vi "main4ChProspectiveStudyBK20251125.vi"() -> ()   [LabVIEW 2024]
doc: "Main VI for FLS imaging system."
uses:
  SubVI/DigitizerConfiguration/FLImDAQ.ctl
  <instrlib>/niScope/Controls/niScope trigger source.ctl
  SubVI/LabJack/LJ Pin Setting.ctl
  ConfigFiles/AimingBeamVideoConfig.ctl
  LaguerreDeconLib/DeconEngineClass/LaguerreDeconEngineClass.lvclass/LaguerreDeconEngineClass.ctl
  <vilib>/Utility/error.llb/DialogType.ctl
  LaguerreDeconLib/DeconEngineClass/LaguerreDeconEngineClass.lvclass
  <vilib>/event_ctls.llb/usereventprio.ctl
  <vilib>/Utility/miscctls.llb/LVMinMaxIncTypeDef.ctl
  SubVI/APD/APDClass.lvclass
  <vilib>/Analysis/baseanly.llb/Mean (DBL).vi
  SubVI/GlobalVariables.vi
  <vilib>/addons/control/pid/pid.llb/PID (DBL).vi
  <instrlib>/niScope/Acquire/Fetch/niScope Multi Fetch Binary 16.vi
  <vilib>/Instr/_visa.llb/VISA Configure Serial Port (Instr).vi
  <vilib>/Python/Open Anaconda Python Session.vi
  C:/Users/MarcuLab/Documents/GitHub/NetDeconForLV/Source/DotNETAssembly/output/build/LaguerreDeConNative.dll
  Documents/GitHub/NetDeconForLV/Source/DotNETAssembly/output/build/LaguerreDeConNative.dll
  <userlib>/_OpenG.lib/file/file.llb/openg_file.lvlib
  <userlib>/_OpenG.lib/time/time.llb/openg_time.lvlib
  <vilib>/Analysis/NI_AALBase.lvlib
  <vilib>/Utility/miscctls.llb/LVPointTypeDef.ctl
  <vilib>/addons/control/pid/NI_PID_pid.lvlib
panel:
  in  "488nm Power":u16(ring)=32 items=["3.30mW"=60, "2.35mW"=50, "2.00mW"=47, "1.75mW"=44, "1.48mW"=41, "1.16mW"=38, "0.87mW"=35, "0.57mW"=32, "0.28mW"=29]
  in  "CancerThreshold":dbl=0.15
  out "Decon Loop timing (ms)":dbl
  out "Ch3 Lifetime (ns)":dbl caption="Lifetime (ns)"
  out "Ch2 Lifetime (ns)":dbl caption="Lifetime (ns)"
  out "Ch1 Lifetime (ns)":dbl caption="Lifetime (ns)"
  out "Cancer Prob":dbl
  in  "Overlay selection":u16(ring)=2 items=["Gain", "Lifetime", "CancerProbability"]
  out "Record Backlog 2":i32
  in  "Auto gain ch4":bool=TRUE caption="Auto gain ch3"
  in  "V 4":dbl caption="Gain 3" min=0.0 max=4.67 step=0.1
  out "Gain4":dbl
  out "IntR4":dbl format="%#_2g"
  out "SNR4":dbl format="%#_3g"
  out "Channel 4":dbl[][](graph) caption="Channel 3"
  out "RunStartTime":u32
  out "Dig1 Temp":dbl
  out "Dig2 Temp":dbl
  out "Visualization PC video source":T1
  in  "V target(1.0)":dbl=1.0 caption="V target(1.5)" min=0.3 max=1.5 step=0.1 format="%#_4g"
  out "SNR3":dbl format="%#_3g"
  out "SNR2":dbl format="%#_3g"
  out "SNR1":dbl format="%#_3g"
  in  "Show BG removed?":bool=TRUE
  out "IntR3":dbl format="%#_2g"
  out "IntR2":dbl format="%#_2g"
  out "IntR1":dbl format="%#_2g"
  in  "Video Display":bool
  out "Gain3":dbl
  out "Gain2":dbl
  out "Gain1":dbl
  in  "Skip Data Save?":bool
  out "Aq Loop?":bool
  out "ML?":bool
  out "aquisition loop Error Out":errorcluster
  out "Laser f (Hz)":dbl
  out "Record Backlog":i32
  out "Fetch Record #":i32
  out "Sync Success?":bool
  out "Disclamer":picture
  out "Calibration #":i8
  out "BG #":i8
  in  "TCP Connect":bool
  out "Help":string
  in  "355nm Laser toggle":bool caption="355nm 460Hz"
  in  "Cali&iRF alignment":bool
  in  "Background":bool
  in  "Aiming beam toggle":bool caption="488nm 15Hz"
  in  "Auto gain ch3":bool=TRUE
  in  "Auto gain ch2":bool=TRUE
  in  "Auto gain ch1":bool=TRUE
  out "Run #":i8
  in  "StopButton":bool caption="Stop"
  out "Aquisition Status:":bool
  in  "StartButton":bool caption="Start"
  in  "V 3":dbl caption="Gain 3" min=0.0 max=4.65 step=0.1
  in  "V 2":dbl caption="Gain 2" min=0.0 max=4.59 step=0.1
  in  "V 1":dbl caption="Gain 1" min=0.0 max=4.63 step=0.1 format="%#_4g"
  in  "Video Source":enum32{"Camera", "FrameGrabber"}(radio)
  out "Case #":string
  out "System Hardware Connection Status":T2
  out "Channel 3":dbl[][](graph)
  out "Channel 2":dbl[][](graph)
  out "Channel 1":dbl[][](graph)
  in  "Tab Control":T3(tab)
  out "display loop timing(ms)":u32
  out "Aquisition loop timing(ms)":u32 format="%.2f"
  out "DisplayLoop":i32
  out "PID loop":i32 caption="processing loop"
  out "PID loop timing(ms)":u32 caption="processing loop timing(ms)"
  out "Communication loop(ms)":u32
  out "laser EM lamp V":dbl format="%0.6f"
  out "Auisition Loop idx":i32
  out "LJ process (ms)":u32
  out "LJ time(ms)":u32[](array[numeric])
  out "output variable":i32
  out "BG Graph":dbl[][](graph)
  out "Lifetime (ns)":cluster{dbl, dbl, dbl}(graph)
  out "DeCon Speed(ms)":dbl(graph)
  out "iRF Graph":dbl[][](graph)
  in  "Show BG":bool
  out "iRF length":i32
  out "BG length":i32
  out "data length":i32
  out "WarmupTime(ms)":u32
  out "BGAll":dbl[][](array[numeric])
  out "DeConOut":dbl[](array[numeric])
  in  "Ch1GainLim":dbl=350.0 format="%#_13g"
  in  "Ch2&3GainLim":dbl=1750.0 format="%#_13g"
  out "LJ Pinout":T4={"Ch1 Bias"="DAC0", "Ch2 Bias"="DAC1", "Ch3 Bias"="DAC2", "Ch4 Bias"="DAC0", "355 PWM"="FIO0", "AimingBeam PWM"="FIO2", "Laser Ready"="FIO3", "Interlock"="FIO1", "Laser Start/Stop"="FIO1", "Red LED"="FIO1", "Green LED"="DIO3", "Foot Pedal"="DIO15"}
  out "FLImDAQ":T5={"Digitizer 1"="", "Digitizer 2"="", "Channel"=enum."Channel 0", "trigger source"="VAL_EXTERNAL", "trigger level"=0.5, "trigger delay"=1.35e-07, "min sample rate"=12500000000.0, "min record length"=2500, "vertical range"=1.0, "vertical offset"=-0.25, "Waveform to Avg"=2000} caption="FLIm DAQ Configuration" {"trigger delay" format="%^#.4e"; "trigger level" min=0.0 max=3.5 step=0.5 format="%.2f"; "vertical offset" format="%.4f"; "vertical range" format="%.2f"; "min sample rate" format="%#.2p"}
  in  "Sys Reconfig":bool
  out "data out(communcation loop)":string
  out "PID loop error out":errorcluster caption="processing Error Out"
  out "decon error out":errorcluster
  out "Laser Rep Rate":dbl
  out "V4 Size":i32 caption="V3 Size"
  in  "Data Class":enum16{"Data", "BG", "Cali"}(ring)=enum."BG"
  out "V1 Size":i32
  out "V2 Size":i32
  out "V3 Size":i32
  out "data Size":i32[](array[numeric])
  out "State log":string
  out "SysConfigCluster":T7
  in  "Ch4 PID gains":T8={"proportional gain (Kc)"=30.0, "integral time (Ti, min)"=0.0003, "derivative time (Td, min)"=1e-05}
  in  "Ch3 PID gains":T8={"proportional gain (Kc)"=30.0, "integral time (Ti, min)"=0.0003, "derivative time (Td, min)"=1e-05}
  in  "Ch2 PID gains":T8={"proportional gain (Kc)"=30.0, "integral time (Ti, min)"=0.0003, "derivative time (Td, min)"=1e-05}
  in  "Ch1 PID gains":T8={"proportional gain (Kc)"=30.0, "integral time (Ti, min)"=0.0003, "derivative time (Td, min)"=1e-05}
  in  "module path":path=path "C:/Users/MarcuLab/Documents/GitHub/NetDeconForLV/Classifier/HNClassifier.py"
  in  "model path":path=path "C:/Users/MarcuLab/Documents/GitHub/NetDeconForLV/Classifier/20241127_dc/200.pkl"
  in  "Env name":string="HNClassifier"
  in  "Python version":string="3.10"
  out "Python session":refnum<k35>
  in  "Quit":bool
  in  "Radio Buttons":T9(radio)=enum."Ch2" caption="DeCon Chan"
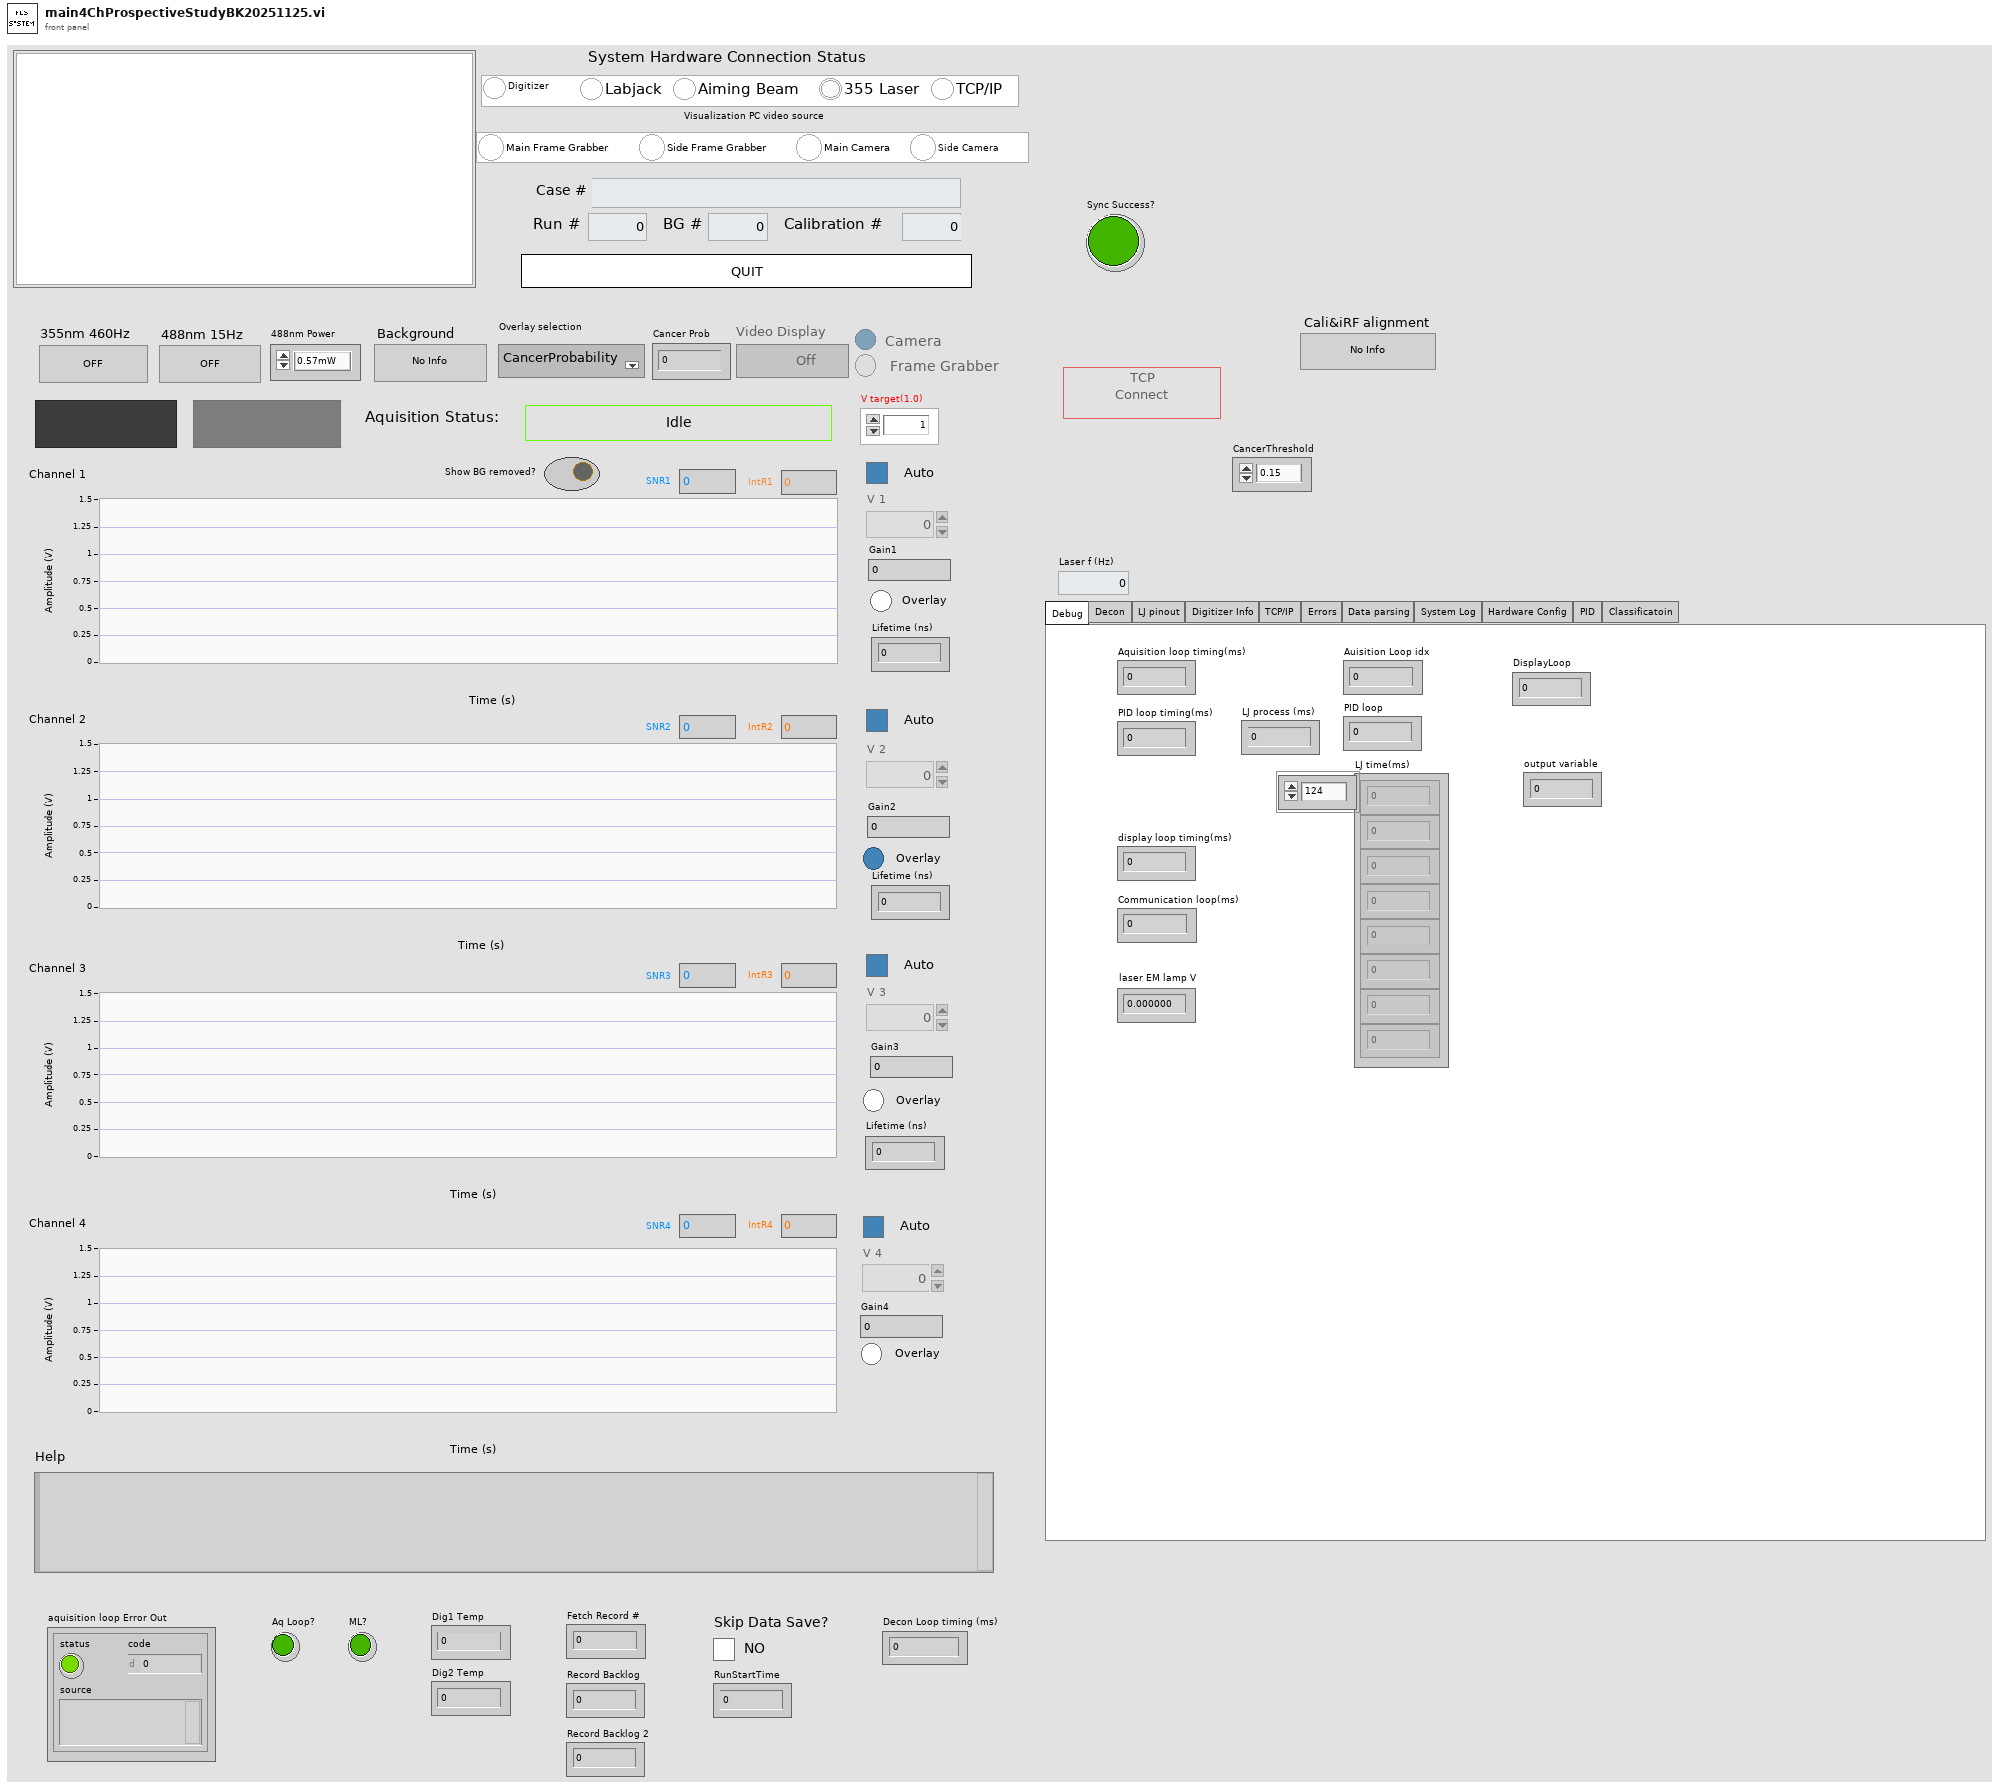
[diagram p1: front panel]
types:
  T1 = cluster{"Main Frame Grabber":bool, "Side Frame Grabber":bool, "Main Camera":bool, "Side Camera":bool}
  T2 = cluster{"Digitizer":bool, "Labjack":bool, "Aiming Beam":bool, "355 Laser":bool, "TCP/IP":bool}
  T3 = enum32{"Debug", "Decon", "LJ pinout", "Digitizer Info", "TCP/IP", "Errors", "Data parsing", "System Log", "Hardware Config", "PID", "Classificatoin"}
  T4 = typedef "LJ Pin Setting.ctl" = cluster{"Ch1 Bias":string, "Ch2 Bias":string, "Ch3 Bias":string, "Ch4 Bias":string, "355 PWM":string, "AimingBeam PWM":string, "Laser Ready":string, "Interlock":string, "Laser Start/Stop":string, "Red LED":string, "Green LED":string, "Foot Pedal":string}
  T5 = typedef "FLImDAQ.ctl" = cluster{"Digitizer 1":refnum<k15>, "Digitizer 2":refnum<k15>, "Channel":enum16{"Channel 0", "Channel 1", "Channel 0&1"}, "trigger source":T6, "trigger level":dbl, "trigger delay":dbl, "min sample rate":dbl, "min record length":i32, "vertical range":dbl, "vertical offset":dbl, "Waveform to Avg":i16}
  T6 = typedef "niScope trigger source.ctl" = string
  T7 = cluster{"Ch1Enable?":bool, "Ch2Enable?":bool, "Ch3Enable?":bool, "Ch1AutoGain?":bool, "Ch2AutoGain?":bool, "Ch3AutoGain?":bool, "AimingBeamEnable?":bool}
  T8 = cluster{"proportional gain (Kc)":dbl, "integral time (Ti, min)":dbl, "derivative time (Td, min)":dbl}
  T9 = enum32{"No Selection", "Ch1", "Ch2", "Ch3", "Ch4"}
  T10 = cluster{"remote start event":refnum<user-event>, "remote stop  event":refnum<user-event>}
  T11 = enum8{"Enabled", "Disabled", "Disabled and Grayed Out"}
  T12 = enum16{"open", "replace", "create", "open or create", "replace or create", "replace or create with confirmation"}
  T13 = cluster{"CH1":dbl[][], "CH2":dbl[][], "CH3":dbl[][], "CH4":dbl[][], "Gain cluster":cluster{"V1":dbl, "V2":dbl, "V3":dbl, "V4":dbl}}
  T14 = cluster{"idx":i32, "CH1&2":dbl[][], "CH3&4":dbl[][], "V cluster":cluster{"V1":dbl, "V2":dbl, "V3":dbl, "V4":dbl}}
  T15 = cluster{"Ch1 iRF":dbl[], "Ch2 iRF":dbl[], "Ch3 iRF":dbl[], "Ch4 iRF":dbl[]}
  T16 = enum16{"open", "open or create", "create or replace", "create", "open (read-only)"}
  T17 = enum32{"Invalid", "Standard", "Closed", "Hidden", "Minimized", "Maximized"}
  T18 = enum32{"invalid app kind", "Development System", "Run Time System", "Student Edition", "Embedded LabVIEW", "Evaluation", "Custom"}
  T19 = typedef "usereventprio.ctl" = enum32{"high priority", "normal priority"}
  T20 = enum32{"Bad", "Idle", "Run top level", "Running"}
  T21 = enum16{"Standard", "Buffered", "CRLF", "Immediate"}
  T22 = typedef "AimingBeamVideoConfig.ctl" = cluster{"DeCon Channel":enum16{"1", "2", "3"}, "Scale Bar":bool, "Scale Low":dbl, "Scale High":dbl, "ANSI":dbl, "Radius":dbl, "3D?":bool, "Firefly?":bool, "Pentero?":bool}
  T23 = cluster{"Core":cluster{"Current VI Reference":refnum<vi>, "Close Panel on Exit?":bool}, "SysConfigCluster":cluster{"Ch1Enable?":bool, "Ch2Enable?":bool, "Ch3Enable?":bool, "Ch1AutoGain?":bool, "Ch2AutoGain?":bool, "Ch3AutoGain?":bool, "AimingBeamEnable?":bool}, "System Status":cluster{"Digitizer":bool, "Labjack":bool, "Aiming Beam":bool, "355 Laser":bool, "TCP/IP":bool}, "IDs":cluster{"RunID":i8, "BG ID":i8, "Cali ID":i8}, "CaseID":string, "DefaultPath":path, "Pathes":cluster{"DataPath":path, "BG Path":path, "iRFPath":path, "CaliPath":path}, "FLImDAQ":cluster{"resource name":refnum<k15>, "resource name 2":refnum<k15>, "Channel":enum16{"Channel 0", "Channel 1", "Channel 0&1"}, "trigger source":T6, "trigger level":dbl, "trigger delay":dbl, "min sample rate":dbl, "min record length":i32, "vertical range":dbl, "vertical offset":dbl, "Waveform to Avg":i32}, "SysRunning?":bool, "AB Cluster":cluster{"Aiming Beam COM Port":refnum<visa-resource-name>, "Min Current":dbl, "Max Current":dbl, "Default Current":dbl, "Freq":i32}, "LJ Pinout":T4, "355 PWM setting":cluster{"DIO_EF_CLOCK1_DIVISOR":i16, "DIO_EF_CLOCK1_ROLL_VALUE":i32, "DIO#_EF_INDEX":i16, "DIO#_EF_OPTIONS":i16, "DIO#_EF_CONFIG_A":i32}, "AB PWM setting":cluster{"DIO_EF_CLOCK1_DIVISOR":i16, "DIO_EF_CLOCK1_ROLL_VALUE":i32, "DIO#_EF_INDEX":i16, "DIO#_EF_OPTIONS":i16, "DIO#_EF_CONFIG_A":i32}, "Last Trigger":u32, "niTClk sessions":refnum<k20>[], "Laser start tic":u32, "TCP attempt count":i32, "Ch1Data":dbl[][], "Ch2Data":dbl[][], "Ch3Data":dbl[][], "Ch4Data":dbl[][], "V1":dbl[], "V2":dbl[], "V3":dbl[], "V4":dbl[], "SlowTimer":u32, "FastTimer":u32, "listener ID":refnum<k5>, "TempPath":path, "CaliPath":path, "LED vi reference":refnum<vi>, "Aquisition Timer":u32, "APDSerialNum":cluster{"Ch1APDSerial#":string, "Ch2APDSerial#":string, "Ch3APDSerial#":string, "Ch4APDSerial#":string}, "VideoConfig":T22, "LED vi ref open?":bool, "video source":cluster{"Main Frame Grabber":bool, "Side Frame Grabber":bool, "Main Camera":bool, "Side Camera":bool}, "bothVidSourceAvail":bool}
  T24 = typedef "LVCursorListTypeDef.ctl" = cluster{"Name":string, "Color":u32, "Style":u8, "Point Style":u8, "Name Visible":bool, "Allow Drag":bool, "Cursor Mode":u32, "Plot":i32, "Index":i32, "Position":cluster{"X":dbl, "Y":dbl}, "X Scale":u32, "Y Scale":u32, "Watch Plots":i32[], "Watch All Plots":bool, "Plot Area":i32, "Label Offset":cluster{"X":dbl, "Y":dbl}}[]
  T25 = cluster{"Name":string, "Color":u32, "Style":u8, "Point Style":u8, "Name Visible":bool, "Allow Drag":bool, "Cursor Mode":u32, "Plot":i32, "Index":i32, "Position":cluster{"X":dbl, "Y":dbl}, "X Scale":u32, "Y Scale":u32, "Watch Plots":i32[], "Watch All Plots":bool, "Plot Area":i32, "Label Offset":cluster{"X":dbl, "Y":dbl}}
  T26 = cluster{"Ch1APDSerial#":string, "Ch2APDSerial#":string, "Ch3APDSerial#":string, "Ch4APDSerial#":string}
  T27 = cluster{"DataPath":path, "BG Path":path, "iRFPath":path, "CaliPath":path}
  T28 = cluster{"DIO_EF_CLOCK1_DIVISOR":i16, "DIO_EF_CLOCK1_ROLL_VALUE":i32, "DIO#_EF_INDEX":i16, "DIO#_EF_OPTIONS":i16, "DIO#_EF_CONFIG_A":i32}
  T29 = cluster{"Aiming Beam COM Port":refnum<visa-resource-name>, "Min Current":dbl, "Max Current":dbl, "Default Current":dbl, "Freq":i32}
  T30 = cluster{"resource name":refnum<k15>, "resource name 2":refnum<k15>, "Channel":enum16{"Channel 0", "Channel 1", "Channel 0&1"}, "trigger source":T6, "trigger level":dbl, "trigger delay":dbl, "min sample rate":dbl, "min record length":i32, "vertical range":dbl, "vertical offset":dbl, "Waveform to Avg":i32}
  T31 = cluster{"Current VI Reference":refnum<vi>, "Close Panel on Exit?":bool}
  T32 = cluster{"Channel 1":dbl[], "Channel 2":dbl[], "Channel 3":dbl[], "Channel 4":dbl[]}
  T33 = cluster{"V 1":dbl[], "V 2":dbl[], "V 3":dbl[], "V 4":dbl[]}
  T34 = cluster{"Ch1 WF":dbl[], "Ch2 WF":dbl[], "Ch3 WF":dbl[], "Ch4 WF":dbl[], "V1":dbl, "V2":dbl, "V3":dbl, "V4":dbl}
  T35 = typedef "iRFData.ctl" = cluster{"dt":dbl, "NumOfWFs":i32, "WFLength":i32, "iRFCtrlV":dbl[], "iRFWFsAvg":dbl[][], "iRFRaw":dbl[][]}
  T36 = cluster{"mean":dbl, "mean":dbl, "mean":dbl, "mean":dbl}
  T37 = cluster{"V1":dbl, "V2":dbl, "V3":dbl, "V4":dbl}[]
  T38 = cluster{"DataPath":path, "CaseID":string, "RunID":i16, "Ch1Data":dbl[][], "Ch2Data":dbl[][], "Ch3Data":dbl[][], "Ch4Data":dbl[][], "V1":dbl[], "V2":dbl[], "V3":dbl[], "V4":dbl[], "LaserRepRate":u16, "WFAverage":i16, "RunStartTime":u64}
  T39 = typedef "DialogType.ctl" = u16
  T40 = typedef "APD.ctl" = cluster{"gainV":dbl[], "gain":dbl[], "irfV":dbl[], "irfTNorm":dbl[][]}
  T41 = typedef "LJ PWM Setting.ctl" = cluster{"DIO_EF_CLOCK1_DIVISOR":i16, "DIO_EF_CLOCK1_ROLL_VALUE":i32, "DIO#_EF_INDEX":i16, "DIO#_EF_OPTIONS":i16, "DIO#_EF_CONFIG_A":i32}
  T42 = typedef "AimingBeam.ctl" = cluster{"Aiming Beam COM Port":refnum<visa-resource-name>, "Min Current":dbl, "Max Current":dbl, "Default Current":dbl, "Frequency(Hz)":u32}
  T43 = cluster{"DC1":i32, "DC2":i32, "BG1":i32, "BG2":i32}
  T44 = typedef "LVMinMaxIncTypeDef.ctl" = cluster{"Minimum":dbl, "Maximum":dbl, "Increment":dbl}
  T45 = typedef "LVBoundsTypeDef.ctl" = cluster{"Width":u32, "Height":u32}
  T46 = typedef "imagedata.ctl" = cluster{"image type":i32, "image depth":i32, "image":u8[], "mask":u8[], "colors":u32[], "Rectangle":cluster{"left":i16, "top":i16, "right":i16, "bottom":i16}}
  T47 = cluster{"DC Idx1":i32, "DC Idx2":i32, "BG Idx1":i32, "BG Idx2":i32}
  T48 = cluster{dbl[][], dbl[][], dbl[][], dbl[][], "V cluster":cluster{"V1":dbl, "V2":dbl, "V3":dbl, "V4":dbl}}
  T49 = cluster{"actualSamples":i32, "absoluteInitialX":dbl, "relativeInitialX":dbl, "xIncrement":dbl, "offset":dbl, "gain":dbl, "reserved1":dbl, "reserved2":dbl}[]
  T50 = cluster{"V1 out":dbl, "V2 out":dbl, "V3 out":dbl, "V3 out":dbl}
  T51 = cluster{i32, dbl[][], dbl[][], cluster{"V1 out":dbl, "V2 out":dbl, "V3 out":dbl, "V3 out":dbl}}
  T52 = typedef "LVPointTypeDef.ctl" = cluster{"Horizontal":i16, "Vertical":i16}
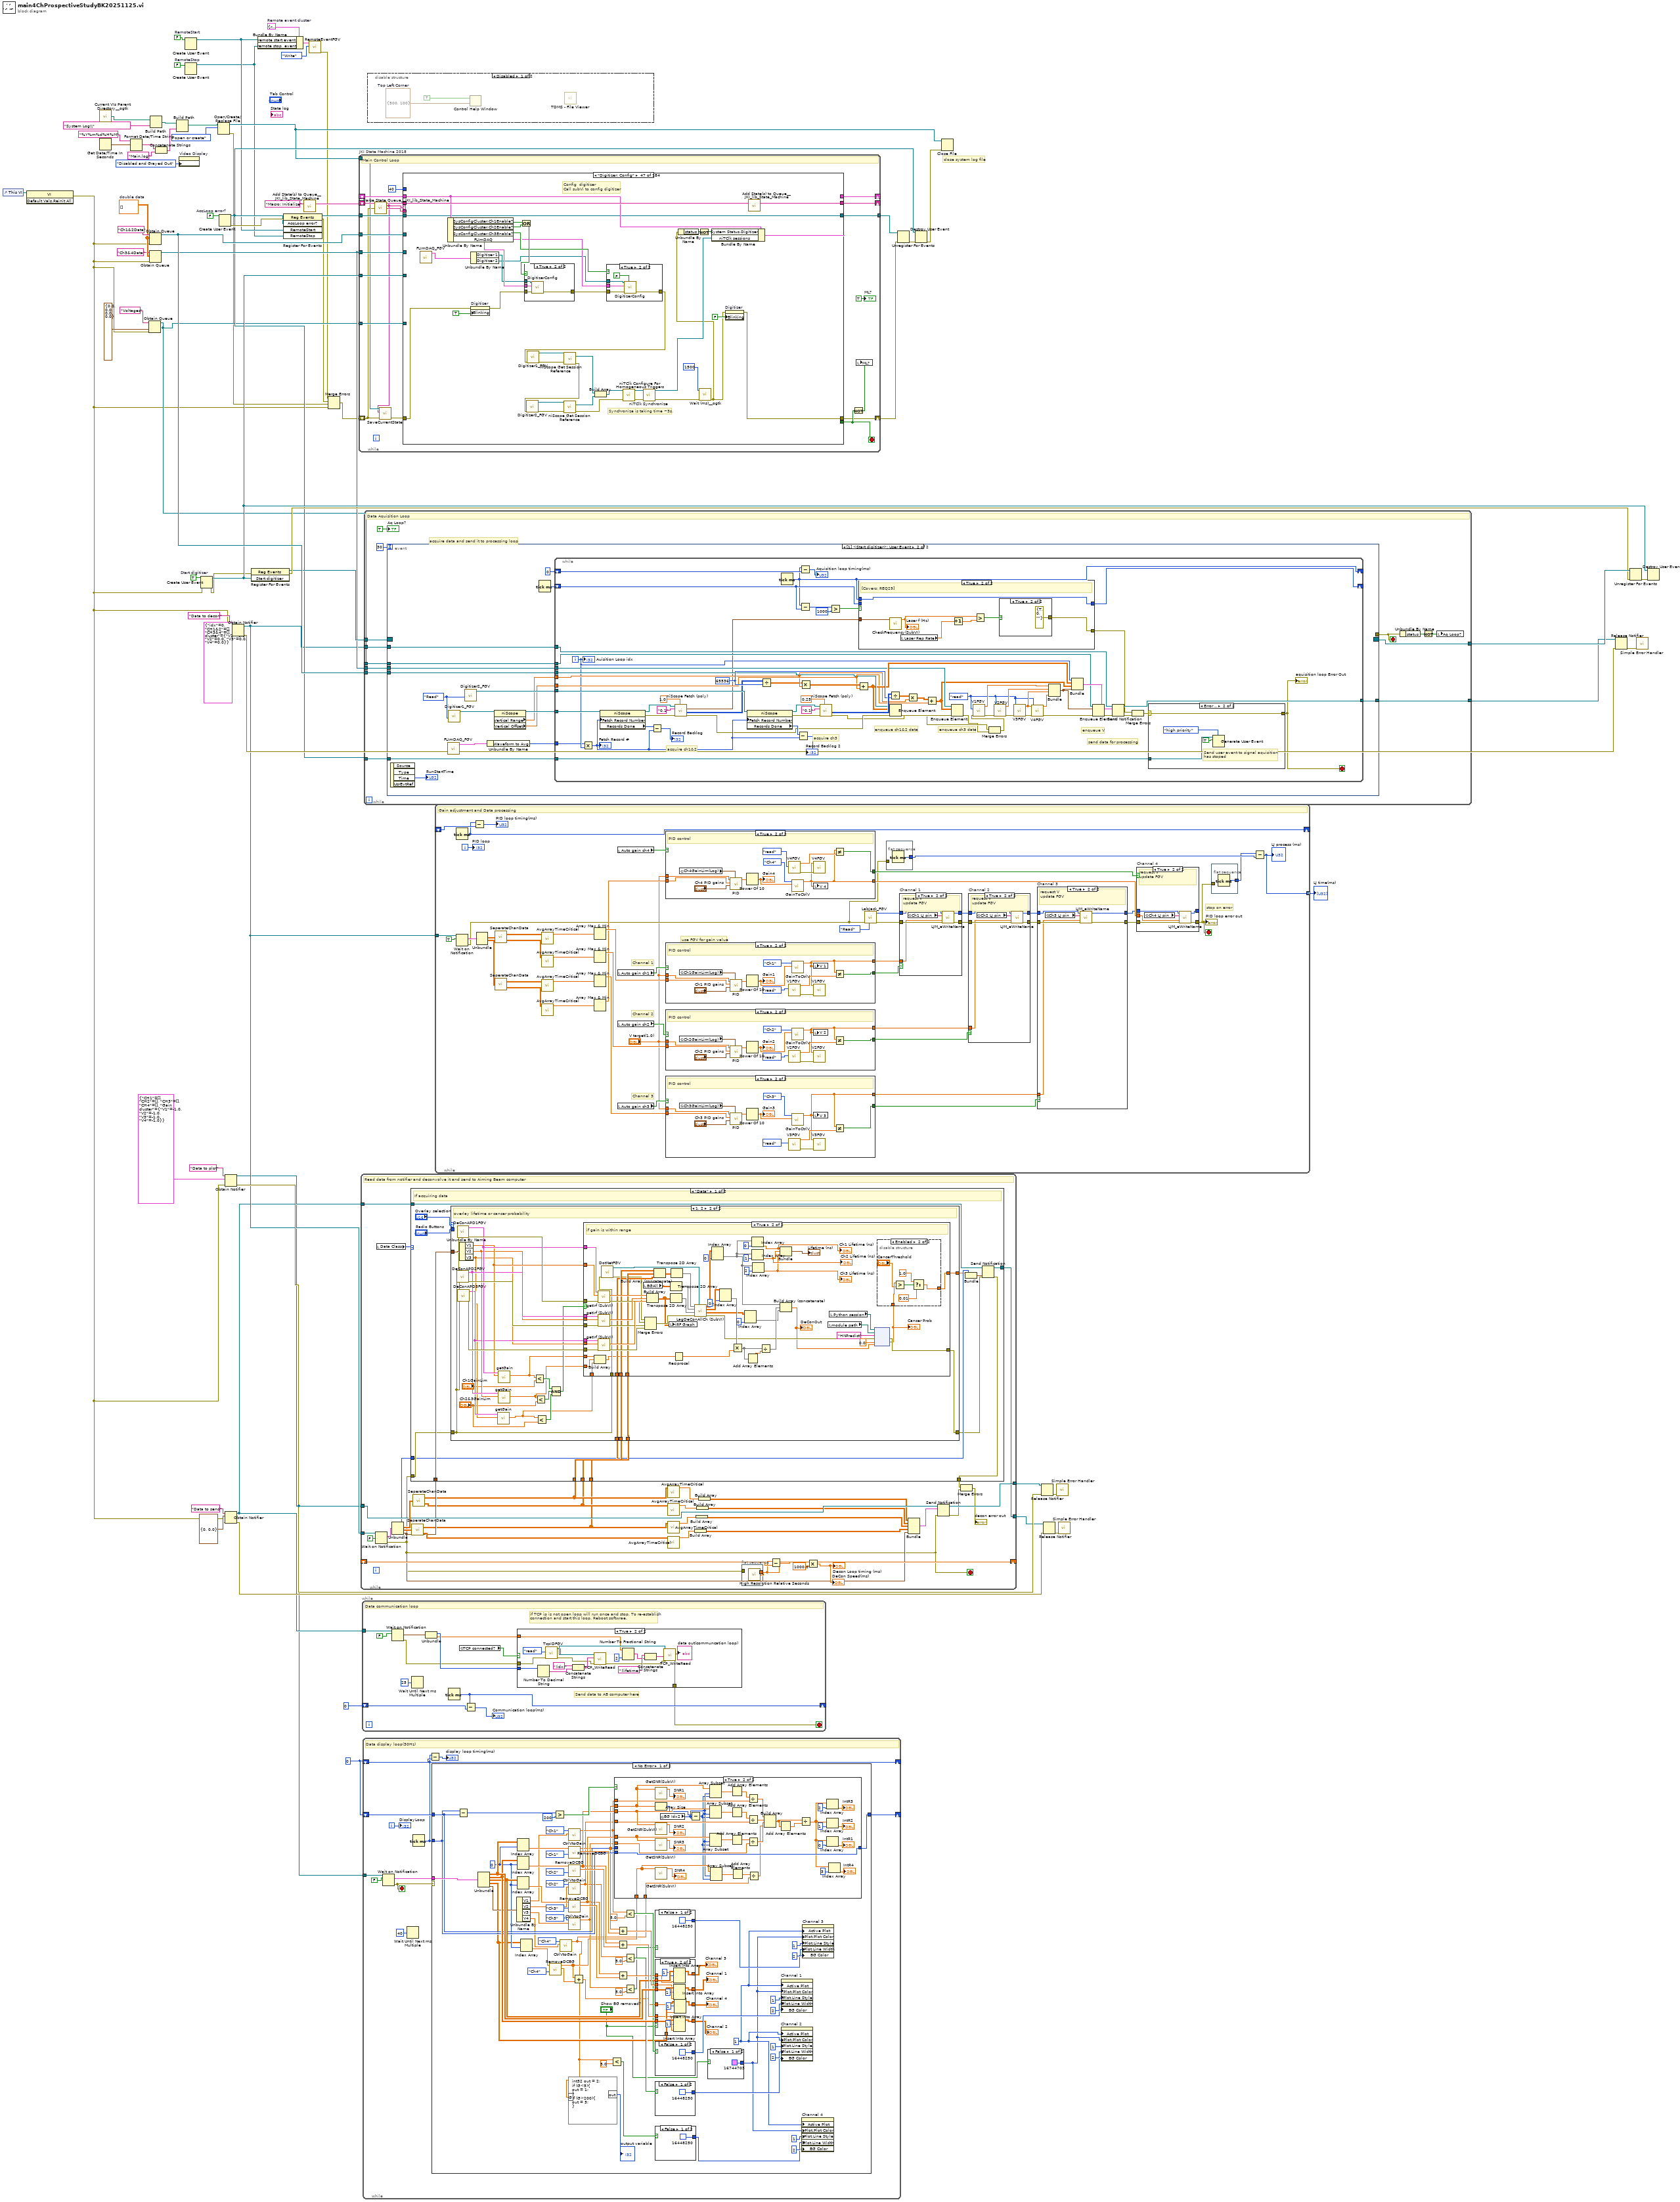
[diagram p0: block diagram]
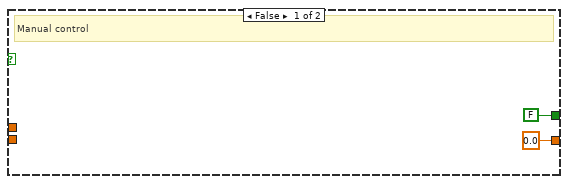
[diagram p6: hidden frame]
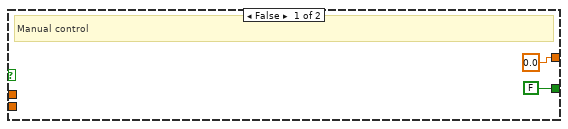
[diagram p7: hidden frame]
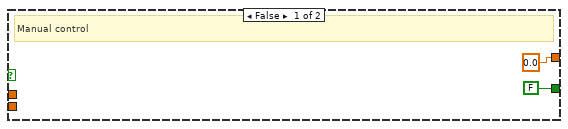
[diagram p8: hidden frame]
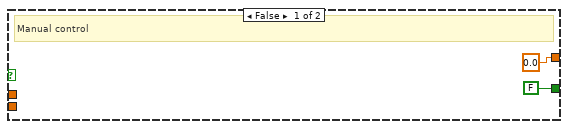
[diagram p9: hidden frame]
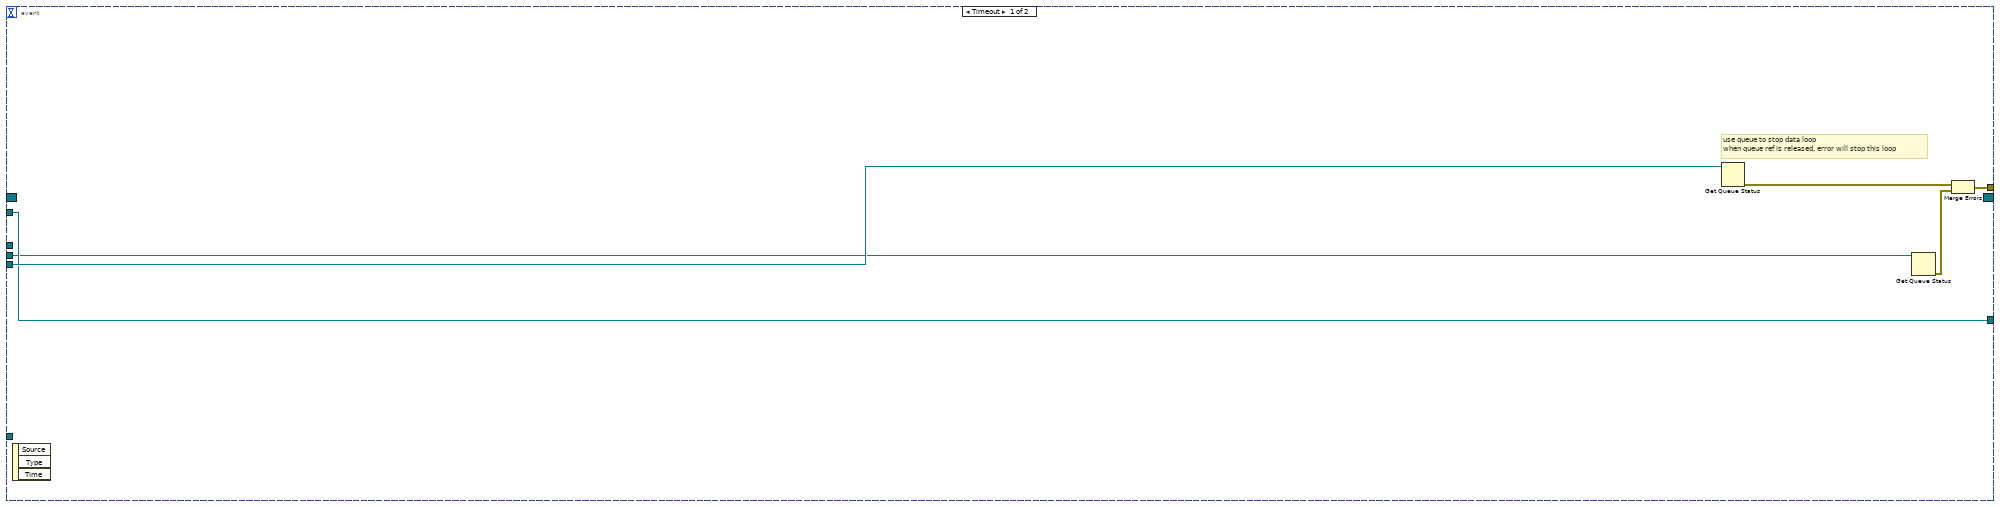
[diagram p10: hidden frame]
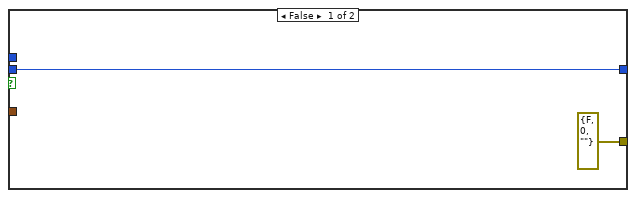
[diagram p11: hidden frame]
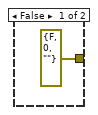
[diagram p12: hidden frame]
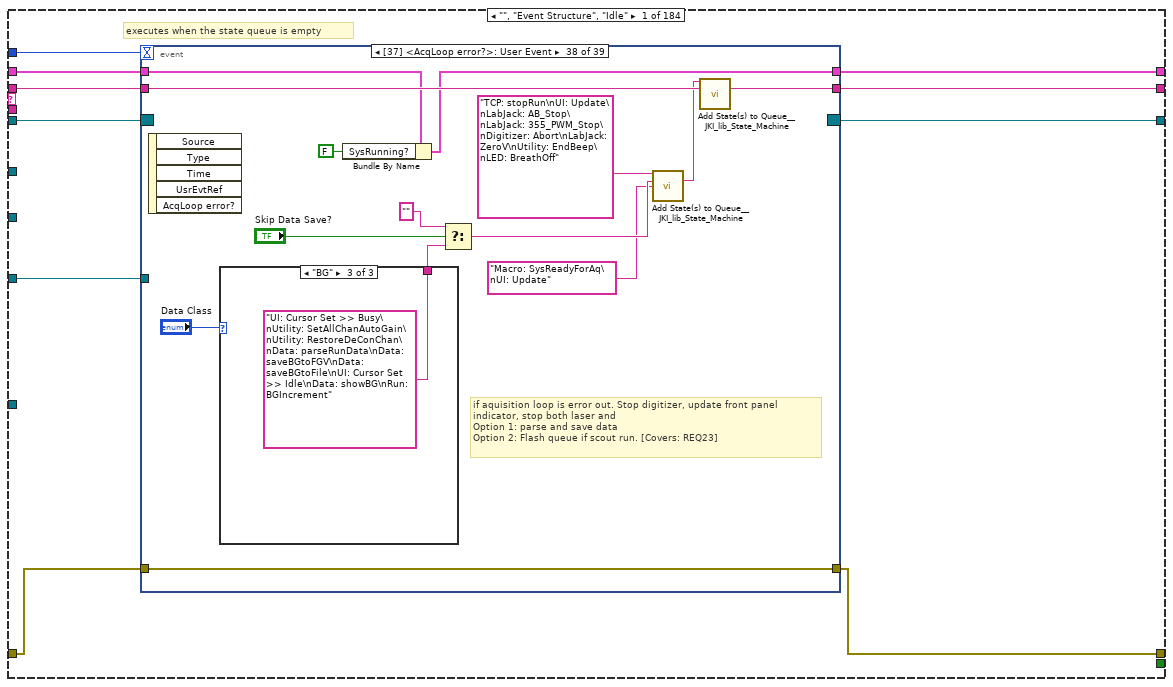
[diagram p14: hidden frame]
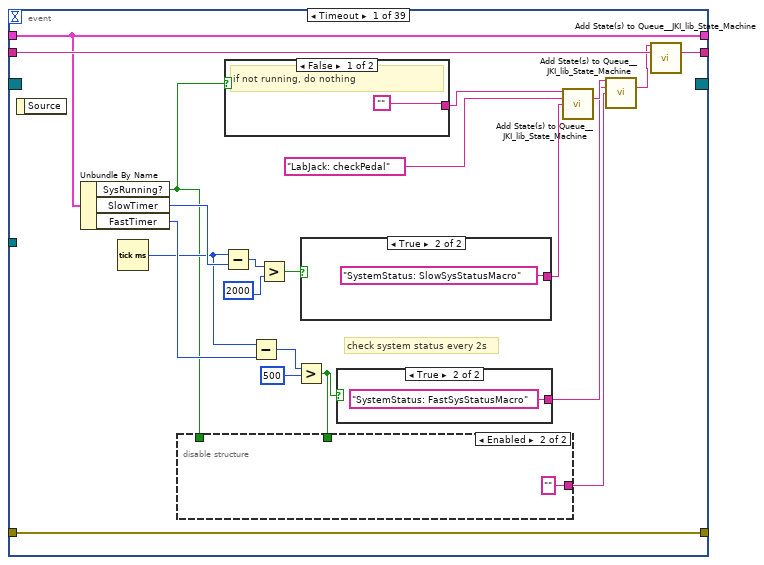
[diagram p15: hidden frame]
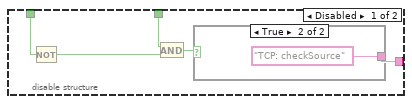
[diagram p16: hidden frame]
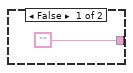
[diagram p17: hidden frame]
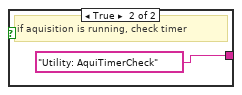
[diagram p18: hidden frame]
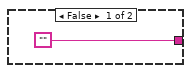
[diagram p19: hidden frame]
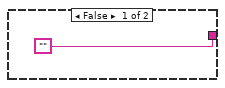
[diagram p20: hidden frame]
diagram:
  w8 = T10 {"remote start event"=refnum, "remote stop  event"=refnum}  # Remote event cluster
  w11 = FALSE  # RemoteStop
  w12 = FALSE  # RemoteStart
  w15 = u32 0 ("millisecond timer value")
  w54 = FALSE  # AcqLoop error?
  w64 = TRUE  # Start digitizer
  w67 = dbl[][] []  # double data
  # "close system log file"
  n1 = control-ref of="This VI"() -> (w69:refnum<vi>)
  n2 = invoke on="Invoke Node" class="VI" method="Default Vals.Reinit All"(reference=w69) -> (error out=w23:errorcluster)  [unwired: 2 in, 2 out]
  n3 = call <userlib>:"Current VIs Parent Directory__ogtk.vi"() -> ("Parent Directory (+ Relative)"=w34:path)  [unwired: 5 in]
  n4 = Get Date/Time In Seconds() -> (seconds since 1Jan1904=w32:timestamp)
  n5 = Format Date/Time String(time format string (%c)="%Y%m%d%H%M", seconds (now)=w32) -> (date/time string=w29:string)  [unwired: 1 in]
  n6 = Obtain Queue(name (unnamed)="Voltages", element data type=cluster{"V1":dbl, "V2":dbl, "V3":dbl, "V4":dbl} {"V1"=0.0, "V2"=0.0, "V3"=0.0, "V4"=0.0}, error in (no error)=w23) -> (queue out=w35:refnum<queue>)  [unwired: 2 in, 2 out]
  n7 = Obtain Queue(name (unnamed)="Ch3&4Data", element data type=w67, error in (no error)=w23) -> (queue out=w48:refnum<queue>)  [unwired: 2 in, 2 out]
  n8 = Obtain Queue(name (unnamed)="Ch1&2Data", element data type=w67, error in (no error)=w23) -> (queue out=w65:refnum<queue>)  [unwired: 2 in, 2 out]
  n9 = Build Path(base path=w34, name or relative path="System Log\\") -> (appended path=w25:path)
  n10 = Concatenate Strings(w29, "Main.log" ("string")) -> (w27:string)
  n11 = Build Path(base path=w25, name or relative path=w27) -> (appended path=w30:path)
  n12 = property on="Video Display" class="Bool (strict)"("DisabledEnum"=T11."Disabled and Grayed Out" ("Disabled")) -> ()  [unwired: 2 in, 2 out]
  n13 = Create User Event(user event datatype=w12) -> (user event=w10:refnum<user-event>)  [unwired: 1 in, 1 out]
  n14 = Create User Event(user event datatype=w11) -> (user event=w9:refnum<user-event>)  [unwired: 1 in, 1 out]
  n15 = Create User Event(user event datatype=w64, error in=w23) -> (user event=w53:refnum<user-event>, error out=w40:errorcluster)
  n16 = Open/Create/Replace File(file path (use dialog)=w30, operation (0:open)=T12."open or create") -> (refnum out=w21:refnum<file>, error out=w22:errorcluster)  [unwired: 4 in, 1 out]
  n17 = Create User Event(user event datatype=w54) -> (user event=w39:refnum<user-event>, error out=w41:errorcluster)  [unwired: 1 in]
  n18 = Obtain Notifier(name (unnamed)="Data to plot", notification data type=T13 {"CH1"=[], "CH2"=[], "CH3"=[], "CH4"=[], "Gain cluster"={"V1"=-1.0, "V2"=-1.0, "V3"=-1.0, "V4"=-1.0}}, error in (no error)=w23) -> (notifier out=w13:refnum<notifier>, error out=w49:errorcluster)  [unwired: 1 in, 1 out]
  n19 = Obtain Notifier(name (unnamed)="Data to send", notification data type=cluster{"idx":i32, "lifetime":dbl} {"idx"=0, "lifetime"=0.0}, error in (no error)=w23) -> (notifier out=w18:refnum<notifier>, error out=w38:errorcluster)  [unwired: 1 in, 1 out]
  n20 = Obtain Notifier(name (unnamed)="Data to decon", notification data type=T14 {"idx"=0, "CH1&2"=[], "CH3&4"=[], "V cluster"={"V1"=0.0, "V2"=0.0, "V3"=0.0, "V4"=0.0}}, error in (no error)=w23) -> (notifier out=w19:refnum<notifier>, error out=w58:errorcluster)  [unwired: 1 in, 1 out]
  n21 = register-events(error in=w40, w53) -> (reference out=w55:refnum<event-registration>, error out=w61:errorcluster)  [unwired: 1 in]
  n22 = Bundle By Name(cluster=w8, "remote start event"=w10, "remote stop  event"=w9) -> (w6:T10)
  n23 = register-events(error in=w41, w39, w10, w9) -> (reference out=w47:refnum<event-registration>, error out=w5:errorcluster)  [unwired: 1 in]
  n24 = call <vilib>:"Add State(s) to Queue__JKI_lib_State_Machine.vi"("State(s) in (\"\")"="Macro: Initialize") -> ("States Out"=w71:string)  [unwired: 14 in]
  n25 = call "RemoteEventFGV.vi"("Operation (Read)"=enum16{"Read", "Write"}."Write", "Remote Event in"=w6) -> ("Error Out"=w2:errorcluster)  [unwired: 8 in, 1 out]
  n26 = Merge Errors(w2, w5, w22, w23) -> (w24:errorcluster)
  n27 = while "JKI State Machine 2018" {
    shift-right: [w88] -> _
    shift-left: _ -> [w87]
    shift-right: [w72] -> w4
    shift-left: w24 -> [w74]
    shift-right: [w89] -> _
    shift-left: w71 -> [w90]
    tunnel: w65 -> [w85]
    tunnel: w48 -> [w84]
    tunnel: w53 -> [w83]
    tunnel: w47 -> [w82]
    tunnel: [w81] -> w46
    tunnel: w35 -> [w77]
    tunnel: w21 -> [w76]
    stop <- w80 stop-if-true
    # "Main Control Loop"
    n28 = call <vilib>:"Parse State Queue__JKI_lib_State_Machine.vi"("State Queue"=w90, "Error In (no error)"=w74) -> ("Remaining States"=w92:string, "Current State"=w75:string, "Arguments"=w91:string)  [unwired: 11 in]
    n29 = call "SaveCurrentState.vi"("error in (no error)"=w74, "Current State"=w75, "Byte Stream File in"=w76) -> ("error out"=w73:errorcluster)  [unwired: 8 in]
    n30 = case shown="\"Digitizer: Config\"" w75 {
      selector: w75 -> [_ _ _ _ _ _ _ _ _ _ _ _ _ _ _ _ _ _ _ _ _ _ _ _ w1096 _ _ _ _ _ _ _ _ _ _ _ _ _ _ _ _ _ _ _ _ _ _ _ _ _ _ _ _ _ _ _ _ _ _ _ _ _ _ _ _ _ _ _ _ _ _ _ _ _ _ _ _ _ _ _ _ _ _ _ _ _ _ _ _ _ _ _ _ _ _ _ _ _ _ _ _ _ _ _ _ _ _ _ _ _ _ _ _ _ _ _ _ _ _ _ _ _ _ _ _ _ _ _ _ _ _ _ _ _ _ _ _ _ _ _ _ _ _ _ _ _ _ _ _ _ _ _ _ _ _ _ _ _ _ _ _ _ _ _ _ _ _ _ _ _ _ _ _ _ _ _ _ _ _ _ _ _ _ _]
      tunnel: w92 -> [w102 w515 w524 w530 w536 w558 w571 w613 w619 w646 w665 w736 w751 w782 w809 w841 w872 w901 w915 w1000 w1037 w1076 w1089 w1094 w1100 w1128 w1136 w1159 w1164 w1177 w1196 w1224 w1252 w1290 w1295 w1304 w1315 w1345 w1353 w1359 w1383 w1407 w1431 w1455 w1460 w1477 w1524 w1546 w1562 w1577 w1597 w1602 w1614 w1643 w1669 w1681 w1719 w1732 w1738 w1749 w1761 w1792 w1805 w1819 w1834 w1853 w1888 w1893 w1907 w1917 w1933 w1945 w1957 w1985 w2000 w2005 w2017 w2029 w2034 w2042 w2050 w2059 w2068 w2073 w2081 w2090 w2108 w2125 w2145 w2156 w2174 w2189 w2206 w2211 w2219 w2227 w2232 w2240 w2247 w2255 w2262 w2272 w2300 w2308 w2315 w2323 w2328 w2336 w2343 w2349 w2358 w2374 w2379 w2386 w2398 w2468 w2480 w2489 w2503 w2512 w2529 w2552 w2569 w2580 w2593 w2618 w2641 w2647 w2663 w2685 w2693 w2699 w2704 w2711 w2721 w2733 w2742 w2747 w2759 w2764 w2774 w2780 w2786 w2791 w2796 w2801 w2811 w2835 w2856 w2861 w2872 w2897 w2924 w2947 w2952 w2967 w3018 w3064 w3109 w3120 w3138 w3158 w3172 w3185 w3193 w3210 w3232 w3256 w3275 w3293 w3311 w3329 w3343 w3357 w3376 w3390 w3405 w3420 w3429 w3434 w3450 w3458 w3465 w3470]
      tunnel: w91 -> [_ _ _ _ _ _ _ _ _ _ _ _ _ _ _ _ _ _ _ _ _ _ _ _ _ _ _ _ _ _ _ _ _ _ _ _ _ _ _ _ _ _ _ _ _ _ _ _ _ _ _ _ _ _ _ _ _ _ _ _ w1759 _ _ _ _ _ _ _ _ _ _ _ _ _ _ _ _ _ _ _ _ _ _ _ _ _ _ _ _ _ _ _ _ _ _ _ _ _ _ _ _ w2263 _ _ _ _ _ _ _ _ _ _ _ w2381 w2392 _ _ _ _ w2509 w2526 _ _ _ _ _ w2637 _ _ _ _ _ _ w2706 _ _ _ _ _ _ w2770 _ _ _ _ _ _ _ _ _ _ _ _ _ _ _ _ _ _ _ _ _ _ _ _ _ _ _ _ _ _ _ _ _ _ _ _ _ _ _ _ _ _ _]
      tunnel: w87 -> [w100 w512 w520 w527 w533 w555 w568 _ w615 w642 w661 w733 w742 w779 w801 w832 w869 w898 w912 w961 w1029 w1064 w1084 w1091 w1098 w1121 w1133 w1157 w1161 w1165 w1186 w1216 w1244 w1286 w1292 w1302 w1313 w1343 w1351 w1356 w1364 w1388 w1413 w1437 w1457 w1470 w1514 w1543 w1547 w1574 w1594 w1599 w1603 w1632 w1659 w1674 w1702 w1730 w1735 w1742 w1757 w1775 w1800 w1811 w1829 w1846 w1871 w1890 w1903 w1911 w1930 w1942 w1954 w1973 w1989 w2002 w2015 w2027 w2031 w2036 w2043 w2055 w2064 w2070 w2077 w2087 w2095 w2112 w2140 w2146 w2171 w2182 w2204 w2208 w2212 w2220 w2229 w2238 w2244 w2252 w2259 w2269 w2297 w2305 w2312 w2320 w2325 w2330 w2341 w2346 w2352 w2371 w2376 w2384 w2394 w2465 w2470 w2483 w2501 w2510 w2527 w2542 w2566 w2577 w2587 w2611 w2638 w2644 w2656 w2681 w2690 w2696 w2701 w2708 w2715 w2729 w2739 w2744 w2756 w2761 w2767 w2777 w2783 w2788 w2793 w2798 w2808 w2833 w2854 w2858 w2870 w2895 w2922 w2945 w2949 w2960 w3012 w3060 w3106 w3116 w3133 w3153 w3167 w3181 w3187 w3205 w3227 w3251 w3270 w3288 w3306 w3324 w3338 w3352 w3371 w3385 w3400 w3417 w3427 w3431 w3448 w3456 w3462 w3467]
      tunnel: [w93 w513 w522 w528 w534 w556 w569 w611 w617 w638 w657 w710 w738 w780 w789 w821 w857 w889 w913 w937 w1026 w1063 w1085 w1092 w1102 w1125 errorcluster {"status"=FALSE, "code"=0, "source"=""} ("error out") w1156 w1162 w1175 w1194 w1208 w1231 w1288 w1293 w1297 w1308 w1318 w1347 w1357 w1365 w1389 w1414 w1438 w1458 w1461 w1506 w1537 w1551 w1575 w1585 w1600 w1606 w1630 w1658 w1673 w1689 w1724 w1736 w1747 w1751 w1766 w1795 w1807 w1825 w1845 w1862 w1891 w1895 w1913 w1928 w1940 w1952 w1975 w1990 w2003 w2007 w2024 w2032 w2040 w2048 w2052 w2061 w2071 w2074 w2083 w2098 w2120 w2139 w2150 w2164 w2186 w2202 w2209 w2217 w2225 w2230 w2237 w2245 w2253 w2260 w2270 w2298 w2306 w2313 w2321 w2326 w2334 w2340 w2347 w2355 w2372 w2377 w2382 w2395 w2466 w2474 w2486 w2493 w2506 w2523 w2543 w2567 w2576 w2589 w2613 w2639 w2645 w2653 w2675 w2691 w2697 w2702 w2709 w2719 w2731 w2740 w2745 w2757 w2762 w2772 w2778 w2784 w2789 w2794 w2799 w2809 w2823 w2847 w2859 w2863 w2882 w2914 w2939 w2950 w2954 w3013 w3061 w3107 w3115 w3135 w3155 w3169 w3183 w3189 w3207 w3229 w3253 w3272 w3290 w3308 w3326 w3340 w3354 w3373 w3387 w3401 w3418 w3425 w3432 w3438 w3451 w3463 w3468] -> w72
      tunnel: w73 -> [w99 w513 w522 w528 w534 w556 w569 w611 w617 w639 w655 w710 w737 w780 w790 w828 w858 w879 w913 w937 w1027 w1066 w1086 w1092 w1101 w1125 w1129 w1156 w1162 w1175 w1194 w1207 w1243 w1288 w1293 w1296 w1309 w1323 w1346 w1357 w1369 w1393 w1418 w1442 w1458 w1468 w1509 w1536 w1550 w1575 w1587 w1600 w1605 w1631 w1649 w1679 w1700 w1723 w1736 w1744 w1754 w1765 w1794 w1810 w1824 w1844 w1861 w1891 w1901 w1914 w1927 w1939 w1951 w1974 w1991 w2003 w2006 w2019 w2032 w2040 w2048 w2051 w2060 w2071 w2075 w2084 w2103 w2119 w2138 w2149 w2170 w2185 w2201 w2209 w2217 w2225 w2230 w2237 w2245 w2253 w2260 w2270 w2298 w2306 w2313 w2321 w2326 w2334 w2340 w2347 w2355 w2372 w2377 w2383 w2396 w2466 w2475 w2485 w2492 w2505 w2522 w2544 w2567 w2576 w2584 w2616 w2639 w2645 w2658 w2674 w2691 w2697 w2702 w2709 w2719 w2731 w2740 w2745 w2757 w2762 w2772 w2778 w2784 w2789 w2794 w2799 w2809 w2822 w2846 w2859 w2862 w2881 w2904 w2930 w2950 _ w3014 w3061 w3107 w3114 w3134 w3154 w3168 w3183 w3188 w3206 w3228 w3252 w3271 w3289 w3307 w3325 w3339 w3353 w3372 w3386 w3399 w3418 w3424 w3432 w3443 w3453 w3463 w3468]
      tunnel: [w101 w514 w523 w529 w535 w557 w570 w612 w618 w645 w664 w735 w750 w781 w808 w840 w871 w900 w914 w999 w1036 w1075 w1088 w1093 w1099 w1127 w1135 w1158 w1163 w1176 w1195 w1223 w1251 w1289 w1294 w1303 w1314 w1344 w1352 w1358 w1382 w1406 w1430 w1454 w1459 w1476 w1523 w1545 w1561 w1576 w1596 w1601 w1613 w1642 w1668 w1680 w1718 w1731 w1737 w1748 w1760 w1791 w1804 w1818 w1833 w1852 w1887 w1892 w1906 w1916 w1932 w1944 w1956 w1984 w1999 w2004 w2016 w2028 w2033 w2041 w2049 w2058 w2067 w2072 w2080 w2089 w2107 w2124 w2144 w2155 w2173 w2188 w2205 w2210 w2218 w2226 w2231 w2239 w2246 w2254 w2261 w2271 w2299 w2307 w2314 w2322 w2327 w2335 w2342 w2348 w2357 w2373 w2378 w2385 w2397 w2467 w2479 w2488 w2502 w2511 w2528 w2551 w2568 w2579 w2592 w2617 w2640 w2646 w2662 w2684 w2692 w2698 w2703 w2710 w2720 w2732 w2741 w2746 w2758 w2763 w2773 w2779 w2785 w2790 w2795 w2800 w2810 w2834 w2855 w2860 w2871 w2896 w2923 w2946 w2951 w2966 w3017 w3063 w3108 w3119 w3137 w3157 w3171 w3184 w3192 w3209 w3231 w3255 w3274 w3292 w3310 w3328 w3342 w3356 w3375 w3389 w3404 w3419 w3428 w3433 w3449 w3457 w3464 w3469] -> w89
      tunnel: [_ _ _ _ _ _ _ _ _ _ _ _ _ _ _ _ _ _ _ _ _ _ _ _ _ _ _ TRUE _ _ _ _ _ _ _ _ _ _ _ _ _ _ _ _ _ _ _ _ _ _ _ _ _ _ _ _ _ _ _ _ _ _ _ _ _ _ _ _ _ _ _ _ _ _ _ _ _ _ _ _ _ _ _ _ _ _ _ _ _ _ _ _ _ _ _ _ _ _ _ _ _ _ _ _ _ _ _ _ _ _ _ _ _ _ _ _ _ _ _ _ _ _ _ _ _ _ _ _ _ _ _ _ _ _ _ _ _ _ _ _ _ _ _ _ _ _ _ _ _ _ _ _ _ _ _ _ _ _ _ _ _ _ _ _ _ _ _ _ _ _ _ _ _ _ _ _ _ _ _ _ _ _ _ _] -> w80
      tunnel: [w98 w512 w520 w527 w533 w555 w568 w586 w615 w642 w661 w733 w742 w779 w801 w832 w869 w898 w912 w961 w1030 w1065 w1084 w1091 w1098 w1126 w1133 w1157 w1161 w1166 w1187 w1217 w1245 w1287 w1292 w1302 w1313 w1343 w1351 w1356 w1364 w1388 w1413 w1437 w1457 w1470 w1515 w1543 w1548 w1574 w1595 w1599 w1604 w1632 w1659 w1678 w1702 w1730 w1735 w1745 w1757 w1775 w1800 w1811 w1829 w1846 w1871 w1890 w1904 w1911 w1930 w1942 w1954 w1973 w1989 w2002 w2015 w2027 w2031 w2037 w2044 w2056 w2065 w2070 w2078 w2088 w2096 w2118 w2127 w2151 w2172 w2183 w2204 w2208 w2213 w2221 w2229 w2238 w2244 w2252 w2259 w2269 w2297 w2305 w2312 w2320 w2325 w2330 w2341 w2346 w2352 w2371 w2376 w2384 w2394 w2465 w2471 w2484 w2501 w2510 w2527 w2542 w2566 w2577 w2588 w2612 w2638 w2644 w2657 w2681 w2690 w2696 w2701 w2708 w2716 w2729 w2739 w2744 w2756 w2761 w2767 w2777 w2783 w2788 w2793 w2798 w2808 w2833 w2854 w2858 w2870 w2895 w2922 w2945 w2949 w2965 w3011 w3060 w3106 w3116 w3133 w3153 w3167 w3181 w3187 w3205 w3227 w3251 w3270 w3288 w3306 w3324 w3338 w3352 w3371 w3385 w3402 w3417 w3427 w3431 w3448 w3456 w3462 w3467] -> w88
      tunnel: 40 ("Timeout") -> [w97 _ _ _ _ _ _ _ _ _ _ _ _ _ _ _ _ _ _ _ _ _ _ _ _ _ _ _ _ _ _ _ _ _ _ _ _ _ _ _ _ _ _ _ _ _ _ _ _ _ _ _ _ _ _ _ _ _ _ _ _ _ _ _ _ _ _ _ _ _ _ _ _ _ _ _ _ _ _ _ _ _ _ _ _ _ _ _ _ _ _ _ _ _ _ _ _ _ _ _ _ _ _ _ _ _ _ _ _ _ _ _ _ _ _ _ _ _ _ _ _ _ _ _ _ _ _ _ _ _ _ _ _ _ _ _ _ _ _ _ _ _ _ _ _ _ _ _ _ _ _ _ _ _ _ _ _ _ _ _ _ _ _ _ _ _ _ _ _ _ _ _ _ _ _ _ _ _ _ _ _ _ _ _]
      tunnel: w85 -> [_ _ _ _ _ _ _ _ _ _ _ _ _ _ _ _ _ _ _ _ w1034 _ _ _ _ _ _ _ _ _ _ _ _ _ _ _ _ _ _ _ _ _ _ _ _ _ _ _ _ _ _ _ _ _ _ _ _ _ _ _ _ _ _ _ _ _ _ _ _ _ _ _ _ _ _ _ w2012 w2023 _ _ _ _ _ _ _ _ _ _ _ _ _ _ _ _ _ _ _ _ _ _ _ _ _ _ _ _ _ _ _ _ _ _ _ _ _ _ _ _ _ _ _ _ _ _ _ _ _ _ _ _ _ _ _ _ _ _ _ _ _ _ _ _ _ _ _ _ _ _ _ _ _ _ _ _ _ _ _ _ _ _ _ _ _ _ _ _ _ _ _ _ _ _ _ _ _ _ _ _ _ _ _ _ _ _]
      tunnel: w84 -> [_ _ _ _ _ _ _ _ _ _ _ _ _ _ _ _ _ _ _ _ w1033 _ _ _ _ _ _ _ _ _ _ _ _ _ _ _ _ _ _ _ _ _ _ _ _ _ _ _ _ _ _ _ _ _ _ _ _ _ _ _ _ _ _ _ _ _ _ _ _ _ _ _ _ _ _ _ w2013 w2022 _ _ _ _ _ _ _ _ _ _ _ _ _ _ _ _ _ _ _ _ _ _ _ _ _ _ _ _ _ _ _ _ _ _ _ _ _ _ _ _ _ _ _ _ _ _ _ _ _ _ _ _ _ _ _ _ _ _ _ _ _ _ _ _ _ _ _ _ _ _ _ _ _ _ _ _ _ _ _ _ _ _ _ _ _ _ _ _ _ _ _ _ _ _ _ _ _ _ _ _ _ _ _ _ _ _]
      tunnel: w83 -> [w96 _ _ _ _ _ _ _ _ _ _ _ _ _ _ _ _ _ _ _ _ _ _ _ _ _ _ _ _ _ _ _ _ _ _ _ _ _ _ _ _ _ _ _ _ _ _ w1539 _ _ _ _ _ _ _ _ _ _ _ _ _ _ _ _ _ _ _ _ _ _ _ _ _ _ _ _ _ _ _ _ _ _ _ _ _ _ _ _ _ _ _ _ _ _ _ _ _ _ _ _ _ _ _ _ _ _ _ _ _ _ _ _ _ _ _ _ _ _ _ _ _ _ _ _ _ _ _ _ _ _ _ _ _ _ _ _ _ _ _ _ _ _ _ _ _ _ _ _ _ _ _ _ _ _ _ _ _ _ _ _ _ _ _ _ _ _ _ _ _ _ _ _ _ _ _ _ _ _ _ _ _ _ _ _]
      tunnel: w82 -> [w95 w511 w521 w526 w532 w547 w567 w596 w616 w644 w663 w734 w749 w778 w807 w839 w870 w899 w911 w998 w1035 w1074 w1083 w1090 w1095 w1113 w1132 w1155 w1160 w1174 w1193 w1222 w1242 w1285 w1291 w1301 w1312 w1342 w1350 w1355 w1363 w1387 w1412 w1436 w1456 w1465 w1489 w1544 w1560 w1573 w1582 w1598 w1612 w1641 w1667 w1672 w1717 w1722 w1734 w1741 w1750 w1762 w1793 w1809 w1823 w1843 w1858 w1889 w1905 w1915 w1931 w1943 w1955 w1983 w1986 w2001 w2014 w2021 w2030 w2039 w2047 w2054 w2063 w2069 w2079 w2082 w2094 w2113 w2128 w2147 w2169 w2187 w2203 w2207 w2215 w2223 w2228 w2236 w2243 w2251 w2258 w2268 w2296 w2304 w2311 w2316 w2324 w2333 w2339 w2345 w2354 w2366 w2375 w2380 w2391 w2464 w2469 w2481 w2491 w2504 w2521 w2550 w2565 w2578 w2590 w2614 w2634 w2642 w2655 w2683 w2688 w2694 w2700 w2707 w2718 w2730 w2738 w2743 w2755 w2760 w2771 w2776 w2782 w2787 w2792 w2797 w2807 w2832 w2853 w2857 w2869 w2894 w2921 w2944 w2948 w2964 w3016 w3062 w3103 w3118 w3136 w3156 w3170 w3182 w3191 w3208 w3230 w3254 w3273 w3291 w3309 w3327 w3341 w3355 w3374 w3388 w3403 w3416 w3426 w3430 w3447 w3455 w3461 w3466]
      tunnel: [w94 w511 w521 w526 w532 w547 w567 w596 w616 w644 w663 w734 w749 w778 w807 w839 w870 w899 w911 w998 w1035 w1074 w1083 w1090 w1095 w1113 w1132 w1155 w1160 w1174 w1193 w1222 w1242 w1285 w1291 w1301 w1312 w1342 w1350 w1355 w1363 w1387 w1412 w1436 w1456 w1465 w1489 w1544 w1560 w1573 w1582 w1598 w1612 w1641 w1667 w1672 w1717 w1722 w1734 w1741 w1750 w1762 w1793 w1809 w1823 w1843 w1858 w1889 w1905 w1915 w1931 w1943 w1955 w1983 w1986 w2001 w2014 w2021 w2030 w2039 w2047 w2054 w2063 w2069 w2079 w2082 w2094 w2113 w2128 w2147 w2169 w2187 w2203 w2207 w2215 w2223 w2228 w2236 w2243 w2251 w2258 w2268 w2296 w2304 w2311 w2316 w2324 w2333 w2339 w2345 w2354 w2366 w2375 w2380 w2391 w2464 w2469 w2481 w2491 w2504 w2521 w2550 w2565 w2578 w2590 w2614 w2634 w2642 w2655 w2683 w2688 w2694 w2700 w2707 w2718 w2730 w2738 w2743 w2755 w2760 w2771 w2776 w2782 w2787 w2792 w2797 w2807 w2832 w2853 w2857 w2869 w2894 w2921 w2944 w2948 w2964 w3016 w3062 w3103 w3118 w3136 w3156 w3170 w3182 w3191 w3208 w3230 w3254 w3273 w3291 w3309 w3327 w3341 w3355 w3374 w3388 w3403 w3416 w3426 w3430 w3447 w3455 w3461 w3466] -> w81
      tunnel: w77 -> [_ _ _ _ _ _ _ _ _ _ _ _ _ _ _ _ _ _ _ _ w1028 _ _ _ _ _ _ _ _ _ _ _ _ _ _ _ _ _ _ _ _ _ _ _ _ _ _ _ _ _ _ _ _ _ _ _ _ _ _ _ _ _ _ _ _ _ _ _ _ _ _ _ _ _ _ _ w2011 w2020 _ _ _ _ _ _ _ _ _ _ _ _ _ _ _ _ _ _ _ _ _ _ _ _ _ _ _ _ _ _ _ _ _ _ _ _ _ _ _ _ _ _ _ _ _ _ _ _ _ _ _ _ _ _ _ _ _ _ _ _ _ _ _ _ _ _ _ _ _ _ _ _ _ _ _ _ _ _ _ _ _ _ _ _ _ _ _ _ _ _ _ _ _ _ _ _ _ _ _ _ _ _ _ _ _ _]
      frame "", "Event Structure", "Idle" {
        # "executes when the state queue is empty"
        n31 = event shown="[37] <AcqLoop error?>: User Event" {
          selector: w95 -> [_ _ _ _ _ _ _ _ _ _ _ _ _ _ _ _ _ _ _ _ _ _ _ _ _ _ _ _ _ _ _ _ _ _ _ _ _ _ _]
          dyn-events: [_ _ _ _ _ _ _ _ _ _ _ _ _ _ _ _ _ _ _ _ _ _ _ _ _ _ _ _ _ _ _ _ _ _ _ _ _ _ _] -> w94
          timeout: w97 -> [_ _ _ _ _ _ _ _ _ _ _ _ _ _ _ _ _ _ _ _ _ _ _ _ _ _ _ _ _ _ _ _ _ _ _ _ _ _ _]
          tunnel: w102 -> [w122 w141 w149 w153 w157 w165 w171 w179 w187 w197 w204 w233 w253 w273 w293 w297 w304 w327 w341 w355 w369 w374 w377 w383 w390 w397 w403 w409 w415 w422 w435 w446 w458 w465 w469 w473 w480 w494 w510]
          tunnel: [w123 w141 w148 w153 w156 w165 w171 w179 w187 w197 w203 w233 w253 w273 w293 w297 w303 w327 w341 w355 w369 w373 w376 w383 w391 w398 w402 w408 w415 w423 w436 w446 w459 w465 w469 w472 w479 w495 w509] -> w101
          tunnel: w100 -> [w106 w139 w143 w151 w158 w164 w172 w180 w188 w195 w199 w231 w251 w271 w291 w295 w299 w326 w340 w354 w368 w370 w378 w381 w386 w393 w405 w410 w413 w417 w430 w444 w454 w463 w467 w474 w481 w492 w507]
          tunnel: [w121 w140 w144 w152 w159 w163 w170 w178 w186 w196 w205 w232 w252 w272 w292 w296 w305 w324 w328 w351 w366 w372 w379 w382 w387 w394 w406 w411 w414 w421 w434 w445 w455 w464 w468 w475 w482 w496 w508] -> w93
          tunnel: w99 -> [w121 w140 w144 w152 w159 w163 w170 w178 w186 w196 w205 w232 w252 w272 w292 w296 w305 w321 w330 w342 w358 w372 w379 w382 w387 w394 w406 w411 w414 w421 w434 w445 w457 w464 w468 w475 w482 w496 w508]
          tunnel: [w106 w139 w143 w151 w158 w164 w172 w180 w188 w195 w200 w231 w251 w271 w291 w295 w300 w326 w340 w354 w368 w370 w378 w381 w388 w395 w405 w410 w413 w418 w431 w444 w460 w463 w467 w474 w481 w493 w507] -> w98
          tunnel: w96 -> [_ _ _ _ _ _ _ _ _ _ _ _ _ _ _ _ _ _ _ _ _ _ _ _ _ _ _ _ _ _ _ _ _ _ _ _ _ _ _]
          event Timeout {
            # "check system status every 2s"
            n32 = event-data() -> ()  [unwired: 1 in, 1 out]
            n33 = Unbundle By Name(w106) -> ("SysRunning?"=w104:bool, "SlowTimer"=w120:u32, "FastTimer"=w114:u32)
            n34 = Tick Count (ms)() -> (millisecond timer value=w107:u32)
            n35 = Subtract(x=w107, y=w120) -> (x-y=w117:u32)
            n36 = case shown="False" w104 {
              tunnel: ["" "Utility: AquiTimerCheck" ("State(s) in Front (\"\")")] -> w112
              frame False {
                # "if not running, do nothing"
              }
              frame True {
                # "if aquisition is running, check timer"
              }
            }
            n37 = Subtract(x=w107, y=w114) -> (x-y=w115:u32)
            n38 = Greater?(x=w117, y=u32 2000) -> (0:w118:bool)
            n39 = Greater?(x=w115, y=u32 500) -> (0:w105:bool)
            n40 = disable-structure shown="Enabled" {
              disable-tunnel: w105 -> [w128 _]
              disable-tunnel: w104 -> [w127 _]
              disable-tunnel: [w124 "" ("State(s) at Back (\"\")")] -> w103
              frame Disabled {
                n41 = Not(x=w127) -> (.not. x?=w126:bool)
                n42 = And(x=w128, y=w126) -> (x .and. y?=w125:bool)
                n43 = case shown="True" w125 {
                  tunnel: ["" ("Empty String Constant") "TCP: checkSource" ("State(s) in Front (\"\")")] -> w124
                  frame False {
                  }
                  frame True {
                  }
                }
              }
              frame Enabled {
              }
            }
            n44 = case shown="True" w118 {
              tunnel: ["" ("Empty String Constant") "SystemStatus: SlowSysStatusMacro" ("State(s) in Front (\"\")")] -> w110
              frame False {
              }
              frame True {
              }
            }
            n45 = case shown="True" w105 {
              tunnel: ["" ("Empty String Constant") "SystemStatus: FastSysStatusMacro" ("State(s) in Front (\"\")")] -> w108
              frame False {
              }
              frame True {
              }
            }
            n46 = call <vilib>:"Add State(s) to Queue__JKI_lib_State_Machine.vi"("State(s) in Front (\"\")"=w112, "State(s) in (\"\")"="LabJack: checkPedal" ("State(s) in Front (\"\")"), "State(s) at Back (\"\")"=w110) -> ("States Out"=w109:string)  [unwired: 12 in]
            n47 = call <vilib>:"Add State(s) to Queue__JKI_lib_State_Machine.vi"("State(s) in Front (\"\")"=w109, "State(s) in (\"\")"=w108, "State(s) at Back (\"\")"=w103) -> ("States Out"=w113:string)  [unwired: 12 in]
            n48 = call <vilib>:"Add State(s) to Queue__JKI_lib_State_Machine.vi"("State(s) in Front (\"\")"=w113, "State(s) in (\"\")"=w122) -> ("States Out"=w123:string)  [unwired: 13 in]
          }
          event "355nm Laser toggle": Mouse Enter {
            n49 = event-data() -> ()  [unwired: 1 in, 4 out]
            n50 = local write "Help"("Toggle 355nm laser." ("Help")) -> ()
          }
          event "355nm Laser toggle": Value Change {
            # "[Covers: REQ34]"
            n51 = event-data() -> ()  [unwired: 1 in, 6 out]
            n52 = Select(t="LabJack: 355_PWM_Start\nLabJack: AB_Start", s="355nm Laser toggle", f="LabJack: 355_PWM_Stop\nLabJack: AB_Stop") -> (s? t:f=w146:string)
            n53 = call <vilib>:"Add State(s) to Queue__JKI_lib_State_Machine.vi"("State(s) in Front (\"\")"=w146, "State(s) in (\"\")"=w149) -> ("States Out"=w148:string)  [unwired: 13 in]
          }
          event "Aiming beam toggle": Mouse Enter {
            n54 = event-data() -> ()  [unwired: 1 in, 4 out]
            n55 = local write "Help"("Toggle aiming beam laser." ("Help")) -> ()
          }
          event "Aiming beam toggle": Value Change {
            # "[Covers: REQ33]"
            n56 = event-data() -> ()  [unwired: 1 in, 6 out]
            n57 = case shown="True" "Aiming beam toggle" {
              tunnel: ["LabJack: AB_Stop" ("State(s) in Front (\"\")") "LabJack: AB_Start" ("State(s) in Front (\"\")")] -> w155
              frame False {
              }
              frame True {
              }
            }
            n58 = call <vilib>:"Add State(s) to Queue__JKI_lib_State_Machine.vi"("State(s) in Front (\"\")"=w155, "State(s) in (\"\")"=w157) -> ("States Out"=w156:string)  [unwired: 13 in]
          }
          event "Auto gain ch1": Value Change {
            n59 = event-data() -> ("NewVal"=w162:bool)  [unwired: 1 in, 5 out]
            n60 = case shown="True" w162 {
              frame False {
                n61 = local read "V 1"() -> (w166:dbl)
                n62 = call "V1FGV.vi"("action (write)"=enum16{"write", "read"}."write" ("action"), "V1 in"=w166) -> ()  [unwired: 8 in, 2 out]
                n63 = property on="V 1" class="DigNum (strict)"("DisabledEnum"=T11."Enabled" ("Disabled")) -> ()  [unwired: 2 in, 2 out]
              }
              frame True {
                n64 = property on="V 1" class="DigNum (strict)"("DisabledEnum"=T11."Disabled and Grayed Out" ("Disabled")) -> ()  [unwired: 2 in, 2 out]
              }
            }
          }
          event "Auto gain ch2": Value Change {
            n65 = event-data() -> ("NewVal"=w173:bool)  [unwired: 1 in, 5 out]
            n66 = case shown="False" w173 {
              frame False {
                n67 = local read "V 2"() -> (w174:dbl)
                n68 = property on="V 2" class="DigNum (strict)"("DisabledEnum"=T11."Enabled" ("Disabled")) -> ()  [unwired: 2 in, 2 out]
                n69 = call "V2FGV.vi"("action(write)"=enum16{"write", "read"}."write" ("action"), "V2 in"=w174) -> ()  [unwired: 8 in, 2 out]
              }
              frame True {
                n70 = property on="V 2" class="DigNum (strict)"("DisabledEnum"=T11."Disabled and Grayed Out" ("Disabled")) -> ()  [unwired: 2 in, 2 out]
              }
            }
          }
          event "Auto gain ch3": Value Change {
            n71 = event-data() -> ("NewVal"=w181:bool)  [unwired: 1 in, 5 out]
            n72 = case shown="False" w181 {
              frame False {
                n73 = local read "V 3"() -> (w182:dbl)
                n74 = property on="V 3" class="DigNum (strict)"("DisabledEnum"=T11."Enabled" ("Disabled")) -> ()  [unwired: 2 in, 2 out]
                n75 = call "V3FGV.vi"("action(write)"=enum16{"write", "read"}."write" ("action"), "V3 in"=w182) -> ()  [unwired: 8 in, 2 out]
              }
              frame True {
                n76 = property on="V 3" class="DigNum (strict)"("DisabledEnum"=T11."Disabled and Grayed Out" ("Disabled")) -> ()  [unwired: 2 in, 2 out]
              }
            }
          }
          event "Auto gain ch4": Value Change {
            n77 = event-data() -> ("NewVal"=w189:bool)  [unwired: 1 in, 5 out]
            n78 = case shown="False" w189 {
              frame False {
                n79 = local read "V 4"() -> (w190:dbl)
                n80 = property on="V 4" class="DigNum (strict)"("DisabledEnum"=T11."Enabled" ("Disabled")) -> ()  [unwired: 2 in, 2 out]
                n81 = call "V4FGV.vi"("action(write)"=enum16{"write", "read"}."write" ("action"), "V3 in"=w190) -> ()  [unwired: 8 in, 2 out]
              }
              frame True {
                n82 = property on="V 4" class="DigNum (strict)"("DisabledEnum"=T11."Disabled and Grayed Out" ("Disabled")) -> ()  [unwired: 2 in, 2 out]
              }
            }
          }
          event "Background": Mouse Enter {
            n83 = event-data() -> ()  [unwired: 1 in, 4 out]
            n84 = local write "Help"("Click to record a background." ("Help")) -> ()
          }
          event "Background": Value Change {
            n85 = event-data() -> ("NewVal"=w201:bool)  [unwired: 1 in, 5 out]
            n86 = case shown="True" w201 {
              tunnel: ["Utility: SetAllChanManualGain\nQueue: Flash\nUtility: Dewelling >> 2500\nLabJack: 355_PWM_Stop\nLabJack: AB_Stop" "Utility: SetDataClass >> Bg\nUI: Update\nLabJack: 355_PWM_Start\nLabJack: AB_Start\nUtility: SaveDeconChan\nUtility: Dewelling >> 50\nLabJack: SetV\nDigitizer: Start\nUtility: AquiTimerReset\nLED: BreathGreen\nUI: duringBGAcquire"] -> w202
              tunnel: [FALSE TRUE] -> w198
              frame False {
                n87 = local read "Skip Data Save?"() -> (w206:bool)
                n88 = case shown="False" w206 {
                  frame False {
                    n89 = property on="Background" class="Bool (strict)"("BoolText.Text"="Done!" ("Boolean Text.Text")) -> ()  [unwired: 2 in, 2 out]
                  }
                  frame True {
                  }
                }
              }
              frame True {
                # "[Covers: REQ6]"
                n90 = property on="Background" class="Bool (strict)"("BoolText.Text"="Running" ("Boolean Text.Text"), "Colors [4]"=cluster{u32, u32}[] [{6618880, 6618880}, {16711680, 16711680}]) -> ()  [unwired: 2 in, 2 out]
              }
            }
            n91 = Bundle By Name(cluster=w199, "SysRunning?"=w198) -> (w200:T23)
            n92 = call <vilib>:"Add State(s) to Queue__JKI_lib_State_Machine.vi"("State(s) in Front (\"\")"=w202, "State(s) in (\"\")"=w204) -> ("States Out"=w203:string)  [unwired: 13 in]
          }
          event "Channel 1": Cursor Move {
            n93 = event-data() -> ("CursIdx"=w217:i32, "CursLoc"=w229:cluster{"X":dbl, "Y":dbl})  [unwired: 1 in, 7 out]
            n94 = property on="Channel 3" class="WFGraph (strict)"() -> ("CrsrList"=w224:T24)  [unwired: 2 in, 2 out]
            n95 = property on="Channel 4" class="WFGraph (strict)"() -> ("CrsrList"=w216:T24)  [unwired: 2 in, 2 out]
            n96 = property on="Channel 2" class="WFGraph (strict)"() -> ("CrsrList"=w227:T24)  [unwired: 2 in, 2 out]
            n97 = Index Array(array=w224, index=w217) -> (element=w228:T25)
            n98 = Index Array(array=w216, index=w217) -> (element=w219:T25)
            n99 = Unbundle By Name(w229) -> ("X"=w218:dbl)
            n100 = Index Array(array=w227, index=w217) -> (element=w230:T25)
            n101 = Bundle By Name(cluster=w228, "Position.X"=w218) -> (w223:T25)
            n102 = Bundle By Name(cluster=w219, "Position.X"=w218) -> (w215:T25)
            n103 = Bundle By Name(cluster=w230, "Position.X"=w218) -> (w226:T25)
            n104 = control-ref of="Channel 1"() -> (w220:refnum<vi>)
            n105 = Replace Array Subset(array=w224, new element=w223, index=w217) -> (w222:T24)
            n106 = Replace Array Subset(array=w216, new element=w215, index=w217) -> (w214:T24)
            n107 = Replace Array Subset(array=w227, new element=w226, index=w217) -> (w225:T24)
            n108 = property on="Channel 3" class="WFGraph (strict)"("CrsrList"=w222) -> (error out=w221:errorcluster)  [unwired: 2 in, 1 out]
            n109 = property on="Channel 4" class="WFGraph (strict)"("CrsrList"=w214) -> ()  [unwired: 2 in, 2 out]
            n110 = property on="Channel 2" class="WFGraph (strict)"("CrsrList"=w225) -> ()  [unwired: 2 in, 2 out]
            n111 = call "UpdateCurserIdx(SubVI).vi"("error in (no error)"=w221, "WaveformGraph in"=w220) -> ()  [unwired: 9 in, 1 out]
          }
          event "Channel 2": Cursor Move {
            n112 = event-data() -> ("CursIdx"=w236:i32, "CursLoc"=w250:cluster{"X":dbl, "Y":dbl})  [unwired: 1 in, 7 out]
            n113 = Unbundle By Name(w250) -> ("X"=w238:dbl)
            n114 = property on="Channel 1" class="WFGraph (strict)"() -> ("CrsrList"=w244:T24)  [unwired: 2 in, 2 out]
            n115 = property on="Channel 3" class="WFGraph (strict)"() -> ("CrsrList"=w246:T24)  [unwired: 2 in, 2 out]
            n116 = property on="Channel 4" class="WFGraph (strict)"() -> ("CrsrList"=w237:T24)  [unwired: 2 in, 2 out]
            n117 = Index Array(array=w244, index=w236) -> (element=w249:T25)
            n118 = Index Array(array=w246, index=w236) -> (element=w248:T25)
            n119 = Index Array(array=w237, index=w236) -> (element=w239:T25)
            n120 = Bundle By Name(cluster=w239, "Position.X"=w238) -> (w235:T25)
            n121 = Bundle By Name(cluster=w249, "Position.X"=w238) -> (w247:T25)
            n122 = Bundle By Name(cluster=w248, "Position.X"=w238) -> (w245:T25)
            n123 = Replace Array Subset(array=w244, new element=w247, index=w236) -> (w243:T24)
            n124 = Replace Array Subset(array=w246, new element=w245, index=w236) -> (w242:T24)
            n125 = Replace Array Subset(array=w237, new element=w235, index=w236) -> (w234:T24)
            n126 = control-ref of="Channel 1"() -> (w241:refnum<vi>)
            n127 = property on="Channel 1" class="WFGraph (strict)"("CrsrList"=w243) -> ()  [unwired: 2 in, 2 out]
            n128 = property on="Channel 3" class="WFGraph (strict)"("CrsrList"=w242) -> (error out=w240:errorcluster)  [unwired: 2 in, 1 out]
            n129 = property on="Channel 4" class="WFGraph (strict)"("CrsrList"=w234) -> ()  [unwired: 2 in, 2 out]
            n130 = call "UpdateCurserIdx(SubVI).vi"("error in (no error)"=w240, "WaveformGraph in"=w241) -> ()  [unwired: 9 in, 1 out]
          }
          event "Channel 3": Cursor Move {
            n131 = event-data() -> ("CursIdx"=w256:i32, "CursLoc"=w270:cluster{"X":dbl, "Y":dbl})  [unwired: 1 in, 7 out]
            n132 = Unbundle By Name(w270) -> ("X"=w258:dbl)
            n133 = property on="Channel 4" class="WFGraph (strict)"() -> ("CrsrList"=w257:T24)  [unwired: 2 in, 2 out]
            n134 = property on="Channel 1" class="WFGraph (strict)"() -> ("CrsrList"=w267:T24)  [unwired: 2 in, 2 out]
            n135 = property on="Channel 2" class="WFGraph (strict)"() -> ("CrsrList"=w265:T24)  [unwired: 2 in, 2 out]
            n136 = Index Array(array=w257, index=w256) -> (element=w259:T25)
            n137 = Index Array(array=w267, index=w256) -> (element=w269:T25)
            n138 = Index Array(array=w265, index=w256) -> (element=w268:T25)
            n139 = Bundle By Name(cluster=w259, "Position.X"=w258) -> (w255:T25)
            n140 = Bundle By Name(cluster=w269, "Position.X"=w258) -> (w266:T25)
            n141 = Bundle By Name(cluster=w268, "Position.X"=w258) -> (w264:T25)
            n142 = Replace Array Subset(array=w257, new element=w255, index=w256) -> (w254:T24)
            n143 = Replace Array Subset(array=w267, new element=w266, index=w256) -> (w263:T24)
            n144 = Replace Array Subset(array=w265, new element=w264, index=w256) -> (w262:T24)
            n145 = control-ref of="Channel 1"() -> (w260:refnum<vi>)
            n146 = property on="Channel 4" class="WFGraph (strict)"("CrsrList"=w254) -> ()  [unwired: 2 in, 2 out]
            n147 = property on="Channel 1" class="WFGraph (strict)"("CrsrList"=w263) -> ()  [unwired: 2 in, 2 out]
            n148 = property on="Channel 2" class="WFGraph (strict)"("CrsrList"=w262) -> (error out=w261:errorcluster)  [unwired: 2 in, 1 out]
            n149 = call "UpdateCurserIdx(SubVI).vi"("error in (no error)"=w261, "WaveformGraph in"=w260) -> ()  [unwired: 9 in, 1 out]
          }
          event "Channel 4": Cursor Move {
            n150 = event-data() -> ("CursIdx"=w278:i32, "CursLoc"=w290:cluster{"X":dbl, "Y":dbl})  [unwired: 1 in, 7 out]
            n151 = Unbundle By Name(w290) -> ("X"=w276:dbl)
            n152 = property on="Channel 1" class="WFGraph (strict)"() -> ("CrsrList"=w288:T24)  [unwired: 2 in, 2 out]
            n153 = property on="Channel 2" class="WFGraph (strict)"() -> ("CrsrList"=w284:T24)  [unwired: 2 in, 2 out]
            n154 = property on="Channel 3" class="WFGraph (strict)"() -> ("CrsrList"=w279:T24)  [unwired: 2 in, 2 out]
            n155 = Index Array(array=w288, index=w278) -> (element=w289:T25)
            n156 = Index Array(array=w284, index=w278) -> (element=w285:T25)
            n157 = Index Array(array=w279, index=w278) -> (element=w281:T25)
            n158 = Bundle By Name(cluster=w289, "Position.X"=w276) -> (w287:T25)
            n159 = Bundle By Name(cluster=w285, "Position.X"=w276) -> (w283:T25)
            n160 = Bundle By Name(cluster=w281, "Position.X"=w276) -> (w280:T25)
            n161 = Replace Array Subset(array=w288, new element=w287, index=w278) -> (w286:T24)
            n162 = Replace Array Subset(array=w284, new element=w283, index=w278) -> (w282:T24)
            n163 = Replace Array Subset(array=w279, new element=w280, index=w278) -> (w277:T24)
            n164 = control-ref of="Channel 1"() -> (w274:refnum<vi>)
            n165 = call "UpdateCurserIdx(SubVI).vi"() -> ()  [unwired: 11 in, 1 out]
            n166 = call "UpdateCurserIdx(SubVI).vi"() -> ()  [unwired: 11 in, 1 out]
            n167 = property on="Channel 1" class="WFGraph (strict)"("CrsrList"=w286) -> ()  [unwired: 2 in, 2 out]
            n168 = property on="Channel 2" class="WFGraph (strict)"("CrsrList"=w282) -> ()  [unwired: 2 in, 2 out]
            n169 = property on="Channel 3" class="WFGraph (strict)"("CrsrList"=w277) -> (error out=w275:errorcluster)  [unwired: 2 in, 1 out]
            n170 = call "UpdateCurserIdx(SubVI).vi"("error in (no error)"=w275, "WaveformGraph in"=w274) -> ()  [unwired: 9 in, 1 out]
          }
          event "Cali&iRF alignment": Mouse Enter {
            n171 = event-data() -> ()  [unwired: 1 in, 4 out]
            n172 = local write "Help"("Click to run system intensity calibration and irf alignment" ("Help")) -> ()
          }
          event "Cali&iRF alignment": Value Change {
            n173 = event-data() -> ("NewVal"=w301:bool)  [unwired: 1 in, 5 out]
            n174 = case shown="False" w301 {
              tunnel: ["Utility: SetAllChanManualGain\nQueue: Flash\nUtility: Dewelling >> 2500\nLabJack: 355_PWM_Stop\nLabJack: AB_Stop" "Utility: SetDataClass >> Cali\nUI: Update\nUtility: SaveDeconChan\nLabJack: 355_PWM_Start\nLabJack: AB_Start\nLabJack: SetV\nDigitizer: Start\nUtility: AquiTimerReset\nLED: BreathGreen\nUI: duringIRFAlign"] -> w302
              tunnel: [FALSE TRUE] -> w298
              frame False {
                n175 = local read "Skip Data Save?"() -> (w306:bool)
                n176 = case shown="False" w306 {
                  frame False {
                    n177 = property on="Cali&iRF alignment" class="Bool (strict)"("BoolText.Text"="Done!" ("Boolean Text.Text")) -> ()  [unwired: 2 in, 2 out]
                  }
                  frame True {
                  }
                }
              }
              frame True {
                n178 = property on="Cali&iRF alignment" class="Bool (strict)"("BoolText.Text"="Running" ("Boolean Text.Text"), "Colors [4]"=cluster{u32, u32}[] [{6618880, 6618880}, {16711680, 16711680}]) -> ()  [unwired: 2 in, 2 out]
              }
            }
            n179 = Bundle By Name(cluster=w299, "SysRunning?"=w298) -> (w300:T23)
            n180 = call <vilib>:"Add State(s) to Queue__JKI_lib_State_Machine.vi"("State(s) in Front (\"\")"=w302, "State(s) in (\"\")"=w304) -> ("States Out"=w303:string)  [unwired: 13 in]
          }
          event "V 1": Value Change {
            n181 = event-data() -> ()  [unwired: 1 in, 6 out]
            n182 = call "LabJack_FGV.vi"("Operation(Read)"=enum16{"Write", "Read"}."Read" ("Operation"), "error in (no error)"=w321) -> ("error out"=w318:errorcluster, "Read data"=w319:i32)  [unwired: 8 in]
            n183 = global read "GlobalVariables.vi" "Ch1 LJ pin"() -> (w317:string)
            n184 = call "LJM_eWriteName.vi"("Handle In"=w319, "Name"=w317, "Value"="V 1", "error in"=w318) -> ("error out"=w315:errorcluster)  [unwired: 10 in, 1 out]
            n185 = call "V1FGV.vi"("Error In"=w315, "action (write)"=enum16{"write", "read"}."write" ("action"), "V1 in"="V 1") -> ("Error Out"=w314:errorcluster)  [unwired: 7 in, 1 out]
            n186 = call "CtrlVtoGain.vi"("error in (no error)"=w314, "CtrlV(V)"="V 1", "Channel"=enum16{"Ch1", "Ch2", "Ch3"}."Ch1" ("Enum")) -> ("error out"=w324:errorcluster, "Gain"=w323:dbl)  [unwired: 7 in]
            n187 = local write "Gain1"(w323) -> ()
          }
          event "V 2": Value Change {
            n188 = event-data() -> ()  [unwired: 1 in, 6 out]
            n189 = call "LabJack_FGV.vi"("Operation(Read)"=enum16{"Write", "Read"}."Read" ("Operation"), "error in (no error)"=w330) -> ("error out"=w335:errorcluster, "Read data"=w336:i32)  [unwired: 8 in]
            n190 = global read "GlobalVariables.vi" "Ch2 LJ pin"() -> (w334:string)
            n191 = call "LJM_eWriteName.vi"("Handle In"=w336, "Name"=w334, "Value"="V 2", "error in"=w335) -> ("error out"=w333:errorcluster)  [unwired: 10 in, 1 out]
            n192 = call "V2FGV.vi"("Error In"=w333, "action(write)"=enum16{"write", "read"}."write" ("action"), "V2 in"="V 2") -> ("Error Out"=w332:errorcluster)  [unwired: 7 in, 1 out]
            n193 = call "CtrlVtoGain.vi"("error in (no error)"=w332, "CtrlV(V)"="V 2", "Channel"=enum16{"Ch1", "Ch2", "Ch3"}."Ch2" ("Enum")) -> ("error out"=w328:errorcluster, "Gain"=w329:dbl)  [unwired: 7 in]
            n194 = local write "Gain2"(w329) -> ()
          }
          event "V 3": Value Change {
            n195 = event-data() -> ()  [unwired: 1 in, 6 out]
            n196 = call "LabJack_FGV.vi"("Operation(Read)"=enum16{"Write", "Read"}."Read" ("Operation"), "error in (no error)"=w342) -> ("error out"=w347:errorcluster, "Read data"=w348:i32)  [unwired: 8 in]
            n197 = global read "GlobalVariables.vi" "Ch3 LJ pin"() -> (w346:string)
            n198 = call "LJM_eWriteName.vi"("Handle In"=w348, "Name"=w346, "Value"="V 3", "error in"=w347) -> ("error out"=w344:errorcluster)  [unwired: 10 in, 1 out]
            n199 = call "V3FGV.vi"("Error In"=w344, "action(write)"=enum16{"write", "read"}."write" ("action"), "V3 in"="V 3") -> ("Error Out"=w343:errorcluster)  [unwired: 7 in, 1 out]
            n200 = call "CtrlVtoGain.vi"("error in (no error)"=w343, "CtrlV(V)"="V 3", "Channel"=enum16{"Ch1", "Ch2", "Ch3"}."Ch3" ("Enum")) -> ("error out"=w351:errorcluster, "Gain"=w350:dbl)  [unwired: 7 in]
            n201 = local write "Gain3"(w350) -> ()
          }
          event "V 4": Value Change {
            n202 = event-data() -> ()  [unwired: 1 in, 6 out]
            n203 = call "LabJack_FGV.vi"("Operation(Read)"=enum16{"Write", "Read"}."Read" ("Operation"), "error in (no error)"=w358) -> ("error out"=w362:errorcluster, "Read data"=w363:i32)  [unwired: 8 in]
            n204 = global read "GlobalVariables.vi" "Ch4 LJ pin"() -> (w361:string)
            n205 = call "LJM_eWriteName.vi"("Handle In"=w363, "Name"=w361, "Value"="V 4", "error in"=w362) -> ("error out"=w360:errorcluster)  [unwired: 10 in, 1 out]
            n206 = call "V4FGV.vi"("Error In"=w360, "action(write)"=enum16{"write", "read"}."write" ("action"), "V3 in"="V 4") -> ("Error Out"=w359:errorcluster)  [unwired: 7 in, 1 out]
            n207 = call "CtrlVtoGain.vi"("error in (no error)"=w359, "CtrlV(V)"="V 4", "Channel"=enum16{"Ch1", "Ch2", "Ch3", "Ch4"}."Ch4") -> ("error out"=w366:errorcluster, "Gain"=w365:dbl)  [unwired: 7 in]
            n208 = local write "Gain4"(w365) -> ()
          }
          event "Quit": Value Change {
            # "Exit Button Value Change (pressed) Event\n(when pressed.  quite)"
            n209 = event-data() -> ()  [unwired: 1 in, 1 out]
            n210 = call <vilib>:"Add State(s) to Queue__JKI_lib_State_Machine.vi"("State(s) in Front (\"\")"="LED: Off\nMacro: Exit", "State(s) in (\"\")"=w374) -> ("States Out"=w373:string)  [unwired: 13 in]
          }
          event "Show BG": Value Change {
            n211 = event-data() -> ()  [unwired: 1 in, 6 out]
            n212 = call <vilib>:"Add State(s) to Queue__JKI_lib_State_Machine.vi"("State(s) in Front (\"\")"="Data: showBG" ("State(s) in Front (\"\")"), "State(s) in (\"\")"=w377) -> ("States Out"=w376:string)  [unwired: 13 in]
          }
          event "StartButton": Mouse Enter {
            n213 = event-data() -> ()  [unwired: 1 in, 4 out]
            n214 = local write "Help"("Press to start aquisition." ("Help")) -> ()
          }
          event "StartButton": Value Change {
            # "[Covers: REQ32]"
            # "start PWM before acquisition"
            # "Initialize both digitizer aquisition and\n send user event to trigger aquisition loop"
            n215 = event-data() -> ()  [unwired: 1 in, 6 out]
            n216 = local write "StartButton"(FALSE ("StartButton")) -> ()
            n217 = Bundle By Name(cluster=w386, "SysRunning?"=TRUE) -> (w388:T23)
            n218 = call <vilib>:"Add State(s) to Queue__JKI_lib_State_Machine.vi"("State(s) in Front (\"\")"="TCP: stopCam\nUtility: SetDataClass >> Data\nQueue: Flash\nUI: Update\nUtility: StartBeep\nLabJack: 355_PWM_Start\nLabJack: AB_Start\nLabJack: SetV\nDigitizer: Start\nUtility: AquiTimerReset\nUI: DuringAquisition\nLED: BreathGreen\nTCP: sendRunNum\nTCP: sendVideoSource\nTCP: sendChannel\nTCP: startRun", "State(s) in (\"\")"=w390) -> ("States Out"=w391:string)  [unwired: 13 in]
          }
          event User Event {
            # "[Covers: REQ32]"
            # "start PWM before acquisition"
            # "Initialize both digitizer aquisition and\n send user event to trigger aquisition loop"
            n219 = event-data() -> ()  [unwired: 1 in, 5 out]
            n220 = Bundle By Name(cluster=w393, "SysRunning?"=TRUE) -> (w395:T23)
            n221 = call <vilib>:"Add State(s) to Queue__JKI_lib_State_Machine.vi"("State(s) in Front (\"\")"="TCP: stopCam\nUtility: SetDataClass >> Data\nQueue: Flash\nUI: Update\nUtility: StartBeep\nLabJack: 355_PWM_Start\nLabJack: AB_Start\nLabJack: SetV\nDigitizer: Start\nUtility: AquiTimerReset\nUI: DuringAquisition\nLED: BreathGreen\nTCP: sendRunNum\nTCP: sendVideoSource\nTCP: sendChannel\nTCP: startRun", "State(s) in (\"\")"=w397) -> ("States Out"=w398:string)  [unwired: 13 in]
          }
          event "Video Display": Value Change {
            n222 = event-data() -> ("NewVal"=w404:bool)  [unwired: 1 in, 5 out]
            n223 = Select(t="TCP: startCam", s=w404, f="TCP: stopCam") -> (s? t:f=w401:string)
            n224 = call <vilib>:"Add State(s) to Queue__JKI_lib_State_Machine.vi"("State(s) in (\"\")"=w403, "State(s) at Back (\"\")"=w401) -> ("States Out"=w402:string)  [unwired: 13 in]
          }
          event "Video Source": Value Change {
            n225 = event-data() -> ()  [unwired: 1 in, 6 out]
            n226 = call <vilib>:"Add State(s) to Queue__JKI_lib_State_Machine.vi"("State(s) in Front (\"\")"="TCP: sendVideoSource" ("State(s) in Front (\"\")"), "State(s) in (\"\")"=w409) -> ("States Out"=w408:string)  [unwired: 13 in]
          }
          event "StopButton": Mouse Enter {
            n227 = event-data() -> ()  [unwired: 1 in, 4 out]
            n228 = local write "Help"("Press to stop data aquisition." ("Help")) -> ()
          }
          event "StopButton": Value Change {
            # "if system is running, send stop command, if not do nothing."
            # "stop aquisition\nupdate UI"
            n229 = event-data() -> ()  [unwired: 1 in, 6 out]
            n230 = Unbundle By Name(w417) -> ("SysRunning?"=w419:bool)
            n231 = case shown="True" w419 {
              tunnel: ["" ("Empty String Constant") "LabJack: AB_Stop\nLabJack: 355_PWM_Stop\n/*Digitizer: Abort"] -> w420
              tunnel: w417 -> [w424 w428]
              tunnel: [w424 w427] -> w418
              frame False {
              }
              frame True {
                n232 = Bundle By Name(cluster=w428, "SysRunning?"=FALSE) -> (w427:T23)
              }
            }
            n233 = call <vilib>:"Add State(s) to Queue__JKI_lib_State_Machine.vi"("State(s) in Front (\"\")"=w420, "State(s) in (\"\")"=w422) -> ("States Out"=w423:string)  [unwired: 13 in]
            n234 = local write "StopButton"(FALSE ("StopButton")) -> ()
          }
          event User Event {
            # "if system is running, send stop command, if not do nothing."
            # "stop aquisition\nupdate UI"
            n235 = event-data() -> ()  [unwired: 1 in, 5 out]
            n236 = Unbundle By Name(w430) -> ("SysRunning?"=w432:bool)
            n237 = case shown="True" w432 {
              tunnel: ["" ("Empty String Constant") "LabJack: AB_Stop\nLabJack: 355_PWM_Stop\n/*Digitizer: Abort"] -> w433
              tunnel: w430 -> [w437 w441]
              tunnel: [w437 w440] -> w431
              frame False {
              }
              frame True {
                n238 = Bundle By Name(cluster=w441, "SysRunning?"=FALSE) -> (w440:T23)
              }
            }
            n239 = call <vilib>:"Add State(s) to Queue__JKI_lib_State_Machine.vi"("State(s) in Front (\"\")"=w433, "State(s) in (\"\")"=w435) -> ("States Out"=w436:string)  [unwired: 13 in]
          }
          event "Sys Reconfig": Mouse Enter {
            n240 = event-data() -> ()  [unwired: 1 in, 4 out]
            n241 = local write "Help"("Click to reconfig digitizer settings." ("Help")) -> ()
          }
          event "Sys Reconfig": Value Change {
            # "everytime the user change data aquisition setting, need to reinitilize decon engine and realign iRF.\ncheck whether data length has changed, if changed, reinitialize Decon engine\nreset BG ready, need a new BG"
            # "update DAQ FGV"
            n242 = event-data() -> ()  [unwired: 1 in, 6 out]
            n243 = call "SystemConfigEditorV6.vi"("error in"=w457) -> ("error out"=w456:errorcluster, "FLImDAQ out"=w451:T5)  [unwired: 1 in]
            n244 = Unbundle By Name(w454) -> ("FLImDAQ.min record length"=w453:i32)
            n245 = Unbundle By Name(w451) -> ("min record length"=w452:i32)
            n246 = call "FLImDAQ_FGV.vi"("error in (no error)"=w456, "Operation (Read)"=enum16{"Write", "Read"}."Write" ("Operation"), "Write data"=w451) -> ("error out"=w455:errorcluster, "Read data"=w450:T5)  [unwired: 7 in]
            n247 = Equal?(x=w453, y=w452) -> (x = y?=w449:bool)
            n248 = case shown="False" w449 {
              tunnel: ["UI: Cursor Set >> Busy\nDigitizer: Config\nDeconEngine: InitializeCh1\nDeconEngine: InitializeCh2\nDeconEngine: InitializeCh3\nUI: CaliAndiRFNotReady\n/*UI iRF not ready\nUI: Update\nUI: Cursor Set >> Idle" "UI: Cursor Set >> Busy\nDigitizer: Config\nUI: Update\nUI: Cursor Set >> Idle"] -> w448
              frame False {
              }
              frame True {
              }
            }
            n249 = Bundle By Name(cluster=w454, "FLImDAQ"=w450) -> (w460:T23)
            n250 = call <vilib>:"Add State(s) to Queue__JKI_lib_State_Machine.vi"("State(s) in Front (\"\")"=w448, "State(s) in (\"\")"=w458) -> ("States Out"=w459:string)  [unwired: 13 in]
          }
          event "System Hardware Connection Status", "StartButton", "StopButton", "355nm Laser toggle", "Aiming beam toggle", "Cali&iRF alignment", "Background", "Sys Reconfig": Mouse Leave {
            n251 = event-data() -> ()  [unwired: 1 in, 4 out]
            n252 = invoke on="Help" class="Str" method="Reinit To Default"() -> ()  [unwired: 3 in, 3 out]
          }
          event "System Hardware Connection Status.Digitizer": Mouse Enter {
            n253 = event-data() -> ()  [unwired: 1 in, 4 out]
            n254 = local write "Help"("Status of hardware connections. TCP/IP is optional." ("Help")) -> ()
          }
          event "TCP Connect": Value Change {
            n255 = event-data() -> ("NewVal"=w470:bool)  [unwired: 1 in, 5 out]
            n256 = case shown="True" w470 {
              tunnel: ["TCP: Close\nUI: Update" ("State(s) in Front (\"\")") "TCP: SendSettingMacro\nUI: Update" ("State(s) in Front (\"\")")] -> w471
              frame False {
              }
              frame True {
              }
            }
            n257 = call <vilib>:"Add State(s) to Queue__JKI_lib_State_Machine.vi"("State(s) in Front (\"\")"=w471, "State(s) in (\"\")"=w473) -> ("States Out"=w472:string)  [unwired: 13 in]
          }
          event "488nm Power": Value Change {
            n258 = event-data() -> ()  [unwired: 1 in, 6 out]
            n259 = call <vilib>:"Add State(s) to Queue__JKI_lib_State_Machine.vi"("State(s) in Front (\"\")"="AimingBeam: Set Current" ("State(s) in Front (\"\")"), "State(s) in (\"\")"=w480) -> ("States Out"=w479:string)  [unwired: 13 in]
          }
          event User Event {
            # "if aquisition loop is error out. Stop digitizer, update front panel indicator, stop both laser and \nOption 1: parse and save data\nOption 2: Flash queue if scout run. [Covers: REQ23]"
            n260 = event-data() -> ()  [unwired: 1 in, 5 out]
            n261 = case shown="\"BG\"" "Data Class" {
              tunnel: [w500 "UI: Cursor Set >> Busy\nUtility: SetAllChanAutoGain\nUtility: RestoreDeConChan\nData: parseRunData\nData: irfAlignment\nUI: Cursor Set >> Idle" "UI: Cursor Set >> Busy\nUtility: SetAllChanAutoGain\nUtility: RestoreDeConChan\nData: parseRunData\nData: saveBGtoFGV\nData: saveBGtoFile\nUI: Cursor Set >> Idle\nData: showBG\nRun: BGIncrement"] -> w490
              frame "Data", Default {
                n262 = local read "Video Display"() -> (w502:bool)
                n263 = Select(t="TCP: startCam", s=w502, f="") -> (s? t:f=w498:string)
                n264 = call <vilib>:"Add State(s) to Queue__JKI_lib_State_Machine.vi"("State(s) in Front (\"\")"="UI: Cursor Set >> Busy\nData: parseRunData\nData: saveRunData\nUI: Cursor Set>>Idle" ("State(s) in Front (\"\")"), "State(s) in (\"\")"=w498) -> ("States Out"=w500:string)  [unwired: 13 in]
              }
              frame "Cali" {
              }
              frame "BG" {
              }
            }
            n265 = Bundle By Name(cluster=w492, "SysRunning?"=FALSE) -> (w493:T23)
            n266 = Select(t="" ("State(s) in Front (\"\")"), s="Skip Data Save?", f=w490) -> (s? t:f=w487:string)
            n267 = call <vilib>:"Add State(s) to Queue__JKI_lib_State_Machine.vi"("State(s) in Front (\"\")"="TCP: stopRun\nUI: Update\nLabJack: AB_Stop\nLabJack: 355_PWM_Stop\nDigitizer: Abort\nLabJack: ZeroV\nUtility: EndBeep\nLED: BreathOff" ("State(s) in Front (\"\")"), "State(s) in (\"\")"=w487, "State(s) at Back (\"\")"="Macro: SysReadyForAq\nUI: Update" ("State(s) in Front (\"\")")) -> ("States Out"=w485:string)  [unwired: 12 in]
            n268 = call <vilib>:"Add State(s) to Queue__JKI_lib_State_Machine.vi"("State(s) in Front (\"\")"=w485, "State(s) in (\"\")"=w494) -> ("States Out"=w495:string)  [unwired: 13 in]
          }
          event Panel Close? {
            # "Discard the event because we'll close the front panel ourselves in Macro: Exit"
            # "Close Panel button (pressed) Event\n(this executes Macro: Exit to terminate the VI)"
            n269 = event-data() -> ()  [unwired: 1 in, 1 out]
            n270 = event-data ("Event Filter Node")("Discard?"=TRUE) -> ()  [unwired: 1 in, 1 out]
            n271 = call <vilib>:"Add State(s) to Queue__JKI_lib_State_Machine.vi"("State(s) in Front (\"\")"="Macro: Exit", "State(s) in (\"\")"=w510) -> ("States Out"=w509:string)  [unwired: 13 in]
          }
        }
      }
      frame "---------- Macro ----------" {
        # "Do not put any code in this frame.\n(It is a separator no-op. You can make a copy of this frame to create a new Macro frame)"
        n272 = call <vilib>:"Add State(s) to Queue__JKI_lib_State_Machine.vi"("State(s) in (\"\")"=w515) -> ("States Out"=w514:string)  [unwired: 14 in]
      }
      frame "Macro: Initialize" {
        # "load Labjack setting 1st as it contaisn laser pin infortmation"
        # "start laser 1st, need 7.5s for laser to get ready"
        # "Initialization Macro\n(This is called once, when the VI starts)"
        n273 = call <vilib>:"Add State(s) to Queue__JKI_lib_State_Machine.vi"("State(s) in Front (\"\")"="UI: showDisclaimer\nUI: Cursor Set >> Busy\nData: Initialize\nInitialize Core Data\nUI: Initialize\nUI: Front Panel State >> Open\nMacro: LoadSysConfig\nTCP: InitializeNew\nTCP: checkSource\nUI: Update\nLabJack: Open\nLabJack: SetDefaultSub\nLED: OpenVIRef\nLED: BreathOrange\nUI: Update\n355 Laser: CheckControllerStatus\n355 Laser: Laser enable\n355 Laser: Dewelling>>500\n355 Laser: CheckControllerStatus\nUI: Update\nLabJack: 355_PWM_Config\nLabJack: AB_PWM_Config\nUI: Update", "State(s) in (\"\")"="Digitizer: Initialize\nDigitizer: Config\nUI: Update\nAimingBeam: Initialize\nAimingBeam: Set APC Status>>Disable\nAimingBeam: Set ACC Status>>Enable\nAimingBeam: Set Current\nUI: Update\n355 Laser: Check Dewelling\nUI: Cursor Set >> Idle\nCase: GetID\nUI: Update\nTCP: SendSettingMacro\nCase: CreatFileStruct\nUI: Update\nData: loadLastUseMacro\nDeconEngine: InitDotNet\nDeconEngine: loadIRF\nDeconEngine: Warmup\nClassifier: Init\nGraph: SetXMultiplier\nGraph: AddCursors\nAPD: Initialize\nAPD: LoadFromSerial\nAPD: UpdateCtrlVLimit\nAPD: GetGainLimits\nPID: loadPID\nLED: BreathOff\nMacro: SysReadyForAq") -> ("States Out"=w516:string)  [unwired: 13 in]
        n274 = call <vilib>:"Add State(s) to Queue__JKI_lib_State_Machine.vi"("State(s) in Front (\"\")"=w516, "State(s) in (\"\")"=w524) -> ("States Out"=w523:string)  [unwired: 13 in]
        "Help" <- "Hover over controls to see help!" ("Help")
      }
      frame "Macro: LoadSysConfig" {
        # "System configuration Macro. [Covers: REQ15]\n(Load configurations for different component of the system)"
        n275 = call <vilib>:"Add State(s) to Queue__JKI_lib_State_Machine.vi"("State(s) in Front (\"\")"="SysConfig: Load Sys Config\nSysConfig: Load Digitizer Setting\nSysConfig: Load AB setting\nSysConfig: Load LJ Pinout\nSysConfig: Load 355 PWM\nSysConfig: LoadAPDSerialNumber\nSysConfig: LoadABVideoSetting\nSysConfig: LoadCursorLocation", "State(s) in (\"\")"=w530) -> ("States Out"=w529:string)  [unwired: 13 in]
      }
      frame "Macro: SysReadyForAq" {
        # "Macro for system ready\n(It is a separator no-op. You can make a copy of this frame to create a new Macro frame)"
        n276 = call <vilib>:"Add State(s) to Queue__JKI_lib_State_Machine.vi"("State(s) in Front (\"\")"="UI: ReadyForAquisition\nLED: Green" ("State(s) in Front (\"\")"), "State(s) in (\"\")"=w536) -> ("States Out"=w535:string)  [unwired: 13 in]
      }
      frame "Macro: Exit" {
        # "close LJ last"
        # "check whether hardware is initilized, if so close, if not do nothing"
        # "Exit Macro, close all hardware\n(This is called once, when the VI exits)"
        n277 = Unbundle By Name(w555) -> ("System Status.Digitizer"=w551:bool, "System Status.Aiming Beam"=w550:bool, "System Status.355 Laser"=w549:bool, "System Status.Labjack"=w540:bool, "Core.Close Panel on Exit?"=w544:bool)
        n278 = case shown="True" w551 {
          tunnel: ["" ("Empty String Constant") "Digitizer: Close"] -> w546
          frame False {
          }
          frame True {
          }
        }
        n279 = case shown="True" w540 {
          tunnel: ["" ("Empty String Constant") "LabJack: SetDefaultAndClose"] -> w537
          frame False {
          }
          frame True {
          }
        }
        n280 = case shown="True" w550 {
          tunnel: ["" ("Empty String Constant") "AimingBeam: Set ACC Status >> Disable\nAimingBeam: Close"] -> w539
          frame False {
          }
          frame True {
          }
        }
        n281 = case shown="True" w549 {
          tunnel: ["" ("Empty String Constant") "355 Laser: Close\n355 Laser: CheckControllerStatus"] -> w538
          frame False {
          }
          frame True {
          }
        }
        n282 = Select(t="UI: Front Panel State >> Close", s=w544, f="" ("Empty String Constant")) -> (s? t:f=w541:string)
        n283 = call <vilib>:"Add State(s) to Queue__JKI_lib_State_Machine.vi"("State(s) in Front (\"\")"="TCP: Close\nDeconEngine: CloseNetRef\nClassifier: Close", "State(s) in (\"\")"=w546, "State(s) at Back (\"\")"=w539) -> ("States Out"=w548:string)  [unwired: 12 in]
        n284 = call <vilib>:"Add State(s) to Queue__JKI_lib_State_Machine.vi"("State(s) in Front (\"\")"=w548, "State(s) in (\"\")"=w538, "State(s) at Back (\"\")"=w537) -> ("States Out"=w543:string)  [unwired: 12 in]
        n285 = call <vilib>:"Add State(s) to Queue__JKI_lib_State_Machine.vi"("State(s) in Front (\"\")"=w543, "State(s) in (\"\")"="UI: Update\nUI: Reset\nGraph: SaveCursorLoc\nLED: CloseVIRef\nQueue: Destory\nData: Cleanup\nExit", "State(s) at Back (\"\")"=w541) -> ("States Out"=w552:string)  [unwired: 12 in]
        n286 = call <vilib>:"Add State(s) to Queue__JKI_lib_State_Machine.vi"("State(s) in Front (\"\")"=w552, "State(s) in (\"\")"=w558) -> ("States Out"=w557:string)  [unwired: 13 in]
      }
      frame "---------- Data ----------" {
        # "Do not put any code in this frame.\n(It is a separator no-op. You can make a copy of this frame to create a new Data frame)"
        n287 = call <vilib>:"Add State(s) to Queue__JKI_lib_State_Machine.vi"("State(s) in (\"\")"=w571) -> ("States Out"=w570:string)  [unwired: 14 in]
      }
      frame "Data: Initialize" {
        w572 = path ""  # CaliPath
        w573 = dbl[] []  # V4
        w574 = dbl[][] []  # Ch4Data
        w575 = FALSE  # bothVidSourceAvail
        w576 = T1 {"Main Frame Grabber"=FALSE, "Side Frame Grabber"=FALSE, "Main Camera"=FALSE, "Side Camera"=FALSE}  # video source
        w577 = FALSE  # LED vi ref open?
        w579 = T22 {"DeCon Channel"=enum."1", "Scale Bar"=FALSE, "Scale Low"=3.0, "Scale High"=8.0, "ANSI"=20.0, "Radius"=1.0, "3D?"=FALSE, "Firefly?"=FALSE, "Pentero?"=FALSE}  # VideoConfig
        w580 = T26 {"Ch1APDSerial#"="", "Ch2APDSerial#"="", "Ch3APDSerial#"="", "Ch4APDSerial#"=""}  # APDSerialNum
        w581 = u32 0  # Aquisition Timer
        w582 = cluster{"RunID":i8, "BG ID":i8, "Cali ID":i8} {"RunID"=1, "BG ID"=1, "Cali ID"=1}  # IDs
        w583 = refnum<vi> refnum  # LED vi reference
        w584 = path ""  # TempPath
        w585 = T27 {"DataPath"=path "", "BG Path"=path "", "iRFPath"=path "", "CaliPath"=path ""}  # Pathes
        w587 = dbl[] []  # V3
        w588 = dbl[] []  # V2
        w589 = dbl[] []  # V1
        w591 = u32 0  # FastTimer
        w592 = u32 0  # SlowTimer
        w593 = dbl[][] []  # Ch3Data
        w594 = dbl[][] []  # Ch2Data
        w578 = dbl[][] []  # Ch1Data
        w597 = T2 {"Digitizer"=FALSE, "Labjack"=FALSE, "Aiming Beam"=FALSE, "355 Laser"=FALSE, "TCP/IP"=FALSE}  # System Status
        w598 = T28 {"DIO_EF_CLOCK1_DIVISOR"=16, "DIO_EF_CLOCK1_ROLL_VALUE"=25000, "DIO#_EF_INDEX"=0, "DIO#_EF_OPTIONS"=1, "DIO#_EF_CONFIG_A"=6250}  # AB PWM setting
        w599 = T4 {"Ch1 Bias"="TDA11", "Ch2 Bias"="DAC10", "Ch3 Bias"="DAC0", "Ch4 Bias"="DAC0", "355 PWM"="FIO0", "AimingBeam PWM"="FIO2", "Laser Ready"="FIO3", "Interlock"="FIO1", "Laser Start/Stop"="FIO1", "Red LED"="FIO1", "Green LED"="FIO1", "Foot Pedal"="DIO15"}  # LJ Pinout
        w600 = 0  # TCP attempt count
        w601 = u32 0  # Laser start tic
        w602 = refnum<k20>[] []  # niTClk sessions
        w603 = u32 0  # Last Trigger
        w604 = T28 {"DIO_EF_CLOCK1_DIVISOR"=16, "DIO_EF_CLOCK1_ROLL_VALUE"=25000, "DIO#_EF_INDEX"=0, "DIO#_EF_OPTIONS"=1, "DIO#_EF_CONFIG_A"=6250}  # 355 PWM setting
        w605 = T29 {"Aiming Beam COM Port"="COM3", "Min Current"=0.0, "Max Current"=63.0, "Default Current"=20.0, "Freq"=0}  # AB Cluster
        w606 = T30 {"resource name"="", "resource name 2"="", "Channel"=enum."Channel 0", "trigger source"="VAL_EXTERNAL", "trigger level"=0.5, "trigger delay"=1.35e-07, "min sample rate"=12500000000.0, "min record length"=2500, "vertical range"=1.0, "vertical offset"=-0.25, "Waveform to Avg"=2000}  # FLImDAQ
        w607 = FALSE  # SysRunning?
        w595 = path ""  # DefaultPath
        w608 = ""  # CaseID
        w609 = T7 {"Ch1Enable?"=FALSE, "Ch2Enable?"=FALSE, "Ch3Enable?"=FALSE, "Ch1AutoGain?"=FALSE, "Ch2AutoGain?"=FALSE, "Ch3AutoGain?"=FALSE, "AimingBeamEnable?"=FALSE}  # SysConfigCluster
        w610 = T31 {"Current VI Reference"=refnum, "Close Panel on Exit?"=FALSE}  # Core
        # "Initialize the shift-register data, here.\n(data names are defined by what you wire into the bundle function)"
        n288 = Bundle("Core"=w610, "SysConfigCluster"=w609, "System Status"=w597, "IDs"=w582, "CaseID"=w608, "DefaultPath"=w595, "Pathes"=w585, "FLImDAQ"=w606, "SysRunning?"=w607, "AB Cluster"=w605, "LJ Pinout"=w599, "355 PWM setting"=w604, "AB PWM setting"=w598, "Last Trigger"=w603, "niTClk sessions"=w602, "Laser start tic"=w601, "TCP attempt count"=w600, "Ch1Data"=w578, "Ch2Data"=w594, "Ch3Data"=w593, "Ch4Data"=w574, "V1"=w589, "V2"=w588, "V3"=w587, "V4"=w573, "SlowTimer"=w592, "FastTimer"=w591, "listener ID"=refnum<k5> refnum, "TempPath"=w584, "CaliPath"=w572, "LED vi reference"=w583, "Aquisition Timer"=w581, "APDSerialNum"=w580, "VideoConfig"=w579, "LED vi ref open?"=w577, "video source"=w576, "bothVidSourceAvail"=w575) -> (w586:T23)  [unwired: 1 in]
        n289 = call <vilib>:"Add State(s) to Queue__JKI_lib_State_Machine.vi"("State(s) in (\"\")"=w613) -> ("States Out"=w612:string)  [unwired: 14 in]
      }
      frame "Data: loadLastUseMacro" {
        # "Load last use BG and Cali and iRF.\n(It is a separator no-op. You can make a copy of this frame to create a new Data frame)"
        n290 = call <vilib>:"Add State(s) to Queue__JKI_lib_State_Machine.vi"("State(s) in Front (\"\")"="Data: loadLastUseBG\nData: loadSystemCali\nData: loadLastUseiRF\n/*Data: LoadiRFFromAPDFile\nUI: CaliAndiRFLoaded\nData: ShowiRF" ("State(s) in Front (\"\")"), "State(s) in (\"\")"=w619) -> ("States Out"=w618:string)  [unwired: 13 in]
      }
      frame "Data: loadLastUseBG" {
        w623 = enum16{"write", "read"}."write" ("action")
        # "Load last use BG.\n()"
        n291 = Unbundle By Name(w642) -> ("TempPath"=w641:path)
        n292 = call "FLImDAQ_FGV.vi"() -> ("Read data"=w637:T5)  [unwired: 10 in, 1 out]
        n293 = Build Path(base path=w641, name or relative path="Background.tdms") -> (appended path=w640:path)
        n294 = call "ReadBGorCali (SubVI).vi"("DataType"=enum16{"BG", "Cali"}."BG", "error in (no error)"=w639, "file path in"=w640) -> ("error out"=w638:errorcluster, "AvgDataCluster"=w633:T32)  [unwired: 6 in, 1 out]
        n295 = Unbundle By Name(w633) -> ("Channel 1"=w620:dbl[], "Channel 2"=w632:dbl[], "Channel 3"=w625:dbl[], "Channel 4"=w622:dbl[])
        n296 = Unbundle By Name(w637) -> ("min record length"=w629:i32)
        n297 = Array Size(array=w620) -> (size(s)=w631:i32)
        "BG length" <- w631
        n298 = Equal?(x=w631, y=w629) -> (x = y?=w630:bool)
        n299 = Select(t="UI: BGLoaded" ("State(s) in Front (\"\")"), s=w630, f="UI: BGSizeError" ("State(s) in Front (\"\")")) -> (s? t:f=w634:string)
        n300 = case shown="True" w630 {
          tunnel: w620 -> [_ w653]
          tunnel: w632 -> [_ w652]
          tunnel: w625 -> [_ w651]
          tunnel: w629 -> [w648 _]
          tunnel: [w647 w653] -> w628
          tunnel: [w647 w652] -> w627
          tunnel: [w647 w651] -> w626
          tunnel: w622 -> [_ w650]
          tunnel: [w647 w650] -> w621
          frame False {
            # "If error set BG all 0, update UI"
            n301 = for {
              N: w648 -> [_]
              tunnel: [0.0] -> w647 mode=indexing
            }
          }
          frame True {
            # "If no error, check size match"
          }
        }
        n302 = call "BG4FGV.vi"("action"=w623, "BG4 in"=w621) -> ()  [unwired: 8 in, 2 out]
        n303 = call "BG3FGV.vi"("action"=w623, "BG3 in"=w626) -> ()  [unwired: 8 in, 2 out]
        n304 = call "BG1FGV.vi"("action"=w623, "BG1 in"=w628) -> ()  [unwired: 8 in, 2 out]
        n305 = call "BG2FGV.vi"("action"=w623, "BG2 in"=w627) -> ()  [unwired: 8 in, 2 out]
        n306 = call <vilib>:"Add State(s) to Queue__JKI_lib_State_Machine.vi"("State(s) in Front (\"\")"=w634, "State(s) in (\"\")"=w646) -> ("States Out"=w645:string)  [unwired: 13 in]
      }
      frame "Data: loadSystemCali" {
        # "Load last use calibration.\n()"
        n307 = Unbundle By Name(w661) -> ("CaliPath"=w660:path)
        n308 = Build Path(base path=w660, name or relative path="Calibration.tdms") -> (appended path=w656:path)
        n309 = call "ReadBGorCali (SubVI).vi"("DataType"=enum16{"BG", "Cali"}."Cali", "error in (no error)"=w655, "file path in"=w656) -> ("error out"=w657:errorcluster, "CtrlVCluster"=w659:T33, "AvgDataCluster"=w658:T32)  [unwired: 6 in]
        n310 = case shown="No Error" w657 {
          tunnel: w659 -> [w680 _]
          tunnel: w658 -> [w679 _]
          frame No Error {
            w670 = T34 {"Ch1 WF"=[], "Ch2 WF"=[], "Ch3 WF"=[], "Ch4 WF"=[], "V1"=0.0, "V2"=0.0, "V3"=0.0, "V4"=0.0}  # SysCaliData
            n311 = Unbundle By Name(w679) -> ("Channel 1"=w678:dbl[], "Channel 2"=w677:dbl[], "Channel 3"=w676:dbl[], "Channel 4"=w669:dbl[])
            n312 = Unbundle By Name(w680) -> ("V 1"=w675:dbl[], "V 2"=w674:dbl[], "V 3"=w668:dbl[], "V 4"=w666:dbl[])
            n313 = Index Array(array=w675) -> (element=w673:dbl)  [unwired: 1 in]
            n314 = Index Array(array=w674) -> (element=w672:dbl)  [unwired: 1 in]
            n315 = Index Array(array=w668) -> (element=w671:dbl)  [unwired: 1 in]
            n316 = Index Array(array=w666) -> (element=w667:dbl)  [unwired: 1 in]
            n317 = Bundle By Name(cluster=w670, "Ch1 WF"=w678, "Ch2 WF"=w677, "Ch3 WF"=w676, "Ch4 WF"=w669, "V1"=w673, "V2"=w672, "V3"=w671, "V4"=w667) -> (w681:T34)
            n318 = global write "GlobalVariables.vi" "SysCaliData"(w681) -> ()
          }
          frame Error {
          }
        }
        n319 = call <vilib>:"Add State(s) to Queue__JKI_lib_State_Machine.vi"("State(s) in (\"\")"=w665) -> ("States Out"=w664:string)  [unwired: 14 in]
      }
      frame "Data: LoadiRFFromAPDFile" {
        w711 = T15 {"Ch1 iRF"=[], "Ch2 iRF"=[], "Ch3 iRF"=[], "Ch4 iRF"=[]}  # LastUseiRF
        # "only load the last 5th  iRF for the moment"
        # "Load APD detector data\n(It is a separator no-op. You can make a copy of this frame to create a new Data frame)"
        n320 = Unbundle By Name(w733) -> ("APDSerialNum.Ch1APDSerial#"=w732:string, "APDSerialNum.Ch2APDSerial#"=w713:string, "APDSerialNum.Ch3APDSerial#"=w712:string, "APDSerialNum.Ch4APDSerial#"=w709:string)
        n321 = call "CreatFromSerialNumNoRaw.vi"("error in (no error)"=w710, "APD Serial #"=w732) -> ("error out"=w730:errorcluster, "APDClass out"=w731:refnum<class "APDClass.lvclass">)  [unwired: 8 in]
        n322 = call "CreatFromSerialNumNoRaw.vi"("error in (no error)"=w710, "APD Serial #"=w713) -> ("error out"=w721:errorcluster, "APDClass out"=w722:refnum<class "APDClass.lvclass">)  [unwired: 8 in]
        n323 = call "CreatFromSerialNumNoRaw.vi"("error in (no error)"=w710, "APD Serial #"=w712) -> ("error out"=w715:errorcluster, "APDClass out"=w716:refnum<class "APDClass.lvclass">)  [unwired: 8 in]
        n324 = call "CreatFromSerialNumNoRaw.vi"("error in (no error)"=w710, "APD Serial #"=w709) -> ("error out"=w707:errorcluster, "APDClass out"=w708:refnum<class "APDClass.lvclass">)  [unwired: 8 in]
        n325 = call-dynamic "Read iRFData.vi"("error in (no error)"=w730, "APDClass in"=w731) -> ("iRFData"=w729:T35)  [unwired: 7 in, 2 out]
        n326 = call-dynamic "Read iRFData.vi"("error in (no error)"=w721, "APDClass in"=w722) -> ("iRFData"=w725:T35)  [unwired: 7 in, 2 out]
        n327 = call-dynamic "Read iRFData.vi"("error in (no error)"=w715, "APDClass in"=w716) -> ("iRFData"=w719:T35)  [unwired: 7 in, 2 out]
        n328 = call-dynamic "Read iRFData.vi"("error in (no error)"=w707, "APDClass in"=w708) -> ("iRFData"=w706:T35)  [unwired: 7 in, 2 out]
        n329 = Unbundle By Name(w729) -> ("iRFWFsAvg"=w728:dbl[][])
        n330 = Unbundle By Name(w725) -> ("iRFWFsAvg"=w724:dbl[][])
        n331 = Unbundle By Name(w719) -> ("iRFWFsAvg"=w718:dbl[][])
        n332 = Unbundle By Name(w706) -> ("iRFWFsAvg"=w703:dbl[][])
        n333 = Array Size(array=w728) -> (size(s)=w727:i32[])
        n334 = Array Size(array=w724) -> (size(s)=w720:i32[])
        n335 = Array Size(array=w718) -> (size(s)=w714:i32[])
        n336 = Array Size(array=w703) -> (size(s)=w704:i32[])
        n337 = Index Array(array=w727, index=0) -> (element=w702:i32)
        n338 = Index Array(array=w720, index=0) -> (element=w698:i32)
        n339 = Index Array(array=w714, index=0) -> (element=w695:i32)
        n340 = Index Array(array=w704, index=0) -> (element=w692:i32)
        n341 = Subtract(x=w702, y=5) -> (x-y=w700:i32)
        n342 = Subtract(x=w698, y=5) -> (x-y=w697:i32)
        n343 = Subtract(x=w695, y=5) -> (x-y=w694:i32)
        n344 = Subtract(x=w692, y=5) -> (x-y=w691:i32)
        n345 = Index Array(array=w728, index (row)=w700) -> (element=w690:dbl[])  [unwired: 1 in]
        n346 = Index Array(array=w724, index (row)=w697) -> (element=w689:dbl[])  [unwired: 1 in]
        n347 = Index Array(array=w718, index (row)=w694) -> (element=w688:dbl[])  [unwired: 1 in]
        n348 = Index Array(array=w703, index (row)=w691) -> (element=w687:dbl[])  [unwired: 1 in]
        n349 = call "DownSampleAndShiftiRF (SubVI).vi"("ArrayIn"=w690) -> ("ArrayOut"=w686:dbl[])  [unwired: 10 in]
        n350 = call "DownSampleAndShiftiRF (SubVI).vi"("ArrayIn"=w689) -> ("ArrayOut"=w682:dbl[])  [unwired: 10 in]
        n351 = call "DownSampleAndShiftiRF (SubVI).vi"("ArrayIn"=w688) -> ("ArrayOut"=w683:dbl[])  [unwired: 10 in]
        n352 = call "DownSampleAndShiftiRF (SubVI).vi"("ArrayIn"=w687) -> ("ArrayOut"=w685:dbl[])  [unwired: 10 in]
        n353 = call <vilib>:"Add State(s) to Queue__JKI_lib_State_Machine.vi"("State(s) in (\"\")"=w736) -> ("States Out"=w735:string)  [unwired: 14 in]
        n354 = Bundle(cluster=w711, "Ch1 iRF"=w686, "Ch2 iRF"=w682, "Ch3 iRF"=w683, "Ch4 iRF"=w685) -> (w684:T15)
        n355 = global write "GlobalVariables.vi" "LastUseiRF"(w684) -> ()
      }
      frame "Data: loadLastUseiRF" {
        # "Load last use iRF.\n()"
        n356 = Unbundle By Name(w742) -> ("TempPath"=w741:path)
        n357 = Build Path(base path=w741, name or relative path="iRF.tdms") -> (appended path=w747:path)
        n358 = TDMS Open(8:w737, 11:w747) -> (0:w745:errorcluster, 3:w746:refnum<k34>)  [unwired: 5 in]
        n359 = TDMS Read(0:w746, 11:w745, 12:dbl[][] []) -> (4:w740:refnum<k34>, 10:w743:dbl[][], 15:w739:errorcluster)  [unwired: 5 in, 3 out]
        n360 = TDMS Close(8:w739, 11:w740) -> (0:w738:errorcluster)  [unwired: 1 out]
        n361 = case shown="No Error" w739 {
          tunnel: w743 -> [w757 _]
          frame No Error {
            w760 = T15 {"Ch1 iRF"=[], "Ch2 iRF"=[], "Ch3 iRF"=[], "Ch4 iRF"=[]}  # LastUseiRF
            n362 = Index Array(array=w757, index (row)=0) -> (element=w752:dbl[])  [unwired: 1 in]
            n363 = Index Array(array=w757, index (row)=1) -> (element=w753:dbl[])  [unwired: 1 in]
            n364 = Index Array(array=w757, index (row)=2) -> (element=w754:dbl[])  [unwired: 1 in]
            n365 = Index Array(array=w757, index (row)=3) -> (element=w755:dbl[])  [unwired: 1 in]
            n366 = Add Array Elements(numeric array=w752) -> (sum=w766:dbl)
            n367 = Add Array Elements(numeric array=w753) -> (sum=w764:dbl)
            n368 = Add Array Elements(numeric array=w754) -> (sum=w762:dbl)
            n369 = Add Array Elements(numeric array=w755) -> (sum=w758:dbl)
            n370 = Divide(x=w752, y=w766) -> (x/y=w765:dbl[])
            n371 = Divide(x=w753, y=w764) -> (x/y=w763:dbl[])
            n372 = Divide(x=w754, y=w762) -> (x/y=w761:dbl[])
            n373 = Divide(x=w755, y=w758) -> (x/y=w756:dbl[])
            n374 = Bundle(cluster=w760, "Ch1 iRF"=w765, "Ch2 iRF"=w763, "Ch3 iRF"=w761, "Ch4 iRF"=w756) -> (w768:T15)
            n375 = Array Size(array=w752) -> (size(s)=→"iRF length":i32)
            n376 = global write "GlobalVariables.vi" "LastUseiRF"(w768) -> ()
          }
          frame Error {
          }
        }
        n377 = call <vilib>:"Add State(s) to Queue__JKI_lib_State_Machine.vi"("State(s) in (\"\")"=w751) -> ("States Out"=w750:string)  [unwired: 14 in]
      }
      frame "Data: ShowiRF" {
        # "Show loaded iRF.\n(It is a separator no-op. You can make a copy of this frame to create a new Data frame)"
        n378 = global read "GlobalVariables.vi" "LastUseiRF"() -> (w777:T15)
        n379 = Unbundle By Name(w777) -> ("Ch1 iRF"=w776:dbl[], "Ch2 iRF"=w775:dbl[], "Ch3 iRF"=w774:dbl[], "Ch4 iRF"=w773:dbl[])
        n380 = Build Array(w776, w775, w774, w773) -> (→"iRF Graph":dbl[][])
        n381 = call <vilib>:"Add State(s) to Queue__JKI_lib_State_Machine.vi"("State(s) in (\"\")"=w782) -> ("States Out"=w781:string)  [unwired: 14 in]
      }
      frame "Data: saveCalibration" {
        # "Average data and save calibration file. [Covers: REQ11]\n(It is a separator no-op. You can make a copy of this frame to create a new Data frame)"
        n382 = Unbundle By Name(w801) -> ("Ch1Data"=w800:dbl[][], "V1"=w799:dbl[], "Ch2Data"=w798:dbl[][], "V2"=w797:dbl[], "Ch3Data"=w796:dbl[][], "V3"=w795:dbl[], "Ch4Data"=w786:dbl[][], "V4"=w785:dbl[], "Pathes.CaliPath"=w804:path, "IDs.Cali ID"=w803:i8)
        n383 = Increment(x=w803) -> (x+1=w787:i8)
        n384 = Bundle("Ch1Data"=w800, "V1"=w799) -> (w794:cluster{"Ch1Data":dbl[][], "V1":dbl[]})  [unwired: 1 in]
        n385 = Bundle("Ch4Data"=w786, "V4"=w785) -> (w784:cluster{"Ch4Data":dbl[][], "V4":dbl[]})  [unwired: 1 in]
        n386 = Bundle("Ch2Data"=w798, "V2"=w797) -> (w793:cluster{"Ch2Data":dbl[][], "V2":dbl[]})  [unwired: 1 in]
        n387 = Bundle("Ch3Data"=w796, "V3"=w795) -> (w792:cluster{"Ch3Data":dbl[][], "V3":dbl[]})  [unwired: 1 in]
        n388 = Format Value(string ("")="Calibration" ("default name"), format string="%02d", value (0)=w787) -> (output string=w806:string)
        n389 = Build Path(base path=w804, name or relative path=w806) -> (appended path=w791:path)
        n390 = call "SaveBGorCali(SubVI).vi"("Channel1"=w794, "BG path"=w791, "DataType"=enum16{"BG", "Cali"}."Cali", "Channel 2"=w793, "Channel 3"=w792, "Channel 4"=w784, "error in (no error)"=w790, "SytemID"="UCDVetMed") -> ("error out"=w789:errorcluster)  [unwired: 7 in]
        n391 = call <vilib>:"Add State(s) to Queue__JKI_lib_State_Machine.vi"("State(s) in (\"\")"=w809) -> ("States Out"=w808:string)  [unwired: 14 in]
      }
      frame "Data: saveiRF" {
        w815 = enum16{"write", "read"}."read" ("action")
        # "Get iRF from decon stracture and save it on disk.\n(It is a separator no-op. You can make a copy of this frame to create a new Data frame)"
        n392 = Unbundle By Name(w832) -> ("TempPath"=w831:path)
        n393 = call "Ch1DeconEngineFGV.vi"("action(read)"=w815) -> ("Error Out"=w837:errorcluster, "Ch1DeconEngine out"=w838:refnum<class "LaguerreDeconEngineClass.lvclass">)  [unwired: 9 in]
        n394 = call "Ch2DeconEngineFGV.vi"("action(read)"=w815) -> ("Error Out"=w835:errorcluster, "Ch2DeconEngine out"=w836:refnum<class "LaguerreDeconEngineClass.lvclass">)  [unwired: 9 in]
        n395 = call "Ch3DeconEngineFGV.vi"("action(read)"=w815) -> ("Error Out"=w833:errorcluster, "Ch3DeconEngine out"=w834:refnum<class "LaguerreDeconEngineClass.lvclass">)  [unwired: 9 in]
        n396 = call "Ch4DeconEngineFGV.vi"("action(read)"=w815) -> ("Error Out"=w814:errorcluster, "Ch3DeconEngine out"=w813:refnum<class "LaguerreDeconEngineClass.lvclass">)  [unwired: 9 in]
        n397 = Build Path(base path=w831, name or relative path="iRF" ("default name")) -> (appended path=w829:path)
        n398 = call "getIRF.vi"("error in (no error)"=w814, "LaguerreDeconEngineClass in"=w813) -> ("iRF"=w812:dbl[])  [unwired: 7 in, 2 out]
        n399 = call "getIRF.vi"("error in (no error)"=w837, "LaguerreDeconEngineClass in"=w838) -> ("iRF"=w820:dbl[])  [unwired: 7 in, 2 out]
        n400 = call "getIRF.vi"("error in (no error)"=w835, "LaguerreDeconEngineClass in"=w836) -> ("iRF"=w819:dbl[])  [unwired: 7 in, 2 out]
        n401 = call "getIRF.vi"("error in (no error)"=w833, "LaguerreDeconEngineClass in"=w834) -> ("iRF"=w818:dbl[])  [unwired: 7 in, 2 out]
        n402 = TDMS Open(8:w828, 10:T16."create or replace" ("operation (0:open)"), 11:w829) -> (0:w825:errorcluster, 3:w826:refnum<k34>)  [unwired: 4 in]
        n403 = Bundle(cluster=T15 {"Ch1 iRF"=[], "Ch2 iRF"=[], "Ch3 iRF"=[], "Ch4 iRF"=[]} ("LastUseiRF"), "Ch1 iRF"=w820, "Ch2 iRF"=w819, "Ch3 iRF"=w818, "Ch4 iRF"=w812) -> (w816:T15)
        n404 = Build Array(w820, w819, w818, w812) -> (w824:dbl[][])
        n405 = global write "GlobalVariables.vi" "LastUseiRF"(w816) -> ()
        n406 = TDMS Write(0:w826, 5:"iRF" ("group name in (Untitled)"), 7:string[] ["Ch1", "Ch2", "Ch3", "Ch4"] ("channel name(s) in (Untitled)"), 9:w824, 11:w825) -> (4:w823:refnum<k34>, 15:w822:errorcluster)  [unwired: 1 in, 2 out]
        n407 = TDMS Close(8:w822, 11:w823) -> (0:w821:errorcluster)  [unwired: 1 out]
        n408 = call <vilib>:"Add State(s) to Queue__JKI_lib_State_Machine.vi"("State(s) in (\"\")"=w841) -> ("States Out"=w840:string)  [unwired: 14 in]
      }
      frame "Data: saveBGtoFGV" {
        w868 = enum16{"write", "read"}."write" ("action")
        # "Save BG and pass it to FGV.\n(save BG to disk and set it to FGV)"
        n409 = call "DotNetFGV.vi"("Error In"=w858) -> ("Error Out"=w863:errorcluster, "reference out"=w864:refnum<k24>)  [unwired: 9 in]
        n410 = Unbundle By Name(w869) -> ("Ch1Data"=w853:dbl[][], "Ch2Data"=w851:dbl[][], "Ch3Data"=w849:dbl[][], "Ch4Data"=w847:dbl[][])
        n411 = Transpose 2D Array(2D array=w853) -> (transposed array=w867:dbl[][])
        n412 = Transpose 2D Array(2D array=w851) -> (transposed array=w866:dbl[][])
        n413 = Transpose 2D Array(2D array=w849) -> (transposed array=w865:dbl[][])
        n414 = call "AvgArrayTimeCritical.vi"("2D array"=w851) -> ("1D Avg"=w850:dbl[])  [unwired: 10 in]
        n415 = call "AvgArrayTimeCritical.vi"("2D array"=w849) -> ("1D Avg"=w848:dbl[])  [unwired: 10 in]
        n416 = call "WaveformTUA(SubVI).vi"("error in (no error)"=w863, "WF in"=w867, "new reference"=w864) -> ("error out"=w845:errorcluster, "WF out"=w854:dbl[])  [unwired: 6 in, 1 out]
        n417 = call "WaveformTUA(SubVI).vi"("error in (no error)"=w863, "WF in"=w866, "new reference"=w864) -> ("error out"=w844:errorcluster, "WF out"=w856:dbl[])  [unwired: 6 in, 1 out]
        n418 = call "WaveformTUA(SubVI).vi"("error in (no error)"=w863, "WF in"=w865, "new reference"=w864) -> ("error out"=w843:errorcluster, "WF out"=w855:dbl[])  [unwired: 6 in, 1 out]
        n419 = call "AvgArrayTimeCritical.vi"("2D array"=w853) -> ("1D Avg"=w852:dbl[])  [unwired: 10 in]
        n420 = call "AvgArrayTimeCritical.vi"("2D array"=w847) -> ("1D Avg"=w846:dbl[])  [unwired: 10 in]
        n421 = call "BG1FGV.vi"("Error In"=w845, "action"=w868, "BG1 in"=w852) -> ("Error Out"=w862:errorcluster)  [unwired: 7 in, 1 out]
        n422 = call "BG2FGV.vi"("Error In"=w844, "action"=w868, "BG2 in"=w850) -> ("Error Out"=w861:errorcluster)  [unwired: 7 in, 1 out]
        n423 = call "BG3FGV.vi"("Error In"=w843, "action"=w868, "BG3 in"=w848) -> ("Error Out"=w860:errorcluster)  [unwired: 7 in, 1 out]
        n424 = call "BG4FGV.vi"("action"=w868, "BG4 in"=w846) -> ("Error Out"=w859:errorcluster)  [unwired: 8 in, 1 out]
        n425 = Build Array(w854, w856, w855) -> (→"BGAll" →"BG Graph":dbl[][])
        n426 = Merge Errors(w862, w861, w860, w859) -> (w857:errorcluster)
        n427 = call <vilib>:"Add State(s) to Queue__JKI_lib_State_Machine.vi"("State(s) in (\"\")"=w872) -> ("States Out"=w871:string)  [unwired: 14 in]
      }
      frame "Data: saveBGtoFile" {
        w894 = "Background" ("name or relative path")
        # "Save BG to file.\n(save BG to disk both data folder and temp folder)"
        n428 = Unbundle By Name(w898) -> ("Pathes.BG Path"=w891:path, "IDs.BG ID"=w890:i8, "Ch1Data"=w888:dbl[][], "V1"=w887:dbl[], "Ch2Data"=w886:dbl[][], "V2"=w885:dbl[], "Ch3Data"=w884:dbl[][], "V3"=w883:dbl[], "Ch4Data"=w875:dbl[][], "V4"=w874:dbl[], "TempPath"=w896:path)
        n429 = Increment(x=w890) -> (x+1=w895:i8)
        n430 = Format Value(string ("")=w894, format string="%02d", value (0)=w895) -> (output string=w893:string)
        n431 = Build Path(base path=w896, name or relative path=w894) -> (appended path=w877:path)
        n432 = call "File Dialog2"("start path"=w891, "prompt"="Please select BG name, DO NOT CANCEL!", "default name"=w893) -> ("selected path"=w878:path)  [unwired: 9 in, 3 out]
        n433 = Bundle("Ch1Data"=w888, "V1"=w887) -> (w882:cluster{"Ch1Data":dbl[][], "V1":dbl[]})  [unwired: 1 in]
        n434 = Bundle("Ch4Data"=w875, "V4"=w874) -> (w873:cluster{"Ch4Data":dbl[][], "V4":dbl[]})  [unwired: 1 in]
        n435 = Bundle("Ch2Data"=w886, "V2"=w885) -> (w881:cluster{"Ch2Data":dbl[][], "V2":dbl[]})  [unwired: 1 in]
        n436 = Bundle("Ch3Data"=w884, "V3"=w883) -> (w880:cluster{"Ch3Data":dbl[][], "V3":dbl[]})  [unwired: 1 in]
        n437 = Build Array(w878, w877) -> (w876:path[])
        n438 = for {
          tunnel: w882 -> [w909]
          tunnel: w881 -> [w908]
          tunnel: w880 -> [w907]
          shift-right: [w910] -> w889
          shift-left: w879 -> [w906]
          tunnel: w876 -> [w905] mode=indexing
          tunnel: w873 -> [w903]
          n439 = call "SaveBGorCali(SubVI).vi"("Channel1"=w909, "BG path"=w905, "DataType"=enum16{"BG", "Cali"}."BG", "Channel 2"=w908, "Channel 3"=w907, "Channel 4"=w903, "error in (no error)"=w906, "SytemID"="UCDVetMed") -> ("error out"=w910:errorcluster)  [unwired: 7 in]
        }
        n440 = call <vilib>:"Add State(s) to Queue__JKI_lib_State_Machine.vi"("State(s) in (\"\")"=w901) -> ("States Out"=w900:string)  [unwired: 14 in]
      }
      frame "Data: showBG" {
        # "Show BG in seperate window.\n()"
        n441 = call "showBG.vi"() -> ()  [unwired: 12 in]
        n442 = call <vilib>:"Add State(s) to Queue__JKI_lib_State_Machine.vi"("State(s) in (\"\")"=w915) -> ("States Out"=w914:string)  [unwired: 14 in]
      }
      frame "Data: irfAlignment" {
        w916 = enum16{"write", "read"}."write" ("action")
        # "do iRF alignment in this state\n(It is a separator no-op. You can make a copy of this frame to create a new Data frame)"
        n443 = Unbundle By Name(w961) -> ("Ch1Data"=w997:dbl[][], "Ch2Data"=w996:dbl[][], "Ch3Data"=w995:dbl[][], "Ch4Data"=w938:dbl[][])
        n444 = call "Ch1DeconEngineFGV.vi"("Error In"=w937) -> ("Error Out"=w993:errorcluster, "Ch1DeconEngine out"=w994:refnum<class "LaguerreDeconEngineClass.lvclass">)  [unwired: 9 in]
        n445 = call "Ch2DeconEngineFGV.vi"("Error In"=w937) -> ("Error Out"=w991:errorcluster, "Ch2DeconEngine out"=w992:refnum<class "LaguerreDeconEngineClass.lvclass">)  [unwired: 9 in]
        n446 = call "Ch3DeconEngineFGV.vi"("Error In"=w937) -> ("Error Out"=w989:errorcluster, "Ch3DeconEngine out"=w990:refnum<class "LaguerreDeconEngineClass.lvclass">)  [unwired: 9 in]
        n447 = call "Ch4DeconEngineFGV.vi"("Error In"=w937) -> ("Error Out"=w928:errorcluster, "Ch3DeconEngine out"=w927:refnum<class "LaguerreDeconEngineClass.lvclass">)  [unwired: 9 in]
        n448 = call "AvgArray.vi"("2D array in"=w996) -> ("1D Avg out"=w943:dbl[])  [unwired: 10 in]
        n449 = call "AvgArray.vi"("2D array in"=w995) -> ("1D Avg out"=w942:dbl[])  [unwired: 10 in]
        n450 = call "AvgArray.vi"("2D array in"=w938) -> ("1D Avg out"=w917:dbl[])  [unwired: 10 in]
        n451 = call "AvgArray.vi"("2D array in"=w997) -> ("1D Avg out"=w944:dbl[])  [unwired: 10 in]
        n452 = call "RemoveDCBG.vi"("WF in"=w944) -> ("DC"=w951:dbl, "WF out"=w941:dbl[])  [unwired: 8 in, 1 out]
        n453 = call "RemoveDCBG.vi"("WF in"=w943) -> ("DC"=w948:dbl, "WF out"=w954:dbl[])  [unwired: 8 in, 1 out]
        n454 = call "RemoveDCBG.vi"("WF in"=w942) -> ("DC"=w946:dbl, "WF out"=w953:dbl[])  [unwired: 8 in, 1 out]
        n455 = call "RemoveDCBG.vi"("WF in"=w917) -> ("DC"=w921:dbl, "WF out"=w919:dbl[])  [unwired: 8 in, 1 out]
        n456 = call "computeIRFAlignment.vi"("error in (no error)"=w993, "fIRF temp"=w941, "LaguerreDeconEngineClass in"=w994) -> ("error out"=w985:errorcluster, "LaguerreDeconEngineClass out"=w986:refnum<class "LaguerreDeconEngineClass.lvclass">)  [unwired: 6 in, 1 out]
        n457 = call "computeIRFAlignment.vi"("error in (no error)"=w991, "fIRF temp"=w954, "LaguerreDeconEngineClass in"=w992) -> ("error out"=w983:errorcluster, "LaguerreDeconEngineClass out"=w984:refnum<class "LaguerreDeconEngineClass.lvclass">)  [unwired: 6 in, 1 out]
        n458 = call "computeIRFAlignment.vi"("error in (no error)"=w989, "fIRF temp"=w953, "LaguerreDeconEngineClass in"=w990) -> ("error out"=w987:errorcluster, "LaguerreDeconEngineClass out"=w988:refnum<class "LaguerreDeconEngineClass.lvclass">)  [unwired: 6 in, 1 out]
        n459 = call "computeIRFAlignment.vi"("error in (no error)"=w928, "fIRF temp"=w919, "LaguerreDeconEngineClass in"=w927) -> ("error out"=w935:errorcluster, "LaguerreDeconEngineClass out"=w936:refnum<class "LaguerreDeconEngineClass.lvclass">)  [unwired: 6 in, 1 out]
        n460 = call "Ch1DeconEngineFGV.vi"("Error In"=w985, "action(read)"=w916, "Ch1DeconEngine in"=w986) -> ("Error Out"=w981:errorcluster, "Ch1DeconEngine out"=w982:refnum<class "LaguerreDeconEngineClass.lvclass">)  [unwired: 7 in]
        n461 = call "Ch2DeconEngineFGV.vi"("Error In"=w983, "action(read)"=w916, "Ch2DeconEngine in"=w984) -> ("Error Out"=w971:errorcluster, "Ch2DeconEngine out"=w972:refnum<class "LaguerreDeconEngineClass.lvclass">)  [unwired: 7 in]
        n462 = call "Ch3DeconEngineFGV.vi"("Error In"=w987, "action(read)"=w916, "Ch3DeconEngine in"=w988) -> ("Error Out"=w965:errorcluster, "Ch3DeconEngine out"=w966:refnum<class "LaguerreDeconEngineClass.lvclass">)  [unwired: 7 in]
        n463 = call "Ch4DeconEngineFGV.vi"("Error In"=w935, "action(read)"=w916, "Ch3DeconEngine in"=w936) -> ("Error Out"=w929:errorcluster, "Ch3DeconEngine out"=w930:refnum<class "LaguerreDeconEngineClass.lvclass">)  [unwired: 7 in]
        n464 = call "setfIRF.vi"("error in (no error)"=w965, "fIRF"=w953, "LaguerreDeconEngineClass in"=w966) -> ("error out"=w969:errorcluster, "LaguerreDeconEngineClass out"=w970:refnum<class "LaguerreDeconEngineClass.lvclass">)  [unwired: 7 in]
        n465 = call "setfIRF.vi"("error in (no error)"=w929, "fIRF"=w919, "LaguerreDeconEngineClass in"=w930) -> ("error out"=w933:errorcluster, "LaguerreDeconEngineClass out"=w934:refnum<class "LaguerreDeconEngineClass.lvclass">)  [unwired: 7 in]
        n466 = call "setfIRF.vi"("error in (no error)"=w971, "fIRF"=w954, "LaguerreDeconEngineClass in"=w972) -> ("error out"=w975:errorcluster, "LaguerreDeconEngineClass out"=w976:refnum<class "LaguerreDeconEngineClass.lvclass">)  [unwired: 7 in]
        n467 = call "setfIRF.vi"("error in (no error)"=w981, "fIRF"=w941, "LaguerreDeconEngineClass in"=w982) -> ("error out"=w979:errorcluster, "LaguerreDeconEngineClass out"=w980:refnum<class "LaguerreDeconEngineClass.lvclass">)  [unwired: 7 in]
        n468 = Unbundle By Name(w961) -> ("V1"=w940:dbl[], "V2"=w960:dbl[], "V3"=w959:dbl[], "V4"=w926:dbl[])
        n469 = call "computeLCs.vi"("error in (no error)"=w979, "LaguerreDeconClass in"=w980) -> ("error out"=w977:errorcluster, "LaguerreDeconClass out"=w978:refnum<class "LaguerreDeconEngineClass.lvclass">)  [unwired: 8 in]
        n470 = call "computeLCs.vi"("error in (no error)"=w975, "LaguerreDeconClass in"=w976) -> ("error out"=w973:errorcluster, "LaguerreDeconClass out"=w974:refnum<class "LaguerreDeconEngineClass.lvclass">)  [unwired: 8 in]
        n471 = call "computeLCs.vi"("error in (no error)"=w969, "LaguerreDeconClass in"=w970) -> ("error out"=w967:errorcluster, "LaguerreDeconClass out"=w968:refnum<class "LaguerreDeconEngineClass.lvclass">)  [unwired: 8 in]
        n472 = call "computeLCs.vi"("error in (no error)"=w933, "LaguerreDeconClass in"=w934) -> ("error out"=w931:errorcluster, "LaguerreDeconClass out"=w932:refnum<class "LaguerreDeconEngineClass.lvclass">)  [unwired: 8 in]
        n473 = call-poly <vilib>:"Mean.vi"("X"=w940) -> ("mean"=w939:dbl)  [unwired: 1 out]
        n474 = call-poly <vilib>:"Mean.vi"("X"=w926) -> ("mean"=w925:dbl)  [unwired: 1 out]
        n475 = call-poly <vilib>:"Mean.vi"("X"=w960) -> ("mean"=w958:dbl)  [unwired: 1 out]
        n476 = call "getFitting.vi"("error in (no error)"=w977, "LaguerreDeconEngineClass in"=w978) -> ("Fitting"=w950:dbl[])  [unwired: 7 in, 2 out]
        n477 = call "getFitting.vi"("error in (no error)"=w973, "LaguerreDeconEngineClass in"=w974) -> ("Fitting"=w947:dbl[])  [unwired: 7 in, 2 out]
        n478 = call "getFitting.vi"("error in (no error)"=w967, "LaguerreDeconEngineClass in"=w968) -> ("Fitting"=w923:dbl[])  [unwired: 7 in, 2 out]
        n479 = call "getFitting.vi"("error in (no error)"=w931, "LaguerreDeconEngineClass in"=w932) -> ("Fitting"=w922:dbl[])  [unwired: 7 in, 2 out]
        n480 = Add(x=w951, y=w950) -> (x+y=w952:dbl[])
        n481 = Add(x=w948, y=w947) -> (x+y=w949:dbl[])
        n482 = call-poly <vilib>:"Mean.vi"("X"=w959) -> ("mean"=w957:dbl)  [unwired: 1 out]
        n483 = Add(x=w946, y=w923) -> (x+y=w945:dbl[])
        n484 = Build Array(w944, w952) -> (w964:dbl[][])
        n485 = Build Array(w943, w949) -> (w963:dbl[][])
        n486 = Build Array(w942, w945) -> (w962:dbl[][])
        n487 = Add(x=w921, y=w922) -> (x+y=w920:dbl[])
        n488 = Bundle("mean"=w939, "mean"=w958, "mean"=w957, "mean"=w925) -> (w924:T36)  [unwired: 1 in]
        n489 = Build Array(w917, w920) -> (w918:dbl[][])
        n490 = call "Calib_and_iRFAlign_confirm.vi"("Current V"=w924, "Ch4 Data"=w918, "Ch3 Data"=w962, "Ch2 Data"=w963, "Ch1 Data"=w964) -> ("Save?"=w956:bool)  [unwired: 6 in]
        n491 = case shown="True" w956 {
          tunnel: ["" ("Empty String Constant") "Data: saveCalibration\nData: saveiRF\nRun: CaliIncrement"] -> w955
          frame False {
          }
          frame True {
            # "[Covers: REQ2]"
          }
        }
        n492 = call <vilib>:"Add State(s) to Queue__JKI_lib_State_Machine.vi"("State(s) in Front (\"\")"=w955, "State(s) in (\"\")"=w1000) -> ("States Out"=w999:string)  [unwired: 13 in]
      }
      frame "Data: parseRunData" {
        # "All APD bias"
        # "flash queue"
        # "Ch3&4"
        # "Ch1&2"
        # "Flash data from queue and save it in structure\n()"
        n493 = Flush Queue(queue=w1028, error in (no error)=w1027) -> (remaining elements=w1022:T37, error out=w1023:errorcluster)  [unwired: 1 out]
        n494 = Flush Queue(queue=w1033, error in (no error)=w1027) -> (remaining elements=w1031:cluster{"double data":dbl[][]}[], error out=w1024:errorcluster)  [unwired: 1 out]
        n495 = Flush Queue(queue=w1034, error in (no error)=w1027) -> (remaining elements=w1032:cluster{"double data":dbl[][]}[], error out=w1025:errorcluster)  [unwired: 1 out]
        n496 = for {
          tunnel: w1032 -> [w1050] mode=indexing
          tunnel: [w1048] -> w1017 mode=concatenating
          tunnel: [w1047] -> w1018 mode=concatenating
          n497 = Unbundle By Name(w1050) -> ("double data"=w1049:dbl[][])
          n498 = call "SeperateChanData.vi"("Input (Ch1&2)"=w1049) -> ("Ch1"=w1048:dbl[][], "Ch2"=w1047:dbl[][])
        }
        n499 = for {
          tunnel: w1031 -> [w1046] mode=indexing
          tunnel: [w1045] -> w1007 mode=concatenating
          tunnel: [w1043] -> w1008 mode=concatenating
          n500 = Unbundle By Name(w1046) -> ("double data"=w1044:dbl[][])
          n501 = call "SeperateChanData.vi"("Input (Ch1&2)"=w1044) -> ("Ch1"=w1045:dbl[][], "Ch2"=w1043:dbl[][])
        }
        n502 = call "FLImDAQ_FGV.vi"() -> ("Read data"=w1015:T5)  [unwired: 10 in, 1 out]
        n503 = Unbundle By Name(w1015) -> ("Waveform to Avg"=w1005:i16)
        n504 = for {
          tunnel: w1022 -> [w1042] mode=indexing
          tunnel: [w1041] -> w1014 mode=indexing
          tunnel: [w1040] -> w1012 mode=indexing
          tunnel: [w1039] -> w1010 mode=indexing
          tunnel: [w1038] -> w1006 mode=indexing
          n505 = Unbundle By Name(w1042) -> ("V1"=w1041:dbl, "V2"=w1040:dbl, "V3"=w1039:dbl, "V4"=w1038:dbl)
        }
        n506 = call "DuplicateV(SubVI).vi"("Averaging"=w1005, "V in"=w1014) -> ("V out"=w1013:dbl[])  [unwired: 9 in]
        n507 = Array Size(array=w1007) -> (size(s)=→"data Size":i32[])
        n508 = call "DuplicateV(SubVI).vi"("Averaging"=w1005, "V in"=w1012) -> ("V out"=w1011:dbl[])  [unwired: 9 in]
        n509 = call "DuplicateV(SubVI).vi"("Averaging"=w1005, "V in"=w1010) -> ("V out"=w1009:dbl[])  [unwired: 9 in]
        n510 = call "DuplicateV(SubVI).vi"("Averaging"=w1005, "V in"=w1006) -> ("V out"=w1003:dbl[])  [unwired: 9 in]
        n511 = Bundle By Name(cluster=w1029, "Ch1Data"=w1017, "Ch2Data"=w1018, "Ch3Data"=w1007, "Ch4Data"=w1008, "V1"=w1013, "V2"=w1011, "V3"=w1009, "V4"=w1003) -> (w1030:T23)
        n512 = Merge Errors(w1025, w1024, w1023) -> (w1026:errorcluster)
        n513 = Array Size(array=w1013) -> (size(s)=→"V1 Size":i32)
        n514 = Array Size(array=w1011) -> (size(s)=→"V2 Size":i32)
        n515 = Array Size(array=w1009) -> (size(s)=→"V3 Size":i32)
        n516 = Array Size(array=w1003) -> (size(s)=→"V4 Size":i32)
        n517 = call <vilib>:"Add State(s) to Queue__JKI_lib_State_Machine.vi"("State(s) in (\"\")"=w1037) -> ("States Out"=w1036:string)  [unwired: 14 in]
      }
      frame "Data: saveRunData" {
        w1053 = T38 {"DataPath"=path "", "CaseID"="", "RunID"=0, "Ch1Data"=[], "Ch2Data"=[], "Ch3Data"=[], "Ch4Data"=[], "V1"=[], "V2"=[], "V3"=[], "V4"=[], "LaserRepRate"=0, "WFAverage"=0, "RunStartTime"=0}  # Data cluster
        # "Save FLIm data to disk.\n(Save to LV tdms file format)"
        n518 = Unbundle By Name(w1064) -> ("Pathes.DataPath"=w1060:path, "CaseID"=w1072:string, "IDs.RunID"=w1062:i8, "Ch1Data"=w1071:dbl[][], "Ch2Data"=w1070:dbl[][], "Ch3Data"=w1059:dbl[][], "Ch4Data"=w1052:dbl[][], "V1"=w1054:dbl[], "V2"=w1069:dbl[], "V3"=w1068:dbl[], "V4"=w1051:dbl[])
        n519 = call "FLImDAQ_FGV.vi"() -> ("Read data"=w1057:T5)  [unwired: 10 in, 1 out]
        n520 = Unbundle By Name(w1057) -> ("Waveform to Avg"=w1056:i16)
        n521 = local read "RunStartTime"() -> (w1055:u32)
        n522 = local read "Laser Rep Rate"() -> (w1058:dbl)
        n523 = Increment(x=w1062) -> (x+1=w1061:i8)
        n524 = Bundle By Name(cluster=w1053, "DataPath"=w1060, "CaseID"=w1072, "RunID"=w1061, "Ch1Data"=w1071, "Ch2Data"=w1070, "Ch3Data"=w1059, "Ch4Data"=w1052, "V1"=w1054, "V2"=w1069, "V3"=w1068, "V4"=w1051, "LaserRepRate"=w1058, "WFAverage"=w1056, "RunStartTime"=w1055) -> (w1067:T38)
        n525 = call "SaveRunData(SubVI).vi"("Data cluster"=w1067, "error in (no error)"=w1066) -> ("error out"=w1063:errorcluster)  [unwired: 13 in]
        n526 = flat-sequence {
          tunnel: w1064 -> [w1080]
          tunnel: [w1079] -> w1065
          tunnel: w1063 -> [_]
          frame #0 {
            w1077 = dbl[][] [] ("Ch1Data")
            w1078 = dbl[] [] ("V1")
            # "reset local data"
            n527 = Bundle By Name(cluster=w1080, "Ch1Data"=w1077, "Ch2Data"=w1077, "Ch3Data"=w1077, "Ch4Data"=w1077, "V1"=w1078, "V2"=w1078, "V3"=w1078, "V4"=w1078) -> (w1079:T23)
          }
        }
        n528 = case shown="No Error" w1063 {
          tunnel: ["Run: Increment" "" ("Empty String Constant")] -> w1073
          frame No Error {
          }
          frame Error {
          }
        }
        n529 = call <vilib>:"Add State(s) to Queue__JKI_lib_State_Machine.vi"("State(s) in Front (\"\")"=w1073, "State(s) in (\"\")"=w1076) -> ("States Out"=w1075:string)  [unwired: 13 in]
      }
      frame "Data: Cleanup" {
        # "Cleanup any data and references, here.\n(this is called automatically, by the Macro: Exit)"
        n530 = Unbundle By Name(w1084) -> ("Core.Current VI Reference"=w1087:refnum<vi>)
        n531 = Close Reference(reference=w1087, error in (no error)=w1086) -> (error out=w1085:errorcluster)
        n532 = call <vilib>:"Add State(s) to Queue__JKI_lib_State_Machine.vi"("State(s) in (\"\")"=w1089) -> ("States Out"=w1088:string)  [unwired: 14 in]
      }
      frame "---------- Core ----------" {
        # "Do not put any code in this frame.\n(it is a separator no-op)"
        n533 = call <vilib>:"Add State(s) to Queue__JKI_lib_State_Machine.vi"("State(s) in (\"\")"=w1094) -> ("States Out"=w1093:string)  [unwired: 14 in]
      }
      frame Default {
        w1105 = 42 items=["No error", "Argument error", "Memory is full", "Out of zone", "End of file", "File already open", "Generic file I/O error", "File not found", "File permission error", "Disk is full", "Duplicate path", "Too many files open", "System feature not enabled", "Resource file not found", "Cannot add resource", "Resource not found", "Image not found", "Image memory error", "Pen does not exist", "Config type invalid", "Config token not found", "Config parse error", "Config memory error", "Bad external code format", "Bad external code offset", "External code not present", "Null window", "Destroy window error", "Null menu", "Print aborted", "Bad print record", "Print driver error", "Windows error during printing", "Memory error during printing", "Print dialog error", "Generic print error", "Invalid device refnum", "Device not found", "Device parameter error", "Device unit error", "Cannot open device", "Device call aborted", "Generic error", "Cancelled by user", "Object ID too low", "Object ID too high", "Object not in heap", "Unknown heap", "Unknown object (invalid DefProc)", "Unknown object (DefProc not in table)", "Message out of range", "Invalid (null) method", "Unknown message", "Manager call not supported", "Bad address", "Network operation in progress", "Network operation timed out", "Connection is busy", "Network attribute not supported", "Network error", "Address in use", "System out of memory", "Connection aborted", "Connection refused", "Not connected", "Already connected", "Connection closed", "Initialization error (interapplication manager)", "Bad occurrence", "Wait on unbound occurrence handler", "Occurrence queue overflow", "Datalog type conflict", "Unused", "Unrecognized type (interapplication manager)", "Memory corrupt", "Failed to make temporary DLL", "Old CIN version", "Drag socket not found", "Failed to load drop-object", "Failed to register OLE object", "Failed to release OLE object", "Format specifier type mismatch", "Unknown format specifier", "Too few format specifiers", "Too many format specifiers", "Scan failed", "Newer CIN version", "Error converting to variant", "Runtime menu error", "Password tampered", "Variant attribute not found", "Incompatible variant data type", "Event data is not available", "Event Store is not present", "Occurrence is not found", "Event Queue is not created", "Event info is not available", "Refnum passed is NULL", "Error retrieving Class GUID", "Error retrieving CoClass GUID", "Error retrieving TypeLib GUID.", "Bad built application magic bytes.", "Specific driver is different from the specific driver associated with the Logical Name.", "There is no session opened to the class driver.", "Max Error", "MAX - Error with config objects", "MAX - Error loading configuration", "MAX - Group not supported"]
        # "Current State"
        # "Do not delete, rename, or modify this frame.\n(this is used to capture unhandled states and typos)"
        # "Handle mistyped state name (developer tool)"
        n534 = Format Into String(format string="Software Exception: Unhandled State \"%s\"." ("message"), error in=w1101, w1096) -> (resulting string=w1104:string, error out=w1103:errorcluster)  [unwired: 1 in]
        n535 = call <vilib>:"Error Cluster From Error Code.vi"("show call chain? (False)"=TRUE, "error in (no error)"=w1103, "error message (\"\")"=w1104, "error code (0)"=w1105) -> ("error out"=w1102:errorcluster)  [unwired: 5 in]
        n536 = call <vilib>:"Add State(s) to Queue__JKI_lib_State_Machine.vi"("State(s) in (\"\")"=w1100) -> ("States Out"=w1099:string)  [unwired: 14 in]
      }
      frame "Initialize Core Data" {
        # "Build default path based on the location of project"
        # "Do not delete, rename, or modify this frame.\n(this is used to determine panel behavior on exit)"
        # "originally closed?"
        # "exe?"
        # "If panel starts closed or is an EXE, then close it when we exit"
        n537 = call <vilib>:"Application Directory.vi"() -> ("Application Directory"=w1108:path)
        n538 = property on="Property Node" class="App"() -> ("App.Kind"=w1124:T18)  [unwired: 2 in, 2 out]
        n539 = property on="Property Node" class="VI"() -> ("FP.State"=w1118:T17)  [unwired: 2 in, 2 out]
        n540 = control-ref of="Current VI Reference"() -> (w1119:refnum<vi>)
        n541 = Equal?(x=w1118, y=T17."Closed" ("Front Panel Window:State")) -> (x = y?=w1116:bool)
        n542 = Strip Path(path=w1108) -> (stripped path=w1107:path)  [unwired: 1 out]
        n543 = Equal?(x=w1124, y=T18."Run Time System" ("Application:Kind")) -> (x = y?=w1122:bool)
        n544 = Build Path(base path=w1107, name or relative path="Data") -> (appended path=w1114:path)
        n545 = Build Path(base path=w1108, name or relative path="SystemTemp") -> (appended path=w1111:path)
        n546 = Build Path(base path=w1108, name or relative path="SystemCalibrationFile") -> (appended path=w1109:path)
        n547 = Or(x=w1116, y=w1122) -> (x .or. y?=w1120:bool)
        n548 = Bundle By Name(cluster=w1121, "Core.Current VI Reference"=w1119, "Core.Close Panel on Exit?"=w1120, "DefaultPath"=w1114, "TempPath"=w1111, "CaliPath"=w1109) -> (w1126:T23)
        n549 = call <vilib>:"Add State(s) to Queue__JKI_lib_State_Machine.vi"("State(s) in (\"\")"=w1128) -> ("States Out"=w1127:string)  [unwired: 14 in]
      }
      frame "Error Handler" {
        # "Unhandled Error -- Display it"
        # "Handle any errors here.\nYou can also output any states to clean-up after errors occur"
        # "Clear error"
        n550 = Unbundle By Name(w1129) -> ("code"=w1131:i32)
        n551 = case shown="Default" w1131 {
          tunnel: ["Macro: Exit" w1141 w1147] -> w1130
          tunnel: w1129 -> [w1137 _ _]
          frame Default {
            w1139 = T39 1 items=["no dialog", "OK message", "continue or stop message", "OK message + warnings", "continue/stop + warnings"] ("type of dialog (OK msg:1)")
            n552 = call <vilib>:"General Error Handler.vi"("type of dialog (OK msg:1)"=w1139, "error in (no error)"=w1137) -> ()  [unwired: 9 in, 5 out]
          }
          frame 5002 {
            n553 = Two Button Dialog(message="Laser interlock open! Please close interlock and try again! ", 1:"Safely Shutdown" ("F button name (\"Cancel\")"), 2:"OK" ("T button name (\"OK\")")) -> (T button?=w1142:bool)
            n554 = case shown="True" w1142 {
              tunnel: ["Macro: Exit" "355 Laser: CheckControllerStatus"] -> w1141
              frame False {
              }
              frame True {
              }
            }
          }
          frame 5001 {
            n555 = Two Button Dialog(message="Unable to connect to imaging computer, do you want to run data aquisiton alone? ", 1:"No" ("F button name (\"Cancel\")"), 2:"Yes" ("T button name (\"OK\")")) -> (T button?=w1148:bool)
            n556 = case shown="False" w1148 {
              tunnel: ["Macro: Exit" "" ("Empty String Constant")] -> w1147
              frame False {
              }
              frame True {
              }
            }
          }
        }
        n557 = call <vilib>:"Add State(s) to Queue__JKI_lib_State_Machine.vi"("State(s) in Front (\"\")"=w1130, "State(s) in (\"\")"=w1136) -> ("States Out"=w1135:string)  [unwired: 13 in]
      }
      frame "Exit" {
        # "Do not put any code in this frame.\n(No errors that occur here will be handled.)"
        n558 = call <vilib>:"Add State(s) to Queue__JKI_lib_State_Machine.vi"("State(s) in (\"\")"=w1159) -> ("States Out"=w1158:string)  [unwired: 14 in]
      }
      frame "---------- Case ----------" {
        # "Template Separator\n(You can make a copy of, or modify, this frame)"
        n559 = call <vilib>:"Add State(s) to Queue__JKI_lib_State_Machine.vi"("State(s) in (\"\")"=w1164) -> ("States Out"=w1163:string)  [unwired: 14 in]
      }
      frame "Case: getCaliID" {
        # "Get Calibration file #\n(You can make a copy of, or modify, this frame)"
        n560 = Unbundle By Name(w1165) -> ("Pathes.CaliPath"=w1168:path)
        n561 = call <vilib>:"Recursive File List.vi"("pattern"="*.tdms", "Treat LLBs as Folders?"=FALSE, "Folder Path"=w1168) -> ("All Files in Dir"=w1173:path[])  [unwired: 4 in, 4 out]
        n562 = for {
          tunnel: w1173 -> [w1183] mode=indexing
          tunnel: [w1182] -> w1172 mode=indexing
          tunnel: "Calibration" -> [w1179]
          n563 = Strip Path(path=w1183) -> (name=w1180:string)  [unwired: 1 out]
          n564 = Search and Replace String(input string=w1180, search string=w1179) -> (result string=w1178:string)  [unwired: 6 in, 3 out]
          n565 = Scan From String(format string="%d" ("string"), input string=w1178) -> (output 1=w1182:i32)  [unwired: 3 in, 3 out]
        }
        n566 = Array Max & Min(array=w1172) -> (max value=w1171:i32)  [unwired: 3 out]
        n567 = Bundle By Name(cluster=w1165, "IDs.Cali ID"=w1171) -> (w1166:T23)
        n568 = call <vilib>:"Add State(s) to Queue__JKI_lib_State_Machine.vi"("State(s) in (\"\")"=w1177) -> ("States Out"=w1176:string)  [unwired: 14 in]
      }
      frame "Case: getBGID" {
        # "Get background #\n(You can make a copy of, or modify, this frame)"
        n569 = Unbundle By Name(w1186) -> ("Pathes.BG Path"=w1191:path)
        n570 = call <vilib>:"Recursive File List.vi"("pattern"="*.tdms", "Treat LLBs as Folders?"=FALSE, "Folder Path"=w1191) -> ("All Files in Dir"=w1189:path[])  [unwired: 4 in, 4 out]
        n571 = for {
          tunnel: w1189 -> [w1206] mode=indexing
          tunnel: "Background" ("name or relative path") -> [w1204]
          shift-right: [w1197] -> w1184
          shift-left: 0 -> [w1201]
          n572 = Strip Path(path=w1206) -> (name=w1205:string)  [unwired: 1 out]
          n573 = Search and Replace String(input string=w1205, search string=w1204) -> (number of replacements=w1203:i32)  [unwired: 6 in, 3 out]
          n574 = Greater Than 0?(x=w1203) -> (x > 0?=w1202:bool)
          n575 = Select(t=1, s=w1202, f=0) -> (s? t:f=w1200:i32)
          n576 = Add(x=w1200, y=w1201) -> (x+y=w1197:i32)
        }
        n577 = Bundle By Name(cluster=w1186, "IDs.BG ID"=w1184) -> (w1187:T23)
        n578 = call <vilib>:"Add State(s) to Queue__JKI_lib_State_Machine.vi"("State(s) in (\"\")"=w1196) -> ("States Out"=w1195:string)  [unwired: 14 in]
      }
      frame "Case: getRunID" {
        # "Check folder for run ID\n(You can make a copy of, or modify, this frame)"
        n579 = Unbundle By Name(w1216) -> ("Pathes.DataPath"=w1215:path, "CaseID"=w1211:string)
        n580 = Build Array("Background" ("name or relative path"), "Calibration", "3DScanData" ("element")) -> (w1221:string[])
        n581 = call <vilib>:"Recursive File List.vi"("Folders to Exclude"=w1221, "pattern"="*.tdms", "Treat LLBs as Folders?"=FALSE, "Folder Path"=w1215) -> ("All Files in Dir"=w1212:path[])  [unwired: 3 in, 4 out]
        n582 = for {
          tunnel: w1212 -> [w1230] mode=indexing
          tunnel: [w1229] -> w1218 mode=indexing
          tunnel: w1211 -> [w1226]
          n583 = Strip Path(path=w1230) -> (name=w1227:string)  [unwired: 1 out]
          n584 = Search and Replace String(input string=w1227, search string=w1226) -> (result string=w1225:string)  [unwired: 6 in, 3 out]
          n585 = Scan From String(format string="_%d" ("string"), input string=w1225) -> (output 1=w1229:i32)  [unwired: 3 in, 3 out]
        }
        n586 = Array Max & Min(array=w1218) -> (max value=w1209:i32)  [unwired: 3 out]
        n587 = Bundle By Name(cluster=w1216, "IDs.RunID"=w1209) -> (w1217:T23)
        n588 = call "RunIDFGV.vi"("Error In"=w1207, "RunID in"=w1209) -> ("Error Out"=w1208:errorcluster)  [unwired: 8 in, 1 out]
        n589 = call <vilib>:"Add State(s) to Queue__JKI_lib_State_Machine.vi"("State(s) in (\"\")"=w1224) -> ("States Out"=w1223:string)  [unwired: 14 in]
      }
      frame "Case: CreatFileStruct" {
        # "Creat case file structure"
        n590 = Unbundle By Name(w1244) -> ("DefaultPath"=w1250:path, "CaseID"=w1237:string)
        n591 = Build Path(base path=w1250, name or relative path=w1237) -> (appended path=w1249:path)
        n592 = call <vilib>:"Check if File or Folder Exists.vi"("error in (no error)"=w1243, "path"=w1249) -> ("error out"=w1246:errorcluster, "file or folder exists?"=w1248:bool, "dup path"=w1247:path)  [unwired: 7 in]
        n593 = case shown="True" w1248 {
          tunnel: w1247 -> [w1267 w1275]
          tunnel: w1246 -> [w1265 w1270]
          tunnel: [w1259 w1275] -> w1235
          tunnel: [w1263 w1277] -> w1234
          tunnel: [u32 0 u32 0] -> w1233
          tunnel: [w1261 w1280] -> w1241
          tunnel: "Background" ("name or relative path") -> [w1260 w1272]
          tunnel: "Calibration" -> [w1258 w1271]
          tunnel: [w1254 w1273] -> w1238
          tunnel: w1237 -> [_ _]
          tunnel: ["" ("Empty String Constant") "Case: getRunID\nCase: getBGID\nCase: getCaliID\nUI: Update"] -> w1236
          frame False {
            # "Folder not exist. Creat folders."
            n594 = Create Folder(path (use dialog)=w1267, error in=w1265) -> (created path=w1259:path, error out=w1256:errorcluster)  [unwired: 1 in, 1 out]
            n595 = Build Path(base path=w1259, name or relative path=w1258) -> (appended path=w1257:path)
            n596 = Build Path(base path=w1259, name or relative path=w1260) -> (appended path=w1266:path)
            n597 = Create Folder(path (use dialog)=w1266, error in=w1256) -> (created path=w1261:path, error out=w1262:errorcluster)  [unwired: 1 in, 1 out]
            n598 = Create Folder(path (use dialog)=w1257, error in=w1256) -> (created path=w1254:path, error out=w1255:errorcluster)  [unwired: 1 in, 1 out]
            n599 = Merge Errors(w1262, w1255) -> (w1263:errorcluster)
          }
          frame True {
            # "Folder exsit, check file #"
            n600 = Build Path(base path=w1275, name or relative path=w1271) -> (appended path=w1276:path)
            n601 = Build Path(base path=w1275, name or relative path=w1272) -> (appended path=w1281:path)
            n602 = call <vilib>:"Check if File or Folder Exists.vi"("path"=w1276) -> ("file or folder exists?"=w1274:bool, "dup path"=w1273:path)  [unwired: 8 in, 1 out]
            n603 = call <vilib>:"Check if File or Folder Exists.vi"("path"=w1281) -> ("file or folder exists?"=w1279:bool, "dup path"=w1280:path)  [unwired: 8 in, 1 out]
            n604 = And(x=w1279, y=w1274) -> (x .and. y?=w1278:bool)
            n605 = case shown="False" w1278 {
              tunnel: w1270 -> [_ w1283]
              tunnel: [errorcluster {"status"=TRUE, "code"=5003, "source"="File structure error."} ("error out") w1283] -> w1277
              frame False {
              }
              frame True {
              }
            }
          }
        }
        n606 = Bundle By Name(cluster=w1244, "Pathes.DataPath"=w1235, "Pathes.BG Path"=w1241, "Pathes.CaliPath"=w1238, "IDs.RunID"=w1233, "IDs.BG ID"=w1233, "IDs.Cali ID"=w1233) -> (w1245:T23)
        n607 = call "DataRootPathFGV.vi"("Error In"=w1234, "PathIn"=w1235) -> ("Error Out"=w1232:errorcluster)  [unwired: 8 in, 1 out]
        n608 = call "RunIDFGV.vi"("Error In"=w1232, "RunID in"=w1233) -> ("Error Out"=w1231:errorcluster)  [unwired: 8 in, 1 out]
        n609 = call <vilib>:"Add State(s) to Queue__JKI_lib_State_Machine.vi"("State(s) in Front (\"\")"=w1236, "State(s) in (\"\")"=w1252) -> ("States Out"=w1251:string)  [unwired: 13 in]
      }
      frame "Case: GetID" {
        # "Template Separator\n(You can make a copy of, or modify, this frame)"
        n610 = call "set_subjectID.vi"() -> ("subject_id"=w1284:string)  [unwired: 10 in]
        n611 = Bundle By Name(cluster=w1286, "CaseID"=w1284) -> (w1287:T23)
        n612 = call <vilib>:"Add State(s) to Queue__JKI_lib_State_Machine.vi"("State(s) in (\"\")"=w1290) -> ("States Out"=w1289:string)  [unwired: 14 in]
      }
      frame "---------- DeconEngine ----------" {
        # "start data aquisition and then set irfAligh to ture and decon channel to 1,2 and 3."
        # "Template Separator\n(You can make a copy of, or modify, this frame)"
        n613 = call <vilib>:"Add State(s) to Queue__JKI_lib_State_Machine.vi"("State(s) in (\"\")"=w1295) -> ("States Out"=w1294:string)  [unwired: 14 in]
      }
      frame "DeconEngine: InitDotNet" {
        # "Initialize Dot Net Decon and save the FGV"
        # "Initilize Dot Net \n(You can make a copy of, or modify, this frame)"
        n614 = constructor on="Constructor Node" class="LaguerreDeCon"(error in=w1296) -> (reference out=w1299:refnum<k24>, error out=w1298:errorcluster)  [unwired: 2 in, 1 out]
        n615 = call "DotNetFGV.vi"("Error In"=w1298, "Operation (Read)"=enum16{"Read", "Write"}."Write", "reference in"=w1299) -> ("Error Out"=w1297:errorcluster)  [unwired: 7 in, 1 out]
        n616 = call <vilib>:"Add State(s) to Queue__JKI_lib_State_Machine.vi"("State(s) in (\"\")"=w1304) -> ("States Out"=w1303:string)  [unwired: 14 in]
      }
      frame "DeconEngine: Warmup" {
        # "Warm up parpool\n(You can make a copy of, or modify, this frame)"
        n617 = call "DotNetFGV.vi"("Error In"=w1309) -> ("Error Out"=w1310:errorcluster, "reference out"=w1311:refnum<k24>)  [unwired: 9 in]
        n618 = flat-sequence {
          tunnel: w1309 -> [_]
          tunnel: [w1317] -> w1306
          frame #0 {
            n619 = Tick Count (ms)() -> (millisecond timer value=w1317:u32)
          }
        }
        n620 = invoke class="LaguerreDeCon" method="init_parpool"(reference=w1311, error in=w1310) -> (error out=w1308:errorcluster)  [unwired: 1 in, 2 out]
        n621 = flat-sequence {
          tunnel: w1308 -> [_]
          tunnel: [w1316] -> w1307
          frame #0 {
            n622 = Tick Count (ms)() -> (millisecond timer value=w1316:u32)
          }
        }
        n623 = Subtract(x=w1307, y=w1306) -> (x-y=→"WarmupTime(ms)":u32)
        n624 = call <vilib>:"Add State(s) to Queue__JKI_lib_State_Machine.vi"("State(s) in (\"\")"=w1315) -> ("States Out"=w1314:string)  [unwired: 14 in]
      }
      frame "DeconEngine: loadIRF" {
        # "Load IRF for decon and save to FGV\n(You can make a copy of, or modify, this frame)"
        n625 = Current VI's Path() -> (path=w1335:path)
        n626 = Strip Path(path=w1335) -> (stripped path=w1334:path)  [unwired: 1 out]
        n627 = Build Path(base path=w1334, name or relative path="DotNetDecon") -> (appended path=w1322:path)
        n628 = Build Path(base path=w1322, name or relative path="Channel1.tdms") -> (appended path=w1339:path)
        n629 = Build Path(base path=w1322, name or relative path="Channel3.tdms") -> (appended path=w1324:path)
        n630 = Build Path(base path=w1322, name or relative path="Channel2.tdms") -> (appended path=w1325:path)
        n631 = call "LoadIRF.vi"("error in (no error)"=w1323, "file path"=w1339) -> ("error out"=w1337:errorcluster, "APD"=w1338:T40)  [unwired: 8 in]
        n632 = call "LoadIRF.vi"("error in (no error)"=w1323, "file path"=w1325) -> ("error out"=w1330:errorcluster, "APD"=w1331:T40)  [unwired: 8 in]
        n633 = call "LoadIRF.vi"("error in (no error)"=w1323, "file path"=w1324) -> ("error out"=w1327:errorcluster, "APD"=w1328:T40)  [unwired: 8 in]
        n634 = call "DeConAPD1FGV.vi"("Error In"=w1337, "Operation (Read)"=enum16{"Read", "Write"}."Write", "APDClass in"=w1338) -> ("Error Out"=w1321:errorcluster)  [unwired: 7 in, 1 out]
        n635 = call "DeConAPD2FGV.vi"("Error In"=w1330, "Operation (Read)"=enum16{"Read", "Write"}."Write", "APDClass in"=w1331) -> ("Error Out"=w1320:errorcluster)  [unwired: 7 in, 1 out]
        n636 = call "DeConAPD3FGV.vi"("Error In"=w1327, "Operation (Read)"=enum16{"Read", "Write"}."Write", "APDClass in"=w1328) -> ("Error Out"=w1319:errorcluster)  [unwired: 7 in, 1 out]
        n637 = Merge Errors(w1321, w1320, w1319) -> (w1318:errorcluster)
        n638 = call <vilib>:"Add State(s) to Queue__JKI_lib_State_Machine.vi"("State(s) in (\"\")"=w1345) -> ("States Out"=w1344:string)  [unwired: 14 in]
      }
      frame "DeconEngine: CloseNetRef" {
        # "Template Separator\n(You can make a copy of, or modify, this frame)"
        n639 = call "DotNetFGV.vi"("Error In"=w1346) -> ("Error Out"=w1348:errorcluster, "reference out"=w1349:refnum<k24>)  [unwired: 9 in]
        n640 = Close Reference(reference=w1349, error in (no error)=w1348) -> (error out=w1347:errorcluster)
        n641 = call <vilib>:"Add State(s) to Queue__JKI_lib_State_Machine.vi"("State(s) in (\"\")"=w1353) -> ("States Out"=w1352:string)  [unwired: 14 in]
      }
      frame "DeconEngine: InitilizeMacro" {
        # "start data aquisition and then set irfAligh to ture and decon channel to 1,2 and 3."
        # "Initilize Decon Engine for all channel\n(You can make a copy of, or modify, this frame)"
        n642 = call <vilib>:"Add State(s) to Queue__JKI_lib_State_Machine.vi"("State(s) in Front (\"\")"="DeconEngine: InitializeCh1\nDeconEngine: InitializeCh2\nDeconEngine: InitializeCh3\nDeconEngine: InitializeCh4" ("State(s) in Front (\"\")"), "State(s) in (\"\")"=w1359) -> ("States Out"=w1358:string)  [unwired: 13 in]
      }
      frame "DeconEngine: InitializeCh1" {
        w1381 = refnum<class "LaguerreDeconEngineClass.lvclass"> refnum  # Ch1DeconObj
        # "Initilize Laguerre Deconvolution engine Object\n(You can make a copy of, or modify, this frame)"
        n643 = global read "GlobalVariables.vi" "LastUseiRF"() -> (w1362:T15)
        n644 = call "setLaguerreOrder.vi"("error in (no error)"=w1369, "LaguerreOrder"=u32 12, "LaguerreDeconClass in"=w1381) -> ("error out"=w1378:errorcluster, "LaguerreDeconClass out"=w1379:refnum<class "LaguerreDeconEngineClass.lvclass">)  [unwired: 7 in]
        n645 = Unbundle By Name(w1362) -> ("Ch1 iRF"=w1361:dbl[])
        n646 = call "setDataLength.vi"("error in (no error)"=w1378, "dataLength"=u32 600, "LaguerreDeconClass in"=w1379) -> ("error out"=w1377:errorcluster, "LaguerreDeconClass out"=w1376:refnum<class "LaguerreDeconEngineClass.lvclass">)  [unwired: 7 in]
        n647 = call "setIRF.vi"("error in (no error)"=w1377, "iRF"=w1361, "LaguerreDeconClass in"=w1376) -> ("error out"=w1374:errorcluster, "LaguerreDeconClass out"=w1375:refnum<class "LaguerreDeconEngineClass.lvclass">)  [unwired: 7 in]
        n648 = call "computeAlpha.vi"("error in (no error)"=w1374, "LaguerreDeconClass in"=w1375) -> ("error out"=w1372:errorcluster, "LaguerreDeconClass out"=w1373:refnum<class "LaguerreDeconEngineClass.lvclass">)  [unwired: 8 in]
        n649 = call "dataInitilize.vi"("error in (no error)"=w1372, "LaguerreDeconClass in"=w1373) -> ("error out"=w1370:errorcluster, "LaguerreDeconClass out"=w1371:refnum<class "LaguerreDeconEngineClass.lvclass">)  [unwired: 8 in]
        n650 = call "computeDeconMatrix.vi"("error in (no error)"=w1370, "LaguerreDeconClass in"=w1371) -> ("error out"=w1366:errorcluster, "LaguerreDeconClass out"=w1368:refnum<class "LaguerreDeconEngineClass.lvclass">)  [unwired: 8 in]
        n651 = call "Ch1DeconEngineFGV.vi"("Error In"=w1366, "action(read)"=enum16{"write", "read"}."write" ("action"), "Ch1DeconEngine in"=w1368) -> ("Error Out"=w1365:errorcluster)  [unwired: 7 in, 1 out]
        n652 = call <vilib>:"Add State(s) to Queue__JKI_lib_State_Machine.vi"("State(s) in (\"\")"=w1383) -> ("States Out"=w1382:string)  [unwired: 14 in]
      }
      frame "DeconEngine: InitializeCh2" {
        w1405 = refnum<class "LaguerreDeconEngineClass.lvclass"> refnum  # Ch2DeconObj
        # "Initilize Laguerre Deconvolution engine Object\n(You can make a copy of, or modify, this frame)"
        n653 = global read "GlobalVariables.vi" "LastUseiRF"() -> (w1386:T15)
        n654 = call "setLaguerreOrder.vi"("error in (no error)"=w1393, "LaguerreOrder"=u32 12, "LaguerreDeconClass in"=w1405) -> ("error out"=w1402:errorcluster, "LaguerreDeconClass out"=w1403:refnum<class "LaguerreDeconEngineClass.lvclass">)  [unwired: 7 in]
        n655 = Unbundle By Name(w1386) -> ("Ch2 iRF"=w1385:dbl[])
        n656 = call "setDataLength.vi"("error in (no error)"=w1402, "dataLength"=u32 600, "LaguerreDeconClass in"=w1403) -> ("error out"=w1401:errorcluster, "LaguerreDeconClass out"=w1400:refnum<class "LaguerreDeconEngineClass.lvclass">)  [unwired: 7 in]
        n657 = call "setIRF.vi"("error in (no error)"=w1401, "iRF"=w1385, "LaguerreDeconClass in"=w1400) -> ("error out"=w1398:errorcluster, "LaguerreDeconClass out"=w1399:refnum<class "LaguerreDeconEngineClass.lvclass">)  [unwired: 7 in]
        n658 = call "computeAlpha.vi"("error in (no error)"=w1398, "LaguerreDeconClass in"=w1399) -> ("error out"=w1396:errorcluster, "LaguerreDeconClass out"=w1397:refnum<class "LaguerreDeconEngineClass.lvclass">)  [unwired: 8 in]
        n659 = call "dataInitilize.vi"("error in (no error)"=w1396, "LaguerreDeconClass in"=w1397) -> ("error out"=w1394:errorcluster, "LaguerreDeconClass out"=w1395:refnum<class "LaguerreDeconEngineClass.lvclass">)  [unwired: 8 in]
        n660 = call "computeDeconMatrix.vi"("error in (no error)"=w1394, "LaguerreDeconClass in"=w1395) -> ("error out"=w1390:errorcluster, "LaguerreDeconClass out"=w1392:refnum<class "LaguerreDeconEngineClass.lvclass">)  [unwired: 8 in]
        n661 = call "Ch2DeconEngineFGV.vi"("Error In"=w1390, "action(read)"=enum16{"write", "read"}."write" ("action"), "Ch2DeconEngine in"=w1392) -> ("Error Out"=w1389:errorcluster)  [unwired: 7 in, 1 out]
        n662 = call <vilib>:"Add State(s) to Queue__JKI_lib_State_Machine.vi"("State(s) in (\"\")"=w1407) -> ("States Out"=w1406:string)  [unwired: 14 in]
      }
      frame "DeconEngine: InitializeCh3" {
        w1409 = refnum<class "LaguerreDeconEngineClass.lvclass"> refnum  # Ch3DeconObj
        # "Initilize Laguerre Deconvolution engine Object\n(You can make a copy of, or modify, this frame)"
        n663 = global read "GlobalVariables.vi" "LastUseiRF"() -> (w1411:T15)
        n664 = call "setLaguerreOrder.vi"("error in (no error)"=w1418, "LaguerreOrder"=u32 12, "LaguerreDeconClass in"=w1409) -> ("error out"=w1427:errorcluster, "LaguerreDeconClass out"=w1428:refnum<class "LaguerreDeconEngineClass.lvclass">)  [unwired: 7 in]
        n665 = Unbundle By Name(w1411) -> ("Ch3 iRF"=w1410:dbl[])
        n666 = call "setDataLength.vi"("error in (no error)"=w1427, "dataLength"=600, "LaguerreDeconClass in"=w1428) -> ("error out"=w1426:errorcluster, "LaguerreDeconClass out"=w1425:refnum<class "LaguerreDeconEngineClass.lvclass">)  [unwired: 7 in]
        n667 = call "setIRF.vi"("error in (no error)"=w1426, "iRF"=w1410, "LaguerreDeconClass in"=w1425) -> ("error out"=w1423:errorcluster, "LaguerreDeconClass out"=w1424:refnum<class "LaguerreDeconEngineClass.lvclass">)  [unwired: 7 in]
        n668 = call "computeAlpha.vi"("error in (no error)"=w1423, "LaguerreDeconClass in"=w1424) -> ("error out"=w1421:errorcluster, "LaguerreDeconClass out"=w1422:refnum<class "LaguerreDeconEngineClass.lvclass">)  [unwired: 8 in]
        n669 = call "dataInitilize.vi"("error in (no error)"=w1421, "LaguerreDeconClass in"=w1422) -> ("error out"=w1419:errorcluster, "LaguerreDeconClass out"=w1420:refnum<class "LaguerreDeconEngineClass.lvclass">)  [unwired: 8 in]
        n670 = call "computeDeconMatrix.vi"("error in (no error)"=w1419, "LaguerreDeconClass in"=w1420) -> ("error out"=w1415:errorcluster, "LaguerreDeconClass out"=w1417:refnum<class "LaguerreDeconEngineClass.lvclass">)  [unwired: 8 in]
        n671 = call "Ch3DeconEngineFGV.vi"("Error In"=w1415, "action(read)"=enum16{"write", "read"}."write" ("action"), "Ch3DeconEngine in"=w1417) -> ("Error Out"=w1414:errorcluster)  [unwired: 7 in, 1 out]
        n672 = call <vilib>:"Add State(s) to Queue__JKI_lib_State_Machine.vi"("State(s) in (\"\")"=w1431) -> ("States Out"=w1430:string)  [unwired: 14 in]
      }
      frame "DeconEngine: InitializeCh4" {
        w1433 = refnum<class "LaguerreDeconEngineClass.lvclass"> refnum  # Ch3DeconObj
        # "Initilize Laguerre Deconvolution engine Object\n(You can make a copy of, or modify, this frame)"
        n673 = global read "GlobalVariables.vi" "LastUseiRF"() -> (w1435:T15)
        n674 = call "setLaguerreOrder.vi"("error in (no error)"=w1442, "LaguerreOrder"=u32 12, "LaguerreDeconClass in"=w1433) -> ("error out"=w1451:errorcluster, "LaguerreDeconClass out"=w1452:refnum<class "LaguerreDeconEngineClass.lvclass">)  [unwired: 7 in]
        n675 = Unbundle By Name(w1435) -> ("Ch4 iRF"=w1434:dbl[])
        n676 = call "setDataLength.vi"("error in (no error)"=w1451, "dataLength"=u32 600, "LaguerreDeconClass in"=w1452) -> ("error out"=w1450:errorcluster, "LaguerreDeconClass out"=w1449:refnum<class "LaguerreDeconEngineClass.lvclass">)  [unwired: 7 in]
        n677 = call "setIRF.vi"("error in (no error)"=w1450, "iRF"=w1434, "LaguerreDeconClass in"=w1449) -> ("error out"=w1447:errorcluster, "LaguerreDeconClass out"=w1448:refnum<class "LaguerreDeconEngineClass.lvclass">)  [unwired: 7 in]
        n678 = call "computeAlpha.vi"("error in (no error)"=w1447, "LaguerreDeconClass in"=w1448) -> ("error out"=w1445:errorcluster, "LaguerreDeconClass out"=w1446:refnum<class "LaguerreDeconEngineClass.lvclass">)  [unwired: 8 in]
        n679 = call "dataInitilize.vi"("error in (no error)"=w1445, "LaguerreDeconClass in"=w1446) -> ("error out"=w1443:errorcluster, "LaguerreDeconClass out"=w1444:refnum<class "LaguerreDeconEngineClass.lvclass">)  [unwired: 8 in]
        n680 = call "computeDeconMatrix.vi"("error in (no error)"=w1443, "LaguerreDeconClass in"=w1444) -> ("error out"=w1439:errorcluster, "LaguerreDeconClass out"=w1441:refnum<class "LaguerreDeconEngineClass.lvclass">)  [unwired: 8 in]
        n681 = call "Ch4DeconEngineFGV.vi"("Error In"=w1439, "action(read)"=enum16{"write", "read"}."write" ("action"), "Ch3DeconEngine in"=w1441) -> ("Error Out"=w1438:errorcluster)  [unwired: 7 in, 1 out]
        n682 = call <vilib>:"Add State(s) to Queue__JKI_lib_State_Machine.vi"("State(s) in (\"\")"=w1455) -> ("States Out"=w1454:string)  [unwired: 14 in]
      }
      frame "---------- Digitizer ----------" {
        # "Template Separator\n(You can make a copy of, or modify, this frame)"
        n683 = call <vilib>:"Add State(s) to Queue__JKI_lib_State_Machine.vi"("State(s) in (\"\")"=w1460) -> ("States Out"=w1459:string)  [unwired: 14 in]
      }
      frame "Digitizer: Initialize" {
        # "reset digitizer to everytime the system runs"
        # "reset digitizer to everytime the system runs"
        # "Initialize digitizer.\nInitialize both digitizer and update status."
        n684 = call "FLImDAQ_FGV.vi"("error in (no error)"=w1468) -> ("error out"=w1462:errorcluster, "Read data"=w1467:T5)  [unwired: 9 in]
        n685 = Unbundle By Name(w1470) -> ("SysConfigCluster.Ch1Enable?"=w1475:bool, "SysConfigCluster.Ch2Enable?"=w1474:bool, "SysConfigCluster.Ch3Enable?"=w1472:bool)
        n686 = Unbundle By Name(w1467) -> ("Digitizer 1"=w1463:refnum<k15>, "Digitizer 2"=w1466:refnum<k15>)
        n687 = property on="Digitizer" class="Bool (strict)"("Blinking"=TRUE) -> ()  [unwired: 2 in, 2 out]
        n688 = Or(x=w1475, y=w1474) -> (x .or. y?=w1473:bool)
        n689 = case shown="True" w1473 {
          tunnel: w1462 -> [w1483 w1486]
          tunnel: [w1483 w1485] -> w1464
          tunnel: w1463 -> [_ w1487]
          frame False {
          }
          frame True {
            n690 = call <instrlib>:"niScope Initialize.vi"("resource name"=w1487, "reset device"=TRUE, "error in"=w1486) -> ("error out"=w1485:errorcluster)  [unwired: 11 in, 1 out]
          }
        }
        n691 = case shown="True" w1472 {
          tunnel: w1462 -> [w1478 w1480]
          tunnel: [w1478 w1482] -> w1469
          tunnel: w1466 -> [_ w1481]
          frame False {
          }
          frame True {
            n692 = call <instrlib>:"niScope Initialize.vi"("resource name"=w1481, "reset device"=TRUE, "error in"=w1480) -> ("error out"=w1482:errorcluster)  [unwired: 11 in, 1 out]
          }
        }
        n693 = Merge Errors(w1464, w1469) -> (w1461:errorcluster)
        n694 = call <vilib>:"Add State(s) to Queue__JKI_lib_State_Machine.vi"("State(s) in (\"\")"=w1477) -> ("States Out"=w1476:string)  [unwired: 14 in]
      }
      frame "Digitizer: Config" {
        # "Synchronize is taking time ~3s."
        # "Config  digitizer\nCall subVi to config digitizer"
        n695 = call "FLImDAQ_FGV.vi"() -> ("Read data"=w1505:T5)  [unwired: 10 in, 1 out]
        n696 = Unbundle By Name(w1514) -> ("SysConfigCluster.Ch1Enable?"=w1522:bool, "SysConfigCluster.Ch2Enable?"=w1521:bool, "SysConfigCluster.Ch3Enable?"=w1519:bool, "FLImDAQ"=w1516:T30)
        n697 = Unbundle By Name(w1505) -> ("Digitizer 1"=w1508:refnum<k15>, "Digitizer 2"=w1507:refnum<k15>)
        n698 = property on="Digitizer" class="Bool (strict)"(error in=w1509, "Blinking"=TRUE) -> (error out=w1510:errorcluster)  [unwired: 1 in, 1 out]
        n699 = Or(x=w1522, y=w1521) -> (x .or. y?=w1520:bool)
        n700 = case shown="True" w1520 {
          tunnel: w1516 -> [_ w1535]
          tunnel: w1510 -> [w1531 w1534]
          tunnel: [w1531 w1533] -> w1517
          tunnel: w1508 -> [_ w1532]
          frame False {
          }
          frame True {
            n701 = call "DigitizerConfig.vi"("error in (no error)"=w1534, "FLImDAQ"=w1535, "IVI Refnum in"=w1532) -> ("error out"=w1533:errorcluster)  [unwired: 7 in, 1 out]
          }
        }
        n702 = case shown="True" w1519 {
          tunnel: w1516 -> [_ w1530]
          tunnel: w1517 -> [w1525 w1529]
          tunnel: [w1525 w1528] -> w1493
          tunnel: w1507 -> [_ w1526]
          frame False {
          }
          frame True {
            n703 = call "DigitizerConfig.vi"("Config Trigger? (T)"=FALSE ("Config Trigge(T)r:"), "error in (no error)"=w1529, "FLImDAQ"=w1530, "IVI Refnum in"=w1526) -> ("error out"=w1528:errorcluster)  [unwired: 6 in, 1 out]
          }
        }
        n704 = call "Digitizer1_FGV.vi"("error in (no error)"=w1493) -> ("error out"=w1503:errorcluster, "Read data"=w1504:refnum<k15>)  [unwired: 9 in]
        n705 = call <instrlib>:"niScope Get Session Reference.vi"("instrument handle"=w1504, "error in"=w1503) -> ("session reference"=w1497:refnum<k20>, "error out"=w1495:errorcluster)  [unwired: 11 in, 1 out]
        n706 = call "Digitizer2_FGV.vi"("error in (no error)"=w1495) -> ("error out"=w1501:errorcluster, "Read data"=w1502:refnum<k15>)  [unwired: 9 in]
        n707 = call <instrlib>:"niScope Get Session Reference.vi"("instrument handle"=w1502, "error in"=w1501) -> ("session reference"=w1496:refnum<k20>, "error out"=w1494:errorcluster)  [unwired: 11 in, 1 out]
        n708 = Build Array(w1497, w1496) -> (w1500:refnum<k20>[])
        n709 = call <instrlib>:"niTClk Configure For Homogeneous Triggers.vi"("error in (no error)"=w1494, "sessions"=w1500) -> ("error out"=w1499:errorcluster, "sessions out"=w1498:refnum<k20>[])  [unwired: 8 in]
        n710 = call <instrlib>:"niTClk Synchronize.vi"("error in (no error)"=w1499, "sessions"=w1498) -> ("error out"=w1492:errorcluster, "sessions out"=w1490:refnum<k20>[])  [unwired: 8 in]
        n711 = call <userlib>:"Wait (ms)__ogtk.vi"("error in (no error)"=w1492, "milliseconds to wait"=u32 1500) -> ("error out"=w1488:errorcluster)  [unwired: 8 in, 1 out]
        n712 = Unbundle By Name(w1488) -> ("status"=w1513:bool)
        n713 = Not(x=w1513) -> (.not. x?=w1512:bool)
        n714 = Bundle By Name(cluster=w1514, "System Status.Digitizer"=w1512, "niTClk sessions"=w1490) -> (w1515:T23)
        n715 = property on="Digitizer" class="Bool (strict)"(error in=w1488, "Blinking"=FALSE) -> (error out=w1506:errorcluster)  [unwired: 1 in, 1 out]
        n716 = call <vilib>:"Add State(s) to Queue__JKI_lib_State_Machine.vi"("State(s) in (\"\")"=w1524) -> ("States Out"=w1523:string)  [unwired: 14 in]
      }
      frame "Digitizer: Start" {
        # "send trigger to start acquisition loop"
        # "initilize aquisition"
        # "Start Digitizer\n(TClk start)"
        n717 = Unbundle By Name(w1543) -> ("niTClk sessions"=w1542:refnum<k20>[])
        n718 = call <instrlib>:"niTClk Initiate.vi"("error in (no error)"=w1536, "sessions"=w1542) -> ("error out"=w1538:errorcluster)  [unwired: 8 in, 1 out]
        n719 = Generate User Event(priority (normal)=usereventprio."high priority", user event=w1539, event data cluster=TRUE ("event data"), error in=w1538) -> (error out=w1537:errorcluster)  [unwired: 1 out]
        n720 = call <vilib>:"Add State(s) to Queue__JKI_lib_State_Machine.vi"("State(s) in (\"\")"=w1546) -> ("States Out"=w1545:string)  [unwired: 14 in]
      }
      frame "Digitizer: Abort" {
        # "Template Separator\n(You can make a copy of, or modify, this frame)"
        n721 = call "Digitizer1_FGV.vi"("error in (no error)"=w1550, "Operation (Read)"=enum16{"Write", "Read"}."Read" ("Operation")) -> ("error out"=w1557:errorcluster, "Read data"=w1554:refnum<k15>)  [unwired: 8 in]
        n722 = call "Digitizer2_FGV.vi"("error in (no error)"=w1550, "Operation (Read)"=enum16{"Write", "Read"}."Read" ("Operation")) -> ("error out"=w1553:errorcluster, "Read data"=w1555:refnum<k15>)  [unwired: 8 in]
        n723 = Bundle By Name(cluster=w1547, "SysRunning?"=FALSE ("System Status")) -> (w1548:T23)
        n724 = call <instrlib>:"niScope Abort.vi"("instrument handle"=w1554, "error in"=w1557) -> ("error out"=w1559:errorcluster)  [unwired: 12 in, 1 out]
        n725 = call <instrlib>:"niScope Abort.vi"("instrument handle"=w1555, "error in"=w1553) -> ("error out"=w1558:errorcluster)  [unwired: 12 in, 1 out]
        n726 = Merge Errors(w1559, w1558) -> (w1551:errorcluster)
        n727 = call <vilib>:"Add State(s) to Queue__JKI_lib_State_Machine.vi"("State(s) in (\"\")"=w1562) -> ("States Out"=w1561:string)  [unwired: 14 in]
      }
      frame "Digitizer: checkTemp" {
        w1565 = 65.0 ("y")
        w1570 = enum16{"Write", "Read"}."Read" ("Operation")
        # "Template Separator\n(You can make a copy of, or modify, this frame)"
        n728 = call "Digitizer1_FGV.vi"("Operation (Read)"=w1570) -> ("error out"=w1571:errorcluster, "Read data"=w1572:refnum<k15>)  [unwired: 9 in]
        n729 = call "Digitizer2_FGV.vi"("Operation (Read)"=w1570) -> ("error out"=w1568:errorcluster, "Read data"=w1569:refnum<k15>)  [unwired: 9 in]
        n730 = property on="Property Node" class="niScope"(reference=w1569, error in=w1568) -> ("Device Temperature"=w1566:dbl)  [unwired: 2 out]
        "Dig2 Temp" <- w1566
        n731 = property on="Property Node" class="niScope"(reference=w1572, error in=w1571) -> ("Device Temperature"=w1567:dbl)  [unwired: 2 out]
        "Dig1 Temp" <- w1567
        n732 = Greater?(x=w1567, y=w1565) -> (0:w1564:bool)
        n733 = Greater?(x=w1566, y=w1565) -> (0:w1563:bool)
        n734 = case shown="True" w1564 {
          frame False {
          }
          frame True {
            n735 = One Button Dialog(message="Digitizer 1 over heating!", button name ("OK")="OK") -> ()  [unwired: 1 out]
          }
        }
        n736 = case shown="True" w1563 {
          frame False {
          }
          frame True {
            n737 = One Button Dialog(message="Digitizer 2 over heating!", button name ("OK")="OK") -> ()  [unwired: 1 out]
          }
        }
        n738 = call <vilib>:"Add State(s) to Queue__JKI_lib_State_Machine.vi"("State(s) in (\"\")"=w1577) -> ("States Out"=w1576:string)  [unwired: 14 in]
      }
      frame "Digitizer: Close" {
        # "Close Digitizer"
        n739 = call "Digitizer1_FGV.vi"("error in (no error)"=w1587, "Operation (Read)"=enum16{"Write", "Read"}."Read" ("Operation")) -> ("error out"=w1589:errorcluster, "Read data"=w1593:refnum<k15>)  [unwired: 8 in]
        n740 = call "Digitizer2_FGV.vi"("error in (no error)"=w1587, "Operation (Read)"=enum16{"Write", "Read"}."Read" ("Operation")) -> ("error out"=w1588:errorcluster, "Read data"=w1591:refnum<k15>)  [unwired: 8 in]
        n741 = call <instrlib>:"niScope Close.vi"("instrument handle"=w1593, "error in"=w1589) -> ("error out"=w1586:errorcluster)  [unwired: 13 in]
        n742 = call <instrlib>:"niScope Close.vi"("instrument handle"=w1591, "error in"=w1588) -> ("error out"=w1585:errorcluster)  [unwired: 13 in]
        n743 = Merge Errors(w1586, w1585) -> (w1584:errorcluster)
        n744 = Unbundle By Name(w1584) -> ("status"=w1583:bool)
        n745 = Bundle By Name(cluster=w1594, "System Status.Digitizer"=w1583) -> (w1595:T23)
        n746 = call <vilib>:"Add State(s) to Queue__JKI_lib_State_Machine.vi"("State(s) in (\"\")"=w1597) -> ("States Out"=w1596:string)  [unwired: 14 in]
      }
      frame "---------- LabJack ----------" {
        # "Template Separator\n(You can make a copy of, or modify, this frame)"
        n747 = call <vilib>:"Add State(s) to Queue__JKI_lib_State_Machine.vi"("State(s) in (\"\")"=w1602) -> ("States Out"=w1601:string)  [unwired: 14 in]
      }
      frame "LabJack: checkPedal" {
        # "Template Separator\n(You can make a copy of, or modify, this frame)"
        n748 = Unbundle By Name(w1603) -> ("LJ Pinout.Foot Pedal"=w1607:string)
        n749 = call "LabJack_FGV.vi"("Operation(Read)"=enum16{"Write", "Read"}."Read" ("Operation"), "error in (no error)"=w1605) -> ("error out"=w1609:errorcluster, "Read data"=w1610:i32)  [unwired: 8 in]
        n750 = call "LJM_eReadName.vi"("Handle In"=w1610, "Name"=w1607, "error in"=w1609) -> ("Value"=w1608:dbl, "error out"=w1606:errorcluster)  [unwired: 10 in, 1 out]
        n751 = case shown="1" w1608 {
          tunnel: w1603 -> [w1615 w1618]
          tunnel: [w1615 w1616] -> w1604
          frame 0, Default {
          }
          frame 1 {
            # "If Pedal pressed"
            n752 = Tick Count (ms)() -> (millisecond timer value=w1622:u32)
            n753 = Unbundle By Name(w1618) -> ("Last Trigger"=w1617:u32)
            n754 = Subtract(x=w1622, y=w1617) -> (x-y=w1621:u32)
            n755 = Greater Or Equal?(x=w1621, y=u32 2000) -> (x >= y?=w1619:bool)
            n756 = case shown="True" w1619 {
              tunnel: w1618 -> [w1623 w1624]
              tunnel: w1617 -> [_ _]
              tunnel: [w1623 w1625] -> w1616
              frame False {
              }
              frame True {
                n757 = Tick Count (ms)() -> (millisecond timer value=w1626:u32)
                n758 = Unbundle By Name(w1624) -> ("SysRunning?"=w1627:bool)
                n759 = case shown="False" w1627 {
                  frame False {
                    n760 = property on="StartButton" class="Bool (strict)"("Val(Sgnl)"=TRUE ("Value (Signaling)")) -> ()  [unwired: 2 in, 2 out]
                  }
                  frame True {
                    n761 = property on="StopButton" class="Bool (strict)"("Val(Sgnl)"=TRUE ("Value (Signaling)")) -> ()  [unwired: 2 in, 2 out]
                  }
                }
                n762 = Bundle By Name(cluster=w1624, "Last Trigger"=w1626) -> (w1625:T23)
              }
            }
          }
        }
        n763 = call <vilib>:"Add State(s) to Queue__JKI_lib_State_Machine.vi"("State(s) in (\"\")"=w1614) -> ("States Out"=w1613:string)  [unwired: 14 in]
      }
      frame "LabJack: ZeroV" {
        # "Just Zero V\nDO not update FGV and front panel\nWIll resume from last V"
        # "set bias to 0"
        # "Zero APD bias\n(You can make a copy of, or modify, this frame)"
        n764 = Unbundle By Name(w1632) -> ("LJ Pinout.Ch1 Bias"=w1637:string, "LJ Pinout.Ch2 Bias"=w1636:string, "LJ Pinout.Ch3 Bias"=w1635:string)
        n765 = Build Array(w1637, w1636, w1635) -> (w1634:string[])
        n766 = call "LabJack_FGV.vi"("Operation(Read)"=enum16{"Write", "Read"}."Read" ("Operation"), "error in (no error)"=w1631) -> ("error out"=w1638:errorcluster, "Read data"=w1639:i32)  [unwired: 8 in]
        n767 = call "LJM_eWriteNames.vi"("Handle In"=w1639, "aNames"=w1634, "aValuesIn"=dbl[] [0.0, 0.0, 0.0], "error in"=w1638) -> ("error out"=w1630:errorcluster)  [unwired: 9 in, 2 out]
        n768 = call <vilib>:"Add State(s) to Queue__JKI_lib_State_Machine.vi"("State(s) in (\"\")"=w1643) -> ("States Out"=w1642:string)  [unwired: 14 in]
      }
      frame "LabJack: SetV" {
        w1650 = enum16{"write", "read"}."read" ("action (write)")
        # "set bias to user specifid"
        # "Set APD bias\n(You can make a copy of, or modify, this frame)"
        n769 = Unbundle By Name(w1659) -> ("LJ Pinout.Ch1 Bias"=w1663:string, "LJ Pinout.Ch2 Bias"=w1662:string, "LJ Pinout.Ch3 Bias"=w1661:string, "LJ Pinout.Ch4 Bias"=w1653:string)
        n770 = call "V2FGV.vi"("Error In"=w1649, "action(write)"=w1650) -> ("Error Out"=w1647:errorcluster, "V2 out"=w1655:dbl)  [unwired: 8 in]
        n771 = call "V4FGV.vi"("Error In"=w1649, "action(write)"=w1650) -> ("Error Out"=w1645:errorcluster, "V3 out"=w1651:dbl)  [unwired: 8 in]
        n772 = call "V1FGV.vi"("Error In"=w1649, "action (write)"=w1650) -> ("Error Out"=w1648:errorcluster, "V1 out"=w1652:dbl)  [unwired: 8 in]
        n773 = call "V3FGV.vi"("Error In"=w1649, "action(write)"=w1650) -> ("Error Out"=w1646:errorcluster, "V3 out"=w1654:dbl)  [unwired: 8 in]
        n774 = local write "V 3"(w1654) -> ()
        n775 = local write "V 2"(w1655) -> ()
        n776 = local write "V 4"(w1651) -> ()
        n777 = local write "V 1"(w1652) -> ()
        n778 = Build Array(w1663, w1662, w1661, w1653) -> (w1660:string[])
        n779 = call "LabJack_FGV.vi"("Operation(Read)"=enum16{"Write", "Read"}."Read" ("Operation"), "error in (no error)"=w1649) -> ("error out"=w1664:errorcluster, "Read data"=w1665:i32)  [unwired: 8 in]
        n780 = Build Array(w1652, w1655, w1654, w1651) -> (w1656:dbl[])
        n781 = call "LJM_eWriteNames.vi"("Handle In"=w1665, "aNames"=w1660, "aValuesIn"=w1656, "error in"=w1664) -> ("error out"=w1657:errorcluster)  [unwired: 9 in, 2 out]
        n782 = Merge Errors(w1648, w1647, w1646, w1645) -> (w1644:errorcluster)
        n783 = call <vilib>:"Add State(s) to Queue__JKI_lib_State_Machine.vi"("State(s) in (\"\")"=w1669) -> ("States Out"=w1668:string)  [unwired: 14 in]
        n784 = Merge Errors(w1644, w1657) -> (w1658:errorcluster)
      }
      frame "LabJack: Open" {
        # "Initialize LabJack T7\nEstablish connection and initialize pins"
        n785 = call "LJ_Open.vi"("error in"=w1679, "DeviceType"="LJM_dtT7") -> ("error out"=w1676:errorcluster, "Success?"=w1677:bool, "Handle Out"=w1671:i32)  [unwired: 7 in]
        n786 = call "LabJack_FGV.vi"("Operation(Read)"=enum16{"Write", "Read"}."Write" ("Operation"), "error in (no error)"=w1676, "Write data"=w1671) -> ("error out"=w1673:errorcluster)  [unwired: 7 in, 1 out]
        n787 = Bundle By Name(cluster=w1674, "System Status.Labjack"=w1677) -> (w1678:T23)
        n788 = call <vilib>:"Add State(s) to Queue__JKI_lib_State_Machine.vi"("State(s) in (\"\")"=w1681) -> ("States Out"=w1680:string)  [unwired: 14 in]
      }
      frame "LabJack: SetDefaultSub" {
        w1691 = enum16{"write", "read"}."write" ("action")
        w1692 = 0.0 ("V1 in")
        w1705 = "_EF_ENABLE" ("string")
        # "1. Disable PWM\n2. Set all V to 0\n3. Set 355 relay to open\n4. Set LED to off"
        # "read once to set DIO to input"
        # "set all initila V to 0. Set footpedal to input. Set PWM to low. Set laser relay to open. Set LEDs to yellow."
        # "Set Labjack to correct input and output state and initial values"
        n789 = disable-structure shown="Disabled" {
          frame Disabled {
            (unwired) dbl[] [0.0, 0.0, 0.0, 0.0, 0.0, 0.0, 0.0, 0.0, 0.0] ("aValuesIn")
          }
          frame Enabled {
          }
        }
        n790 = Unbundle By Name(w1702) -> ("LJ Pinout.355 PWM"=w1707:string, "LJ Pinout.AimingBeam PWM"=w1706:string, "LJ Pinout.Ch1 Bias"=w1712:string, "LJ Pinout.Ch2 Bias"=w1682:string, "LJ Pinout.Ch3 Bias"=w1716:string, "LJ Pinout.Ch4 Bias"=w1696:string, "LJ Pinout.Laser Start/Stop"=w1715:string, "LJ Pinout.Red LED"=w1714:string, "LJ Pinout.Green LED"=w1713:string)
        n791 = call "V1FGV.vi"("Error In"=w1700, "action (write)"=w1691, "V1 in"=w1692) -> ("Error Out"=w1695:errorcluster, "V1 out"=w1699:dbl)  [unwired: 7 in]
        n792 = local write "V 1"(w1699) -> ()
        n793 = call "V2FGV.vi"("Error In"=w1695, "action(write)"=w1691, "V2 in"=w1692) -> ("Error Out"=w1694:errorcluster, "V2 out"=w1698:dbl)  [unwired: 7 in]
        n794 = call "LabJack_FGV.vi"("Operation(Read)"=enum16{"Write", "Read"}."Read" ("Operation"), "error in (no error)"=w1700) -> ("error out"=w1688:errorcluster, "Read data"=w1710:i32)  [unwired: 8 in]
        n795 = Concatenate Strings(w1707, w1705) -> (w1704:string)
        n796 = Concatenate Strings(w1706, w1705) -> (w1703:string)
        n797 = local write "V 2"(w1698) -> ()
        n798 = call "V3FGV.vi"("Error In"=w1694, "action(write)"=w1691, "V3 in"=w1692) -> ("Error Out"=w1693:errorcluster, "V3 out"=w1697:dbl)  [unwired: 7 in]
        n799 = Build Array(w1704, w1703, w1712, w1682, w1716, w1696, w1715, w1714, w1713) -> (w1686:string[])
        n800 = local write "V 3"(w1697) -> ()
        n801 = call "V4FGV.vi"("Error In"=w1693, "action(write)"=w1691, "V3 in"=w1692) -> ("Error Out"=w1689:errorcluster, "V3 out"=w1690:dbl)  [unwired: 7 in]
        n802 = Array Size(array=w1686) -> (size(s)=w1685:i32)
        n803 = local write "V 4"(w1690) -> ()
        n804 = Initialize Array(0.0 ("element"), w1685) -> (w1683:dbl[])
        n805 = Unbundle By Name(w1702) -> ("LJ Pinout.Foot Pedal"=w1701:string)
        n806 = call "LJM_eWriteNames.vi"("Handle In"=w1710, "aNames"=w1686, "aValuesIn"=w1683, "error in"=w1688) -> ("Handle Out"=w1709:i32, "error out"=w1708:errorcluster)  [unwired: 9 in, 1 out]
        n807 = call "LJM_eReadName.vi"("Handle In"=w1709, "Name"=w1701, "error in"=w1708) -> ("error out"=w1687:errorcluster)  [unwired: 10 in, 2 out]
        n808 = case shown="Error .." w1687 {
          frame No Error {
            # "no error"
          }
          frame Error {
            # "handle error"
            n809 = One Button Dialog(message="Labjack error! The pin assignment is likely wrong. Please check pin setting of Labjack. Program will terminate.", button name ("OK")="OK") -> ()  [unwired: 1 out]
          }
        }
        n810 = call <vilib>:"Add State(s) to Queue__JKI_lib_State_Machine.vi"("State(s) in (\"\")"=w1719) -> ("States Out"=w1718:string)  [unwired: 14 in]
      }
      frame "LabJack: FootPedalConfig" {
        # "Setup footPedal\n(You can make a copy of, or modify, this frame)"
        n811 = call "LabJack_FGV.vi"("Operation(Read)"=enum16{"Write", "Read"}."Read" ("Operation"), "error in (no error)"=w1723) -> ("error out"=w1727:errorcluster, "Read data"=w1728:i32)  [unwired: 8 in]
        n812 = call "LJM_eWriteName.vi"("Handle In"=w1728, "Name"="DIO15", "Value"=1.0, "error in"=w1727) -> ("error out"=w1724:errorcluster)  [unwired: 10 in, 1 out]
        n813 = call <vilib>:"Add State(s) to Queue__JKI_lib_State_Machine.vi"("State(s) in (\"\")"=w1732) -> ("States Out"=w1731:string)  [unwired: 14 in]
      }
      frame "LabJack: SetDefaultAndClose" {
        # "Template Separator\n(You can make a copy of, or modify, this frame)"
        n814 = call <vilib>:"Add State(s) to Queue__JKI_lib_State_Machine.vi"("State(s) in Front (\"\")"="LabJack: SetDefaultSub\nLabJack: Close" ("State(s) in Front (\"\")"), "State(s) in (\"\")"=w1738) -> ("States Out"=w1737:string)  [unwired: 13 in]
      }
      frame "LabJack: Close" {
        # "Close LabJack Refnum"
        n815 = call "LabJack_FGV.vi"("Operation(Read)"=enum16{"Write", "Read"}."Read" ("Operation"), "error in (no error)"=w1744) -> ("error out"=w1739:errorcluster, "Read data"=w1740:i32)  [unwired: 8 in]
        n816 = Bundle By Name(cluster=w1742, "System Status.Labjack"=FALSE ("System Status.Gain Control")) -> (w1745:T23)
        n817 = call "LJM_Close.vi"("error in"=w1739, "Handle"=w1740) -> ("error out"=w1747:errorcluster)  [unwired: 9 in]
        n818 = call <vilib>:"Add State(s) to Queue__JKI_lib_State_Machine.vi"("State(s) in (\"\")"=w1749) -> ("States Out"=w1748:string)  [unwired: 14 in]
      }
      frame "LabJack: Interlock enable/disable" {
        w1758 = i8 0  # int8
        # "[Covers: REQ8]"
        # "Interlock enable/disable\n(Usage: \"LabJack: Interlock enable/disable >> 1|0\")"
        n819 = Fract/Exp String To Number(string=w1759, default (0 dbl)=w1758) -> (number=w1755:i8)  [unwired: 2 in, 1 out]
        n820 = Unbundle By Name(w1757) -> ("LJ Pinout.Interlock"=w1756:string)
        n821 = call "LabJack_FGV.vi"("Operation(Read)"=enum16{"Write", "Read"}."Read" ("Operation")) -> ("Read data"=w1753:i32)  [unwired: 9 in, 1 out]
        n822 = call "LJM_eWriteName.vi"("Handle In"=w1753, "Name"=w1756, "Value"=w1755, "error in"=w1754) -> ("error out"=w1751:errorcluster)  [unwired: 10 in, 1 out]
        n823 = call <vilib>:"Add State(s) to Queue__JKI_lib_State_Machine.vi"("State(s) in (\"\")"=w1761) -> ("States Out"=w1760:string)  [unwired: 14 in]
      }
      frame "LabJack: 355_PWM_Config" {
        w1763 = 0.0 ("element")
        w1783 = "DIO_EF_CLOCK1_ENABLE"
        # "Config PWM frequency"
        n824 = Unbundle By Name(w1775) -> ("LJ Pinout.355 PWM"=w1782:string)
        n825 = Unbundle By Name(w1775) -> ("355 PWM setting.DIO_EF_CLOCK1_DIVISOR"=w1774:i16, "355 PWM setting.DIO_EF_CLOCK1_ROLL_VALUE"=w1773:i32, "355 PWM setting.DIO#_EF_INDEX"=w1770:i16, "355 PWM setting.DIO#_EF_OPTIONS"=w1769:i16, "355 PWM setting.DIO#_EF_CONFIG_A"=w1768:i32)
        n826 = Concatenate Strings(w1782, "_EF_ENABLE" ("string")) -> (w1778:string)
        n827 = Concatenate Strings(w1782, "_EF_INDEX") -> (w1781:string)
        n828 = Concatenate Strings(w1782, "_EF_OPTIONS") -> (w1780:string)
        n829 = Concatenate Strings(w1782, "_EF_CONFIG_A") -> (w1779:string)
        n830 = call "LabJack_FGV.vi"("Operation(Read)"=enum16{"Write", "Read"}."Read" ("Operation")) -> ("Read data"=w1776:i32)  [unwired: 9 in, 1 out]
        n831 = Build Array(w1763, w1763, w1774, w1773, 1.0 ("element"), 0.0 ("element"), w1770, w1769, w1768) -> (w1767:dbl[])
        n832 = Build Array("DIO_EF_CLOCK0_ENABLE", w1783, "DIO_EF_CLOCK1_DIVISOR", "DIO_EF_CLOCK1_ROLL_VALUE", w1783, w1778, w1781, w1780, w1779) -> (w1777:string[])
        n833 = call "LJM_eWriteNames.vi"("Handle In"=w1776, "aNames"=w1777, "aValuesIn"=w1767, "error in"=w1765) -> ("error out"=w1766:errorcluster)  [unwired: 9 in, 2 out]
        n834 = call <vilib>:"Add State(s) to Queue__JKI_lib_State_Machine.vi"("State(s) in (\"\")"=w1792) -> ("States Out"=w1791:string)  [unwired: 14 in]
      }
      frame "LabJack: 355_PWM_Start" {
        # "Template Separator\n(You can make a copy of, or modify, this frame)"
        n835 = Unbundle By Name(w1800) -> ("LJ Pinout.355 PWM"=w1799:string)
        n836 = call "LabJack_FGV.vi"("Operation(Read)"=enum16{"Write", "Read"}."Read" ("Operation"), "error in (no error)"=w1794) -> ("error out"=w1801:errorcluster, "Read data"=w1802:i32)  [unwired: 8 in]
        n837 = Concatenate Strings(w1799, "_EF_ENABLE" ("string")) -> (w1797:string)
        n838 = call "LJM_eWriteName.vi"("Handle In"=w1802, "Name"=w1797, "Value"=1.0, "error in"=w1801) -> ("error out"=w1795:errorcluster)  [unwired: 10 in, 1 out]
        n839 = call <vilib>:"Add State(s) to Queue__JKI_lib_State_Machine.vi"("State(s) in (\"\")"=w1805) -> ("States Out"=w1804:string)  [unwired: 14 in]
      }
      frame "LabJack: 355_PWM_Stop" {
        # "Template Separator\n(You can make a copy of, or modify, this frame)"
        n840 = Unbundle By Name(w1811) -> ("LJ Pinout.355 PWM"=w1815:string)
        n841 = call "LabJack_FGV.vi"("Operation(Read)"=enum16{"Write", "Read"}."Read" ("Operation"), "error in (no error)"=w1810) -> ("error out"=w1816:errorcluster, "Read data"=w1808:i32)  [unwired: 8 in]
        n842 = Concatenate Strings(w1815, "_EF_ENABLE" ("string")) -> (w1813:string)
        n843 = call "LJM_eWriteName.vi"("Handle In"=w1808, "Name"=w1813, "Value"=0.0, "error in"=w1816) -> ("error out"=w1807:errorcluster)  [unwired: 10 in, 1 out]
        n844 = local write "355nm Laser toggle"(FALSE ("355nm Laser toggle")) -> ()
        n845 = call <vilib>:"Add State(s) to Queue__JKI_lib_State_Machine.vi"("State(s) in (\"\")"=w1819) -> ("States Out"=w1818:string)  [unwired: 14 in]
      }
      frame "LabJack: AB_Start" {
        # "Aiming Beam Start\n(Based on aimging beam frequency, set LabJack pin)"
        n846 = Unbundle By Name(w1829) -> ("AB Cluster.Freq"=w1821:i32, "LJ Pinout.AimingBeam PWM"=w1828:string)
        n847 = Greater Than 0?(x=w1821) -> (x > 0?=w1820:bool)
        n848 = case shown="False" w1820 {
          tunnel: w1828 -> [w1835 w1838]
          tunnel: [w1835 w1836] -> w1827
          frame False {
            # "if 0 freq, set PWM pin"
          }
          frame True {
            # "if non zero freq, set PWM enable"
            n849 = Concatenate Strings(w1838, "_EF_ENABLE" ("string")) -> (w1836:string)
          }
        }
        n850 = call "LabJack_FGV.vi"("Operation(Read)"=enum16{"Write", "Read"}."Read" ("Operation"), "error in (no error)"=w1824) -> ("error out"=w1830:errorcluster, "Read data"=w1831:i32)  [unwired: 8 in]
        n851 = call "LJM_eWriteName.vi"("Handle In"=w1831, "Name"=w1827, "Value"=1.0, "error in"=w1830) -> ("error out"=w1825:errorcluster)  [unwired: 10 in, 1 out]
        n852 = local write "Aiming beam toggle"(TRUE ("Aiming beam toggle")) -> ()
        n853 = call <vilib>:"Add State(s) to Queue__JKI_lib_State_Machine.vi"("State(s) in (\"\")"=w1834) -> ("States Out"=w1833:string)  [unwired: 14 in]
      }
      frame "LabJack: AB_Stop" {
        # "Aiming Beam Stop\n(Based on aiming beam frequency, set LabJack pin low)"
        n854 = Unbundle By Name(w1846) -> ("AB Cluster.Freq"=w1841:i32, "LJ Pinout.AimingBeam PWM"=w1848:string)
        n855 = Greater Than 0?(x=w1841) -> (x > 0?=w1840:bool)
        n856 = case shown="False" w1840 {
          tunnel: w1848 -> [w1854 w1857]
          tunnel: [w1854 w1855] -> w1839
          frame False {
          }
          frame True {
            n857 = Concatenate Strings(w1857, "_EF_ENABLE" ("string")) -> (w1855:string)
          }
        }
        n858 = call "LabJack_FGV.vi"("Operation(Read)"=enum16{"Write", "Read"}."Read" ("Operation"), "error in (no error)"=w1844) -> ("error out"=w1849:errorcluster, "Read data"=w1850:i32)  [unwired: 8 in]
        n859 = call "LJM_eWriteName.vi"("Handle In"=w1850, "Name"=w1839, "Value"=0.0, "error in"=w1849) -> ("error out"=w1845:errorcluster)  [unwired: 10 in, 1 out]
        n860 = local write "Aiming beam toggle"(FALSE ("Aiming beam toggle")) -> ()
        n861 = call <vilib>:"Add State(s) to Queue__JKI_lib_State_Machine.vi"("State(s) in (\"\")"=w1853) -> ("States Out"=w1852:string)  [unwired: 14 in]
      }
      frame "LabJack: AB_PWM_Config" {
        w1859 = 0.0 ("element")
        w1879 = "DIO_EF_CLOCK2_ENABLE"
        # "Config PWM frequency"
        n862 = Unbundle By Name(w1871) -> ("LJ Pinout.AimingBeam PWM"=w1878:string)
        n863 = Unbundle By Name(w1871) -> ("AB PWM setting.DIO_EF_CLOCK1_DIVISOR"=w1870:i16, "AB PWM setting.DIO_EF_CLOCK1_ROLL_VALUE"=w1869:i32, "AB PWM setting.DIO#_EF_INDEX"=w1866:i16, "AB PWM setting.DIO#_EF_OPTIONS"=w1865:i16, "AB PWM setting.DIO#_EF_CONFIG_A"=w1864:i32)
        n864 = Concatenate Strings(w1878, "_EF_ENABLE" ("string")) -> (w1874:string)
        n865 = Concatenate Strings(w1878, "_EF_INDEX") -> (w1877:string)
        n866 = Concatenate Strings(w1878, "_EF_OPTIONS") -> (w1876:string)
        n867 = Concatenate Strings(w1878, "_EF_CONFIG_A") -> (w1875:string)
        n868 = call "LabJack_FGV.vi"("Operation(Read)"=enum16{"Write", "Read"}."Read" ("Operation")) -> ("Read data"=w1872:i32)  [unwired: 9 in, 1 out]
        n869 = Build Array(w1859, w1859, w1870, w1869, 1.0 ("element"), 0.0 ("element"), w1866, w1865, w1864) -> (w1863:dbl[])
        n870 = Build Array("DIO_EF_CLOCK0_ENABLE", w1879, "DIO_EF_CLOCK2_DIVISOR", "DIO_EF_CLOCK2_ROLL_VALUE", w1879, w1874, w1877, w1876, w1875) -> (w1873:string[])
        n871 = call "LJM_eWriteNames.vi"("Handle In"=w1872, "aNames"=w1873, "aValuesIn"=w1863, "error in"=w1861) -> ("error out"=w1862:errorcluster)  [unwired: 9 in, 2 out]
        n872 = call <vilib>:"Add State(s) to Queue__JKI_lib_State_Machine.vi"("State(s) in (\"\")"=w1888) -> ("States Out"=w1887:string)  [unwired: 14 in]
      }
      frame "---------- LED ----------" {
        # "Template Separator\n(You can make a copy of, or modify, this frame)"
        n873 = call <vilib>:"Add State(s) to Queue__JKI_lib_State_Machine.vi"("State(s) in (\"\")"=w1893) -> ("States Out"=w1892:string)  [unwired: 14 in]
      }
      frame "LED: OpenVIRef" {
        # "Template Separator\n(You can make a copy of, or modify, this frame)"
        n874 = call <vilib>:"Application Directory.vi"() -> ("Application Directory"=w1900:path)
        n875 = Build Path(base path=w1900, name or relative path="SubVI") -> (appended path=w1898:path)
        n876 = Build Path(base path=w1898, name or relative path="LEDBreath.vi") -> (appended path=w1896:path)
        n877 = Open VI Reference(vi path=w1896, error in (no error)=w1901) -> (vi reference=w1902:refnum<vi>, error out=w1895:errorcluster)  [unwired: 4 in]
        n878 = case shown="Error .." w1895 {
          tunnel: [TRUE FALSE] -> w1894
          frame No Error {
          }
          frame Error {
          }
        }
        n879 = Bundle By Name(cluster=w1903, "LED vi reference"=w1902, "LED vi ref open?"=w1894) -> (w1904:T23)
        n880 = call <vilib>:"Add State(s) to Queue__JKI_lib_State_Machine.vi"("State(s) in (\"\")"=w1907) -> ("States Out"=w1906:string)  [unwired: 14 in]
      }
      frame "LED: CloseVIRef" {
        # "Template Separator\n(You can make a copy of, or modify, this frame)"
        n881 = Unbundle By Name(w1911) -> ("LED vi reference"=w1912:refnum<vi>, "LED vi ref open?"=w1910:bool)
        n882 = case shown="True" w1910 {
          tunnel: w1914 -> [w1918 w1921]
          tunnel: [w1918 w1920] -> w1913
          tunnel: w1912 -> [_ w1919]
          frame False {
          }
          frame True {
            n883 = Close Reference(reference=w1919, error in (no error)=w1921) -> (error out=w1920:errorcluster)
          }
        }
        n884 = call <vilib>:"Add State(s) to Queue__JKI_lib_State_Machine.vi"("State(s) in (\"\")"=w1917) -> ("States Out"=w1916:string)  [unwired: 14 in]
      }
      frame "LED: BreathGreen" {
        w1922 = FALSE ("Wait Until Done")
        # "Breath system LED\n(LED: Breath >> True/False)"
        n885 = Unbundle By Name(w1930) -> ("LED vi reference"=w1929:refnum<vi>)
        n886 = invoke class="VI" method="Ctrl Val.Set"(reference=w1929, error in=w1927, "Control Name"="Color", "Value"=0) -> (reference out=w1926:refnum<vi>, error out=w1925:errorcluster)  [unwired: 1 in, 3 out]
        n887 = invoke on="Invoke Node" class="VI" method="Run VI"(reference=w1926, error in=w1925, "Wait until done"=w1922, "Auto Dispose Ref"=w1922) -> (error out=w1928:errorcluster)  [unwired: 1 in, 4 out]
        n888 = call <vilib>:"Add State(s) to Queue__JKI_lib_State_Machine.vi"("State(s) in (\"\")"=w1933) -> ("States Out"=w1932:string)  [unwired: 14 in]
      }
      frame "LED: BreathOrange" {
        w1934 = FALSE ("Wait Until Done")
        # "Breath system LED\n(LED: Breath >> True/False)"
        n889 = Unbundle By Name(w1942) -> ("LED vi reference"=w1941:refnum<vi>)
        n890 = invoke class="VI" method="Ctrl Val.Set"(reference=w1941, error in=w1939, "Control Name"="Color", "Value"=1) -> (reference out=w1938:refnum<vi>, error out=w1937:errorcluster)  [unwired: 1 in, 3 out]
        n891 = invoke on="Invoke Node" class="VI" method="Run VI"(reference=w1938, error in=w1937, "Wait until done"=w1934, "Auto Dispose Ref"=w1934) -> (error out=w1940:errorcluster)  [unwired: 1 in, 4 out]
        n892 = call <vilib>:"Add State(s) to Queue__JKI_lib_State_Machine.vi"("State(s) in (\"\")"=w1945) -> ("States Out"=w1944:string)  [unwired: 14 in]
      }
      frame "LED: BreathOff" {
        # "System LED Breath Off\n(Breath off, check VI status to make sure it is off)"
        n893 = Unbundle By Name(w1954) -> ("LED vi reference"=w1953:refnum<vi>)
        n894 = invoke on="Invoke Node" class="VI" method="Ctrl Val.Set"(reference=w1953, error in=w1951, "Control Name"="Stop", "Value"=TRUE) -> (reference out=w1946:refnum<vi>, error out=w1947:errorcluster)  [unwired: 1 in, 3 out]
        n895 = case shown="No Error" w1947 {
          selector: w1947 -> [w1959 _]
          tunnel: [w1958 errorcluster {"status"=FALSE, "code"=0, "source"=""} ("error IO")] -> w1952
          tunnel: ["" ("State(s) in Front (\"\")") "LED: BreathOff" ("State(s) in Front (\"\")")] -> w1950
          tunnel: w1946 -> [w1960 _]
          frame No Error {
            # "No error, wait for VI to stop"
            n896 = while {
              tunnel: w1960 -> [w1968]
              shift-right: [w1962] -> w1958
              shift-left: w1959 -> [w1967]
              stop <- w1964 stop-if-true
              # "continue check whether vi is running"
              n897 = property class="VI"(reference=w1968, error in=w1967) -> (error out=w1962:errorcluster, "Exec.State"=w1966:T20)  [unwired: 1 out]
              n898 = Wait (ms)(milliseconds to wait=u32 50) -> ()  [unwired: 1 out]
              n899 = Equal?(x=w1966, y=T20."Idle") -> (x = y?=w1964:bool)
            }
          }
          frame Error {
            # "try again when error"
          }
        }
        n900 = call <vilib>:"Add State(s) to Queue__JKI_lib_State_Machine.vi"("State(s) in Front (\"\")"=w1950, "State(s) in (\"\")"=w1957) -> ("States Out"=w1956:string)  [unwired: 13 in]
      }
      frame "LED: Off" {
        # "set LED to red"
        # "Template Separator\n(You can make a copy of, or modify, this frame)"
        n901 = Unbundle By Name(w1973) -> ("LJ Pinout.Red LED"=w1972:string, "LJ Pinout.Green LED"=w1971:string)
        n902 = call "LabJack_FGV.vi"("Operation(Read)"=enum16{"Write", "Read"}."Read" ("Operation"), "error in (no error)"=w1974) -> ("error out"=w1981:errorcluster, "Read data"=w1980:i32)  [unwired: 8 in]
        n903 = call "LJM_eWriteName.vi"("Handle In"=w1980, "Name"=w1972, "Value"=0.0, "error in"=w1981) -> ("Handle Out"=w1978:i32, "error out"=w1977:errorcluster)  [unwired: 10 in]
        n904 = call "LJM_eWriteName.vi"("Handle In"=w1978, "Name"=w1971, "Value"=0.0, "error in"=w1977) -> ("error out"=w1975:errorcluster)  [unwired: 10 in, 1 out]
        n905 = call <vilib>:"Add State(s) to Queue__JKI_lib_State_Machine.vi"("State(s) in (\"\")"=w1985) -> ("States Out"=w1984:string)  [unwired: 14 in]
      }
      frame "LED: Green" {
        # "set LED to green"
        # "Template Separator\n(You can make a copy of, or modify, this frame)"
        n906 = Unbundle By Name(w1989) -> ("LJ Pinout.Red LED"=w1987:string, "LJ Pinout.Green LED"=w1988:string)
        n907 = call "LabJack_FGV.vi"("Operation(Read)"=enum16{"Write", "Read"}."Read" ("Operation"), "error in (no error)"=w1991) -> ("error out"=w1997:errorcluster, "Read data"=w1996:i32)  [unwired: 8 in]
        n908 = call "LJM_eWriteName.vi"("Handle In"=w1996, "Name"=w1987, "Value"=0.0, "error in"=w1997) -> ("Handle Out"=w1994:i32, "error out"=w1993:errorcluster)  [unwired: 10 in]
        n909 = call "LJM_eWriteName.vi"("Handle In"=w1994, "Name"=w1988, "Value"=9.0, "error in"=w1993) -> ("error out"=w1990:errorcluster)  [unwired: 10 in, 1 out]
        n910 = call <vilib>:"Add State(s) to Queue__JKI_lib_State_Machine.vi"("State(s) in (\"\")"=w2000) -> ("States Out"=w1999:string)  [unwired: 14 in]
      }
      frame "---------- Queue ----------" {
        # "Template Separator\n(You can make a copy of, or modify, this frame)"
        n911 = call <vilib>:"Add State(s) to Queue__JKI_lib_State_Machine.vi"("State(s) in (\"\")"=w2005) -> ("States Out"=w2004:string)  [unwired: 14 in]
      }
      frame "Queue: Flash" {
        # "Clear queue contnet\n(clear queue content by flash it)"
        n912 = Flush Queue(queue=w2012, error in (no error)=w2006) -> (error out=w2010:errorcluster)  [unwired: 2 out]
        n913 = Flush Queue(queue=w2013, error in (no error)=w2006) -> (error out=w2009:errorcluster)  [unwired: 2 out]
        n914 = Flush Queue(queue=w2011, error in (no error)=w2006) -> (error out=w2008:errorcluster)  [unwired: 2 out]
        n915 = Merge Errors(w2010, w2009, w2008) -> (w2007:errorcluster)
        n916 = call <vilib>:"Add State(s) to Queue__JKI_lib_State_Machine.vi"("State(s) in (\"\")"=w2017) -> ("States Out"=w2016:string)  [unwired: 14 in]
      }
      frame "Queue: Destory" {
        # "Destory Data Queue\nDistory data queue ref so the aquisition loop stop"
        n917 = Release Queue(queue=w2023, error in (no error)=w2019) -> (error out=w2026:errorcluster)  [unwired: 1 in, 2 out]
        n918 = Release Queue(queue=w2022, error in (no error)=w2019) -> (error out=w2025:errorcluster)  [unwired: 1 in, 2 out]
        n919 = Release Queue(queue=w2020, error in (no error)=w2019) -> (error out=w2018:errorcluster)  [unwired: 1 in, 2 out]
        n920 = Merge Errors(w2026, w2025, w2018) -> (w2024:errorcluster)
        n921 = call <vilib>:"Simple Error Handler.vi"("error in (no error)"=w2024) -> ()  [unwired: 4 in, 5 out]
        n922 = call <vilib>:"Add State(s) to Queue__JKI_lib_State_Machine.vi"("State(s) in (\"\")"=w2029) -> ("States Out"=w2028:string)  [unwired: 14 in]
      }
      frame "---------- Run ----------" {
        # "Template Separator\n(You can make a copy of, or modify, this frame)"
        n923 = call <vilib>:"Add State(s) to Queue__JKI_lib_State_Machine.vi"("State(s) in (\"\")"=w2034) -> ("States Out"=w2033:string)  [unwired: 14 in]
      }
      frame "Run: CaliIncrement" {
        # "Increment Calibration #\n(You can make a copy of, or modify, this frame)"
        n924 = Unbundle By Name(w2036) -> ("IDs.Cali ID"=w2038:i8)
        n925 = Increment(x=w2038) -> (x+1=w2035:i8)
        n926 = Bundle By Name(cluster=w2036, "IDs.Cali ID"=w2035) -> (w2037:T23)
        n927 = call <vilib>:"Add State(s) to Queue__JKI_lib_State_Machine.vi"("State(s) in (\"\")"=w2042) -> ("States Out"=w2041:string)  [unwired: 14 in]
      }
      frame "Run: BGIncrement" {
        # "Increment BG #\n(You can make a copy of, or modify, this frame)"
        n928 = Unbundle By Name(w2043) -> ("IDs.BG ID"=w2046:i8)
        n929 = Increment(x=w2046) -> (x+1=w2045:i8)
        n930 = Bundle By Name(cluster=w2043, "IDs.BG ID"=w2045) -> (w2044:T23)
        n931 = call <vilib>:"Add State(s) to Queue__JKI_lib_State_Machine.vi"("State(s) in (\"\")"=w2050) -> ("States Out"=w2049:string)  [unwired: 14 in]
      }
      frame "Run: Increment" {
        # "Increase Run# by 1"
        n932 = Unbundle By Name(w2055) -> ("IDs.RunID"=w2057:i8)
        n933 = Increment(x=w2057) -> (x+1=w2053:i8)
        n934 = Bundle By Name(cluster=w2055, "IDs.RunID"=w2053) -> (w2056:T23)
        n935 = call "RunIDFGV.vi"("Error In"=w2051, "RunID in"=w2053) -> ("Error Out"=w2052:errorcluster)  [unwired: 8 in, 1 out]
        n936 = call <vilib>:"Add State(s) to Queue__JKI_lib_State_Machine.vi"("State(s) in (\"\")"=w2059) -> ("States Out"=w2058:string)  [unwired: 14 in]
      }
      frame "Run: Decrement" {
        # "Increase Run# by 1"
        n937 = Unbundle By Name(w2064) -> ("IDs.RunID"=w2066:i8)
        n938 = Decrement(x=w2066) -> (x-1=w2062:i8)
        n939 = Bundle By Name(cluster=w2064, "IDs.RunID"=w2062) -> (w2065:T23)
        n940 = call "RunIDFGV.vi"("Error In"=w2060, "RunID in"=w2062) -> ("Error Out"=w2061:errorcluster)  [unwired: 8 in, 1 out]
        n941 = call <vilib>:"Add State(s) to Queue__JKI_lib_State_Machine.vi"("State(s) in (\"\")"=w2068) -> ("States Out"=w2067:string)  [unwired: 14 in]
      }
      frame "---------- SysConfig ----------" {
        # "Template Separator\n(You can make a copy of, or modify, this frame)"
        n942 = call <vilib>:"Add State(s) to Queue__JKI_lib_State_Machine.vi"("State(s) in (\"\")"=w2073) -> ("States Out"=w2072:string)  [unwired: 14 in]
      }
      frame "SysConfig: LoadAPDSerialNumber" {
        # "Template Separator\n(You can make a copy of, or modify, this frame)"
        n943 = call "readAPDSerial.vi"("Error In"=w2075) -> ("Error Out"=w2074:errorcluster, "output cluster"=w2076:T26)  [unwired: 9 in]
        n944 = Bundle By Name(cluster=w2077, "APDSerialNum"=w2076) -> (w2078:T23)
        n945 = call <vilib>:"Add State(s) to Queue__JKI_lib_State_Machine.vi"("State(s) in (\"\")"=w2081) -> ("States Out"=w2080:string)  [unwired: 14 in]
      }
      frame "SysConfig: Load Sys Config" {
        # "[Covers: REQ5]"
        # "Load System config"
        # "Load system configuration\n(Load both hardware and DAQ config)"
        n946 = call "LoadSysConfig.vi"("Error In"=w2084, "Enum"=enum16{"LastUse", "Default"}."LastUse") -> ("Error Out"=w2083:errorcluster, "SysConfigCluster"=w2086:T7)  [unwired: 8 in]
        "SysConfigCluster" <- w2086
        n947 = Bundle By Name(cluster=w2087, "SysConfigCluster"=w2086) -> (w2088:T23)
        n948 = call <vilib>:"Add State(s) to Queue__JKI_lib_State_Machine.vi"("State(s) in (\"\")"=w2090) -> ("States Out"=w2089:string)  [unwired: 14 in]
      }
      frame "SysConfig: Load Digitizer Setting" {
        w2091 = enum16{"Write", "Read"}."Write" ("Operation")
        # "Load DAQ config\nSave to FGV"
        # "Template Separator\n(You can make a copy of, or modify, this frame)"
        n949 = call <userlib>:"Current VIs Parent Directory__ogtk.vi"() -> ("Parent Directory (+ Relative)"=w2105:path)  [unwired: 5 in]
        n950 = Build Path(base path=w2105, name or relative path="SubVI\\DigitizerConfiguration\\V6_Scope_last_use.config") -> (appended path=w2106:path)
        n951 = call "ReadDigitizerConfig(SubVI).vi"("error in (no error)"=w2103, "appended path"=w2106) -> ("error out"=w2099:errorcluster, "FLImDAQ"=w2097:T5)  [unwired: 8 in]
        n952 = call "FLImDAQ_FGV.vi"("error in (no error)"=w2099, "Operation (Read)"=w2091, "Write data"=w2097) -> ("error out"=w2101:errorcluster)  [unwired: 7 in, 1 out]
        n953 = Unbundle By Name(w2097) -> ("min record length"=→"data length":i32, "Digitizer 1"=w2093:refnum<k15>, "Digitizer 2"=w2100:refnum<k15>)
        n954 = Bundle By Name(cluster=w2095, "FLImDAQ"=w2097) -> (w2096:T23)
        n955 = call "Digitizer1_FGV.vi"("error in (no error)"=w2101, "Operation (Read)"=w2091, "Write data"=w2093) -> ("error out"=w2102:errorcluster)  [unwired: 7 in, 1 out]
        n956 = call "Digitizer2_FGV.vi"("error in (no error)"=w2102, "Operation (Read)"=w2091, "Write data"=w2100) -> ("error out"=w2098:errorcluster)  [unwired: 7 in, 1 out]
        n957 = call <vilib>:"Add State(s) to Queue__JKI_lib_State_Machine.vi"("State(s) in (\"\")"=w2108) -> ("States Out"=w2107:string)  [unwired: 14 in]
      }
      frame "SysConfig: Load LJ Pinout" {
        # "Template Separator\n(You can make a copy of, or modify, this frame)"
        n958 = call <userlib>:"Current VIs Parent Directory__ogtk.vi"() -> ("Parent Directory (+ Relative)"=w2123:path)  [unwired: 5 in]
        n959 = Build Path(base path=w2123, name or relative path="SubVI\\LabJack\\LJ_pin_setting.config") -> (appended path=w2121:path)
        n960 = call "ReadLabjackConfig(SubVI).vi"("error in (no error)"=w2119, "appended path"=w2121) -> ("error out"=w2120:errorcluster, "Utility"=w2117:T4)  [unwired: 8 in]
        n961 = Unbundle By Name(w2117) -> ("Ch1 Bias"=w2116:string, "Ch2 Bias"=w2115:string, "Ch3 Bias"=w2114:string, "Ch4 Bias"=w2109:string, "Red LED"=w2111:string, "Green LED"=w2110:string)
        n962 = global write "GlobalVariables.vi" "LED Green pin"(w2110) -> ()
        n963 = global write "GlobalVariables.vi" "Ch1 LJ pin"(w2116) -> ()
        n964 = global write "GlobalVariables.vi" "Ch2 LJ pin"(w2115) -> ()
        n965 = global write "GlobalVariables.vi" "Ch3 LJ pin"(w2114) -> ()
        n966 = global write "GlobalVariables.vi" "Ch4 LJ pin"(w2109) -> ()
        n967 = global write "GlobalVariables.vi" "LED Red pin"(w2111) -> ()
        n968 = Bundle By Name(cluster=w2112, "LJ Pinout"=w2117) -> (w2118:T23)
        n969 = call <vilib>:"Add State(s) to Queue__JKI_lib_State_Machine.vi"("State(s) in (\"\")"=w2125) -> ("States Out"=w2124:string)  [unwired: 14 in]
      }
      frame "SysConfig: Load 355 PWM" {
        # "Template Separator\n(You can make a copy of, or modify, this frame)"
        n970 = call <userlib>:"Current VIs Parent Directory__ogtk.vi"() -> ("Parent Directory (+ Relative)"=w2143:path)  [unwired: 5 in]
        n971 = Build Path(base path=w2143, name or relative path="SubVI\\LabJack\\PWM_setting_355.config") -> (appended path=w2141:path)
        n972 = call "ReadPWMConfig(SubVI).vi"("error in (no error)"=w2138, "appended path"=w2141) -> ("error out"=w2139:errorcluster, "PWM Setting"=w2137:T41)  [unwired: 8 in]
        n973 = Unbundle By Name(w2137) -> ("DIO_EF_CLOCK1_DIVISOR"=w2134:i16, "DIO_EF_CLOCK1_ROLL_VALUE"=w2133:i32)
        n974 = Multiply(x=w2134, y=w2133) -> (x*y=w2135:i32)
        n975 = Bundle By Name(cluster=w2140, "355 PWM setting"=w2137) -> (w2127:T23)
        n976 = Divide(x=80000000.0, y=w2135) -> (x/y=w2132:dbl)
        "Laser Rep Rate" <- w2132
        n977 = Number To Decimal String(number=w2132) -> (decimal integer string=w2131:string)  [unwired: 1 in]
        n978 = Concatenate Strings("355nm " ("string"), w2131, "Hz" ("string")) -> (w2129:string)
        n979 = property on="355nm Laser toggle" class="Bool (strict)"("Caption.Text"=w2129) -> ()  [unwired: 2 in, 2 out]
        n980 = call <vilib>:"Add State(s) to Queue__JKI_lib_State_Machine.vi"("State(s) in (\"\")"=w2145) -> ("States Out"=w2144:string)  [unwired: 14 in]
      }
      frame "SysConfig: Load AB PWM" {
        # "Template Separator\n(You can make a copy of, or modify, this frame)"
        n981 = call <userlib>:"Current VIs Parent Directory__ogtk.vi"() -> ("Parent Directory (+ Relative)"=w2154:path)  [unwired: 5 in]
        n982 = Build Path(base path=w2154, name or relative path="SubVI\\LabJack\\PWM_setting_AB.config") -> (appended path=w2152:path)
        n983 = call "ReadPWMConfig(SubVI).vi"("error in (no error)"=w2149, "appended path"=w2152) -> ("error out"=w2150:errorcluster, "PWM Setting"=w2148:T41)  [unwired: 8 in]
        n984 = Bundle By Name(cluster=w2146, "AB PWM setting"=w2148) -> (w2151:T23)
        n985 = call <vilib>:"Add State(s) to Queue__JKI_lib_State_Machine.vi"("State(s) in (\"\")"=w2156) -> ("States Out"=w2155:string)  [unwired: 14 in]
      }
      frame "SysConfig: Load AB setting" {
        # "load aming beam setting\n(check frequency, if 0 do nothing, if not zero, config PWM)"
        n986 = call "readAimingBeamSetting.vi"("error in (no error)"=w2170) -> ("error out"=w2165:errorcluster, "Aiming Beam Setting"=w2158:T42)  [unwired: 9 in]
        n987 = Unbundle By Name(w2158) -> ("Frequency(Hz)"=w2157:u32)
        n988 = Equal To 0?(x=w2157) -> (x = 0?=w2163:bool)
        n989 = Select(t="", s=w2163, f="SysConfig: Load AB PWM" ("State(s) in Front (\"\")")) -> (s? t:f=w2166:string)
        n990 = Number To Decimal String(number=w2157) -> (decimal integer string=w2162:string)  [unwired: 1 in]
        n991 = Concatenate Strings("488nm " ("string"), w2162, "Hz " ("string")) -> (w2161:string)
        n992 = property on="Aiming beam toggle" class="Bool (strict)"("Caption.Text"=w2161) -> ()  [unwired: 2 in, 2 out]
        n993 = case shown="False" w2163 {
          tunnel: w2165 -> [w2178 w2181]
          tunnel: [w2177 w2181] -> w2164
          tunnel: w2157 -> [w2176 _]
          frame False {
            n994 = call "LJ_calculate_PWM_parameters.vi"("Duty Cycle (%)"=u32 10, "Error In"=w2178, "Show Confirmation"=FALSE, "Laser Rep Rate (Hz)"=w2176, "Laser"=enum16{"355nm", "AimingBeam"}."AimingBeam") -> ("Error Out"=w2177:errorcluster)  [unwired: 5 in, 1 out]
          }
          frame True {
          }
        }
        n995 = Bundle By Name(cluster=w2171, "AB Cluster"=w2158) -> (w2172:T23)
        n996 = call <vilib>:"Add State(s) to Queue__JKI_lib_State_Machine.vi"("State(s) in Front (\"\")"=w2166, "State(s) in (\"\")"=w2174) -> ("States Out"=w2173:string)  [unwired: 13 in]
      }
      frame "SysConfig: LoadABVideoSetting" {
        # "Load AB video setting form ini file\n()"
        n997 = call "readVideoConfig.vi"("error in (no error)"=w2185) -> ("error out"=w2186:errorcluster, "Aiming Beam Config"=w2184:T22)  [unwired: 8 in, 1 out]
        n998 = Bundle By Name(cluster=w2182, "VideoConfig"=w2184) -> (w2183:T23)
        n999 = call <vilib>:"Add State(s) to Queue__JKI_lib_State_Machine.vi"("State(s) in (\"\")"=w2189) -> ("States Out"=w2188:string)  [unwired: 14 in]
      }
      frame "SysConfig: LoadCursorLocation" {
        # "Load cursor location from ini file\n(load cursor from system setting ini file)"
        n1000 = call "readCursorConfigMain.vi"("error in (no error)"=w2201) -> ("error out"=w2202:errorcluster, "Cursor Locations"=w2200:T43)  [unwired: 9 in]
        n1001 = Unbundle By Name(w2200) -> ("DC1"=w2199:i32, "DC2"=w2198:i32, "BG1"=w2193:i32, "BG2"=w2192:i32)
        n1002 = Build Array(w2199, w2198) -> (w2197:i32[])
        n1003 = Build Array(w2193, w2192) -> (w2194:i32[])
        n1004 = Array Max & Min(array=w2197) -> (max value=w2196:i32, min value=w2195:i32)  [unwired: 2 out]
        n1005 = Array Max & Min(array=w2194) -> (max value=w2191:i32, min value=w2190:i32)  [unwired: 2 out]
        n1006 = global write "GlobalVariables.vi" "DC Idx2"(w2196) -> ()
        n1007 = global write "GlobalVariables.vi" "DC Idx1"(w2195) -> ()
        n1008 = global write "GlobalVariables.vi" "BG Idx2"(w2191) -> ()
        n1009 = global write "GlobalVariables.vi" "BG Idx1"(w2190) -> ()
        n1010 = call <vilib>:"Add State(s) to Queue__JKI_lib_State_Machine.vi"("State(s) in (\"\")"=w2206) -> ("States Out"=w2205:string)  [unwired: 14 in]
      }
      frame "---------- SystemStatus ----------" {
        # "Template Separator\n(You can make a copy of, or modify, this frame)"
        n1011 = call <vilib>:"Add State(s) to Queue__JKI_lib_State_Machine.vi"("State(s) in (\"\")"=w2211) -> ("States Out"=w2210:string)  [unwired: 14 in]
      }
      frame "SystemStatus: SlowSysStatusMacro" {
        # "store system check time"
        # "Template Separator\n(You can make a copy of, or modify, this frame)"
        n1012 = Tick Count (ms)() -> (millisecond timer value=w2214:u32)
        n1013 = Bundle By Name(cluster=w2212, "SlowTimer"=w2214) -> (w2213:T23)
        n1014 = call <vilib>:"Add State(s) to Queue__JKI_lib_State_Machine.vi"("State(s) in Front (\"\")"="Digitizer: checkTemp\nTCP: CheckConnection" ("State(s) in Front (\"\")"), "State(s) in (\"\")"=w2219) -> ("States Out"=w2218:string)  [unwired: 13 in]
      }
      frame "SystemStatus: FastSysStatusMacro" {
        # "store system check time"
        # "Template Separator\n(You can make a copy of, or modify, this frame)"
        n1015 = Tick Count (ms)() -> (millisecond timer value=w2222:u32)
        n1016 = Bundle By Name(cluster=w2220, "FastTimer"=w2222) -> (w2221:T23)
        n1017 = call <vilib>:"Add State(s) to Queue__JKI_lib_State_Machine.vi"("State(s) in Front (\"\")"="355 Laser: CheckPWMStatus\nAimingBeam: GetPWMStatus\n/*355 Laser: CheckControllerStatus" ("State(s) in Front (\"\")"), "State(s) in (\"\")"=w2227) -> ("States Out"=w2226:string)  [unwired: 13 in]
      }
      frame "---------- UI ----------" {
        # "Do not put any code in this frame.\n(It is a separator no-op. You can make a copy of this frame to create a new UI frame)"
        n1018 = call <vilib>:"Add State(s) to Queue__JKI_lib_State_Machine.vi"("State(s) in (\"\")"=w2232) -> ("States Out"=w2231:string)  [unwired: 14 in]
      }
      frame "UI: Initialize" {
        w2234 = T44 {"Minimum"=0.0, "Maximum"=4.6, "Increment"=0.1} ("Data Entry Limits")
        w2233 = T11."Disabled and Grayed Out" ("Disabled")
        # "Disable all button on startup"
        # "Initialize the User Interface, here.\n(this is called automatically, by the Macro: Init)"
        n1019 = property on="V 1" class="DigNum (strict)"("DisabledEnum"=w2233) -> ()  [unwired: 2 in, 2 out]
        n1020 = property on="V 2" class="DigNum (strict)"("DisabledEnum"=w2233) -> ()  [unwired: 2 in, 2 out]
        n1021 = property on="StopButton" class="Bool (strict)"("DisabledEnum"=w2233) -> ()  [unwired: 2 in, 2 out]
        n1022 = property on="Sys Reconfig" class="Bool"("DisabledEnum"=w2233) -> ()  [unwired: 2 in, 2 out]
        n1023 = property on="StartButton" class="Bool (strict)"("DisabledEnum"=w2233) -> ()  [unwired: 2 in, 2 out]
        n1024 = property on="355nm Laser toggle" class="Bool (strict)"("DisabledEnum"=w2233) -> ()  [unwired: 2 in, 2 out]
        n1025 = property on="Aiming beam toggle" class="Bool (strict)"("DisabledEnum"=w2233) -> ()  [unwired: 2 in, 2 out]
        n1026 = property on="Background" class="Bool (strict)"("DisabledEnum"=w2233) -> ()  [unwired: 2 in, 2 out]
        n1027 = property on="Cali&iRF alignment" class="Bool (strict)"("DisabledEnum"=w2233) -> ()  [unwired: 2 in, 2 out]
        n1028 = property on="V 3" class="DigNum (strict)"("DisabledEnum"=w2233) -> ()  [unwired: 2 in, 2 out]
        n1029 = property on="Video Source" class="RadioBtnsControl (strict)"("DisabledEnum"=w2233) -> ()  [unwired: 2 in, 2 out]
        n1030 = property on="V 1" class="DigNum (strict)"("Data Range"=w2234) -> ()  [unwired: 2 in, 2 out]
        n1031 = property on="V 2" class="DigNum (strict)"("Data Range"=w2234) -> ()  [unwired: 2 in, 2 out]
        n1032 = property on="V 3" class="DigNum (strict)"("Data Range"=w2234) -> ()  [unwired: 2 in, 2 out]
        n1033 = call <vilib>:"Add State(s) to Queue__JKI_lib_State_Machine.vi"("State(s) in Front (\"\")"="UI: CaliAndiRFNotReady" ("State(s) in Front (\"\")"), "State(s) in (\"\")"=w2240) -> ("States Out"=w2239:string)  [unwired: 13 in]
      }
      frame "UI: BGLoaded" {
        # "[Covers: REQ24]"
        # "Do not put any code in this frame.\n(It is a separator no-op. You can make a copy of this frame to create a new UI frame)"
        n1034 = property on="Background" class="Bool (strict)"("BoolText.Text"="Loaded!" ("Boolean Text.Text"), "Colors [4]"=cluster{u32, u32}[] [{15764023, 15764023}, {16711680, 16711680}]) -> ()  [unwired: 2 in, 2 out]
        n1035 = call <vilib>:"Add State(s) to Queue__JKI_lib_State_Machine.vi"("State(s) in (\"\")"=w2247) -> ("States Out"=w2246:string)  [unwired: 14 in]
      }
      frame "UI: BGSizeError" {
        # "[Covers: REQ24]"
        # "Do not put any code in this frame.\n(It is a separator no-op. You can make a copy of this frame to create a new UI frame)"
        n1036 = property on="Background" class="Bool (strict)"("BoolText.Text"="Loaded!" ("Boolean Text.Text"), "Colors [4]"=cluster{u32, u32}[] [{7171459, 7171459}, {16711680, 16711680}]) -> ()  [unwired: 2 in, 2 out]
        n1037 = One Button Dialog(message="Background waveform length and current digitizer setting mismatch! Please take a new background before any aquisition!") -> ()  [unwired: 1 in, 1 out]
        n1038 = call <vilib>:"Add State(s) to Queue__JKI_lib_State_Machine.vi"("State(s) in (\"\")"=w2255) -> ("States Out"=w2254:string)  [unwired: 14 in]
      }
      frame "UI: CaliAndiRFLoaded" {
        # "[Covers: REQ24]"
        # "Do not put any code in this frame.\n(It is a separator no-op. You can make a copy of this frame to create a new UI frame)"
        n1039 = property on="Cali&iRF alignment" class="Bool (strict)"("BoolText.Text"="Loaded!" ("Boolean Text.Text"), "Colors [4]"=cluster{u32, u32}[] [{15764023, 15764023}, {16711680, 16711680}]) -> ()  [unwired: 2 in, 2 out]
        n1040 = call <vilib>:"Add State(s) to Queue__JKI_lib_State_Machine.vi"("State(s) in (\"\")"=w2262) -> ("States Out"=w2261:string)  [unwired: 14 in]
      }
      frame "UI: WFAutoScale" {
        # "Set graph auto scale.\n(UI: WFAutoScale >> T/F)"
        n1041 = Equal?(x=w2263, y="F") -> (x = y?=w2264:bool)
        n1042 = Equal?(x=w2263, y="T") -> (x = y?=w2266:bool)
        n1043 = case shown="True" w2266 {
          frame False {
          }
          frame True {
            w2282 = u8 2 ("Y Scale.Scale Fit")
            n1044 = property on="Channel 1" class="WFGraph (strict)"("YScale.ScaleFit"=w2282) -> ()  [unwired: 2 in, 2 out]
            n1045 = property on="Channel 2" class="WFGraph (strict)"("YScale.ScaleFit"=w2282) -> ()  [unwired: 2 in, 2 out]
            n1046 = property on="Channel 3" class="WFGraph (strict)"("YScale.ScaleFit"=w2282) -> ()  [unwired: 2 in, 2 out]
          }
        }
        n1047 = case shown="True" w2264 {
          frame False {
          }
          frame True {
            w2279 = 0.0 ("Y Scale.Range:Maximum")
            w2280 = 2.0 ("Y Scale.Range:Maximum")
            w2281 = u8 0 ("Y Scale.Scale Fit")
            n1048 = property on="Channel 1" class="WFGraph (strict)"("YScale.ScaleFit"=w2281) -> (error out=w2278:errorcluster)  [unwired: 2 in, 1 out]
            n1049 = property on="Channel 2" class="WFGraph (strict)"("YScale.ScaleFit"=w2281) -> (error out=w2277:errorcluster)  [unwired: 2 in, 1 out]
            n1050 = property on="Channel 3" class="WFGraph (strict)"("YScale.ScaleFit"=w2281) -> (error out=w2276:errorcluster)  [unwired: 2 in, 1 out]
            n1051 = property on="Channel 1" class="WFGraph (strict)"(error in=w2278, "YScale.Maximum"=w2280) -> (error out=w2275:errorcluster)  [unwired: 1 in, 1 out]
            n1052 = property on="Channel 2" class="WFGraph (strict)"(error in=w2277, "YScale.Maximum"=w2280) -> (error out=w2274:errorcluster)  [unwired: 1 in, 1 out]
            n1053 = property on="Channel 3" class="WFGraph (strict)"(error in=w2276, "YScale.Maximum"=w2280) -> (error out=w2273:errorcluster)  [unwired: 1 in, 1 out]
            n1054 = property on="Channel 1" class="WFGraph (strict)"(error in=w2275, "YScale.Minimum"=w2279) -> ()  [unwired: 1 in, 2 out]
            n1055 = property on="Channel 2" class="WFGraph (strict)"(error in=w2274, "YScale.Minimum"=w2279) -> ()  [unwired: 1 in, 2 out]
            n1056 = property on="Channel 3" class="WFGraph (strict)"(error in=w2273, "YScale.Minimum"=w2279) -> ()  [unwired: 1 in, 2 out]
          }
        }
        n1057 = call <vilib>:"Add State(s) to Queue__JKI_lib_State_Machine.vi"("State(s) in (\"\")"=w2272) -> ("States Out"=w2271:string)  [unwired: 14 in]
      }
      frame "UI: showDisclaimer" {
        # "Show disclamer window.\n(It is a separator no-op. You can make a copy of this frame to create a new UI frame)"
        n1058 = call <vilib>:"Application Directory.vi"() -> ("Application Directory"=w2295:path)
        n1059 = Build Path(base path=w2295, name or relative path="Disclamer.png") -> (appended path=w2293:path)
        n1060 = property on="Disclamer" class="Pict"() -> ("Draw Area Size"=w2291:T45)  [unwired: 2 in, 2 out]
        n1061 = disable-structure "Diagram Disable Structure" shown="Disabled" {
          frame Disabled {
            n1062 = flat-sequence {
              frame #0 {
                n1063 = call "disclaimer.vi"() -> ()  [unwired: 12 in]
              }
              frame #1 {
                n1064 = Wait (ms)(milliseconds to wait=u32 250) -> ()  [unwired: 1 out]
              }
              frame #2 {
                n1065 = call "SoftwareNote.vi"() -> ()  [unwired: 12 in]
              }
            }
          }
          frame Enabled {
          }
        }
        n1066 = call <vilib>:"Read PNG File.vi"("path to PNG file"=w2293) -> ("image data"=w2290:T46)  [unwired: 8 in, 2 out]
        n1067 = Unbundle By Name(w2290) -> ("Rectangle.right"=w2288:i16, "Rectangle.bottom"=w2286:i16)
        n1068 = Unbundle By Name(w2291) -> ("Width"=w2289:u32, "Height"=w2287:u32)
        n1069 = call <vilib>:"Draw Flattened Pixmap.vi"("image data"=w2290) -> ("new picture"=→"Disclamer":picture)  [unwired: 8 in]
        n1070 = Divide(x=w2289, y=w2288) -> (x/y=w2285:dbl)
        n1071 = Divide(x=w2287, y=w2286) -> (x/y=w2284:dbl)
        n1072 = Max & Min(x=w2285, y=w2284) -> (min(x,y)=w2283:dbl)  [unwired: 1 out]
        n1073 = property on="Disclamer" class="Pict"("ZoomFactor"=w2283) -> ()  [unwired: 2 in, 2 out]
        n1074 = call <vilib>:"Add State(s) to Queue__JKI_lib_State_Machine.vi"("State(s) in (\"\")"=w2300) -> ("States Out"=w2299:string)  [unwired: 14 in]
      }
      frame "UI: CaliAndiRFNotReady" {
        # "Do not put any code in this frame.\n(It is a separator no-op. You can make a copy of this frame to create a new UI frame)"
        n1075 = property on="Cali&iRF alignment" class="Bool (strict)"("BoolText.Text"="No Info" ("Boolean Text.Text"), "Colors [4]"=cluster{u32, u32}[] [{13816530, 13816530}, {16711680, 16711680}]) -> ()  [unwired: 2 in, 2 out]
        n1076 = call <vilib>:"Add State(s) to Queue__JKI_lib_State_Machine.vi"("State(s) in (\"\")"=w2308) -> ("States Out"=w2307:string)  [unwired: 14 in]
      }
      frame "UI: BGnotReady" {
        # "Do not put any code in this frame.\n(It is a separator no-op. You can make a copy of this frame to create a new UI frame)"
        n1077 = property on="Background" class="Bool (strict)"("BoolText.Text"="No Info" ("Boolean Text.Text"), "Colors [4]"=cluster{u32, u32}[] [{13816530, 13816530}, {16711680, 16711680}]) -> ()  [unwired: 2 in, 2 out]
        n1078 = call <vilib>:"Add State(s) to Queue__JKI_lib_State_Machine.vi"("State(s) in (\"\")"=w2315) -> ("States Out"=w2314:string)  [unwired: 14 in]
      }
      frame "UI: Reset" {
        w2317 = cluster{u32, u32}[] [{13816530, 13816530}, {13816530, 13816530}] ("Colors [4]")
        # "Do not put any code in this frame.\n(It is a separator no-op. You can make a copy of this frame to create a new UI frame)"
        n1079 = property on="Cali&iRF alignment" class="Bool (strict)"("BoolText.Text"="No Info" ("Boolean Text.Text"), "Colors [4]"=w2317) -> ()  [unwired: 2 in, 2 out]
        n1080 = property on="Background" class="Bool (strict)"("BoolText.Text"="No Info" ("Boolean Text.Text"), "Colors [4]"=w2317) -> ()  [unwired: 2 in, 2 out]
        n1081 = call <vilib>:"Add State(s) to Queue__JKI_lib_State_Machine.vi"("State(s) in (\"\")"=w2323) -> ("States Out"=w2322:string)  [unwired: 14 in]
      }
      frame "UI: SetButtonText" {
        # "Set button text of 355nm laser and aiming beam."
        n1082 = call <vilib>:"Add State(s) to Queue__JKI_lib_State_Machine.vi"("State(s) in (\"\")"=w2328) -> ("States Out"=w2327:string)  [unwired: 14 in]
      }
      frame "UI: DuringAquisition" {
        w2331 = T11."Disabled and Grayed Out" ("Disabled")
        # "Do not put any code in this frame.\n(It is a separator no-op. You can make a copy of this frame to create a new UI frame)"
        n1083 = Unbundle By Name(w2330) -> ("bothVidSourceAvail"=w2329:bool)
        n1084 = case shown="True" w2329 {
          tunnel: w2331 -> [_ w2337]
          frame False {
          }
          frame True {
            n1085 = property on="Video Source" class="RadioBtnsControl (strict)"("DisabledEnum"=w2337) -> ()  [unwired: 2 in, 2 out]
          }
        }
        n1086 = property on="StartButton" class="Bool (strict)"("DisabledEnum"=w2331) -> ()  [unwired: 2 in, 2 out]
        n1087 = property on="Sys Reconfig" class="Bool"("DisabledEnum"=w2331) -> ()  [unwired: 2 in, 2 out]
        n1088 = property on="355nm Laser toggle" class="Bool (strict)"("DisabledEnum"=w2331) -> ()  [unwired: 2 in, 2 out]
        n1089 = property on="Aiming beam toggle" class="Bool (strict)"("DisabledEnum"=w2331) -> ()  [unwired: 2 in, 2 out]
        n1090 = property on="Background" class="Bool (strict)"("DisabledEnum"=w2331) -> ()  [unwired: 2 in, 2 out]
        n1091 = property on="Radio Buttons" class="RadioBtnsControl (strict)"("DisabledEnum"=w2331) -> ()  [unwired: 2 in, 2 out]
        n1092 = property on="Cali&iRF alignment" class="Bool (strict)"("DisabledEnum"=w2331) -> ()  [unwired: 2 in, 2 out]
        n1093 = property on="Quit" class="Bool"("DisabledEnum"=w2331) -> ()  [unwired: 2 in, 2 out]
        n1094 = property on="Skip Data Save?" class="Bool (strict)"("DisabledEnum"=w2331) -> ()  [unwired: 2 in, 2 out]
        n1095 = property on="Video Display" class="Bool (strict)"("DisabledEnum"=w2331) -> ()  [unwired: 2 in, 2 out]
        n1096 = property on="StopButton" class="Bool (strict)"("DisabledEnum"=T11."Enabled" ("Disabled")) -> ()  [unwired: 2 in, 2 out]
        n1097 = call <vilib>:"Add State(s) to Queue__JKI_lib_State_Machine.vi"("State(s) in (\"\")"=w2336) -> ("States Out"=w2335:string)  [unwired: 14 in]
      }
      frame "UI: duringIRFAlign" {
        w2338 = T11."Disabled and Grayed Out" ("Disabled")
        # "Set UI to during iRF alignment\n(It is a separator no-op. You can make a copy of this frame to create a new UI frame)"
        n1098 = property on="StartButton" class="Bool (strict)"("DisabledEnum"=w2338) -> ()  [unwired: 2 in, 2 out]
        n1099 = property on="Sys Reconfig" class="Bool"("DisabledEnum"=w2338) -> ()  [unwired: 2 in, 2 out]
        n1100 = property on="355nm Laser toggle" class="Bool (strict)"("DisabledEnum"=w2338) -> ()  [unwired: 2 in, 2 out]
        n1101 = property on="Aiming beam toggle" class="Bool (strict)"("DisabledEnum"=w2338) -> ()  [unwired: 2 in, 2 out]
        n1102 = property on="Background" class="Bool (strict)"("DisabledEnum"=w2338) -> ()  [unwired: 2 in, 2 out]
        n1103 = property on="StopButton" class="Bool (strict)"("DisabledEnum"=w2338) -> ()  [unwired: 2 in, 2 out]
        n1104 = call <vilib>:"Add State(s) to Queue__JKI_lib_State_Machine.vi"("State(s) in (\"\")"=w2343) -> ("States Out"=w2342:string)  [unwired: 14 in]
      }
      frame "UI: duringBGAcquire" {
        w2344 = T11."Disabled and Grayed Out" ("Disabled")
        # "Do not put any code in this frame.\n(It is a separator no-op. You can make a copy of this frame to create a new UI frame)"
        n1105 = property on="StartButton" class="Bool (strict)"("DisabledEnum"=w2344) -> ()  [unwired: 2 in, 2 out]
        n1106 = property on="StopButton" class="Bool (strict)"("DisabledEnum"=w2344) -> ()  [unwired: 2 in, 2 out]
        n1107 = property on="Sys Reconfig" class="Bool"("DisabledEnum"=w2344) -> ()  [unwired: 2 in, 2 out]
        n1108 = property on="355nm Laser toggle" class="Bool (strict)"("DisabledEnum"=w2344) -> ()  [unwired: 2 in, 2 out]
        n1109 = property on="Aiming beam toggle" class="Bool (strict)"("DisabledEnum"=w2344) -> ()  [unwired: 2 in, 2 out]
        n1110 = property on="Cali&iRF alignment" class="Bool (strict)"("DisabledEnum"=w2344) -> ()  [unwired: 2 in, 2 out]
        n1111 = call <vilib>:"Add State(s) to Queue__JKI_lib_State_Machine.vi"("State(s) in (\"\")"=w2349) -> ("States Out"=w2348:string)  [unwired: 14 in]
      }
      frame "UI: ReadyForAquisition" {
        w2353 = T11."Enabled" ("Disabled")
        # "Do not put any code in this frame.\n(It is a separator no-op. You can make a copy of this frame to create a new UI frame)"
        n1112 = Unbundle By Name(w2352) -> ("System Status.TCP/IP"=w2351:bool, "bothVidSourceAvail"=w2350:bool)
        n1113 = property on="StartButton" class="Bool (strict)"("DisabledEnum"=w2353) -> ()  [unwired: 2 in, 2 out]
        n1114 = property on="Sys Reconfig" class="Bool"("DisabledEnum"=w2353) -> ()  [unwired: 2 in, 2 out]
        n1115 = property on="355nm Laser toggle" class="Bool (strict)"("DisabledEnum"=w2353) -> ()  [unwired: 2 in, 2 out]
        n1116 = property on="Aiming beam toggle" class="Bool (strict)"("DisabledEnum"=w2353) -> ()  [unwired: 2 in, 2 out]
        n1117 = property on="Cali&iRF alignment" class="Bool (strict)"("DisabledEnum"=w2353) -> ()  [unwired: 2 in, 2 out]
        n1118 = property on="Background" class="Bool (strict)"("DisabledEnum"=w2353) -> ()  [unwired: 2 in, 2 out]
        n1119 = property on="Quit" class="Bool"("DisabledEnum"=w2353) -> ()  [unwired: 2 in, 2 out]
        n1120 = property on="Radio Buttons" class="RadioBtnsControl (strict)"("DisabledEnum"=w2353) -> ()  [unwired: 2 in, 2 out]
        n1121 = case shown="True" w2350 {
          tunnel: w2353 -> [_ w2359]
          frame False {
          }
          frame True {
            n1122 = property on="Video Source" class="RadioBtnsControl (strict)"("DisabledEnum"=w2359) -> ()  [unwired: 2 in, 2 out]
          }
        }
        n1123 = property on="Skip Data Save?" class="Bool (strict)"("DisabledEnum"=w2353) -> ()  [unwired: 2 in, 2 out]
        n1124 = case shown="True" w2351 {
          tunnel: w2353 -> [_ w2360]
          frame False {
          }
          frame True {
            n1125 = property on="Video Display" class="Bool (strict)"("DisabledEnum"=w2360) -> ()  [unwired: 2 in, 2 out]
          }
        }
        n1126 = property on="StopButton" class="Bool (strict)"("DisabledEnum"=T11."Disabled and Grayed Out" ("Disabled")) -> ()  [unwired: 2 in, 2 out]
        n1127 = call <vilib>:"Add State(s) to Queue__JKI_lib_State_Machine.vi"("State(s) in (\"\")"=w2358) -> ("States Out"=w2357:string)  [unwired: 14 in]
      }
      frame "UI: Update" {
        # "Do not put any code in this frame.\n(It is a separator no-op. You can make a copy of this frame to create a new UI frame)"
        n1128 = Unbundle By Name(w2371) -> ("System Status"=→"System Hardware Connection Status":T2, "IDs.RunID"=→"Run #":i8, "CaseID"=→"Case #":string, "FLImDAQ"=→"FLImDAQ":T30, "SysRunning?"=→"Aquisition Status:":bool, "LJ Pinout"=→"LJ Pinout":T4, "IDs.BG ID"=→"BG #":i8, "IDs.Cali ID"=→"Calibration #":i8, "video source"=→"Visualization PC video source":T1)
        n1129 = call <vilib>:"Add State(s) to Queue__JKI_lib_State_Machine.vi"("State(s) in (\"\")"=w2374) -> ("States Out"=w2373:string)  [unwired: 14 in]
      }
      frame "UI: updateVideoToggle" {
        # "Set video toggle based on visualization PC video source.\n(take )"
        n1130 = call <vilib>:"Add State(s) to Queue__JKI_lib_State_Machine.vi"("State(s) in (\"\")"=w2379) -> ("States Out"=w2378:string)  [unwired: 14 in]
      }
      frame "UI: Cursor Set" {
        # "Argument"
        # "Set and Unset Cursor Busy.\n(Usage: \"UI: Cursor Set >> Busy|Idle\")"
        n1131 = case shown="\"Idle\", Default" w2381 {
          tunnel: w2383 -> [w2388 w2390]
          tunnel: [w2387 w2389] -> w2382
          frame "Idle", Default {
            n1132 = call <vilib>:"Unset Busy.vi"("error in (no error)"=w2388) -> ("error out"=w2387:errorcluster)  [unwired: 10 in]
          }
          frame "Busy" {
            n1133 = call <vilib>:"Set Busy.vi"("error in (no error)"=w2390) -> ("error out"=w2389:errorcluster)  [unwired: 9 in, 1 out]
          }
        }
        n1134 = call <vilib>:"Add State(s) to Queue__JKI_lib_State_Machine.vi"("State(s) in (\"\")"=w2386) -> ("States Out"=w2385:string)  [unwired: 14 in]
      }
      frame "UI: Front Panel State" {
        # "Argument"
        # "Set Front Panel Open or Closed\n(Usage: \"UI: Front Panel State >> Open|Close\")"
        n1135 = Unbundle By Name(w2394) -> ("Core.Current VI Reference"=w2393:refnum<vi>)
        n1136 = case shown="\"Open\", \"Standard\", Default" w2392 {
          tunnel: w2396 -> [w2404 w2419 w2430 w2443 w2456]
          tunnel: [w2406 w2420 w2432 w2445 w2458] -> w2395
          tunnel: w2393 -> [w2405 w2417 w2431 w2444 w2457]
          frame "Open", "Standard", Default {
            w2399 = T17."Standard" ("State")
            n1137 = property on="Property Node" class="VI"(reference=w2405, error in=w2404) -> (reference out=w2402:refnum<vi>, error out=w2403:errorcluster, "FP.State"=w2401:T17)
            n1138 = Not Equal?(x=w2401, y=w2399) -> (x != y?=w2400:bool)
            n1139 = case shown="True" w2400 {
              tunnel: [w2410 w2412] -> w2406
              tunnel: w2403 -> [w2409 w2412]
              tunnel: w2402 -> [w2408 _]
              tunnel: w2399 -> [w2407 _]
              frame True {
                n1140 = invoke on="Invoke Node" class="VI" method="FP.Open"(reference=w2408, error in=w2409, "Activate"=TRUE, "State"=w2407) -> (error out=w2410:errorcluster)  [unwired: 1 in, 4 out]
              }
              frame False {
              }
            }
          }
          frame "Close", "Closed" {
            n1141 = property on="Property Node" class="VI"(reference=w2417, error in=w2419) -> (reference out=w2416:refnum<vi>, error out=w2418:errorcluster, "FP.State"=w2414:T17)
            n1142 = Not Equal?(x=w2414, y=T17."Closed" ("Front Panel Window:State")) -> (x != y?=w2413:bool)
            n1143 = case shown="True" w2413 {
              tunnel: [w2421 w2424] -> w2420
              tunnel: w2418 -> [w2421 w2423]
              tunnel: w2416 -> [_ w2422]
              frame False {
              }
              frame True {
                n1144 = invoke on="Invoke Node" class="VI" method="FP.Close"(reference=w2422, error in=w2423) -> (error out=w2424:errorcluster)  [unwired: 1 in, 2 out]
              }
            }
          }
          frame "Hidden", "Hide" {
            w2425 = T17."Hidden" ("State")
            n1145 = property on="Property Node" class="VI"(reference=w2431, error in=w2430) -> (reference out=w2428:refnum<vi>, error out=w2429:errorcluster, "FP.State"=w2427:T17)
            n1146 = Not Equal?(x=w2427, y=w2425) -> (x != y?=w2426:bool)
            n1147 = case shown="True" w2426 {
              tunnel: [w2436 w2437] -> w2432
              tunnel: w2429 -> [w2435 w2437]
              tunnel: w2428 -> [w2434 _]
              tunnel: w2425 -> [w2433 _]
              frame True {
                n1148 = invoke on="Invoke Node" class="VI" method="FP.Open"(reference=w2434, error in=w2435, "State"=w2433) -> (error out=w2436:errorcluster)  [unwired: 2 in, 4 out]
              }
              frame False {
              }
            }
          }
          frame "Minimize", "Minimized" {
            w2438 = T17."Minimized" ("State")
            n1149 = property on="Property Node" class="VI"(reference=w2444, error in=w2443) -> (reference out=w2441:refnum<vi>, error out=w2442:errorcluster, "FP.State"=w2440:T17)
            n1150 = Not Equal?(x=w2440, y=w2438) -> (x != y?=w2439:bool)
            n1151 = case shown="True" w2439 {
              tunnel: [w2449 w2450] -> w2445
              tunnel: w2442 -> [w2448 w2450]
              tunnel: w2441 -> [w2447 _]
              tunnel: w2438 -> [w2446 _]
              frame True {
                n1152 = invoke on="Invoke Node" class="VI" method="FP.Open"(reference=w2447, error in=w2448, "State"=w2446) -> (error out=w2449:errorcluster)  [unwired: 2 in, 4 out]
              }
              frame False {
              }
            }
          }
          frame "Maximize", "Maximized" {
            w2451 = T17."Maximized" ("State")
            n1153 = property on="Property Node" class="VI"(reference=w2457, error in=w2456) -> (reference out=w2454:refnum<vi>, error out=w2455:errorcluster, "FP.State"=w2453:T17)
            n1154 = Not Equal?(x=w2453, y=w2451) -> (x != y?=w2452:bool)
            n1155 = case shown="True" w2452 {
              tunnel: [w2462 w2463] -> w2458
              tunnel: w2455 -> [w2461 w2463]
              tunnel: w2454 -> [w2460 _]
              tunnel: w2451 -> [w2459 _]
              frame True {
                n1156 = invoke on="Invoke Node" class="VI" method="FP.Open"(reference=w2460, error in=w2461, "State"=w2459) -> (error out=w2462:errorcluster)  [unwired: 2 in, 4 out]
              }
              frame False {
              }
            }
          }
        }
        n1157 = call <vilib>:"Add State(s) to Queue__JKI_lib_State_Machine.vi"("State(s) in (\"\")"=w2398) -> ("States Out"=w2397:string)  [unwired: 14 in]
      }
      frame "---------- AimingBeam ----------" {
        # "Template Separator\n(You can make a copy of, or modify, this frame)"
        n1158 = call <vilib>:"Add State(s) to Queue__JKI_lib_State_Machine.vi"("State(s) in (\"\")"=w2468) -> ("States Out"=w2467:string)  [unwired: 14 in]
      }
      frame "AimingBeam: Initialize" {
        # "set aiming beam button color"
        # "Open COM port for Aiming Beam\n(Require USB connection)"
        n1159 = Unbundle By Name(w2470) -> ("AB Cluster.Aiming Beam COM Port"=w2478:refnum<visa-resource-name>)
        n1160 = call-poly "VISA Configure Serial Port"("VISA resource name"=w2478, "Enable Termination\nChar (T)"=TRUE ("Enable Termination\nChar (T)"), "baud rate (9600)"=u32 9600, "error in (no error)"=w2475) -> ("error out"=w2474:errorcluster)  [unwired: 10 in, 1 out]
        n1161 = Unbundle By Name(w2474) -> ("status"=w2473:bool)
        n1162 = Not(x=w2473) -> (.not. x?=w2472:bool)
        n1163 = Bundle By Name(cluster=w2470, "System Status.Aiming Beam"=w2472) -> (w2471:T23)
        n1164 = call <vilib>:"Add State(s) to Queue__JKI_lib_State_Machine.vi"("State(s) in (\"\")"=w2480) -> ("States Out"=w2479:string)  [unwired: 14 in]
      }
      frame "AimingBeam: Close" {
        # "Close Aiming Beam COM port\n(Require USB connection to Aiming Beam Laser)"
        n1165 = Unbundle By Name(w2483) -> ("AB Cluster.Aiming Beam COM Port"=w2487:refnum<visa-resource-name>)
        n1166 = VISA Close(VISA resource name=w2487, error in (no error)=w2485) -> (error out=w2486:errorcluster)
        n1167 = Bundle By Name(cluster=w2483, "System Status.Aiming Beam"=FALSE) -> (w2484:T23)
        n1168 = call <vilib>:"Add State(s) to Queue__JKI_lib_State_Machine.vi"("State(s) in (\"\")"=w2489) -> ("States Out"=w2488:string)  [unwired: 14 in]
      }
      frame "AimingBeam: Set Current" {
        # "Set Aiming Beam Current\n(You can make a copy of, or modify, this frame)"
        n1169 = Unbundle By Name(w2501) -> ("AB Cluster.Aiming Beam COM Port"=w2494:refnum<visa-resource-name>)
        n1170 = Number To Fractional String(number="488nm Power", precision (6)=i16 2) -> (F-format string=w2495:string)  [unwired: 2 in]
        n1171 = Concatenate Strings("slc:", w2495, "\r" ("Carriage Return Constant"), "\n" ("Line Feed Constant")) -> (w2498:string)
        n1172 = VISA Write(VISA resource name=w2494, write buffer=w2498, error in (no error)=w2492) -> (error out=w2493:errorcluster)  [unwired: 2 out]
        n1173 = call <vilib>:"Add State(s) to Queue__JKI_lib_State_Machine.vi"("State(s) in (\"\")"=w2503) -> ("States Out"=w2502:string)  [unwired: 14 in]
      }
      frame "AimingBeam: Set ACC Status" {
        # "Enable Aiming Beam\n(Usage: \"AimingBeam: Set >> Enable|Disable\")"
        n1174 = Unbundle By Name(w2510) -> ("AB Cluster.Aiming Beam COM Port"=w2507:refnum<visa-resource-name>)
        n1175 = case shown="\"Enable\"" w2509 {
          tunnel: [w2513 w2517] -> w2508
          frame "Disable", Default {
            n1176 = Concatenate Strings("cof", "\r" ("Carriage Return Constant"), "\n" ("Line Feed Constant")) -> (w2513:string)
          }
          frame "Enable" {
            n1177 = Concatenate Strings("con", "\r" ("Carriage Return Constant"), "\n" ("Line Feed Constant")) -> (w2517:string)
          }
        }
        n1178 = VISA Write(VISA resource name=w2507, write buffer=w2508, error in (no error)=w2505) -> (error out=w2506:errorcluster)  [unwired: 2 out]
        n1179 = call <vilib>:"Add State(s) to Queue__JKI_lib_State_Machine.vi"("State(s) in (\"\")"=w2512) -> ("States Out"=w2511:string)  [unwired: 14 in]
      }
      frame "AimingBeam: Set APC Status" {
        # "Enable Aiming Beam\n(Usage: \"AimingBeam: Set >> Enable|Disable\")"
        n1180 = Unbundle By Name(w2527) -> ("AB Cluster.Aiming Beam COM Port"=w2524:refnum<visa-resource-name>)
        n1181 = case shown="\"Disable\", Default" w2526 {
          tunnel: [w2530 w2534] -> w2525
          frame "Disable", Default {
            n1182 = Concatenate Strings("lof", "\r" ("Carriage Return Constant"), "\n" ("Line Feed Constant")) -> (w2530:string)
          }
          frame "Enable" {
            n1183 = Concatenate Strings("lon", "\r" ("Carriage Return Constant"), "\n" ("Line Feed Constant")) -> (w2534:string)
          }
        }
        n1184 = VISA Write(VISA resource name=w2524, write buffer=w2525, error in (no error)=w2522) -> (error out=w2523:errorcluster)  [unwired: 2 out]
        n1185 = call <vilib>:"Add State(s) to Queue__JKI_lib_State_Machine.vi"("State(s) in (\"\")"=w2529) -> ("States Out"=w2528:string)  [unwired: 14 in]
      }
      frame "AimingBeam: GetPWMStatus" {
        # "Get aiming beam PWM status\n()"
        n1186 = Unbundle By Name(w2542) -> ("AB Cluster.Freq"=w2541:i32, "LJ Pinout.AimingBeam PWM"=w2548:string)
        n1187 = Equal To 0?(x=w2541) -> (x = 0?=w2540:bool)
        n1188 = call "LabJack_FGV.vi"("Operation(Read)"=enum16{"Write", "Read"}."Read" ("Operation"), "error in (no error)"=w2544) -> ("error out"=w2546:errorcluster, "Read data"=w2547:i32)  [unwired: 8 in]
        n1189 = case shown="True" w2540 {
          tunnel: w2548 -> [w2561 _]
          tunnel: [w2559 "DIO_STATE"] -> w2545
          frame False {
            n1190 = Concatenate Strings(w2561, "_EF_ENABLE" ("string")) -> (w2559:string)
          }
          frame True {
          }
        }
        n1191 = call "LJM_eReadName.vi"("Handle In"=w2547, "Name"=w2545, "error in"=w2546) -> ("Value"=w2539:dbl, "error out"=w2543:errorcluster)  [unwired: 10 in, 1 out]
        n1192 = case shown="True" w2540 {
          tunnel: w2539 -> [w2554 w2558]
          tunnel: [w2553 w2555] -> w2538
          frame False {
            n1193 = Greater Than 0?(x=w2554) -> (x > 0?=w2553:bool)
          }
          frame True {
            n1194 = Number To Boolean Array(number=w2558) -> (Boolean array=w2557:bool[])
            n1195 = Index Array(array=w2557, index=3) -> (element=w2555:bool)
          }
        }
        n1196 = case shown="False" w2538 {
          frame False {
            # "PWM is off\nset color to dark green"
            n1197 = local write "Aiming beam toggle"(FALSE ("Aimging beam")) -> ()
          }
          frame True {
            # "PWM is on\nset color to light green"
            n1198 = local write "Aiming beam toggle"(TRUE ("Aimging beam")) -> ()
          }
        }
        n1199 = call <vilib>:"Add State(s) to Queue__JKI_lib_State_Machine.vi"("State(s) in (\"\")"=w2552) -> ("States Out"=w2551:string)  [unwired: 14 in]
      }
      frame "---------- 355 Laser ----------" {
        # "Template Separator\n(You can make a copy of, or modify, this frame)"
        n1200 = call <vilib>:"Add State(s) to Queue__JKI_lib_State_Machine.vi"("State(s) in (\"\")"=w2569) -> ("States Out"=w2568:string)  [unwired: 14 in]
      }
      frame "355 Laser: Check Dewelling" {
        # "if time laser start time is less than 7.5s before, wait 250ms then check again."
        # "Template Separator\n(You can make a copy of, or modify, this frame)"
        n1201 = Unbundle By Name(w2577) -> ("Laser start tic"=w2574:u32)
        n1202 = Tick Count (ms)() -> (millisecond timer value=w2575:u32)
        n1203 = Subtract(x=w2575, y=w2574) -> (x-y=w2573:u32)
        n1204 = Greater?(x=w2573, y=u32 5000) -> (0:w2571:bool)
        n1205 = case shown="False" w2571 {
          tunnel: ["355 Laser: Check Dewelling" ""] -> w2570
          frame False {
            n1206 = Wait (ms)(milliseconds to wait=u32 250) -> ()  [unwired: 1 out]
          }
          frame True {
          }
        }
        n1207 = call <vilib>:"Add State(s) to Queue__JKI_lib_State_Machine.vi"("State(s) in Front (\"\")"=w2570, "State(s) in (\"\")"=w2580) -> ("States Out"=w2579:string)  [unwired: 13 in]
      }
      frame "355 Laser: Laser enable" {
        # "Laser enable/disable\n(Usage: \"LabJack: Laser enable/disable >> 1|0\")"
        n1208 = Unbundle By Name(w2587) -> ("LJ Pinout.Laser Start/Stop"=w2591:string, "System Status.355 Laser"=w2585:bool)
        n1209 = case shown="False" w2585 {
          tunnel: w2584 -> [w2606 w2607]
          tunnel: w2591 -> [w2600 _]
          tunnel: [w2595 w2607] -> w2589
          tunnel: [w2594 u32 0 ("millisecond timer value")] -> w2586
          frame False {
            n1210 = call "LabJack_FGV.vi"("Operation(Read)"=enum16{"Write", "Read"}."Read" ("Operation")) -> ("Read data"=w2602:i32)  [unwired: 9 in, 1 out]
            n1211 = call "LJM_eWriteName.vi"("Handle In"=w2602, "Name"=w2600, "Value"=1.0, "error in"=w2606) -> ("Handle Out"=w2601:i32, "error out"=w2599:errorcluster)  [unwired: 10 in]
            n1212 = call <userlib>:"Wait (ms)__ogtk.vi"("error in (no error)"=w2599, "milliseconds to wait"=u32 250) -> ("error out"=w2598:errorcluster)  [unwired: 8 in, 1 out]
            n1213 = call "LJM_eWriteName.vi"("Handle In"=w2601, "Name"=w2600, "Value"=0.0, "error in"=w2598) -> ("error out"=w2596:errorcluster)  [unwired: 10 in, 1 out]
            n1214 = call <userlib>:"Tick Count (ms)__ogtk.vi"("error in (no error)"=w2596) -> ("error out"=w2595:errorcluster, "millisecond timer value"=w2594:u32)  [unwired: 9 in]
          }
          frame True {
          }
        }
        n1215 = Bundle By Name(cluster=w2587, "Laser start tic"=w2586) -> (w2588:T23)
        n1216 = call <vilib>:"Add State(s) to Queue__JKI_lib_State_Machine.vi"("State(s) in (\"\")"=w2593) -> ("States Out"=w2592:string)  [unwired: 14 in]
      }
      frame "355 Laser: Laser disable" {
        # "Laser enable/disable\n(Usage: \"LabJack: Laser enable/disable >> 1|0\")"
        n1217 = Unbundle By Name(w2611) -> ("LJ Pinout.Laser Start/Stop"=w2615:string, "System Status.355 Laser"=w2609:bool)
        n1218 = case shown="True" w2609 {
          tunnel: w2616 -> [w2619 w2633]
          tunnel: w2615 -> [_ w2627]
          tunnel: [w2619 w2622] -> w2613
          tunnel: [u32 0 ("millisecond timer value") w2621] -> w2610
          frame False {
          }
          frame True {
            n1219 = call "LabJack_FGV.vi"("Operation(Read)"=enum16{"Write", "Read"}."Read" ("Operation")) -> ("Read data"=w2629:i32)  [unwired: 9 in, 1 out]
            n1220 = call "LJM_eWriteName.vi"("Handle In"=w2629, "Name"=w2627, "Value"=1.0, "error in"=w2633) -> ("Handle Out"=w2628:i32, "error out"=w2626:errorcluster)  [unwired: 10 in]
            n1221 = call <userlib>:"Wait (ms)__ogtk.vi"("error in (no error)"=w2626, "milliseconds to wait"=u32 250) -> ("error out"=w2625:errorcluster)  [unwired: 8 in, 1 out]
            n1222 = call "LJM_eWriteName.vi"("Handle In"=w2628, "Name"=w2627, "Value"=0.0, "error in"=w2625) -> ("error out"=w2623:errorcluster)  [unwired: 10 in, 1 out]
            n1223 = call <userlib>:"Tick Count (ms)__ogtk.vi"("error in (no error)"=w2623) -> ("error out"=w2622:errorcluster, "millisecond timer value"=w2621:u32)  [unwired: 9 in]
          }
        }
        n1224 = Bundle By Name(cluster=w2611, "Laser start tic"=w2610) -> (w2612:T23)
        n1225 = call <vilib>:"Add State(s) to Queue__JKI_lib_State_Machine.vi"("State(s) in (\"\")"=w2618) -> ("States Out"=w2617:string)  [unwired: 14 in]
      }
      frame "355 Laser: Dewelling" {
        # "Wait some time (ms)\n(355 Laser: Dewelling >> #)"
        n1226 = Fract/Exp String To Number(string=w2637, default (0 dbl)=0) -> (number=w2635:i32)  [unwired: 2 in, 1 out]
        n1227 = Wait (ms)(milliseconds to wait=w2635) -> ()  [unwired: 1 out]
        n1228 = call <vilib>:"Add State(s) to Queue__JKI_lib_State_Machine.vi"("State(s) in (\"\")"=w2641) -> ("States Out"=w2640:string)  [unwired: 14 in]
      }
      frame "355 Laser: Close" {
        # "Template Separator\n(You can make a copy of, or modify, this frame)"
        n1229 = call <vilib>:"Add State(s) to Queue__JKI_lib_State_Machine.vi"("State(s) in Front (\"\")"="355 Laser: CheckControllerStatus\n355 Laser: Laser disable\n355 Laser: Dewelling >>1000", "State(s) in (\"\")"=w2647) -> ("States Out"=w2646:string)  [unwired: 13 in]
      }
      frame "355 Laser: CheckControllerStatus" {
        # "if average < 2, laser no power\nif average 2 < average < 9.3, laser on\nif 9.3<average<10, interlock open, blink indicator\nif average > 10, laser off\n[Covers: REQ30]"
        # "take 10 measuremt and look at average"
        # "Check 355 laser controller status\nBy probing Emisison Lamp negative terminal voltage"
        n1230 = Unbundle By Name(w2656) -> ("LJ Pinout.Laser Ready"=w2659:string)
        n1231 = call "LabJack_FGV.vi"("Operation(Read)"=enum16{"Write", "Read"}."Read" ("Operation")) -> ("Read data"=w2660:i32)  [unwired: 9 in, 1 out]
        n1232 = for {
          N: 20 -> [_]
          tunnel: w2660 -> [w2671]
          tunnel: w2659 -> [w2670]
          shift-right: [w2669] -> w2652
          shift-left: w2658 -> [w2668]
          tunnel: [w2666] -> w2651 mode=indexing
          n1233 = call "LJM_eReadName.vi"("Handle In"=w2671, "Name"=w2670, "error in"=w2668) -> ("Value"=w2666:dbl, "error out"=w2669:errorcluster)  [unwired: 10 in, 1 out]
          n1234 = Wait (ms)(milliseconds to wait=u32 25) -> ()  [unwired: 1 out]
        }
        n1235 = call "checkLaserStatus.vi"("error in (no error)"=w2652, "Laser LED voltage"=w2651) -> ("error out"=w2653:errorcluster, "Interlock open?"=w2648:bool, "Laser on?"=w2650:bool, "Mean voltage"=→"laser EM lamp V":dbl)  [unwired: 6 in]
        n1236 = Bundle By Name(cluster=w2656, "System Status.355 Laser"=w2650) -> (w2657:T23)
        n1237 = case shown="True" w2648 {
          frame False {
            n1238 = property on="355 Laser" class="Bool (strict)"("Blinking"=FALSE) -> ()  [unwired: 2 in, 2 out]
          }
          frame True {
            n1239 = property on="355 Laser" class="Bool (strict)"("Blinking"=TRUE) -> ()  [unwired: 2 in, 2 out]
          }
        }
        n1240 = call <vilib>:"Add State(s) to Queue__JKI_lib_State_Machine.vi"("State(s) in (\"\")"=w2663) -> ("States Out"=w2662:string)  [unwired: 14 in]
      }
      frame "355 Laser: CheckPWMStatus" {
        # "Check 355 laser PWM status\n(Read LJ DIO#EF_ENABLE register to determine PWM status)"
        n1241 = Unbundle By Name(w2681) -> ("LJ Pinout.355 PWM"=w2680:string)
        n1242 = call "LabJack_FGV.vi"("Operation(Read)"=enum16{"Write", "Read"}."Read" ("Operation"), "error in (no error)"=w2674) -> ("error out"=w2677:errorcluster, "Read data"=w2678:i32)  [unwired: 8 in]
        n1243 = Concatenate Strings(w2680, "_EF_ENABLE" ("string")) -> (w2676:string)
        n1244 = call "LJM_eReadName.vi"("Handle In"=w2678, "Name"=w2676, "error in"=w2677) -> ("Value"=w2673:dbl, "error out"=w2675:errorcluster)  [unwired: 10 in, 1 out]
        n1245 = Greater Than 0?(x=w2673) -> (x > 0?=w2672:bool)
        n1246 = case shown="False" w2672 {
          frame False {
            # "PWM is off\nset color to gray"
            n1247 = local write "355nm Laser toggle"(FALSE ("355nm Laser")) -> ()
          }
          frame True {
            # "PWM is on\nset color to light green"
            n1248 = local write "355nm Laser toggle"(TRUE ("355nm Laser")) -> ()
          }
        }
        n1249 = call <vilib>:"Add State(s) to Queue__JKI_lib_State_Machine.vi"("State(s) in (\"\")"=w2685) -> ("States Out"=w2684:string)  [unwired: 14 in]
      }
      frame "355 Laser: Start" {
        # "Template Separator\n(You can make a copy of, or modify, this frame)"
        n1250 = call <vilib>:"Add State(s) to Queue__JKI_lib_State_Machine.vi"("State(s) in Front (\"\")"="LabJack: 355_PWM_Start", "State(s) in (\"\")"=w2693) -> ("States Out"=w2692:string)  [unwired: 13 in]
      }
      frame "355 Laser: Stop" {
        # "Template Separator\n(You can make a copy of, or modify, this frame)"
        n1251 = call <vilib>:"Add State(s) to Queue__JKI_lib_State_Machine.vi"("State(s) in Front (\"\")"="LabJack: 355_PWM_Stop", "State(s) in (\"\")"=w2699) -> ("States Out"=w2698:string)  [unwired: 13 in]
      }
      frame "---------- Utility ----------" {
        # "Template Separator\n(You can make a copy of, or modify, this frame)"
        n1252 = call <vilib>:"Add State(s) to Queue__JKI_lib_State_Machine.vi"("State(s) in (\"\")"=w2704) -> ("States Out"=w2703:string)  [unwired: 14 in]
      }
      frame "Utility: SetDataClass" {
        # "Set Data Class in Queues\n(Set data class to either Data, Bg or Cali)"
        n1253 = case shown="\"Cali\"" w2706 {
          tunnel: [enum16{"Data", "BG", "Cali"}."Data" ("Data Class") enum16{"Data", "BG", "Cali"}."BG" ("Data Class") enum16{"Data", "BG", "Cali"}."Cali" ("Data Class")] -> w2705
          frame "Data", Default {
          }
          frame "Bg" {
          }
          frame "Cali" {
          }
        }
        n1254 = local write "Data Class"(w2705) -> ()
        n1255 = call <vilib>:"Add State(s) to Queue__JKI_lib_State_Machine.vi"("State(s) in (\"\")"=w2711) -> ("States Out"=w2710:string)  [unwired: 14 in]
      }
      frame "Utility: AquiTimerReset" {
        # "Set Aquisition Timer\n(You can make a copy of, or modify, this frame)"
        n1256 = Tick Count (ms)() -> (millisecond timer value=w2717:u32)
        n1257 = Bundle By Name(cluster=w2715, "Aquisition Timer"=w2717) -> (w2716:T23)
        n1258 = call <vilib>:"Add State(s) to Queue__JKI_lib_State_Machine.vi"("State(s) in (\"\")"=w2721) -> ("States Out"=w2720:string)  [unwired: 14 in]
      }
      frame "Utility: AquiTimerCheck" {
        # "5min to ms"
        # "Set Aquisition Timer\n([Covers: REQ35])"
        n1259 = Unbundle By Name(w2729) -> ("Aquisition Timer"=w2727:u32)
        n1260 = Tick Count (ms)() -> (millisecond timer value=w2728:u32)
        n1261 = Subtract(x=w2728, y=w2727) -> (x-y=w2726:u32)
        n1262 = Multiply(x=1000, y=300) -> (x*y=w2723:i32)
        n1263 = Greater Or Equal?(x=w2726, y=w2723) -> (x >= y?=w2722:bool)
        n1264 = case shown="True" w2722 {
          frame False {
            # "do nothing"
          }
          frame True {
            # "if timed out, stop aquisition"
            n1265 = property on="StopButton" class="Bool (strict)"("Val(Sgnl)"=TRUE ("Value (Signaling)")) -> ()  [unwired: 2 in, 2 out]
          }
        }
        n1266 = call <vilib>:"Add State(s) to Queue__JKI_lib_State_Machine.vi"("State(s) in (\"\")"=w2733) -> ("States Out"=w2732:string)  [unwired: 14 in]
      }
      frame "Utility: StartBeep" {
        # "Beep\n([Covers: REQ18])"
        n1267 = call <vilib>:"Beep.vi"("use system alert? (T)"=FALSE, "duration (msec)"=u32 1000, "frequency (Hz)"=u32 2000) -> ()  [unwired: 9 in]
        n1268 = call <vilib>:"Add State(s) to Queue__JKI_lib_State_Machine.vi"("State(s) in (\"\")"=w2742) -> ("States Out"=w2741:string)  [unwired: 14 in]
      }
      frame "Utility: EndBeep" {
        # "Beep\n([Covers: REQ18])"
        n1269 = flat-sequence {
          frame #0 {
            n1270 = call <vilib>:"Beep.vi"("use system alert? (T)"=FALSE, "duration (msec)"=u32 500, "frequency (Hz)"=u32 2000) -> ()  [unwired: 9 in]
          }
          frame #1 {
            n1271 = call <vilib>:"Beep.vi"("use system alert? (T)"=FALSE, "duration (msec)"=u32 500, "frequency (Hz)"=u32 2000) -> ()  [unwired: 9 in]
          }
        }
        n1272 = call <vilib>:"Add State(s) to Queue__JKI_lib_State_Machine.vi"("State(s) in (\"\")"=w2747) -> ("States Out"=w2746:string)  [unwired: 14 in]
      }
      frame "Utility: RestoreDeConChan" {
        # "Template Separator\n(You can make a copy of, or modify, this frame)"
        n1273 = global read "GlobalVariables.vi" "DeconChan Temp"() -> (w2754:T9)
        n1274 = local write "Radio Buttons"(w2754) -> ()
        n1275 = call <vilib>:"Add State(s) to Queue__JKI_lib_State_Machine.vi"("State(s) in (\"\")"=w2759) -> ("States Out"=w2758:string)  [unwired: 14 in]
      }
      frame "Utility: SaveDeconChan" {
        # "Save Decon Channel to global temp\n(You can make a copy of, or modify, this frame)"
        n1276 = flat-sequence {
          frame #0 {
            n1277 = local read "Radio Buttons"() -> (w2765:T9)
            n1278 = global write "GlobalVariables.vi" "DeconChan Temp"(w2765) -> ()
          }
          frame #1 {
            n1279 = local write "Radio Buttons"(T9."No Selection" ("Radio Buttons")) -> ()
          }
        }
        n1280 = flat-sequence {
          frame #0 {
          }
          frame #1 {
            (unwired) enum32{"No Selection", "Ch1", "Ch2", "Ch3"}."No Selection" ("Radio Buttons")
          }
        }
        n1281 = call <vilib>:"Add State(s) to Queue__JKI_lib_State_Machine.vi"("State(s) in (\"\")"=w2764) -> ("States Out"=w2763:string)  [unwired: 14 in]
      }
      frame "Utility: Dewelling" {
        # "Main loop dewell\n(Dewelling >> #)"
        n1282 = Fract/Exp String To Number(string=w2770, default (0 dbl)=0) -> (number=w2768:i32)  [unwired: 2 in, 1 out]
        n1283 = Wait (ms)(milliseconds to wait=w2768) -> ()  [unwired: 1 out]
        n1284 = call <vilib>:"Add State(s) to Queue__JKI_lib_State_Machine.vi"("State(s) in (\"\")"=w2774) -> ("States Out"=w2773:string)  [unwired: 14 in]
      }
      frame "Utility: SetAllChanManualGain" {
        w2775 = FALSE ("Value (Signaling)")
        # "Set all channel to manual gain\n(You can make a copy of, or modify, this frame)"
        n1285 = property on="Auto gain ch1" class="Bool (strict)"("Val(Sgnl)"=w2775) -> ()  [unwired: 2 in, 2 out]
        n1286 = property on="Auto gain ch2" class="Bool (strict)"("Val(Sgnl)"=w2775) -> ()  [unwired: 2 in, 2 out]
        n1287 = property on="Auto gain ch3" class="Bool (strict)"("Val(Sgnl)"=w2775) -> ()  [unwired: 2 in, 2 out]
        n1288 = property on="Auto gain ch4" class="Bool (strict)"("Val(Sgnl)"=w2775) -> ()  [unwired: 2 in, 2 out]
        n1289 = call <vilib>:"Add State(s) to Queue__JKI_lib_State_Machine.vi"("State(s) in (\"\")"=w2780) -> ("States Out"=w2779:string)  [unwired: 14 in]
      }
      frame "Utility: SetAllChanAutoGain" {
        w2781 = TRUE ("Value (Signaling)")
        # "Set all channels to auto gain\n(You can make a copy of, or modify, this frame)"
        n1290 = property on="Auto gain ch1" class="Bool (strict)"("Val(Sgnl)"=w2781) -> ()  [unwired: 2 in, 2 out]
        n1291 = property on="Auto gain ch2" class="Bool (strict)"("Val(Sgnl)"=w2781) -> ()  [unwired: 2 in, 2 out]
        n1292 = property on="Auto gain ch3" class="Bool (strict)"("Val(Sgnl)"=w2781) -> ()  [unwired: 2 in, 2 out]
        n1293 = property on="Auto gain ch4" class="Bool (strict)"("Val(Sgnl)"=w2781) -> ()  [unwired: 2 in, 2 out]
        n1294 = call <vilib>:"Add State(s) to Queue__JKI_lib_State_Machine.vi"("State(s) in (\"\")"=w2786) -> ("States Out"=w2785:string)  [unwired: 14 in]
      }
      frame "---------- SysLog ----------" {
        # "Template Separator\n(You can make a copy of, or modify, this frame)"
        n1295 = call <vilib>:"Add State(s) to Queue__JKI_lib_State_Machine.vi"("State(s) in (\"\")"=w2791) -> ("States Out"=w2790:string)  [unwired: 14 in]
      }
      frame "SysLog: OpenLogFile" {
        # "Template Separator\n(You can make a copy of, or modify, this frame)"
        n1296 = call <vilib>:"Add State(s) to Queue__JKI_lib_State_Machine.vi"("State(s) in (\"\")"=w2796) -> ("States Out"=w2795:string)  [unwired: 14 in]
      }
      frame "---------- Graph ----------" {
        # "Template Separator\n(You can make a copy of, or modify, this frame)"
        n1297 = call <vilib>:"Add State(s) to Queue__JKI_lib_State_Machine.vi"("State(s) in (\"\")"=w2801) -> ("States Out"=w2800:string)  [unwired: 14 in]
      }
      frame "Graph: SetXMultiplier" {
        # "Set X multiplier of WF graphs\n(You can make a copy of, or modify, this frame)"
        n1298 = call "Digitizer1_FGV.vi"() -> ("error out"=w2805:errorcluster, "Read data"=w2806:refnum<k15>)  [unwired: 10 in]
        n1299 = property class="niScope"(reference=w2806, error in=w2805) -> ("Min Sample Rate"=w2804:dbl)  [unwired: 2 out]
        n1300 = Divide(x=1.0, y=w2804) -> (x/y=w2802:dbl)
        n1301 = property on="Channel 1" class="WFGraph (strict)"("XScale.Multiplier"=w2802) -> ()  [unwired: 2 in, 2 out]
        n1302 = property on="Channel 2" class="WFGraph (strict)"("XScale.Multiplier"=w2802) -> ()  [unwired: 2 in, 2 out]
        n1303 = property on="Channel 3" class="WFGraph (strict)"("XScale.Multiplier"=w2802) -> ()  [unwired: 2 in, 2 out]
        n1304 = property on="Channel 4" class="WFGraph (strict)"("XScale.Multiplier"=w2802) -> ()  [unwired: 2 in, 2 out]
        n1305 = call <vilib>:"Add State(s) to Queue__JKI_lib_State_Machine.vi"("State(s) in (\"\")"=w2811) -> ("States Out"=w2810:string)  [unwired: 14 in]
      }
      frame "Graph: AddCursors" {
        # "Add BG and DC cursor to all graphs\n(You can make a copy of, or modify, this frame)"
        n1306 = property on="Channel 1" class="WFGraph (strict)"() -> ("XScale.Multiplier"=w2820:dbl)  [unwired: 2 in, 2 out]
        n1307 = global read "GlobalVariables.vi" "DC Idx1"() -> (w2819:i32)
        n1308 = global read "GlobalVariables.vi" "DC Idx2"() -> (w2818:i32)
        n1309 = global read "GlobalVariables.vi" "BG Idx1"() -> (w2817:i32)
        n1310 = global read "GlobalVariables.vi" "BG Idx2"() -> (w2816:i32)
        n1311 = property on="Channel 1" class="WFGraph (strict)"(error in=w2822) -> ("CrsrList"=w2831:T24)  [unwired: 1 in, 2 out]
        n1312 = property on="Channel 2" class="WFGraph (strict)"() -> ("CrsrList"=w2828:T24)  [unwired: 2 in, 2 out]
        n1313 = property on="Channel 3" class="WFGraph (strict)"() -> ("CrsrList"=w2827:T24)  [unwired: 2 in, 2 out]
        n1314 = property on="Channel 4" class="WFGraph (strict)"() -> ("CrsrList"=w2813:T24)  [unwired: 2 in, 2 out]
        n1315 = Build Array(w2819, w2818, w2817, w2816) -> (w2815:i32[])
        n1316 = Multiply(x=w2815, y=w2820) -> (x*y=w2814:dbl[])
        n1317 = for {
          tunnel: w2831 -> [w2845] mode=indexing
          tunnel: w2814 -> [w2838] mode=indexing
          tunnel: [w2844] -> w2830 mode=indexing
          tunnel: u32[] [6618880, 6618880, 16711680, 16711680] -> [w2837] mode=indexing
          tunnel: w2828 -> [w2843] mode=indexing
          tunnel: w2827 -> [w2842] mode=indexing
          tunnel: [w2841] -> w2826 mode=indexing
          tunnel: [w2840] -> w2825 mode=indexing
          tunnel: w2813 -> [w2839] mode=indexing
          tunnel: [w2836] -> w2812 mode=indexing
          n1318 = Bundle By Name(cluster=w2845, "Position.X"=w2838, "Color"=w2837) -> (w2844:T25)
          n1319 = Bundle By Name(cluster=w2843, "Position.X"=w2838, "Color"=w2837) -> (w2841:T25)
          n1320 = Bundle By Name(cluster=w2842, "Position.X"=w2838, "Color"=w2837) -> (w2840:T25)
          n1321 = Bundle By Name(cluster=w2839, "Position.X"=w2838, "Color"=w2837) -> (w2836:T25)
        }
        n1322 = property on="Channel 1" class="WFGraph (strict)"("CrsrList"=w2830) -> (error out=w2821:errorcluster)  [unwired: 2 in, 1 out]
        n1323 = property on="Channel 2" class="WFGraph (strict)"("CrsrList"=w2826) -> ()  [unwired: 2 in, 2 out]
        n1324 = property on="Channel 3" class="WFGraph (strict)"("CrsrList"=w2825) -> ()  [unwired: 2 in, 2 out]
        n1325 = property on="Channel 4" class="WFGraph (strict)"("CrsrList"=w2812) -> ()  [unwired: 2 in, 2 out]
        n1326 = control-ref of="Channel 1"() -> (w2824:refnum<vi>)
        n1327 = call <vilib>:"Add State(s) to Queue__JKI_lib_State_Machine.vi"("State(s) in (\"\")"=w2835) -> ("States Out"=w2834:string)  [unwired: 14 in]
        n1328 = call "UpdateCurserIdx(SubVI).vi"("error in (no error)"=w2821, "WaveformGraph in"=w2824) -> ("error out"=w2823:errorcluster)  [unwired: 9 in]
      }
      frame "Graph: SaveCursorLoc" {
        # "Save cursor location to ini file\n(Save cursor location to system setting ini file)"
        n1329 = global read "GlobalVariables.vi" "DC Idx1"() -> (w2852:i32)
        n1330 = global read "GlobalVariables.vi" "DC Idx2"() -> (w2851:i32)
        n1331 = global read "GlobalVariables.vi" "BG Idx1"() -> (w2850:i32)
        n1332 = global read "GlobalVariables.vi" "BG Idx2"() -> (w2849:i32)
        n1333 = Bundle("DC Idx1"=w2852, "DC Idx2"=w2851, "BG Idx1"=w2850, "BG Idx2"=w2849) -> (w2848:T47)  [unwired: 1 in]
        n1334 = call "writeCursorConfigMain.vi"("error in (no error)"=w2846, "Cursor Locations"=w2848) -> ("error out"=w2847:errorcluster)  [unwired: 9 in]
        n1335 = call <vilib>:"Add State(s) to Queue__JKI_lib_State_Machine.vi"("State(s) in (\"\")"=w2856) -> ("States Out"=w2855:string)  [unwired: 14 in]
      }
      frame "---------- APD ----------" {
        # "Template Separator\n(You can make a copy of, or modify, this frame)"
        n1336 = call <vilib>:"Add State(s) to Queue__JKI_lib_State_Machine.vi"("State(s) in (\"\")"=w2861) -> ("States Out"=w2860:string)  [unwired: 14 in]
      }
      frame "APD: Initialize" {
        w2868 = enum16{"Read", "Write"}."Write" ("Operation (Read)")
        w2867 = refnum<class "APDClass.lvclass"> refnum  # APDClass.lvclass
        # "Initialize APD FGV\n(Initialized APD FGV for holding data)"
        n1337 = call "APD1FGV.vi"("Error In"=w2862, "Operation (Read)"=w2868, "APDClass in"=w2867) -> ("Error Out"=w2866:errorcluster)  [unwired: 7 in, 1 out]
        n1338 = call "APD2FGV.vi"("Error In"=w2862, "Operation (Read)"=w2868, "APDClass in"=w2867) -> ("Error Out"=w2865:errorcluster)  [unwired: 7 in, 1 out]
        n1339 = call "APD3FGV.vi"("Error In"=w2862, "Operation (Read)"=w2868, "APDClass in"=w2867) -> ("Error Out"=w2864:errorcluster)  [unwired: 7 in, 1 out]
        n1340 = Merge Errors(w2866, w2865, w2864) -> (w2863:errorcluster)
        n1341 = call <vilib>:"Add State(s) to Queue__JKI_lib_State_Machine.vi"("State(s) in (\"\")"=w2872) -> ("States Out"=w2871:string)  [unwired: 14 in]
      }
      frame "APD: LoadFromSerial" {
        w2874 = enum16{"Read", "Write"}."Write" ("Operation (Read)")
        # "Load APD data from tdms file\n(load and update FGV)"
        n1342 = call "readAPDSerial.vi"("Error In"=w2881) -> ("Error Out"=w2877:errorcluster, "output cluster"=w2880:T26)  [unwired: 9 in]
        n1343 = Unbundle By Name(w2880) -> ("Ch1APDSerial#"=w2893:string, "Ch2APDSerial#"=w2879:string, "Ch3APDSerial#"=w2892:string, "Ch4APDSerial#"=w2878:string)
        n1344 = call "CreatFromSerialNumNoRaw.vi"("error in (no error)"=w2877, "APD Serial #"=w2893) -> ("error out"=w2890:errorcluster, "APDClass out"=w2891:refnum<class "APDClass.lvclass">)  [unwired: 8 in]
        n1345 = call "CreatFromSerialNumNoRaw.vi"("error in (no error)"=w2877, "APD Serial #"=w2879) -> ("error out"=w2888:errorcluster, "APDClass out"=w2889:refnum<class "APDClass.lvclass">)  [unwired: 8 in]
        n1346 = call "CreatFromSerialNumNoRaw.vi"("error in (no error)"=w2877, "APD Serial #"=w2892) -> ("error out"=w2886:errorcluster, "APDClass out"=w2887:refnum<class "APDClass.lvclass">)  [unwired: 8 in]
        n1347 = call "CreatFromSerialNumNoRaw.vi"("error in (no error)"=w2877, "APD Serial #"=w2878) -> ("error out"=w2875:errorcluster, "APDClass out"=w2876:refnum<class "APDClass.lvclass">)  [unwired: 8 in]
        n1348 = call "APD1FGV.vi"("Error In"=w2890, "Operation (Read)"=w2874, "APDClass in"=w2891) -> ("Error Out"=w2885:errorcluster)  [unwired: 7 in, 1 out]
        n1349 = call "APD2FGV.vi"("Error In"=w2888, "Operation (Read)"=w2874, "APDClass in"=w2889) -> ("Error Out"=w2883:errorcluster)  [unwired: 7 in, 1 out]
        n1350 = call "APD3FGV.vi"("Error In"=w2886, "Operation (Read)"=w2874, "APDClass in"=w2887) -> ("Error Out"=w2884:errorcluster)  [unwired: 7 in, 1 out]
        n1351 = call "APD4FGV.vi"("Error In"=w2875, "Operation (Read)"=w2874, "APDClass in"=w2876) -> ("Error Out"=w2873:errorcluster)  [unwired: 7 in, 1 out]
        n1352 = Merge Errors(w2885, w2883, w2884, w2873) -> (w2882:errorcluster)
        n1353 = call <vilib>:"Add State(s) to Queue__JKI_lib_State_Machine.vi"("State(s) in (\"\")"=w2897) -> ("States Out"=w2896:string)  [unwired: 14 in]
      }
      frame "APD: UpdateCtrlVLimit" {
        w2903 = enum16{"Read", "Write"}."Read" ("Operation (Read)")
        # "Set V limit\n(You can make a copy of, or modify, this frame)"
        n1354 = call "APD1FGV.vi"("Error In"=w2904, "Operation (Read)"=w2903) -> ("Error Out"=w2919:errorcluster, "APDClass out"=w2920:refnum<class "APDClass.lvclass">)  [unwired: 8 in]
        n1355 = call "APD2FGV.vi"("Error In"=w2904, "Operation (Read)"=w2903) -> ("Error Out"=w2917:errorcluster, "APDClass out"=w2918:refnum<class "APDClass.lvclass">)  [unwired: 8 in]
        n1356 = call "APD3FGV.vi"("Error In"=w2904, "Operation (Read)"=w2903) -> ("Error Out"=w2915:errorcluster, "APDClass out"=w2916:refnum<class "APDClass.lvclass">)  [unwired: 8 in]
        n1357 = call "APD4FGV.vi"("Error In"=w2904, "Operation (Read)"=w2903) -> ("Error Out"=w2901:errorcluster, "APDClass out"=w2902:refnum<class "APDClass.lvclass">)  [unwired: 8 in]
        n1358 = call-dynamic "ReadMaxCtrlV.vi"("error in (no error)"=w2919, "APDClass in"=w2920) -> ("error out"=w2910:errorcluster, "Numeric"=w2913:dbl)  [unwired: 7 in, 1 out]
        n1359 = call-dynamic "ReadMaxCtrlV.vi"("error in (no error)"=w2917, "APDClass in"=w2918) -> ("error out"=w2908:errorcluster, "Numeric"=w2912:dbl)  [unwired: 7 in, 1 out]
        n1360 = call-dynamic "ReadMaxCtrlV.vi"("error in (no error)"=w2915, "APDClass in"=w2916) -> ("error out"=w2906:errorcluster, "Numeric"=w2911:dbl)  [unwired: 7 in, 1 out]
        n1361 = call-dynamic "ReadMaxCtrlV.vi"("error in (no error)"=w2901, "APDClass in"=w2902) -> ("error out"=w2899:errorcluster, "Numeric"=w2900:dbl)  [unwired: 7 in, 1 out]
        n1362 = property on="V 1" class="DigNum (strict)"(error in=w2910, "Maximum"=w2913) -> (error out=w2909:errorcluster)  [unwired: 1 in, 1 out]
        n1363 = property on="V 2" class="DigNum (strict)"(error in=w2908, "Maximum"=w2912) -> (error out=w2907:errorcluster)  [unwired: 1 in, 1 out]
        n1364 = property on="V 4" class="DigNum (strict)"(error in=w2899, "Maximum"=w2900) -> (error out=w2898:errorcluster)  [unwired: 1 in, 1 out]
        n1365 = property on="V 3" class="DigNum (strict)"(error in=w2906, "Maximum"=w2911) -> (error out=w2905:errorcluster)  [unwired: 1 in, 1 out]
        n1366 = Merge Errors(w2909, w2907, w2905, w2898) -> (w2914:errorcluster)
        n1367 = call <vilib>:"Add State(s) to Queue__JKI_lib_State_Machine.vi"("State(s) in (\"\")"=w2924) -> ("States Out"=w2923:string)  [unwired: 14 in]
      }
      frame "APD: GetGainLimits" {
        w2929 = enum16{"Read", "Write"}."Read" ("Operation (Read)")
        # "Template Separator\n(You can make a copy of, or modify, this frame)"
        n1368 = call "APD1FGV.vi"("Error In"=w2930, "Operation (Read)"=w2929) -> ("Error Out"=w2935:errorcluster, "APDClass out"=w2936:refnum<class "APDClass.lvclass">)  [unwired: 8 in]
        n1369 = call "APD2FGV.vi"("Error In"=w2930, "Operation (Read)"=w2929) -> ("Error Out"=w2942:errorcluster, "APDClass out"=w2943:refnum<class "APDClass.lvclass">)  [unwired: 8 in]
        n1370 = call "APD3FGV.vi"("Error In"=w2930, "Operation (Read)"=w2929) -> ("Error Out"=w2940:errorcluster, "APDClass out"=w2941:refnum<class "APDClass.lvclass">)  [unwired: 8 in]
        n1371 = call "APD4FGV.vi"("Error In"=w2930, "Operation (Read)"=w2929) -> ("Error Out"=w2927:errorcluster, "APDClass out"=w2928:refnum<class "APDClass.lvclass">)  [unwired: 8 in]
        n1372 = call-dynamic "Read Gain Limits(Log).vi"("error in (no error)"=w2935, "APDClass in"=w2936) -> ("error out"=w2934:errorcluster, "GainLimits(Log)"=w2931:cluster{"GainMax":dbl, "GainMin":dbl})  [unwired: 7 in, 1 out]
        n1373 = call-dynamic "Read Gain Limits(Log).vi"("error in (no error)"=w2942, "APDClass in"=w2943) -> ("error out"=w2938:errorcluster, "GainLimits(Log)"=w2933:cluster{"GainMax":dbl, "GainMin":dbl})  [unwired: 7 in, 1 out]
        n1374 = call-dynamic "Read Gain Limits(Log).vi"("error in (no error)"=w2940, "APDClass in"=w2941) -> ("error out"=w2937:errorcluster, "GainLimits(Log)"=w2932:cluster{"GainMax":dbl, "GainMin":dbl})  [unwired: 7 in, 1 out]
        n1375 = call-dynamic "Read Gain Limits(Log).vi"("error in (no error)"=w2927, "APDClass in"=w2928) -> ("error out"=w2925:errorcluster, "GainLimits(Log)"=w2926:cluster{"GainMax":dbl, "GainMin":dbl})  [unwired: 7 in, 1 out]
        n1376 = Merge Errors(w2934, w2938, w2937, w2925) -> (w2939:errorcluster)
        n1377 = global write "GlobalVariables.vi" "Ch1GainLim(Log)"(w2931) -> ()
        n1378 = global write "GlobalVariables.vi" "Ch2GainLim(Log)"(w2933) -> ()
        n1379 = global write "GlobalVariables.vi" "Ch3GainLim(Log)"(w2932) -> ()
        n1380 = global write "GlobalVariables.vi" "Ch4GainLim(Log)"(w2926) -> ()
        n1381 = call <vilib>:"Add State(s) to Queue__JKI_lib_State_Machine.vi"("State(s) in (\"\")"=w2947) -> ("States Out"=w2946:string)  [unwired: 14 in]
      }
      frame "---------- TCP ----------" {
        # "Template Separator\n(You can make a copy of, or modify, this frame)"
        n1382 = call <vilib>:"Add State(s) to Queue__JKI_lib_State_Machine.vi"("State(s) in (\"\")"=w2952) -> ("States Out"=w2951:string)  [unwired: 14 in]
      }
      frame "TCP: InitializeNew" {
        # "if unsuccessful and count <10, increament count \nand try again"
        # "Initialize TCP connection to aimging beam computer\n(You can make a copy of, or modify, this frame)"
        n1383 = TCP Create Listener(10:u16 2100 ("port"), 11:"RTLT" ("service name")) -> (0:w2961:errorcluster, 3:w2953:refnum<k5>)  [unwired: 3 in, 1 out]
        n1384 = while {
          tunnel: w2953 -> [w2981]
          tunnel: w2961 -> [w2980]
          tunnel: [w2971] -> w2959
          tunnel: [w2968] -> w2955
          i -> [w2977]
          stop <- w2968 stop-if-true
          n1385 = TCP Wait On Listener(8:w2980, 9:200 ("timeout ms (wait forever: -1)"), 11:w2981) -> (0:w2978:errorcluster, 4:w2975:refnum<k5>)  [unwired: 1 in, 3 out]
          n1386 = Less Or Equal?(x=50, y=w2977) -> (x <= y?=w2974:bool)
          n1387 = case shown="No Error" w2978 {
            selector: w2978 -> [w2991 w3001]
            tunnel: w2975 -> [w2992 _]
            tunnel: [errorcluster {"status"=TRUE, "code"=0, "source"=""} ("No error") w3002] -> w2970
            tunnel: [w2983 FALSE ("TCP connected?")] -> w2971
            frame No Error {
              # "connection is ready, read data"
              n1388 = TCP Read(connection ID=w2992, bytes to read=512, error in (no error)=w2991, 7:T21."CRLF" ("mode (standard)"), 9:5000 ("timeout ms (25000)")) -> (connection ID out=w2985:refnum<k5>, data out=w2987:string, error out=w2984:errorcluster)
              n1389 = Concatenate Strings("alive" ("string"), "\r\n" ("End of Line Constant")) -> (w2988:string)
              n1390 = Equal?(x=w2988, y=w2987) -> (x = y?=w2986:bool)
              n1391 = case shown="False" w2986 {
                tunnel: w2985 -> [_ w2997]
                tunnel: w2984 -> [_ _]
                tunnel: [FALSE ("TCP connected?") TRUE ("TCP connected?")] -> w2983
                frame False {
                }
                frame True {
                  n1392 = call "TcpIDFGV.vi"("action"=enum16{"write", "read"}."write", "connection ID in"=w2997) -> ()  [unwired: 8 in, 2 out]
                }
              }
            }
            frame Error {
              # "connection not ready, keep waiting"
              n1393 = Unbundle By Name(w3001) -> ("code"=w3003:i32)
              n1394 = case shown="56" w3003 {
                tunnel: w3001 -> [w3004 _]
                tunnel: [w3004 w3005] -> w3002
                frame Default {
                }
                frame 56 {
                  w3005 = errorcluster {"status"=FALSE, "code"=0, "source"=""}  # No error
                }
              }
            }
          }
          n1395 = Select(t=errorcluster {"status"=TRUE, "code"=5001, "source"=""} ("error in (no error)"), s=w2974, f=errorcluster {"status"=FALSE, "code"=0, "source"=""} ("error in (no error)")) -> (s? t:f=w2969:errorcluster)
          n1396 = Merge Errors(w2970, w2969) -> (w2968:errorcluster)
        }
        n1397 = Unbundle By Name(w2955) -> ("code"=w2958:i32)
        n1398 = Bundle By Name(cluster=w2960, "System Status.TCP/IP"=w2959, "listener ID"=w2953) -> (w2965:T23)
        n1399 = global write "GlobalVariables.vi" "TCP connected?"(w2959) -> ()
        n1400 = Equal To 0?(x=w2958) -> (x = 0?=w2957:bool)
        n1401 = Select(t=errorcluster {"status"=FALSE, "code"=0, "source"=""} ("error in (no error)"), s=w2957, f=w2955) -> (s? t:f=w2954:errorcluster)
        n1402 = call <vilib>:"Add State(s) to Queue__JKI_lib_State_Machine.vi"("State(s) in (\"\")"=w2967) -> ("States Out"=w2966:string)  [unwired: 14 in]
      }
      frame "TCP: checkSource" {
        # "Check visualization PC video source\n(send !video_source message, listen for response, then parse it to binary mask)"
        n1403 = Unbundle By Name(w3012) -> ("System Status.TCP/IP"=w3015:bool)
        n1404 = case shown="True" w3015 {
          tunnel: w3014 -> [w3020 w3043]
          tunnel: [w3020 w3027] -> w3013
          tunnel: [w3019 w3032] -> w3010
          tunnel: [w3019 w3030] -> w3009
          tunnel: [w3019 w3031] -> w3008
          tunnel: [w3019 w3029] -> w3007
          tunnel: [w3019 w3021] -> w3006
          frame False {
            w3019 = FALSE
          }
          frame True {
            n1405 = call "TcpIDFGV.vi"("Error In"=w3043, "action"=enum16{"write", "read"}."read") -> ("Error Out"=w3040:errorcluster, "connection ID out"=w3042:refnum<k5>)  [unwired: 8 in]
            n1406 = call "TCP_WriteRead.vi"("error in (no error)"=w3040, "data in"="!video_source", "connectin ID in"=w3042) -> ("error out"=w3037:errorcluster, "data out"=w3039:string)  [unwired: 4 in, 1 out]
            n1407 = Scan From String(format string="!video_source:%d", input string=w3039, error in=w3037) -> (error out=w3028:errorcluster, output 1=w3026:i32)  [unwired: 2 in, 2 out]
            n1408 = case shown="5..7, 9..11, 13..15" w3026 {
              tunnel: w3028 -> [_ _ _ _]
              tunnel: [errorcluster {"status"=TRUE, "code"=5007, "source"="Visualization PC"} ("error out") errorcluster {"status"=FALSE, "code"=0, "source"=""} ("error out") errorcluster {"status"=FALSE, "code"=0, "source"=""} ("error out") errorcluster {"status"=FALSE, "code"=0, "source"=""} ("error out")] -> w3027
              tunnel: [FALSE FALSE FALSE TRUE] -> w3021
              frame 0, Default {
                # "No video source available or default"
                n1409 = property on="Video Source" class="RadioBtnsControl (strict)"("DisabledEnum"=T11."Disabled and Grayed Out" ("Disabled")) -> ()  [unwired: 2 in, 2 out]
              }
              frame 1..3 {
                # "one or both camera available"
                n1410 = local write "Video Source"(enum32{"Camera", "FrameGrabber"}."Camera" ("Video Source")) -> ()
                n1411 = property on="Video Source" class="RadioBtnsControl (strict)"("DisabledEnum"=T11."Disabled and Grayed Out" ("Disabled")) -> ()  [unwired: 2 in, 2 out]
              }
              frame 4, 8, 12 {
                # "one or both frame grabber available"
                n1412 = local write "Video Source"(enum32{"Camera", "FrameGrabber"}."FrameGrabber" ("Video Source")) -> ()
                n1413 = property on="Video Source" class="RadioBtnsControl (strict)"("DisabledEnum"=T11."Disabled and Grayed Out" ("Disabled")) -> ()  [unwired: 2 in, 2 out]
              }
              frame 5..7, 9..11, 13..15 {
                n1414 = property on="Video Source" class="RadioBtnsControl (strict)"("DisabledEnum"=T11."Enabled" ("Disabled")) -> ()  [unwired: 2 in, 2 out]
              }
            }
            n1415 = Integer to Fixed-Point Cast(fixed-point type=fxp<+,4,4> 0.0, integer=w3026) -> (fixed-point=w3025:fxp<+,4,4>)
            n1416 = Number To Boolean Array(number=w3025) -> (Boolean array=w3023:bool[])
            n1417 = Reverse 1D Array(array=w3023) -> (reversed array=w3022:bool[])
            n1418 = Index Array(array=w3022, index=0) -> (element=w3032:bool)
            n1419 = Index Array(array=w3022, index=1) -> (element=w3030:bool)
            n1420 = Index Array(array=w3022, index=2) -> (element=w3031:bool)
            n1421 = Index Array(array=w3022, index=3) -> (element=w3029:bool)
          }
        }
        n1422 = Bundle By Name(cluster=w3012, "video source.Main Frame Grabber"=w3010, "video source.Side Frame Grabber"=w3009, "video source.Main Camera"=w3008, "video source.Side Camera"=w3007, "bothVidSourceAvail"=w3006) -> (w3011:T23)
        n1423 = call <vilib>:"Add State(s) to Queue__JKI_lib_State_Machine.vi"("State(s) in (\"\")"=w3018) -> ("States Out"=w3017:string)  [unwired: 14 in]
      }
      frame "TCP: SyncTime" {
        # "Template Separator\n(You can make a copy of, or modify, this frame)"
        n1424 = Unbundle By Name(w3060) -> ("System Status.TCP/IP"=w3059:bool)
        n1425 = case shown="True" w3059 {
          tunnel: w3061 -> [_ w3069]
          frame False {
          }
          frame True {
            n1426 = call "TcpIDFGV.vi"("Error In"=w3069, "action"=enum16{"write", "read"}."read") -> ("Error Out"=w3068:errorcluster, "connection ID out"=w3065:refnum<k5>)  [unwired: 8 in]
            n1427 = call <userlib>:"Tick Count (ms)__ogtk.vi"("error in (no error)"=w3068) -> ("error out"=w3067:errorcluster, "millisecond timer value"=w3066:u32)  [unwired: 9 in]
            n1428 = while {
              tunnel: w3067 -> [w3089]
              tunnel: w3065 -> [w3088]
              tunnel: w3066 -> [w3077]
              stop <- w3072 stop-if-true
              n1429 = Concatenate Strings("latencycheck" ("string"), "\r\n" ("End of Line Constant")) -> (w3084:string)
              n1430 = TCP Read(connection ID=w3088, bytes to read=512, error in (no error)=w3089, 7:T21."CRLF" ("mode (standard)"), 9:2000 ("timeout ms (25000)")) -> (connection ID out=w3081:refnum<k5>, data out=w3079:string, error out=w3071:errorcluster)
              n1431 = Tick Count (ms)() -> (millisecond timer value=w3078:u32)
              n1432 = Subtract(x=w3078, y=w3077) -> (x-y=w3076:u32)
              n1433 = Equal?(x=w3079, y=w3084) -> (x = y?=w3080:bool)
              n1434 = case shown="False" w3080 {
                tunnel: w3081 -> [_ w3102]
                tunnel: w3079 -> [w3094 _]
                tunnel: [w3090 FALSE] -> w3074
                tunnel: w3071 -> [_ w3096]
                frame False {
                  n1435 = Concatenate Strings("synctimer" ("string"), "\r\n" ("End of Line Constant")) -> (w3091:string)
                  n1436 = Equal?(x=w3094, y=w3091) -> (x = y?=w3090:bool)
                  "Sync Success?" <- w3090
                }
                frame True {
                  n1437 = Concatenate Strings("latencycheck:" ("string"), "\r\n" ("End of Line Constant")) -> (w3101:string)
                  n1438 = TCP Write(connection ID=w3102, data in=w3101, error in (no error)=w3096, 9:1000 ("timeout ms (25000)")) -> (error out=w3095:errorcluster)  [unwired: 2 out]
                  n1439 = call <vilib>:"Clear Errors.vi"("error in (no error)"=w3095) -> ()  [unwired: 5 in, 2 out]
                }
              }
              n1440 = Greater?(x=w3076, y=u32 10000 ("x-y")) -> (0:w3073:bool)
              n1441 = Or(x=w3074, y=w3073) -> (x .or. y?=w3072:bool)
            }
          }
        }
        n1442 = call <vilib>:"Add State(s) to Queue__JKI_lib_State_Machine.vi"("State(s) in (\"\")"=w3064) -> ("States Out"=w3063:string)  [unwired: 14 in]
      }
      frame "TCP: SendSettingMacro" {
        # "Template Separator\n(You can make a copy of, or modify, this frame)"
        n1443 = Unbundle By Name(w3106) -> ("System Status.TCP/IP"=w3105:bool)
        n1444 = case shown="True" w3105 {
          tunnel: ["" ("Empty String Constant") "TCP: sendSubjectID\nTCP: sendScaleBarSetting\nTCP: sendScaleMaxMin\nTCP: sendDeconChannel\nTCP: sendANSI\nTCP: sendRadius\nTCP: send3Dsetting\nTCP: sendFirefly\nTCP: sendPentero"] -> w3104
          frame False {
          }
          frame True {
          }
        }
        n1445 = call <vilib>:"Add State(s) to Queue__JKI_lib_State_Machine.vi"("State(s) in Front (\"\")"=w3104, "State(s) in (\"\")"=w3109) -> ("States Out"=w3108:string)  [unwired: 13 in]
      }
      frame "TCP: sendRunNum" {
        # "Send run number to AB PC\n(You can make a copy of, or modify, this frame)"
        n1446 = Unbundle By Name(w3116) -> ("System Status.TCP/IP"=w3113:bool, "IDs.RunID"=w3117:i8)
        n1447 = Increment(x=w3117) -> (x+1=w3112:i8)
        n1448 = case shown="True" w3113 {
          tunnel: w3112 -> [_ w3131]
          tunnel: [w3121 w3123] -> w3115
          tunnel: w3114 -> [w3121 w3122]
          frame False {
          }
          frame True {
            n1449 = Number To Decimal String(number=w3131, width (-)=i16 3) -> (decimal integer string=w3126:string)
            n1450 = call "TcpIDFGV.vi"("Error In"=w3122, "action"=enum16{"write", "read"}."read") -> ("Error Out"=w3124:errorcluster, "connection ID out"=w3128:refnum<k5>)  [unwired: 8 in]
            n1451 = Concatenate Strings("!run:", w3126) -> (w3125:string)
            n1452 = call "TCP_WriteRead.vi"("error in (no error)"=w3124, "data in"=w3125, "connectin ID in"=w3128) -> ("error out"=w3123:errorcluster)  [unwired: 4 in, 2 out]
          }
        }
        n1453 = call <vilib>:"Add State(s) to Queue__JKI_lib_State_Machine.vi"("State(s) in (\"\")"=w3120) -> ("States Out"=w3119:string)  [unwired: 14 in]
      }
      frame "TCP: sendVideoSource" {
        # "Send video source \n(You can make a copy of, or modify, this frame)"
        n1454 = Unbundle By Name(w3133) -> ("System Status.TCP/IP"=w3132:bool)
        n1455 = case shown="True" w3132 {
          tunnel: [w3139 w3141] -> w3135
          tunnel: w3134 -> [w3139 w3140]
          frame False {
          }
          frame True {
            n1456 = case shown="\"Camera\", Default" "Video Source" {
              tunnel: [0 1] -> w3146
              frame "Camera", Default {
              }
              frame "FrameGrabber" {
              }
            }
            n1457 = call "TcpIDFGV.vi"("Error In"=w3140, "action"=enum16{"write", "read"}."read") -> ("Error Out"=w3142:errorcluster, "connection ID out"=w3148:refnum<k5>)  [unwired: 8 in]
            n1458 = Number To Decimal String(number=w3146) -> (decimal integer string=w3144:string)  [unwired: 1 in]
            n1459 = Concatenate Strings("!invivo:" ("data in"), w3144) -> (w3143:string)
            n1460 = call "TCP_WriteRead.vi"("error in (no error)"=w3142, "data in"=w3143, "connectin ID in"=w3148) -> ("error out"=w3141:errorcluster)  [unwired: 4 in, 2 out]
          }
        }
        n1461 = call <vilib>:"Add State(s) to Queue__JKI_lib_State_Machine.vi"("State(s) in (\"\")"=w3138) -> ("States Out"=w3137:string)  [unwired: 14 in]
      }
      frame "TCP: startRun" {
        # "Template Separator\n(You can make a copy of, or modify, this frame)"
        n1462 = Unbundle By Name(w3153) -> ("System Status.TCP/IP"=w3152:bool)
        n1463 = case shown="True" w3152 {
          tunnel: [w3159 w3161] -> w3155
          tunnel: w3154 -> [w3159 w3160]
          frame False {
          }
          frame True {
            n1464 = call "TcpIDFGV.vi"("Error In"=w3160, "action"=enum16{"write", "read"}."read") -> ("Error Out"=w3162:errorcluster, "connection ID out"=w3163:refnum<k5>)  [unwired: 8 in]
            n1465 = call "TCP_WriteRead.vi"("error in (no error)"=w3162, "data in"="!acquire:1", "connectin ID in"=w3163) -> ("error out"=w3161:errorcluster)  [unwired: 4 in, 2 out]
          }
        }
        n1466 = call <vilib>:"Add State(s) to Queue__JKI_lib_State_Machine.vi"("State(s) in (\"\")"=w3158) -> ("States Out"=w3157:string)  [unwired: 14 in]
      }
      frame "TCP: stopRun" {
        # "Send stop run to AB PC\n(You can make a copy of, or modify, this frame)"
        n1467 = Unbundle By Name(w3167) -> ("System Status.TCP/IP"=w3166:bool)
        n1468 = case shown="True" w3166 {
          tunnel: [w3173 w3175] -> w3169
          tunnel: w3168 -> [w3173 w3174]
          frame False {
            # "if not connected, do nothing"
          }
          frame True {
            # "If TCP connected, send stop run"
            n1469 = call "TcpIDFGV.vi"("Error In"=w3174, "action"=enum16{"write", "read"}."read") -> ("Error Out"=w3176:errorcluster, "connection ID out"=w3178:refnum<k5>)  [unwired: 8 in]
            n1470 = call "TCP_WriteRead.vi"("error in (no error)"=w3176, "data in"="!acquire:0", "connectin ID in"=w3178) -> ("error out"=w3175:errorcluster)  [unwired: 4 in, 2 out]
          }
        }
        n1471 = call <vilib>:"Add State(s) to Queue__JKI_lib_State_Machine.vi"("State(s) in (\"\")"=w3172) -> ("States Out"=w3171:string)  [unwired: 14 in]
      }
      frame "TCP: CheckConnection" {
        # "Check TCP/IP connection statuse\n(If connection is lost, throw error)"
        n1472 = Unbundle By Name(w3181) -> ("System Status.TCP/IP"=w3180:bool)
        n1473 = case shown="False" w3180 {
          frame False {
          }
          frame True {
            # "If TCP/IP is true check, otherwise skip"
          }
        }
        n1474 = call <vilib>:"Add State(s) to Queue__JKI_lib_State_Machine.vi"("State(s) in (\"\")"=w3185) -> ("States Out"=w3184:string)  [unwired: 14 in]
      }
      frame "TCP: sendSubjectID" {
        # "Send subject ID"
        n1475 = Unbundle By Name(w3187) -> ("System Status.TCP/IP"=w3186:bool, "CaseID"=w3190:string)
        n1476 = case shown="True" w3186 {
          tunnel: w3190 -> [_ w3201]
          tunnel: [w3194 w3196] -> w3189
          tunnel: w3188 -> [w3194 w3195]
          frame False {
          }
          frame True {
            n1477 = call "TcpIDFGV.vi"("Error In"=w3195, "action"=enum16{"write", "read"}."read") -> ("Error Out"=w3197:errorcluster, "connection ID out"=w3199:refnum<k5>)  [unwired: 8 in]
            n1478 = Concatenate Strings("!subject:", w3201) -> (w3198:string)
            n1479 = call "TCP_WriteRead.vi"("error in (no error)"=w3197, "data in"=w3198, "connectin ID in"=w3199) -> ("error out"=w3196:errorcluster)  [unwired: 4 in, 2 out]
          }
        }
        n1480 = call <vilib>:"Add State(s) to Queue__JKI_lib_State_Machine.vi"("State(s) in (\"\")"=w3193) -> ("States Out"=w3192:string)  [unwired: 14 in]
      }
      frame "TCP: sendScaleBarSetting" {
        # "Template Separator\n(You can make a copy of, or modify, this frame)"
        n1481 = Unbundle By Name(w3205) -> ("System Status.TCP/IP"=w3203:bool, "VideoConfig.Scale Bar"=w3204:bool)
        n1482 = case shown="True" w3203 {
          tunnel: [w3211 w3220] -> w3207
          tunnel: w3206 -> [w3211 w3219]
          tunnel: w3204 -> [_ w3218]
          frame False {
          }
          frame True {
            n1483 = Boolean To (0,1)(Boolean=w3218) -> (0, 1=w3217:i16)
            n1484 = call "TcpIDFGV.vi"("Error In"=w3219, "action"=enum16{"write", "read"}."read") -> ("Error Out"=w3221:errorcluster, "connection ID out"=w3222:refnum<k5>)  [unwired: 8 in]
            n1485 = Number To Fractional String(number=w3217, width (-)=i16 1, precision (6)=i16 0) -> (F-format string=w3215:string)  [unwired: 1 in]
            n1486 = Concatenate Strings("!autocolor:" ("data in"), w3215) -> (w3213:string)
            n1487 = call "TCP_WriteRead.vi"("error in (no error)"=w3221, "data in"=w3213, "connectin ID in"=w3222) -> ("error out"=w3220:errorcluster)  [unwired: 4 in, 2 out]
          }
        }
        n1488 = call <vilib>:"Add State(s) to Queue__JKI_lib_State_Machine.vi"("State(s) in (\"\")"=w3210) -> ("States Out"=w3209:string)  [unwired: 14 in]
      }
      frame "TCP: sendScaleMaxMin" {
        # "Send scale bar max and min to AB PC\n(You can make a copy of, or modify, this frame)"
        n1489 = Unbundle By Name(w3227) -> ("System Status.TCP/IP"=w3224:bool, "VideoConfig.Scale Low"=w3226:dbl, "VideoConfig.Scale High"=w3225:dbl)
        n1490 = case shown="True" w3224 {
          tunnel: [w3233 w3246] -> w3229
          tunnel: w3228 -> [w3233 w3245]
          tunnel: w3226 -> [_ w3244]
          tunnel: w3225 -> [_ w3235]
          frame False {
          }
          frame True {
            n1491 = call "TcpIDFGV.vi"("Error In"=w3245, "action"=enum16{"write", "read"}."read") -> ("Error Out"=w3247:errorcluster, "connection ID out"=w3248:refnum<k5>)  [unwired: 8 in]
            n1492 = Number To Fractional String(number=w3244, width (-)=i16 4, precision (6)=i16 2) -> (F-format string=w3240:string)  [unwired: 1 in]
            n1493 = Number To Fractional String(number=w3235, width (-)=i16 4, precision (6)=i16 2) -> (F-format string=w3236:string)  [unwired: 1 in]
            n1494 = Concatenate Strings("!color:" ("string"), w3240, ";" ("string"), w3236) -> (w3234:string)
            n1495 = call "TCP_WriteRead.vi"("error in (no error)"=w3247, "data in"=w3234, "connectin ID in"=w3248) -> ("error out"=w3246:errorcluster)  [unwired: 4 in, 2 out]
          }
        }
        n1496 = call <vilib>:"Add State(s) to Queue__JKI_lib_State_Machine.vi"("State(s) in (\"\")"=w3232) -> ("States Out"=w3231:string)  [unwired: 14 in]
      }
      frame "TCP: sendDeconChannel" {
        # "Send Decon channel\n(You can make a copy of, or modify, this frame)"
        n1497 = Unbundle By Name(w3251) -> ("System Status.TCP/IP"=w3250:bool)
        n1498 = case shown="True" w3250 {
          tunnel: [w3257 w3262] -> w3253
          tunnel: w3252 -> [w3257 w3261]
          frame False {
          }
          frame True {
            n1499 = local read "Radio Buttons"() -> (w3260:T9)
            n1500 = Increment(x=w3260) -> (x+1=w3259:T9)
            n1501 = Number To Decimal String(number=w3259) -> (decimal integer string=w3258:string)  [unwired: 1 in]
            n1502 = call "TcpIDFGV.vi"("Error In"=w3261, "action"=enum16{"write", "read"}."read") -> ("Error Out"=w3263:errorcluster, "connection ID out"=w3266:refnum<k5>)  [unwired: 8 in]
            n1503 = Concatenate Strings("!channel:", w3258) -> (w3264:string)
            n1504 = call "TCP_WriteRead.vi"("error in (no error)"=w3263, "data in"=w3264, "connectin ID in"=w3266) -> ("error out"=w3262:errorcluster)  [unwired: 4 in, 2 out]
          }
        }
        n1505 = call <vilib>:"Add State(s) to Queue__JKI_lib_State_Machine.vi"("State(s) in (\"\")"=w3256) -> ("States Out"=w3255:string)  [unwired: 14 in]
      }
      frame "TCP: sendANSI" {
        # "Template Separator\n(You can make a copy of, or modify, this frame)"
        n1506 = Unbundle By Name(w3270) -> ("System Status.TCP/IP"=w3268:bool, "VideoConfig.ANSI"=w3269:dbl)
        n1507 = case shown="True" w3268 {
          tunnel: [w3276 w3282] -> w3272
          tunnel: w3271 -> [w3276 w3281]
          tunnel: w3269 -> [_ w3280]
          frame False {
          }
          frame True {
            n1508 = Number To Fractional String(number=w3280) -> (F-format string=w3278:string)  [unwired: 3 in]
            n1509 = call "TcpIDFGV.vi"("Error In"=w3281, "action"=enum16{"write", "read"}."read") -> ("Error Out"=w3283:errorcluster, "connection ID out"=w3284:refnum<k5>)  [unwired: 8 in]
            n1510 = Concatenate Strings("!ansi:" ("data in"), w3278) -> (w3277:string)
            n1511 = call "TCP_WriteRead.vi"("error in (no error)"=w3283, "data in"=w3277, "connectin ID in"=w3284) -> ("error out"=w3282:errorcluster)  [unwired: 4 in, 2 out]
          }
        }
        n1512 = call <vilib>:"Add State(s) to Queue__JKI_lib_State_Machine.vi"("State(s) in (\"\")"=w3275) -> ("States Out"=w3274:string)  [unwired: 14 in]
      }
      frame "TCP: sendRadius" {
        # "Send drawing radius to AB PC\n(You can make a copy of, or modify, this frame)"
        n1513 = Unbundle By Name(w3288) -> ("System Status.TCP/IP"=w3286:bool, "VideoConfig.Radius"=w3287:dbl)
        n1514 = case shown="True" w3286 {
          tunnel: [w3294 w3300] -> w3290
          tunnel: w3289 -> [w3294 w3299]
          tunnel: w3287 -> [_ w3298]
          frame False {
          }
          frame True {
            n1515 = Number To Fractional String(number=w3298) -> (F-format string=w3297:string)  [unwired: 3 in]
            n1516 = Concatenate Strings("!radius:" ("data in"), w3297) -> (w3295:string)
            n1517 = call "TcpIDFGV.vi"("Error In"=w3299, "action"=enum16{"write", "read"}."read") -> ("Error Out"=w3301:errorcluster, "connection ID out"=w3302:refnum<k5>)  [unwired: 8 in]
            n1518 = call "TCP_WriteRead.vi"("error in (no error)"=w3301, "data in"=w3295, "connectin ID in"=w3302) -> ("error out"=w3300:errorcluster)  [unwired: 4 in, 2 out]
          }
        }
        n1519 = call <vilib>:"Add State(s) to Queue__JKI_lib_State_Machine.vi"("State(s) in (\"\")"=w3293) -> ("States Out"=w3292:string)  [unwired: 14 in]
      }
      frame "TCP: send3Dsetting" {
        # "Send 3D setting to AB computer\n(You can make a copy of, or modify, this frame)"
        n1520 = Unbundle By Name(w3306) -> ("System Status.TCP/IP"=w3304:bool, "VideoConfig.3D?"=w3305:bool)
        n1521 = case shown="True" w3304 {
          tunnel: [w3312 w3319] -> w3308
          tunnel: w3307 -> [w3312 w3318]
          tunnel: w3305 -> [_ w3317]
          frame False {
          }
          frame True {
            n1522 = Boolean To (0,1)(Boolean=w3317) -> (0, 1=w3316:i16)
            n1523 = Number To Fractional String(number=w3316) -> (F-format string=w3315:string)  [unwired: 3 in]
            n1524 = call "TcpIDFGV.vi"("Error In"=w3318, "action"=enum16{"write", "read"}."read") -> ("Error Out"=w3320:errorcluster, "connection ID out"=w3321:refnum<k5>)  [unwired: 8 in]
            n1525 = Concatenate Strings("!3dset:" ("data in"), w3315) -> (w3313:string)
            n1526 = call "TCP_WriteRead.vi"("error in (no error)"=w3320, "data in"=w3313, "connectin ID in"=w3321) -> ("error out"=w3319:errorcluster)  [unwired: 4 in, 2 out]
          }
        }
        n1527 = call <vilib>:"Add State(s) to Queue__JKI_lib_State_Machine.vi"("State(s) in (\"\")"=w3311) -> ("States Out"=w3310:string)  [unwired: 14 in]
      }
      frame "TCP: sendFirefly" {
        # "Template Separator\n(You can make a copy of, or modify, this frame)"
        n1528 = Unbundle By Name(w3324) -> ("System Status.TCP/IP"=w3323:bool)
        n1529 = case shown="False" w3323 {
          tunnel: [w3330 w3332] -> w3326
          tunnel: w3325 -> [w3330 w3331]
          frame False {
          }
          frame True {
            n1530 = call "TcpIDFGV.vi"("Error In"=w3331, "action"=enum16{"write", "read"}."read") -> ("Error Out"=w3333:errorcluster, "connection ID out"=w3335:refnum<k5>)  [unwired: 8 in]
            n1531 = call "TCP_WriteRead.vi"("error in (no error)"=w3333, "data in"="!firefly:0", "connectin ID in"=w3335) -> ("error out"=w3332:errorcluster)  [unwired: 4 in, 2 out]
          }
        }
        n1532 = call <vilib>:"Add State(s) to Queue__JKI_lib_State_Machine.vi"("State(s) in (\"\")"=w3329) -> ("States Out"=w3328:string)  [unwired: 14 in]
      }
      frame "TCP: sendPentero" {
        # "Send Pentero setting to AB computer\n(You can make a copy of, or modify, this frame)"
        n1533 = Unbundle By Name(w3338) -> ("System Status.TCP/IP"=w3337:bool)
        n1534 = case shown="True" w3337 {
          tunnel: [w3344 w3346] -> w3340
          tunnel: w3339 -> [w3344 w3345]
          frame False {
          }
          frame True {
            n1535 = call "TcpIDFGV.vi"("Error In"=w3345, "action"=enum16{"write", "read"}."read") -> ("Error Out"=w3347:errorcluster, "connection ID out"=w3349:refnum<k5>)  [unwired: 8 in]
            n1536 = call "TCP_WriteRead.vi"("error in (no error)"=w3347, "data in"="!pentero:0", "connectin ID in"=w3349) -> ("error out"=w3346:errorcluster)  [unwired: 4 in, 2 out]
          }
        }
        n1537 = call <vilib>:"Add State(s) to Queue__JKI_lib_State_Machine.vi"("State(s) in (\"\")"=w3343) -> ("States Out"=w3342:string)  [unwired: 14 in]
      }
      frame "TCP: sendChannel" {
        # "Send DeCon Channel to AB computer\n()"
        n1538 = Unbundle By Name(w3352) -> ("System Status.TCP/IP"=w3351:bool)
        n1539 = case shown="True" w3351 {
          tunnel: [w3358 w3362] -> w3354
          tunnel: w3353 -> [w3358 w3361]
          frame False {
          }
          frame True {
            n1540 = local read "Radio Buttons"() -> (w3360:T9)
            n1541 = case shown="\"No Selection\", Default" w3360 {
              tunnel: ["" ("data in") "!channel:1" ("data in") "!channel:2" ("data in") "!channel:3" ("data in")] -> w3359
              frame "No Selection", Default {
              }
              frame "Ch1" {
              }
              frame "Ch2" {
              }
              frame "Ch3" {
              }
            }
            n1542 = call "TcpIDFGV.vi"("Error In"=w3361, "action"=enum16{"write", "read"}."read") -> ("Error Out"=w3363:errorcluster, "connection ID out"=w3364:refnum<k5>)  [unwired: 8 in]
            n1543 = call "TCP_WriteRead.vi"("error in (no error)"=w3363, "data in"=w3359, "connectin ID in"=w3364) -> ("error out"=w3362:errorcluster)  [unwired: 4 in, 2 out]
          }
        }
        n1544 = call <vilib>:"Add State(s) to Queue__JKI_lib_State_Machine.vi"("State(s) in (\"\")"=w3357) -> ("States Out"=w3356:string)  [unwired: 14 in]
      }
      frame "TCP: startCam" {
        # "Send Pentero setting to AB computer\n(You can make a copy of, or modify, this frame)"
        n1545 = Unbundle By Name(w3371) -> ("System Status.TCP/IP"=w3370:bool)
        n1546 = case shown="True" w3370 {
          tunnel: [w3377 w3379] -> w3373
          tunnel: w3372 -> [w3377 w3378]
          frame False {
          }
          frame True {
            n1547 = call "TcpIDFGV.vi"("Error In"=w3378, "action"=enum16{"write", "read"}."read") -> ("Error Out"=w3380:errorcluster, "connection ID out"=w3382:refnum<k5>)  [unwired: 8 in]
            n1548 = call "TCP_WriteRead.vi"("error in (no error)"=w3380, "data in"="!focus:1", "connectin ID in"=w3382) -> ("error out"=w3379:errorcluster)  [unwired: 4 in, 2 out]
          }
        }
        n1549 = call <vilib>:"Add State(s) to Queue__JKI_lib_State_Machine.vi"("State(s) in (\"\")"=w3376) -> ("States Out"=w3375:string)  [unwired: 14 in]
      }
      frame "TCP: stopCam" {
        # "Send Pentero setting to AB computer\n(You can make a copy of, or modify, this frame)"
        n1550 = Unbundle By Name(w3385) -> ("System Status.TCP/IP"=w3384:bool)
        n1551 = case shown="True" w3384 {
          tunnel: [w3391 w3393] -> w3387
          tunnel: w3386 -> [w3391 w3392]
          frame False {
          }
          frame True {
            n1552 = call "TcpIDFGV.vi"("Error In"=w3392, "action"=enum16{"write", "read"}."read") -> ("Error Out"=w3394:errorcluster, "connection ID out"=w3396:refnum<k5>)  [unwired: 8 in]
            n1553 = call "TCP_WriteRead.vi"("error in (no error)"=w3394, "data in"="!focus:0", "connectin ID in"=w3396) -> ("error out"=w3393:errorcluster)  [unwired: 4 in, 2 out]
          }
        }
        n1554 = call <vilib>:"Add State(s) to Queue__JKI_lib_State_Machine.vi"("State(s) in (\"\")"=w3390) -> ("States Out"=w3389:string)  [unwired: 14 in]
      }
      frame "TCP: Close" {
        # "Close TCP connection\n()"
        n1555 = Unbundle By Name(w3400) -> ("System Status.TCP/IP"=w3398:bool)
        n1556 = case shown="True" w3398 {
          tunnel: [w3406 w3408] -> w3401
          tunnel: w3399 -> [w3406 w3407]
          frame False {
          }
          frame True {
            n1557 = call "TcpIDFGV.vi"("Error In"=w3407, "action"=enum16{"write", "read"}."read") -> ("Error Out"=w3410:errorcluster, "connection ID out"=w3411:refnum<k5>)  [unwired: 8 in]
            n1558 = TCP Close Connection(connection ID=w3411, error in (no error)=w3410) -> (error out=w3408:errorcluster)  [unwired: 1 in, 1 out]
          }
        }
        n1559 = case shown="Error .." w3401 {
          tunnel: [w3414 w3415] -> w3402
          tunnel: w3400 -> [w3413 w3415]
          frame No Error {
            w3412 = FALSE ("System Status.TCP/IP")
            n1560 = Bundle By Name(cluster=w3413, "System Status.TCP/IP"=w3412) -> (w3414:T23)
            n1561 = global write "GlobalVariables.vi" "TCP connected?"(w3412) -> ()
          }
          frame Error {
          }
        }
        n1562 = call <vilib>:"Add State(s) to Queue__JKI_lib_State_Machine.vi"("State(s) in (\"\")"=w3405) -> ("States Out"=w3404:string)  [unwired: 14 in]
      }
      frame "---------- PID ----------" {
        # "Template Separator\n(You can make a copy of, or modify, this frame)"
        n1563 = call <vilib>:"Add State(s) to Queue__JKI_lib_State_Machine.vi"("State(s) in (\"\")"=w3420) -> ("States Out"=w3419:string)  [unwired: 14 in]
      }
      frame "PID: loadPID" {
        # "Template Separator\n(You can make a copy of, or modify, this frame)"
        n1564 = call "readPIDSetting.vi"("Error In"=w3424) -> ("Error Out"=w3425:errorcluster, "Ch3 PID out"=w3421:T8, "Ch2 PID out"=w3422:T8, "Ch1 PID out"=w3423:T8)  [unwired: 7 in]
        n1565 = local write "Ch1 PID gains"(w3423) -> ()
        n1566 = local write "Ch2 PID gains"(w3422) -> ()
        n1567 = local write "Ch3 PID gains"(w3421) -> ()
        n1568 = local write "Ch4 PID gains"(w3421) -> ()
        n1569 = call <vilib>:"Add State(s) to Queue__JKI_lib_State_Machine.vi"("State(s) in (\"\")"=w3429) -> ("States Out"=w3428:string)  [unwired: 14 in]
      }
      frame "---------- Classifier ----------" {
        # "Template Separator\n(You can make a copy of, or modify, this frame)"
        n1570 = call <vilib>:"Add State(s) to Queue__JKI_lib_State_Machine.vi"("State(s) in (\"\")"=w3434) -> ("States Out"=w3433:string)  [unwired: 14 in]
      }
      frame "Classifier: Init" {
        # "Initilize Python\n(You can make a copy of, or modify, this frame)"
        n1571 = call-poly <vilib>:"Open Virtual Environment Session.vi"("error in (no error)"=w3443, "Anaconda path"=path "C:/ProgramData/miniconda3", "Python version"="Python version", "Env name"="Env name") -> ("error out"=w3439:errorcluster, "session out"=w3442:refnum<k35>)  [unwired: 6 in]
        n1572 = Path To String(path="model path") -> (string=w3436:string)
        n1573 = node "Python Node"(w3442, "module path", "load_model" ("function name"), w3439, w3436) -> (→"Python session":refnum<k35>, w3438:errorcluster)  [unwired: 3 in, 2 out]
        n1574 = call <vilib>:"Add State(s) to Queue__JKI_lib_State_Machine.vi"("State(s) in (\"\")"=w3450) -> ("States Out"=w3449:string)  [unwired: 14 in]
      }
      frame "Classifier: Close" {
        # "Template Separator\n(You can make a copy of, or modify, this frame)"
        n1575 = local read "Python session"() -> (w3454:refnum<k35>)
        n1576 = Close Python Session(session in=w3454, error in=w3453) -> (11:w3452:errorcluster)
        n1577 = case shown="Error .." w3452 {
          selector: w3452 -> [w3459 _]
          tunnel: [w3459 errorcluster {"status"=FALSE, "code"=0, "source"=""} ("error IO")] -> w3451
          frame No Error {
          }
          frame Error {
          }
        }
        n1578 = call <vilib>:"Add State(s) to Queue__JKI_lib_State_Machine.vi"("State(s) in (\"\")"=w3458) -> ("States Out"=w3457:string)  [unwired: 14 in]
      }
      frame "---------- Temp ----------" {
        # "Template Separator\n(You can make a copy of, or modify, this frame)"
        n1579 = call <vilib>:"Add State(s) to Queue__JKI_lib_State_Machine.vi"("State(s) in (\"\")"=w3465) -> ("States Out"=w3464:string)  [unwired: 14 in]
      }
      frame "Temp: KeepEmpty" {
        # "Template Separator\n(You can make a copy of, or modify, this frame)"
        n1580 = call <vilib>:"Add State(s) to Queue__JKI_lib_State_Machine.vi"("State(s) in (\"\")"=w3470) -> ("States Out"=w3469:string)  [unwired: 14 in]
      }
    }
    n1581 = Not(x=w80) -> (.not. x?=w79:bool)
    n1582 = local write "ML?"(w79) -> ()
    "ML?" <- TRUE ("main loop running?")
  }
  n1583 = while {
    tunnel: w19 -> [w3504]
    tunnel: w18 -> [w3473]
    tunnel: [w3472] -> w17
    tunnel: w13 -> [w3500]
    tunnel: [w3499] -> w16
    shift-right: [w3495] -> _
    shift-left: _ -> [w3496]
    stop <- w3475 stop-if-true
    # "Read data from notifier and deconvolve it and send to Aiming Beam computer"
    n1584 = Wait on Notification(notifier=w3504, ignore previous (F)=FALSE) -> (notification=w3491:T14, error out=w3475:errorcluster)  [unwired: 2 in, 2 out]
    n1585 = local read "Data Class"() -> (w3476:enum16{"Data", "BG", "Cali"})
    n1586 = Unbundle(w3491) -> ("idx"=w3474:i32, "CH1&2"=w3503:dbl[][], "CH3&4"=w3502:dbl[][], "V cluster"=w3481:cluster{"V1":dbl, "V2":dbl, "V3":dbl, "V4":dbl})
    n1587 = call "SeperateChanData.vi"("Input (Ch1&2)"=w3502) -> ("Ch1"=w3478:dbl[][], "Ch2"=w3486:dbl[][])
    n1588 = call "SeperateChanData.vi"("Input (Ch1&2)"=w3503) -> ("Ch1"=w3480:dbl[][], "Ch2"=w3479:dbl[][])
    n1589 = case shown="\"Data\"" w3476 {
      tunnel: w3481 -> [w3516 _]
      tunnel: w3480 -> [w3515 _]
      tunnel: w3479 -> [w3514 _]
      tunnel: w3478 -> [w3513 _]
      tunnel: w3475 -> [w3512 w3624]
      tunnel: w3474 -> [w3511 _]
      tunnel: w3473 -> [w3509 w3625]
      tunnel: [w3506 w3625] -> w3472
      tunnel: [w3505 w3624] -> w3471
      frame "Data" {
        # "If acquiring data"
        n1590 = case shown="1, 2" "Overlay selection" {
          tunnel: "Radio Buttons" -> [w3520 _]
          tunnel: [w3521 w3544] -> w3507
          tunnel: w3512 -> [w3521 w3543]
          tunnel: [w3519 w3531] -> w3510
          tunnel: w3516 -> [_ w3550]
          tunnel: w3515 -> [_ w3547]
          tunnel: w3514 -> [_ w3546]
          tunnel: w3513 -> [_ w3545]
          frame 0, Default {
            # "overlay gain"
            n1591 = case shown="\"Ch4\"" w3520 {
              tunnel: [0.0 ("Gain1") w3523 w3524 w3525 w3526] -> w3519
              frame "No Selection", Default {
              }
              frame "Ch1" {
                n1592 = local read "Gain1"() -> (w3523:dbl)
              }
              frame "Ch2" {
                n1593 = local read "Gain2"() -> (w3524:dbl)
              }
              frame "Ch3" {
                n1594 = local read "Gain3"() -> (w3525:dbl)
              }
              frame "Ch4" {
                n1595 = local read "Gain4"() -> (w3526:dbl)
              }
            }
          }
          frame 1, 2 {
            # "overlay lifetime or cancer probability"
            n1596 = call "DeConAPD2FGV.vi"("Error In"=w3543) -> ("Error Out"=w3549:errorcluster, "APDClass out"=w3540:T40)  [unwired: 9 in]
            n1597 = call "DeConAPD1FGV.vi"("Error In"=w3543) -> ("Error Out"=w3551:errorcluster, "APDClass out"=w3542:T40)  [unwired: 9 in]
            n1598 = call "DeConAPD3FGV.vi"("Error In"=w3543) -> ("Error Out"=w3548:errorcluster, "APDClass out"=w3538:T40)  [unwired: 9 in]
            n1599 = Unbundle By Name(w3550) -> ("V1"=w3541:dbl, "V2"=w3539:dbl, "V3"=w3537:dbl)
            n1600 = call "getGain.vi"("CtrlV"=w3537, "APD"=w3538) -> ("gain"=w3528:dbl)  [unwired: 8 in, 1 out]
            n1601 = call "getGain.vi"("CtrlV"=w3541, "APD"=w3542) -> ("gain"=w3530:dbl)  [unwired: 8 in, 1 out]
            n1602 = call "getGain.vi"("CtrlV"=w3539, "APD"=w3540) -> ("gain"=w3529:dbl)  [unwired: 8 in, 1 out]
            n1603 = Less?(x=w3530, y="Ch1GainLim") -> (x < y?=w3535:bool)
            n1604 = Less?(x=w3529, y="Ch2&3GainLim") -> (x < y?=w3534:bool)
            n1605 = Less?(x=w3528, y="Ch2&3GainLim") -> (x < y?=w3533:bool)
            n1606 = Compound Arithmetic op=AND(w3535, w3534, w3533) -> (w3532:bool)
            n1607 = case shown="True" w3532 {
              tunnel: w3551 -> [_ w3614]
              tunnel: w3549 -> [_ w3613]
              tunnel: w3548 -> [_ w3612]
              tunnel: w3547 -> [_ w3602]
              tunnel: w3546 -> [_ w3601]
              tunnel: w3545 -> [_ w3600]
              tunnel: [w3552 w3561] -> w3544
              tunnel: w3543 -> [w3552 w3593]
              tunnel: w3542 -> [_ w3592]
              tunnel: w3541 -> [_ w3591]
              tunnel: w3540 -> [_ w3590]
              tunnel: w3539 -> [_ w3589]
              tunnel: w3538 -> [_ w3588]
              tunnel: w3537 -> [_ w3587]
              tunnel: [0.0 ("Gain4") w3554] -> w3531
              tunnel: w3530 -> [_ w3579]
              tunnel: w3529 -> [_ w3578]
              tunnel: w3528 -> [_ w3577]
              frame False {
                # "give probability of 0.5"
                # "if gain is out of acceptable range"
              }
              frame True {
                # "if gain is within range"
                n1608 = Build Array(w3579, w3578, w3577) -> (w3576:dbl[])
                n1609 = call "getIrf (SubVI).vi"("error in"=w3614, "CtrlV"=w3591, "APD"=w3592) -> ("error out"=w3606:errorcluster, "irfTNorm"=w3609:dbl[])  [unwired: 6 in, 1 out]
                n1610 = call "getIrf (SubVI).vi"("error in"=w3613, "CtrlV"=w3589, "APD"=w3590) -> ("error out"=w3605:errorcluster, "irfTNorm"=w3608:dbl[])  [unwired: 6 in, 1 out]
                n1611 = call "getIrf (SubVI).vi"("error in"=w3612, "CtrlV"=w3587, "APD"=w3588) -> ("error out"=w3604:errorcluster, "irfTNorm"=w3607:dbl[])  [unwired: 6 in, 1 out]
                n1612 = call "DotNetFGV.vi"("Error In"=w3593) -> ("Error Out"=w3597:errorcluster, "reference out"=w3598:refnum<k24>)  [unwired: 9 in]
                n1613 = local read "BGAll"() -> (w3611:dbl[][])
                n1614 = Merge Errors(w3597, w3606, w3605, w3604) -> (w3603:errorcluster)
                n1615 = Build Array(w3609, w3608, w3607) -> (w3594:dbl[][])
                n1616 = Build Array (concatenate)(w3602, w3601, w3600) -> (w3599:dbl[][])
                n1617 = local write "iRF Graph"(w3594) -> ()
                n1618 = Transpose 2D Array(2D array=w3611) -> (transposed array=w3610:dbl[][])
                n1619 = Transpose 2D Array(2D array=w3594) -> (transposed array=w3595:dbl[][])
                n1620 = Transpose 2D Array(2D array=w3599) -> (transposed array=w3596:dbl[][])
                n1621 = Reciprocal(x=w3576) -> (1/x=w3574:dbl[])
                n1622 = call "LagDeConAllCh (SubVI).vi"("new reference"=w3598, "error in (no error)"=w3603, "irf"=w3595, "BG"=w3610, "WF"=w3596) -> ("error out"=w3562:errorcluster, "LCs"=w3570:dbl[][], "INTs"=w3581:dbl[][], "LTs"=w3586:dbl[][])  [unwired: 3 in]
                n1623 = Index Array(array=w3586, index (col)=0 ("disabled index (col)")) -> (element=w3568:dbl[])  [unwired: 1 in]
                n1624 = Index Array(array=w3581, index (col)=0 ("disabled index (col)")) -> (element=w3575:dbl[])  [unwired: 1 in]
                n1625 = Multiply(x=w3575, y=w3574) -> (x*y=w3573:dbl[])
                n1626 = Index Array(array=w3570, index (col)=0 ("disabled index (col)")) -> (element=w3566:dbl[])  [unwired: 1 in]
                n1627 = Add Array Elements(numeric array=w3573) -> (sum=w3572:dbl)
                n1628 = Index Array(array=w3568, index=0) -> (element=w3558:dbl)
                "Ch1 Lifetime (ns)" <- w3558
                n1629 = Index Array(array=w3568, index=1) -> (element=w3557:dbl)
                "Ch2 Lifetime (ns)" <- w3557
                n1630 = Index Array(array=w3568, index=2) -> (element=w3556:dbl)
                "Ch3 Lifetime (ns)" <- w3556
                n1631 = Divide(x=w3573, y=w3572) -> (x/y=w3567:dbl[])
                n1632 = Bundle(w3558, w3557, w3556) -> (→"Lifetime (ns)":cluster{dbl, dbl, dbl})  [unwired: 1 in]
                n1633 = Build Array (concatenate)(w3568, w3567, w3566) -> (w3559:dbl[])
                "DeConOut" <- w3559
                n1634 = local read "module path"() -> (w3564:path)
                n1635 = local read "Python session"() -> (w3565:refnum<k35>)
                n1636 = node(w3565, w3564, "HNPredict" ("function name"), w3562, 0.0, w3559) -> (w3561:errorcluster, w3555:dbl)  [unwired: 1 in, 3 out]
                "Cancer Prob" <- w3555
                n1637 = disable-structure shown="Enabled" {
                  disable-tunnel: w3555 -> [w3617 w3622]
                  disable-tunnel: [w3616 w3618] -> w3554
                  frame Disabled {
                    n1638 = Add(x=0.01, y=w3617) -> (x+y=w3616:dbl)
                  }
                  frame Enabled {
                    n1639 = Greater?(x=w3622, y="CancerThreshold") -> (0:w3623:bool)
                    n1640 = Select(t=1.0, s=w3623, f=0.01) -> (s? t:f=w3618:dbl)
                  }
                }
              }
            }
          }
        }
        n1641 = Bundle("idx"=w3511, "f"=w3510) -> (w3508:cluster{"idx":i32, "f":dbl})  [unwired: 1 in]
        n1642 = Send Notification(notification=w3508, notifier=w3509, error in (no error)=w3507) -> (notifier out=w3506:refnum<notifier>, error out=w3505:errorcluster)
      }
      frame "BG", Default {
        # "if not acquiting data"
      }
    }
    n1643 = call "AvgArrayTimeCritical.vi"("2D array"=w3480) -> ("1D Avg"=w3487:dbl[])  [unwired: 10 in]
    n1644 = call "AvgArrayTimeCritical.vi"("2D array"=w3479) -> ("1D Avg"=w3488:dbl[])  [unwired: 10 in]
    n1645 = call "AvgArrayTimeCritical.vi"("2D array"=w3478) -> ("1D Avg"=w3489:dbl[])  [unwired: 10 in]
    n1646 = call "AvgArrayTimeCritical.vi"("2D array"=w3486) -> ("1D Avg"=w3490:dbl[])  [unwired: 10 in]
    n1647 = Build Array(w3490) -> (w3485:dbl[][])
    n1648 = Build Array(w3489) -> (w3484:dbl[][])
    n1649 = Build Array(w3488) -> (w3483:dbl[][])
    n1650 = Build Array(w3487) -> (w3482:dbl[][])
    n1651 = flat-sequence {
      tunnel: [w3626] -> w3495
      tunnel: w3475 -> [_]
      frame #0 {
        n1652 = call <vilib>:"High Resolution Relative Seconds.vi"() -> ("relative seconds"=w3626:dbl)
      }
    }
    n1653 = Subtract(x=w3495, y=w3496) -> (x-y=w3498:dbl)
    n1654 = Multiply(x=w3498, y=1000.0) -> (x*y=→"Decon Loop timing (ms)" →"DeCon Speed(ms)":dbl)
    n1655 = Bundle(w3482, w3483, w3484, w3485, "V cluster"=w3481) -> (w3501:T48)  [unwired: 1 in]
    n1656 = Send Notification(notification=w3501, notifier=w3500, error in (no error)=w3475) -> (notifier out=w3499:refnum<notifier>, error out=w3477:errorcluster)
    n1657 = Merge Errors(w3471, w3477) -> (→"decon error out":errorcluster)
  }
  n1658 = while {
    tunnel: w18 -> [w3638]
    shift-right: [w3631] -> _
    shift-left: u32 0 -> [w3632]
    stop <- w3629 stop-if-true
    # "Send data to AB computer here"
    # "if TCP ip is not open loop will run once and stop. To re-establish connection and start this loop. Reboot softwrae."
    # "Data communication loop"
    n1659 = Wait on Notification(notifier=w3638, ignore previous (F)=FALSE) -> (notification=w3636:cluster{"idx":i32, "lifetime":dbl}, error out=w3630:errorcluster)  [unwired: 2 in, 2 out]
    n1660 = Wait Until Next ms Multiple(millisecond multiple=u32 25) -> ()  [unwired: 1 out]
    n1661 = Unbundle(w3636) -> ("idx"=w3635:i32, "lifetime"=w3634:dbl)
    n1662 = Tick Count (ms)() -> (millisecond timer value=w3631:u32)
    n1663 = global read "GlobalVariables.vi" "TCP connected?"() -> (w3628:bool)
    n1664 = Subtract(x=w3631, y=w3632) -> (x-y=→"Communication loop(ms)":u32)
    n1665 = case shown="True" w3628 {
      tunnel: w3635 -> [_ w3647]
      tunnel: w3634 -> [_ w3646]
      tunnel: w3630 -> [w3639 w3643]
      tunnel: [w3639 w3640] -> w3629
      frame False {
      }
      frame True {
        n1666 = Number To Decimal String(number=w3647) -> (decimal integer string=w3655:string)  [unwired: 1 in]
        n1667 = call "TcpIDFGV.vi"("Error In"=w3643, "action"=enum16{"write", "read"}."read") -> ("Error Out"=w3642:errorcluster, "connection ID out"=w3653:refnum<k5>)  [unwired: 8 in]
        n1668 = Concatenate Strings("!idx:", w3655) -> (w3656:string)
        n1669 = call "TCP_WriteRead.vi"("error in (no error)"=w3642, "data in"=w3656, "connectin ID in"=w3653) -> ("error out"=w3641:errorcluster, "connectin ID out"=w3654:refnum<k5>)  [unwired: 4 in, 1 out]
        n1670 = Number To Fractional String(number=w3646, precision (6)=i16 2) -> (F-format string=w3645:string)  [unwired: 2 in]
        n1671 = Concatenate Strings("!lifetime:", w3645) -> (w3652:string)
        n1672 = call "TCP_WriteRead.vi"("error in (no error)"=w3641, "data in"=w3652, "connectin ID in"=w3654) -> ("error out"=w3640:errorcluster, "data out"=→"data out(communcation loop)":string)  [unwired: 4 in, 1 out]
      }
    }
  }
  n1673 = while {
    tunnel: w13 -> [w3667]
    shift-right: [w3658] -> _
    shift-left: w15 -> [w3665]
    shift-right: [w3660] -> _
    shift-left: w15 -> [w3659]
    i -> [w3661]
    stop <- w3662 stop-if-true
    # "Data display loop(30Hz)"
    n1674 = Wait on Notification(notifier=w3667, ignore previous (F)=FALSE) -> (notification=w3663:T13, error out=w3662:errorcluster)  [unwired: 2 in, 2 out]
    n1675 = Wait Until Next ms Multiple(millisecond multiple=u32 40) -> ()  [unwired: 1 out]
    n1676 = Tick Count (ms)() -> (millisecond timer value=w3658:u32)
    n1677 = Subtract(x=w3658, y=w3665) -> (x-y=→"display loop timing(ms)":u32)
    n1678 = case shown="No Error" w3662 {
      tunnel: w3663 -> [w3740 _]
      tunnel: w3659 -> [w3712 w3812]
      tunnel: [w3714 w3812] -> w3660
      tunnel: w3658 -> [w3711 _]
      frame No Error {
        w3669 = u32 1 ("Active Plot")
        w3688 = 0 ("index (row)")
        n1679 = Subtract(x=w3711, y=w3712) -> (x-y=w3713:u32)
        n1680 = Unbundle(w3740) -> ("CH1"=w3735:dbl[][], "CH2"=w3733:dbl[][], "CH3"=w3730:dbl[][], "CH4"=w3683:dbl[][], "Gain cluster"=w3689:cluster{"V1":dbl, "V2":dbl, "V3":dbl, "V4":dbl})
        n1681 = Unbundle By Name(w3689) -> ("V1"=w3707:dbl, "V2"=w3705:dbl, "V3"=w3703:dbl, "V4"=w3681:dbl)
        n1682 = Index Array(array=w3735, index (row)=w3688) -> (element=w3719:dbl[])  [unwired: 1 in]
        n1683 = Index Array(array=w3733, index (row)=w3688) -> (element=w3717:dbl[])  [unwired: 1 in]
        n1684 = Index Array(array=w3730, index (row)=w3688) -> (element=w3718:dbl[])  [unwired: 1 in]
        n1685 = Index Array(array=w3683, index (row)=w3688) -> (element=w3687:dbl[])  [unwired: 1 in]
        n1686 = call "RemoveDCBG.vi"("Channel"=enum16{"DC Only", "Ch1", "Ch2", "Ch3", "Ch4"}."Ch4", "WF in"=w3687) -> ("DC"=w3685:dbl, "WF out"=w3674:dbl[])  [unwired: 7 in, 1 out]
        n1687 = Greater?(x=w3713, y=u32 200) -> (0:w3715:bool)
        n1688 = call "CtrlVtoGain.vi"("CtrlV(V)"=w3681, "Channel"=enum16{"Ch1", "Ch2", "Ch3", "Ch4"}."Ch4") -> ("Gain"=w3673:dbl)  [unwired: 8 in, 1 out]
        n1689 = call "CtrlVtoGain.vi"("CtrlV(V)"=w3707, "Channel"=enum16{"Ch1", "Ch2", "Ch3"}."Ch1") -> ("Gain"=w3701:dbl)  [unwired: 8 in, 1 out]
        n1690 = call "RemoveDCBG.vi"("Channel"=enum16{"DC Only", "Ch1", "Ch2", "Ch3"}."Ch1", "WF in"=w3719) -> ("DC"=w3736:dbl, "WF out"=w3708:dbl[])  [unwired: 7 in, 1 out]
        n1691 = call "RemoveDCBG.vi"("Channel"=enum16{"DC Only", "Ch1", "Ch2", "Ch3"}."Ch2", "WF in"=w3717) -> ("DC"=w3732:dbl, "WF out"=w3709:dbl[])  [unwired: 7 in, 1 out]
        n1692 = call "CtrlVtoGain.vi"("CtrlV(V)"=w3705, "Channel"=enum16{"Ch1", "Ch2", "Ch3"}."Ch2") -> ("Gain"=w3696:dbl)  [unwired: 8 in, 1 out]
        n1693 = call "RemoveDCBG.vi"("Channel"=enum16{"DC Only", "Ch1", "Ch2", "Ch3"}."Ch3", "WF in"=w3718) -> ("DC"=w3729:dbl, "WF out"=w3710:dbl[])  [unwired: 7 in, 1 out]
        n1694 = call "CtrlVtoGain.vi"("CtrlV(V)"=w3703, "Channel"=enum16{"Ch1", "Ch2", "Ch3"}."Ch3") -> ("Gain"=w3692:dbl)  [unwired: 8 in, 1 out]
        n1695 = formula code="int32 out = 2;\nif (G<5){\nout = 1;\n}\nif (G>200){\nout = 3;\n}"("G"=w3673) -> ("out"=→"output variable":i32)
        n1696 = Add(x=w3674, y=w3685) -> (x+y=w3684:dbl[])
        n1697 = Less?(x=w3673, y=5.0) -> (x < y?=w3679:bool)
        n1698 = case shown="True" w3715 {
          tunnel: w3708 -> [_ w3769]
          tunnel: w3709 -> [_ w3772]
          tunnel: w3710 -> [_ w3771]
          tunnel: w3711 -> [_ w3787]
          tunnel: [w3751 w3787] -> w3714
          tunnel: w3712 -> [w3751 _]
          tunnel: w3701 -> [_ w3765]
          tunnel: w3696 -> [_ w3764]
          tunnel: w3692 -> [_ w3763]
          tunnel: w3674 -> [_ w3759]
          tunnel: w3673 -> [_ w3756]
          frame False {
          }
          frame True {
            n1699 = call "GetSNR(SubVI).vi"("Waveform"=w3769) -> ("SNR"=→"SNR1":dbl)  [unwired: 10 in]
            n1700 = Array Size(array=w3769) -> (size(s)=w3770:i32)
            n1701 = call "GetSNR(SubVI).vi"("Waveform"=w3772) -> ("SNR"=→"SNR2":dbl)  [unwired: 10 in]
            n1702 = call "GetSNR(SubVI).vi"("Waveform"=w3771) -> ("SNR"=→"SNR3":dbl)  [unwired: 10 in]
            n1703 = call "GetSNR(SubVI).vi"("Waveform"=w3759) -> ("SNR"=→"SNR4":dbl)  [unwired: 10 in]
            n1704 = global read "GlobalVariables.vi" "BG Idx2"() -> (w3758:i32)
            n1705 = Subtract(x=w3770, y=w3758) -> (x-y=w3757:i32)
            n1706 = Array Subset(array=w3769, index=w3758, length=w3757) -> (w3776:dbl[])
            n1707 = Array Subset(array=w3772, index=w3758, length=w3757) -> (w3778:dbl[])
            n1708 = Array Subset(array=w3771, index=w3758, length=w3757) -> (w3780:dbl[])
            n1709 = Array Subset(array=w3759, index=w3758, length=w3757) -> (w3760:dbl[])
            n1710 = Add Array Elements(numeric array=w3776) -> (sum=w3777:dbl)
            n1711 = Add Array Elements(numeric array=w3778) -> (sum=w3779:dbl)
            n1712 = Add Array Elements(numeric array=w3780) -> (sum=w3781:dbl)
            n1713 = Add Array Elements(numeric array=w3760) -> (sum=w3761:dbl)
            n1714 = Divide(x=w3777, y=w3765) -> (x/y=w3782:dbl)
            n1715 = Divide(x=w3779, y=w3764) -> (x/y=w3783:dbl)
            n1716 = Divide(x=w3781, y=w3763) -> (x/y=w3784:dbl)
            n1717 = Divide(x=w3761, y=w3756) -> (x/y=w3755:dbl)
            n1718 = Build Array(w3782, w3783, w3784, w3755) -> (w3785:dbl[])
            n1719 = Add Array Elements(numeric array=w3785) -> (sum=w3786:dbl)
            n1720 = Divide(x=w3785, y=w3786) -> (x/y=w3754:dbl[])
            n1721 = Index Array(array=w3754, index=2) -> (element=→"IntR3":dbl)
            n1722 = Index Array(array=w3754, index=1) -> (element=→"IntR2":dbl)
            n1723 = Index Array(array=w3754, index=0) -> (element=→"IntR1":dbl)
            n1724 = Index Array(array=w3754, index=3) -> (element=→"IntR4":dbl)
          }
        }
        n1725 = Add(x=w3708, y=w3736) -> (x+y=w3734:dbl[])
        n1726 = Add(x=w3709, y=w3732) -> (x+y=w3731:dbl[])
        n1727 = Add(x=w3710, y=w3729) -> (x+y=w3728:dbl[])
        n1728 = Less?(x=w3701, y=5.0 ("x")) -> (x < y?=w3699:bool)
        n1729 = Less?(x=w3696, y=5.0 ("x")) -> (x < y?=w3695:bool)
        n1730 = Less?(x=w3692, y=5.0 ("x")) -> (x < y?=w3691:bool)
        n1731 = case shown="False" w3691 {
          tunnel: [u32 16448250 ("Plot.Plot Color") u32 16711680 ("Plot.Plot Color")] -> w3690
          frame False {
          }
          frame True {
          }
        }
        n1732 = case shown="True" "Show BG removed?" {
          tunnel: w3735 -> [w3794 w3810]
          tunnel: w3734 -> [_ w3800]
          tunnel: [w3794 w3809] -> w3727
          tunnel: w3733 -> [w3793 w3808]
          tunnel: [w3793 w3807] -> w3671
          tunnel: w3731 -> [_ w3796]
          tunnel: w3730 -> [w3792 w3806]
          tunnel: [w3792 w3805] -> w3722
          tunnel: w3728 -> [_ w3801]
          tunnel: [w3791 w3804] -> w3678
          tunnel: w3684 -> [_ w3798]
          tunnel: w3683 -> [w3791 w3803]
          frame False {
          }
          frame True {
            n1733 = Insert Into Array(array=w3806, index (row)=1, new element=w3801) -> (w3805:dbl[][])  [unwired: 1 in]
            n1734 = Insert Into Array(array=w3810, index (row)=1, new element=w3800) -> (w3809:dbl[][])  [unwired: 1 in]
            n1735 = Insert Into Array(array=w3808, index (row)=1, new element=w3796) -> (w3807:dbl[][])  [unwired: 1 in]
            n1736 = Insert Into Array(array=w3803, index (row)=1, new element=w3798) -> (w3804:dbl[][])  [unwired: 1 in]
          }
        }
        "Channel 1" <- w3727
        "Channel 2" <- w3671
        "Channel 3" <- w3722
        "Channel 4" <- w3678
        n1737 = case shown="False" w3699 {
          tunnel: [u32 16448250 ("Plot.Plot Color") u32 16711680 ("Plot.Plot Color")] -> w3698
          frame False {
          }
          frame True {
          }
        }
        n1738 = case shown="False" w3695 {
          tunnel: [u32 16448250 ("Plot.Plot Color") u32 16711680 ("Plot.Plot Color")] -> w3694
          frame False {
          }
          frame True {
          }
        }
        n1739 = case shown="False" w3679 {
          tunnel: [u32 16448250 ("Plot.Plot Color") u32 16711680 ("Plot.Plot Color")] -> w3675
          frame False {
          }
          frame True {
          }
        }
        n1740 = case shown="False" "Show BG removed?" {
          tunnel: [u32 16744703 ("Plot.Plot Color") u32 16741120 ("Plot.Plot Color")] -> w3668
          frame False {
          }
          frame True {
          }
        }
        n1741 = property on="Channel 1" class="WFGraph (strict)"("Active Plot"=w3669, "Plot.Plot Color"=w3668, "Plot.Line Style"=u8 1, "Plot.Line Width"=u8 2, "BG Color"=w3698) -> ()  [unwired: 2 in, 2 out]
        n1742 = property on="Channel 2" class="WFGraph (strict)"("Active Plot"=w3669, "Plot.Plot Color"=w3668, "Plot.Line Style"=u8 1, "Plot.Line Width"=u8 2, "BG Color"=w3694) -> ()  [unwired: 2 in, 2 out]
        n1743 = property on="Channel 4" class="WFGraph (strict)"("Active Plot"=w3669, "Plot.Plot Color"=w3668, "Plot.Line Style"=u8 1, "Plot.Line Width"=u8 2, "BG Color"=w3675) -> ()  [unwired: 2 in, 2 out]
        n1744 = property on="Channel 3" class="WFGraph (strict)"("Active Plot"=w3669, "Plot.Plot Color"=w3668, "Plot.Line Style"=u8 1, "Plot.Line Width"=u8 2, "BG Color"=w3690) -> ()  [unwired: 2 in, 2 out]
      }
      frame Error {
        w3811 = u32 16448250 ("Plot Area:Colors:BG Color")
        n1745 = property on="Channel 1" class="WFGraph (strict)"("BG Color"=w3811) -> ()  [unwired: 2 in, 2 out]
        n1746 = property on="Channel 2" class="WFGraph (strict)"("BG Color"=w3811) -> ()  [unwired: 2 in, 2 out]
        n1747 = property on="Channel 3" class="WFGraph (strict)"("BG Color"=w3811) -> ()  [unwired: 2 in, 2 out]
      }
    }
    "DisplayLoop" <- w3661
  }
  n1748 = while {
    tunnel: w65 -> [w3825]
    tunnel: w55 -> [w3824]
    tunnel: [w3823] -> w63
    tunnel: w19 -> [w3822]
    tunnel: [w3821] -> w59
    tunnel: w39 -> [w3819]
    tunnel: w48 -> [w3818]
    tunnel: w35 -> [w3813]
    stop <- w3816 stop-if-true
    # "acquire data and send it to processing loop"
    # "Data Aquisition Loop"
    n1749 = event shown="[1] <Start digitizer>: User Event" {
      selector: w3824 -> [_ _]
      dyn-events: [_ _] -> w3823
      timeout: 30 -> [_ _]
      tunnel: w3825 -> [w3831 w3841]
      tunnel: [w3826 _] -> w3816
      tunnel: w3822 -> [w3830 w3848]
      tunnel: [w3830 w3847] -> w3821
      tunnel: w3819 -> [_ w3845]
      tunnel: w3818 -> [w3829 w3840]
      tunnel: w3813 -> [_ w3838]
      event Timeout {
        # "use queue to stop data loop\nwhen queue ref is released, error will stop this loop"
        n1750 = event-data() -> ()  [unwired: 1 in, 3 out]
        n1751 = Get Queue Status(queue=w3831) -> (error out=w3828:errorcluster)  [unwired: 2 in, 7 out]
        n1752 = Get Queue Status(queue=w3829) -> (error out=w3827:errorcluster)  [unwired: 2 in, 7 out]
        n1753 = Merge Errors(w3828, w3827) -> (w3826:errorcluster)
      }
      event User Event {
        w3846 = enum16{"Write", "Read"}."Read" ("Operation")
        n1754 = event-data() -> ("Time"=→"RunStartTime":u32)  [unwired: 1 in, 3 out]
        n1755 = call "FLImDAQ_FGV.vi"() -> ("Read data"=w3843:T5)  [unwired: 10 in, 1 out]
        n1756 = call "Digitizer1_FGV.vi"("Operation (Read)"=w3846) -> ("Read data"=w3837:refnum<k15>)  [unwired: 9 in, 1 out]
        n1757 = call "Digitizer2_FGV.vi"("Operation (Read)"=w3846) -> ("Read data"=w3844:refnum<k15>)  [unwired: 9 in, 1 out]
        n1758 = Unbundle By Name(w3843) -> ("Waveform to Avg"=w3842:i16)
        n1759 = property on="Property Node" class="niScope"(reference=w3837) -> (reference out=w3836:refnum<k15>, "Vertical Range"=w3835:dbl, "Vertical Offset"=w3834:dbl)  [unwired: 1 in, 1 out]
        n1760 = Tick Count (ms)() -> (millisecond timer value=w3833:u32)
        n1761 = while {
          tunnel: w3848 -> [w3908]
          tunnel: [w3907] -> w3847
          tunnel: w3844 -> [w3901]
          tunnel: w3836 -> [w3900]
          tunnel: w3845 -> [w3899]
          shift-right: [w3868] -> _
          shift-left: u32 0 ("millisecond timer value") -> [w3893]
          tunnel: w3842 -> [w3849]
          tunnel: w3841 -> [w3890]
          tunnel: w3840 -> [w3888]
          tunnel: w3838 -> [w3881]
          tunnel: w3835 -> [w3878]
          tunnel: w3834 -> [w3879]
          shift-right: [w3873] -> _
          shift-left: w3833 -> [w3872]
          i -> [w3850]
          stop <- w3871 stop-if-true
          w3861 = enum16{"write", "read"}."read" ("action")
          w3894 = 65536
          # "enqueue V"
          # "enqueue ch3 data"
          # "enqueue ch1&2 data"
          # "acquire ch3"
          # "acquire ch1&2"
          # "send data for processing"
          n1762 = Multiply(x=w3849, y=w3850) -> (x*y=w3858:i32)
          "Fetch Record #" <- w3858
          n1763 = property on="Property Node" class="niScope"(reference=w3900, "Fetch Record Number"=w3858) -> (reference out=w3912:refnum<k15>, error out=w3911:errorcluster, "Records Done"=w3880:i32)  [unwired: 1 in]
          n1764 = Subtract(x=w3880, y=w3858) -> (x-y=→"Record Backlog":i32)
          n1765 = call-poly <instrlib>:"niScope Fetch (poly).vi"("timeout"=1.0, "error in"=w3911, "channels"="0,1", "instrument handle"=w3912) -> ("error out"=w3855:errorcluster, "wfm"=w3856:i16[][], "wfm info"=w3877:T49)  [unwired: 4 in, 1 out]
          n1766 = property on="Property Node" class="niScope"(reference=w3901, "Fetch Record Number"=w3858) -> (reference out=w3905:refnum<k15>, error out=w3902:errorcluster, "Records Done"=w3859:i32)  [unwired: 1 in]
          n1767 = Divide(x=w3856, y=w3894) -> (x/y=w3867:dbl[][])
          n1768 = Tick Count (ms)() -> (millisecond timer value=w3868:u32)
          n1769 = Subtract(x=w3859, y=w3858) -> (x-y=→"Record Backlog 2":i32)
          n1770 = Subtract(x=w3868, y=w3893) -> (x-y=→"Aquisition loop timing(ms)":u32)
          n1771 = Subtract(x=w3868, y=w3872) -> (x-y=w3876:u32)
          n1772 = Multiply(x=w3867, y=w3878) -> (x*y=w3898:dbl[][])
          n1773 = call-poly <instrlib>:"niScope Fetch (poly).vi"("timeout"=0.25, "error in"=w3902, "channels"="0,1", "instrument handle"=w3905) -> ("error out"=w3854:errorcluster, "wfm"=w3895:i16[][])  [unwired: 4 in, 2 out]
          n1774 = Greater?(x=w3876, y=u32 1000) -> (0:w3874:bool)
          n1775 = Add(x=w3898, y=w3879) -> (x+y=w3889:dbl[][])
          n1776 = case shown="True" w3874 {
            tunnel: w3877 -> [_ w3921]
            tunnel: w3868 -> [_ w3920]
            tunnel: [w3914 w3920] -> w3873
            tunnel: w3872 -> [w3914 _]
            tunnel: [errorcluster {"status"=FALSE, "code"=0, "source"=""} ("error constant") w3917] -> w3869
            frame False {
            }
            frame True {
              # "[Covers: REQ29]"
              n1777 = call "CheckFrequency(SubVI).vi"("wfm info"=w3921) -> ("f (Hz)"=w3919:dbl)  [unwired: 10 in]
              "Laser f (Hz)" <- w3919
              n1778 = local read "Laser Rep Rate"() -> (w3916:dbl)
              n1779 = Increment(x=w3916) -> (x+1=w3915:dbl)
              n1780 = Greater?(x=w3919, y=w3915) -> (0:w3918:bool)
              n1781 = case shown="True" w3918 {
                tunnel: [errorcluster {"status"=FALSE, "code"=0, "source"=""} ("error constant") errorcluster {"status"=TRUE, "code"=0, "source"=""} ("error constant")] -> w3917
                frame False {
                }
                frame True {
                }
              }
            }
          }
          n1782 = Divide(x=w3895, y=w3894) -> (x/y=w3897:dbl[][])
          n1783 = Enqueue Element(queue=w3890, element=w3889, error in (no error)=w3855) -> (error out=w3853:errorcluster)  [unwired: 1 in, 2 out]
          n1784 = Multiply(x=w3897, y=w3878) -> (x*y=w3896:dbl[][])
          n1785 = Add(x=w3896, y=w3879) -> (x+y=w3887:dbl[][])
          n1786 = Enqueue Element(queue=w3888, element=w3887, error in (no error)=w3854) -> (error out=w3852:errorcluster)  [unwired: 1 in, 2 out]
          n1787 = Merge Errors(w3853, w3852) -> (w3851:errorcluster)
          n1788 = call "V1FGV.vi"("Error In"=w3851, "action (write)"=w3861) -> ("Error Out"=w3885:errorcluster, "V1 out"=w3883:dbl)  [unwired: 8 in]
          n1789 = call "V2FGV.vi"("Error In"=w3885, "action(write)"=w3861) -> ("Error Out"=w3884:errorcluster, "V2 out"=w3882:dbl)  [unwired: 8 in]
          n1790 = call "V3FGV.vi"("Error In"=w3884, "action(write)"=w3861) -> ("Error Out"=w3864:errorcluster, "V3 out"=w3863:dbl)  [unwired: 8 in]
          n1791 = call "V4FGV.vi"("Error In"=w3864, "action(write)"=w3861, "V3 in"=w3863) -> ("Error Out"=w3862:errorcluster, "V3 out"=w3860:dbl)  [unwired: 7 in]
          n1792 = Bundle("V1 out"=w3883, "V2 out"=w3882, "V3 out"=w3863, "V3 out"=w3860) -> (w3866:T50)  [unwired: 1 in]
          n1793 = Bundle(w3850, w3889, w3887, w3866) -> (w3891:T51)  [unwired: 1 in]
          n1794 = Enqueue Element(queue=w3881, element=w3866, error in (no error)=w3862) -> (error out=w3865:errorcluster)  [unwired: 1 in, 2 out]
          n1795 = Send Notification(notification=w3891, notifier=w3908, error in (no error)=w3865) -> (notifier out=w3907:refnum<notifier>, error out=w3870:errorcluster)
          n1796 = Merge Errors(w3869, w3870) -> (w3886:errorcluster)
          n1797 = case shown="Error .." w3886 {
            selector: w3886 -> [w3924 w3925]
            tunnel: w3899 -> [_ w3928]
            tunnel: [w3924 w3925] -> w3871
            frame No Error {
            }
            frame Error {
              # "Send user event to signal aquisition has stoped"
              n1798 = Generate User Event(priority (normal)=usereventprio."high priority", user event=w3928, event data cluster=TRUE ("event data")) -> ()  [unwired: 1 in, 2 out]
            }
          }
          "aquisition loop Error Out" <- w3871
          "Auisition Loop idx" <- w3850
        }
      }
    }
    n1799 = Unbundle By Name(w3816) -> ("status"=w3815:bool)
    n1800 = Not(x=w3815) -> (.not. x?=w3814:bool)
    n1801 = local write "Aq Loop?"(w3814) -> ()
    "Aq Loop?" <- TRUE ("Aq L?")
  }
  n1802 = disable-structure "Diagram Disable Structure" shown="Disabled" {
    frame Disabled {
      w3929 = T52 {"Horizontal"=500, "Vertical"=100}  # Top Left Corner
      n1803 = Control Help Window(0:w3929, 1:TRUE ("Show")) -> ()
      n1804 = call <vilib>:"TDMS - File Viewer.vi"() -> ()  [unwired: 6 in, 2 out]
    }
    frame Enabled {
    }
  }
  n1805 = while {
    tunnel: w19 -> [w3978]
    shift-right: [w3942] -> _
    shift-left: _ -> [w3974]
    tunnel: [w3933] -> w1 mode=indexing
    i -> [w3958]
    stop <- w3939 stop-if-true
    # "Channel 3"
    # "Channel 2"
    # "Channel 1"
    # "use FGV for gain value"
    # "stop on error"
    # "Gain adjustment and Data processing"
    n1806 = Tick Count (ms)() -> (millisecond timer value=w3942:u32)
    n1807 = Wait on Notification(notifier=w3978, ignore previous (F)=TRUE) -> (notification=w3952:T14, error out=w3932:errorcluster)  [unwired: 2 in, 2 out]
    n1808 = Subtract(x=w3942, y=w3974) -> (x-y=→"PID loop timing(ms)":u32)
    n1809 = Unbundle(w3952) -> ("CH1&2"=w3968:dbl[][], "CH3&4"=w3967:dbl[][])  [unwired: 2 out]
    n1810 = call "SeperateChanData.vi"("Input (Ch1&2)"=w3968) -> ("Ch1"=w3963:dbl[][], "Ch2"=w3961:dbl[][])
    n1811 = call "SeperateChanData.vi"("Input (Ch1&2)"=w3967) -> ("Ch1"=w3957:dbl[][], "Ch2"=w3950:dbl[][])
    n1812 = call "AvgArrayTimeCritical.vi"("2D array"=w3963) -> ("1D Avg"=w3962:dbl[])  [unwired: 10 in]
    n1813 = call "AvgArrayTimeCritical.vi"("2D array"=w3961) -> ("1D Avg"=w3972:dbl[])  [unwired: 10 in]
    n1814 = call "AvgArrayTimeCritical.vi"("2D array"=w3957) -> ("1D Avg"=w3969:dbl[])  [unwired: 10 in]
    n1815 = call "AvgArrayTimeCritical.vi"("2D array"=w3950) -> ("1D Avg"=w3949:dbl[])  [unwired: 10 in]
    n1816 = Array Max & Min(array=w3962) -> (max value=w3960:dbl)  [unwired: 3 out]
    n1817 = Array Max & Min(array=w3972) -> (max value=w3959:dbl)  [unwired: 3 out]
    n1818 = Array Max & Min(array=w3969) -> (max value=w3943:dbl)  [unwired: 3 out]
    n1819 = Array Max & Min(array=w3949) -> (max value=w3947:dbl)  [unwired: 3 out]
    n1820 = local read "Auto gain ch4"() -> (w3948:bool)
    n1821 = local read "Auto gain ch1"() -> (w3966:bool)
    n1822 = local read "Auto gain ch2"() -> (w3965:bool)
    n1823 = local read "Auto gain ch3"() -> (w3964:bool)
    n1824 = case shown="True" w3948 {
      tunnel: w3947 -> [_ w4025]
      tunnel: "V target(1.0)" -> [_ w4023]
      tunnel: [FALSE w4020] -> w3945
      tunnel: [0.0 ("CtrlV") w4015] -> w3946
      frame False {
        # "Manual control"
      }
      frame True {
        # "PID control"
        n1825 = global read "GlobalVariables.vi" "Ch4GainLim(Log)"() -> (w4026:cluster{"GainMax":dbl, "GainMin":dbl})
        n1826 = call-poly <vilib>:"PID.vi"("output range"=w4026, "PID gains"="Ch4 PID gains", "process variable"=w4025, "setpoint"=w4023) -> ("output"=w4024:dbl)  [unwired: 6 in, 1 out]
        n1827 = Power Of 10(x=w4024) -> (10^x=w4016:dbl)
        "Gain4" <- w4016
        n1828 = call "V4FGV.vi"("action(write)"=enum16{"write", "read"}."read") -> ("Error Out"=w4019:errorcluster, "V3 out"=w4021:dbl)  [unwired: 9 in]
        n1829 = call "GainToCtrlV.vi"("Gain"=w4016, "Channel"=enum16{"Ch1", "Ch2", "Ch3", "Ch4"}."Ch4") -> ("CtrlV"=w4015:dbl)  [unwired: 8 in, 1 out]
        n1830 = call "V4FGV.vi"("Error In"=w4019, "V3 in"=w4015) -> ()  [unwired: 8 in, 2 out]
        n1831 = local write "V 4"(w4015) -> ()
        n1832 = Not Equal?(x=w4015, y=w4021) -> (x != y?=w4020:bool)
      }
    }
    n1833 = case shown="True" w3966 {
      tunnel: "V target(1.0)" -> [_ w4040]
      tunnel: w3960 -> [_ w4037]
      tunnel: [0.0 ("CtrlV") w4029] -> w3940
      tunnel: [FALSE w4031] -> w3956
      frame False {
        # "Manual control"
      }
      frame True {
        # "PID control"
        n1834 = global read "GlobalVariables.vi" "Ch1GainLim(Log)"() -> (w4036:cluster{"GainMax":dbl, "GainMin":dbl})
        n1835 = call-poly <vilib>:"PID.vi"("output range"=w4036, "PID gains"="Ch1 PID gains", "process variable"=w4037, "setpoint"=w4040) -> ("output"=w4035:dbl)  [unwired: 6 in, 1 out]
        n1836 = Power Of 10(x=w4035) -> (10^x=w4034:dbl)
        "Gain1" <- w4034
        n1837 = call "V1FGV.vi"("action (write)"=enum16{"write", "read"}."read") -> ("Error Out"=w4030:errorcluster, "V1 out"=w4032:dbl)  [unwired: 9 in]
        n1838 = call "GainToCtrlV.vi"("Gain"=w4034, "Channel"=enum16{"Ch1", "Ch2", "Ch3"}."Ch1") -> ("CtrlV"=w4029:dbl)  [unwired: 8 in, 1 out]
        n1839 = local write "V 1"(w4029) -> ()
        n1840 = call "V1FGV.vi"("Error In"=w4030, "V1 in"=w4029) -> ()  [unwired: 8 in, 2 out]
        n1841 = Not Equal?(x=w4029, y=w4032) -> (x != y?=w4031:bool)
      }
    }
    n1842 = case shown="True" w3965 {
      tunnel: w3959 -> [_ w4067]
      tunnel: "V target(1.0)" -> [_ w4068]
      tunnel: [FALSE w4061] -> w3955
      tunnel: [0.0 ("CtrlV") w4057] -> w3951
      frame False {
        # "Manual control"
      }
      frame True {
        # "PID control"
        n1843 = global read "GlobalVariables.vi" "Ch2GainLim(Log)"() -> (w4065:cluster{"GainMax":dbl, "GainMin":dbl})
        n1844 = call-poly <vilib>:"PID.vi"("output range"=w4065, "PID gains"="Ch2 PID gains", "process variable"=w4067, "setpoint"=w4068) -> ("output"=w4064:dbl)  [unwired: 6 in, 1 out]
        n1845 = Power Of 10(x=w4064) -> (10^x=w4062:dbl)
        "Gain2" <- w4062
        n1846 = call "V2FGV.vi"("action(write)"=enum16{"write", "read"}."read") -> ("Error Out"=w4058:errorcluster, "V2 out"=w4059:dbl)  [unwired: 9 in]
        n1847 = call "GainToCtrlV.vi"("Gain"=w4062, "Channel"=enum16{"Ch1", "Ch2", "Ch3"}."Ch2") -> ("CtrlV"=w4057:dbl)  [unwired: 8 in, 1 out]
        n1848 = local write "V 2"(w4057) -> ()
        n1849 = call "V2FGV.vi"("Error In"=w4058, "V2 in"=w4057) -> ()  [unwired: 8 in, 2 out]
        n1850 = Not Equal?(x=w4057, y=w4059) -> (x != y?=w4061:bool)
      }
    }
    n1851 = case shown="True" w3964 {
      tunnel: w3943 -> [_ w4052]
      tunnel: "V target(1.0)" -> [_ w4049]
      tunnel: [FALSE w4045] -> w3954
      tunnel: [0.0 ("CtrlV") w4043] -> w3953
      frame False {
        # "Manual control"
      }
      frame True {
        # "PID control"
        n1852 = global read "GlobalVariables.vi" "Ch3GainLim(Log)"() -> (w4053:cluster{"GainMax":dbl, "GainMin":dbl})
        n1853 = call-poly <vilib>:"PID.vi"("output range"=w4053, "PID gains"="Ch3 PID gains", "process variable"=w4052, "setpoint"=w4049) -> ("output"=w4051:dbl)  [unwired: 6 in, 1 out]
        n1854 = Power Of 10(x=w4051) -> (10^x=w4048:dbl)
        "Gain3" <- w4048
        n1855 = call "V3FGV.vi"("action(write)"=enum16{"write", "read"}."read") -> ("Error Out"=w4044:errorcluster, "V3 out"=w4046:dbl)  [unwired: 9 in]
        n1856 = call "GainToCtrlV.vi"("Gain"=w4048, "Channel"=enum16{"Ch1", "Ch2", "Ch3"}."Ch3") -> ("CtrlV"=w4043:dbl)  [unwired: 8 in, 1 out]
        n1857 = local write "V 3"(w4043) -> ()
        n1858 = call "V3FGV.vi"("Error In"=w4044, "V3 in"=w4043) -> ()  [unwired: 8 in, 2 out]
        n1859 = Not Equal?(x=w4043, y=w4046) -> (x != y?=w4045:bool)
      }
    }
    n1860 = call "LabJack_FGV.vi"("Operation(Read)"=enum16{"Write", "Read"}."Read" ("Operation"), "error in (no error)"=w3932) -> ("error out"=w3941:errorcluster, "Read data"=w3976:i32)  [unwired: 8 in]
    n1861 = flat-sequence {
      tunnel: [w3980] -> w3938
      tunnel: w3932 -> [_]
      frame #0 {
        n1862 = Tick Count (ms)() -> (millisecond timer value=w3980:u32)
      }
    }
    n1863 = case "Channel 1" shown="True" w3956 {
      tunnel: w3941 -> [w4006 w4012]
      tunnel: w3976 -> [w4005 w4011]
      tunnel: [w4006 w4007] -> w3936
      tunnel: [w4005 w4010] -> w3971
      tunnel: w3940 -> [_ w4008]
      frame False {
        # "Do nothing"
      }
      frame True {
        # "request V\nupdate FGV"
        n1864 = global read "GlobalVariables.vi" "Ch1 LJ pin"() -> (w4009:string)
        n1865 = call "LJM_eWriteName.vi"("Handle In"=w4011, "Name"=w4009, "Value"=w4008, "error in"=w4012) -> ("Handle Out"=w4010:i32, "error out"=w4007:errorcluster)  [unwired: 10 in]
      }
    }
    n1866 = case "Channel 2" shown="True" w3955 {
      tunnel: w3936 -> [w3997 w4004]
      tunnel: [w3997 w3999] -> w3935
      tunnel: w3971 -> [w3998 w4003]
      tunnel: [w3998 w4002] -> w3970
      tunnel: w3951 -> [_ w4000]
      frame False {
        # "Do nothing"
      }
      frame True {
        # "request V\nupdate FGV"
        n1867 = global read "GlobalVariables.vi" "Ch2 LJ pin"() -> (w4001:string)
        n1868 = call "LJM_eWriteName.vi"("Handle In"=w4003, "Name"=w4001, "Value"=w4000, "error in"=w4004) -> ("Handle Out"=w4002:i32, "error out"=w3999:errorcluster)  [unwired: 10 in]
      }
    }
    n1869 = case "Channel 3" shown="True" w3954 {
      tunnel: w3935 -> [w3990 w3996]
      tunnel: [w3990 w3992] -> w3934
      tunnel: w3970 -> [w3989 w3995]
      tunnel: w3953 -> [_ w3993]
      tunnel: [w3989 w3991] -> w3944
      frame False {
        # "Do nothing"
      }
      frame True {
        # "request V\nupdate FGV"
        n1870 = global read "GlobalVariables.vi" "Ch3 LJ pin"() -> (w3994:string)
        n1871 = call "LJM_eWriteName.vi"("Handle In"=w3995, "Name"=w3994, "Value"=w3993, "error in"=w3996) -> ("Handle Out"=w3991:i32, "error out"=w3992:errorcluster)  [unwired: 10 in]
      }
    }
    n1872 = case "Channel 4" shown="True" w3945 {
      tunnel: w3934 -> [w3982 w3988]
      tunnel: w3944 -> [w3981 w3987]
      tunnel: [w3982 w3983] -> w3939
      tunnel: [w3981 w3986] -> _
      tunnel: w3946 -> [_ w3984]
      frame False {
        # "Do nothing"
      }
      frame True {
        # "request V\nupdate FGV"
        n1873 = global read "GlobalVariables.vi" "Ch4 LJ pin"() -> (w3985:string)
        n1874 = call "LJM_eWriteName.vi"("Handle In"=w3987, "Name"=w3985, "Value"=w3984, "error in"=w3988) -> ("Handle Out"=w3986:i32, "error out"=w3983:errorcluster)  [unwired: 10 in]
      }
    }
    "PID loop error out" <- w3939
    n1875 = flat-sequence {
      tunnel: [w3979] -> w3937
      tunnel: w3939 -> [_]
      frame #0 {
        n1876 = Tick Count (ms)() -> (millisecond timer value=w3979:u32)
      }
    }
    n1877 = Subtract(x=w3937, y=w3938) -> (x-y=w3933:u32)
    "LJ process (ms)" <- w3933
    "PID loop" <- w3958
  }
  "LJ time(ms)" <- w1
  n1878 = Unregister For Events(event registration refnum=w46, error in=w4) -> (error out=w52:errorcluster)
  n1879 = Destroy User Event(user event=w39, error in=w52) -> (error out=w3:errorcluster)
  n1880 = Close File(refnum=w21, error in=w3) -> ()  [unwired: 2 out]
  n1881 = Release Notifier(notifier=w16, error in (no error)=w49) -> (error out=w50:errorcluster)  [unwired: 1 in, 2 out]
  n1882 = Release Notifier(notifier=w17, error in (no error)=w38) -> (error out=w43:errorcluster)  [unwired: 1 in, 2 out]
  n1883 = call <vilib>:"Simple Error Handler.vi"("error in (no error)"=w50) -> ()  [unwired: 4 in, 5 out]
  n1884 = call <vilib>:"Simple Error Handler.vi"("error in (no error)"=w43) -> ()  [unwired: 4 in, 5 out]
  n1885 = Release Notifier(notifier=w59, error in (no error)=w58) -> (error out=w57:errorcluster)  [unwired: 1 in, 2 out]
  n1886 = Unregister For Events(event registration refnum=w63, error in=w61) -> (error out=w62:errorcluster)
  n1887 = call <vilib>:"Simple Error Handler.vi"("error in (no error)"=w57) -> ()  [unwired: 4 in, 5 out]
  n1888 = Destroy User Event(user event=w53, error in=w62) -> ()  [unwired: 1 out]
